vi "CRYStimulus Editor Sub.vi"(8 "List Index":i32, 9 "Stimulus In":T2={"StimulusType"="", "UseMLValArray"=[], "ML_axisArray"=[], "MLValLevelNameArray"=[], "Level(U)Array"=[1.0, 0.0, 0.0, 0.0, 0.0, 0.0, 0.26], "Start(Stop)FreqArray"=[20000.0, 20.0], "Start(Stop)AmpArray"=[0.5, 1.0], "StepResolutionArray"=[], "Unit_Array"=[], "DegValArray"=[], "DegUnitArray"=[], "Steps1"=19, "Cycle/step1(#)"=20, "Time/step1(s)"=0.01, "Transition1"=0.0, "SweepRate2"=1.0, "Freq3(Hz)"=0.0, "Steps3(#)"=19.0, "Cycles3(#)"=12, "StepSize3"=0.0, "wave time"="", "RMS_Value4"=0.0, "Peak_Value4"=0.0, "WavePath4"="", "RMS_unit4"="", "Peak_unit4"="", "wave Info"="", "dc_ctrl5_1"=0, "dc_ctrl5_2"=0, "dc_polar5"=0, "Max.Current"=0, "Steps5(#)"=19, "Time/Step5"=0.05, "Level5"=0.0, "StepsSize5Val"=0.0, "StepSize5Unit"="", "SweepType"=0, "Fixed/Ratio6"=0, "Transition6"=0.0, "Steps6(#)"=19.0, "Cycle/Steps6(#)"=12, "Time/Steps6(s)"=0.0, "Freq6(Hz)"=0.0, "Difference6(Hz)"=0.0, "Ratio6"="", "NoiseType7"=0, "Duration7(s)"=1.0, "MinFreq7(Hz)"=20000.0, "MaxFreq7(Hz)"=20.0, "MinFreq8(Hz)"=20000.0, "MaxFreq8(Hz)"=20.0, "FreqRounding8"=FALSE, "Duration8(s)"=1.0, "Tones8"=0.0, "RoundingVal8"=0.0, "ApplyEQ"=FALSE, "Duration(s)"=0.0, "CustomStimulusName "="", "Flatten Element Array"=[], "sine waves"=[], "Channel Out"=0, "RatioVal6"=0.0, "TabCtrl6"=enum."Master Tone", "Signal Type Name"="", "Help"="", "Channel Sel"=19, "V on DUT"=FALSE, "Output Imp"=6300.0, "Nominal Imp"=100.0} {"Nominal Imp" format="%.2p"; "Output Imp" format="%.2p"; "sine waves"."cycles" format="%.2f"; "sine waves"."ampl" format="%.2f"; "sine waves"."freq" format="%.2f"}) -> (1 "Ok Boolean":bool, 2 "Flatten Element Out":string, 3 "Stimulus Out":T2={"StimulusType"="", "UseMLValArray"=[], "ML_axisArray"=[], "MLValLevelNameArray"=[], "Level(U)Array"=[1.0, 0.0, 0.0, 0.0, 0.0, 0.0, 0.26], "Start(Stop)FreqArray"=[20000.0, 20.0], "Start(Stop)AmpArray"=[0.5, 1.0], "StepResolutionArray"=[], "Unit_Array"=[], "DegValArray"=[], "DegUnitArray"=[], "Steps1"=19, "Cycle/step1(#)"=20, "Time/step1(s)"=0.01, "Transition1"=0.0, "SweepRate2"=1.0, "Freq3(Hz)"=0.0, "Steps3(#)"=19.0, "Cycles3(#)"=12, "StepSize3"=0.0, "wave time"="", "RMS_Value4"=0.0, "Peak_Value4"=0.0, "WavePath4"="", "RMS_unit4"="", "Peak_unit4"="", "wave Info"="", "dc_ctrl5_1"=0, "dc_ctrl5_2"=0, "dc_polar5"=0, "Max.Current"=0, "Steps5(#)"=19, "Time/Step5"=0.05, "Level5"=0.0, "StepsSize5Val"=0.0, "StepSize5Unit"="", "SweepType"=0, "Fixed/Ratio6"=0, "Transition6"=0.0, "Steps6(#)"=19.0, "Cycle/Steps6(#)"=12, "Time/Steps6(s)"=0.0, "Freq6(Hz)"=0.0, "Difference6(Hz)"=0.0, "Ratio6"="", "NoiseType7"=0, "Duration7(s)"=1.0, "MinFreq7(Hz)"=20000.0, "MaxFreq7(Hz)"=20.0, "MinFreq8(Hz)"=20000.0, "MaxFreq8(Hz)"=20.0, "FreqRounding8"=FALSE, "Duration8(s)"=1.0, "Tones8"=0.0, "RoundingVal8"=0.0, "ApplyEQ"=FALSE, "Duration(s)"=0.0, "CustomStimulusName "="", "Flatten Element Array"=[], "sine waves"=[], "Channel Out"=0, "RatioVal6"=0.0, "TabCtrl6"=enum."Master Tone", "Signal Type Name"="", "Help"="", "Channel Sel"=19, "V on DUT"=FALSE, "Output Imp"=6300.0, "Nominal Imp"=100.0} {"Nominal Imp" format="%.2p"; "Output Imp" format="%.2p"; "sine waves"."cycles" format="%.2f"; "sine waves"."ampl" format="%.2f"; "sine waves"."freq" format="%.2f"})   [LabVIEW 2013]
uses:
  Typedef Control/CRYStimulus Cluster.ctl
  Control/CRYfstepsw.ctl
  Control/CRYflogsw.ctl
  Control/CRYampsw.ctl
  Control/CRYwavefile.ctl
  Control/CRYdcconn.ctl
  Control/CRYtwotone.ctl
  Control/CRYnoise.ctl
  Control/CRYmltitone.ctl
  SubVI/CRYStimulus Global.vi
  CRYProject/CRYProject Editor Global.vi
  CRYMainGlobal.vi
panel:
  in  "CurLibChange":bool caption="Add Lib"
  in  "StartFreq8_Flag":string
  in  "StopFreq8_Flag":string
  in  "StartFreq7_Flag":string
  in  "StopFreq7_Flag":string
  in  "StartFreq6_Flag":string
  in  "StopFreq6_Flag":string
  in  "StartFreq2_Flag":string
  in  "StopFreq2_Flag":string
  in  "StopFreq1_Flag":string
  in  "StartFreq1_Flag":string
  in  "StartStopFreqValue":string
  in  "StartStopAxis":string
  in  "Cancel":bool caption="Apply"
  in  "OK":bool caption="Apply"
  in  "stop":bool
  in  "Board1 Tab":enum32{"Setting", "Help"}(tab)
  in  "Stimulus Type":u16(ring) caption="激励类型" items=["频率步进扫频"=0, "频率对数扫频"=1, "幅度对数扫频"=2, "WAV文件"=3, "双音信号"=5, "噪声信号"=6, "多音信号"=7]
  in  "Control Tab":T1(tab)
  in  "StopFreq1_CurLib":u16(ring) caption="unity" items=["采集延迟", "Max FSD Out 12th&3rd Oct Sweep", "Max FSD In", "unity cal-in sens-in", "CRY33x Mic 1 sens-in", "CRY33x Mic 2 sens-in", "CRY33x Mic 3 sens-in", "CRY33x Mic 4 sens-in", "USB In L sens-in", "USB In R sens-in", "unity cal-out sens-out", "CRY602 Mouth 1 sens-out", "CRY602 Mouth 2 sens-out", "USB Out R sens-out"]
  in  "StopFreq1_axis":u16(slide) scale=0.0..2.0
  out "StopFreq1_Value":dbl caption="Hz" format="%#_6p"
  in  "StartFreq1_CurLib":u16(ring) caption="unity" items=["采集延迟", "Max FSD Out 12th&3rd Oct Sweep", "Max FSD In", "unity cal-in sens-in", "CRY33x Mic 1 sens-in", "CRY33x Mic 2 sens-in", "CRY33x Mic 3 sens-in", "CRY33x Mic 4 sens-in", "USB In L sens-in", "USB In R sens-in", "unity cal-out sens-out", "CRY602 Mouth 1 sens-out", "CRY602 Mouth 2 sens-out", "USB Out R sens-out"]
  in  "StartFreq1_axis":u16(slide) scale=0.0..2.0
  out "StartFreq1_Value":dbl caption="Hz" format="%#_6p"
  in  "StartFreq1_Caption":string caption="Message"
  in  "ML axis1":u16(slide) scale=0.0..2.0
  in  "UseMLVal_Level_1":u16(slide)
  in  "Time/steps1(s)":dbl=0.01 caption="最短持续时间(s)" format="%#_3p"
  out "Transition1":dbl caption="转换频率" format="%#_3p"
  in  "Cycle/step1":u32=20 caption="最小周期数" min=1 max=1000 format="%.0p"
  in  "Steps1":i32=19 caption="步骤数" format="%.0p"
  in  "StopFreq1(Hz)":dbl=20.0 caption="停止(Hz)" step=1000.0002384185791 format="%#.3p"
  in  "StartFreq1(Hz)":dbl=20000.0 caption="开始(Hz)" step=1200.0012397766113 format="%#.3p"
  in  "Step Resolution1":u16(ring) caption="分辨率" items=["R10(1/3 Oct.)", "R20(1/6 Oct.)", "R40(1/12 Oct.)", "R80(1/24 Oct.)", "User Defined, Log", "User Defined,Linear"]
  in  "unit1":u16(ring) items=["V  RMS", "dB re 1V"]
  in  "Level(U)1":dbl=1.0 format="%-#1.3p"
  out "deg1":dbl caption="Hz" format="%#_6p"
  in  "ML val level name":u16(ring) caption="unity" items=["unity cal-in sens-in", "CRY33x Mic 1 sens-in", "CRY33x Mic 2 sens-in", "CRY33x Mic 3 sens-in", "CRY33x Mic 4 sens-in", "USB In L sens-in", "USB In R sens-in", "unity cal-out sens-out", "CRY602 Mouth 1 sens-out", "CRY602 Mouth 2 sens-out", "USB Out R sens-out"]
  out "Level1":bool caption="幅度"
  out "Step Progression1":bool caption="步进设置"
  out "Frequency Range1":bool caption="频率范围"
  out "Step Size1":bool caption="步长"
  in  "StopFreq1_Caption":string caption="Message"
  in  "Nominal Imp1":dbl=1.0 caption="额定阻抗" min=1.0 max=2000.0 format="%-#1.3f"
  in  "Output Imp1":u16(ring) caption="输出阻抗" items=["1", "33", "150", "600", "750"]
  in  "V on DUT1":bool caption="Boolean"
  in  "V on DUT2":bool caption="Boolean"
  in  "Output Imp2":u16(ring) caption="输出阻抗" items=["1", "33", "150", "600", "750"]
  in  "Nominal Imp2":dbl=1.0 caption="额定阻抗" min=1.0 max=2000.0 format="%-#1.3f"
  in  "StopFreq2_CurLib":u16(ring) caption="unity" items=["采集延迟", "Max FSD Out 12th&3rd Oct Sweep", "Max FSD In", "unity cal-in sens-in", "CRY33x Mic 1 sens-in", "CRY33x Mic 2 sens-in", "CRY33x Mic 3 sens-in", "CRY33x Mic 4 sens-in", "USB In L sens-in", "USB In R sens-in", "unity cal-out sens-out", "CRY602 Mouth 1 sens-out", "CRY602 Mouth 2 sens-out", "USB Out R sens-out"]
  in  "StopFreq2_axis":u16(slide) scale=0.0..2.0
  out "StopFreq2_Value":dbl caption="Hz" format="%#_6p"
  in  "StartFreq2_CurLib":u16(ring) caption="unity" items=["采集延迟", "Max FSD Out 12th&3rd Oct Sweep", "Max FSD In", "unity cal-in sens-in", "CRY33x Mic 1 sens-in", "CRY33x Mic 2 sens-in", "CRY33x Mic 3 sens-in", "CRY33x Mic 4 sens-in", "USB In L sens-in", "USB In R sens-in", "unity cal-out sens-out", "CRY602 Mouth 1 sens-out", "CRY602 Mouth 2 sens-out", "USB Out R sens-out"]
  in  "StartFreq2_axis":u16(slide) scale=0.0..2.0
  out "StartFreq2_Value":dbl caption="Hz" format="%#_6p"
  out "Frequency Range2":bool caption="频率范围"
  out "Step Progression2":bool caption="步进设置"
  out "Level2":bool caption="幅度"
  in  "Sweept Rate2(s/dec)":dbl=1.0 caption="扫频速率(s/dec)" format="%#.3p"
  in  "StopFreq2(Hz)":dbl=100.0 caption="停止(Hz)" format="%#.3p"
  in  "StartFreq2(Hz)":dbl=10.0 caption="开始(Hz)" max=20000.0 format="%#.3p"
  in  "unit2":u16(ring) items=["V  RMS", "dB re 1V"]
  in  "Level(U)2":dbl=1.0 min=3.355e-21 max=1.84838 format="%-#1.3p"
  in  "ML val level name2":u16(ring) caption="unity" items=["unity cal-in sens-in", "CRY33x Mic 1 sens-in", "CRY33x Mic 2 sens-in", "CRY33x Mic 3 sens-in", "CRY33x Mic 4 sens-in", "USB In L sens-in", "USB In R sens-in", "unity cal-out sens-out", "CRY602 Mouth 1 sens-out", "CRY602 Mouth 2 sens-out", "USB Out R sens-out"]
  out "deg2":dbl caption="Hz" format="%#_6p"
  in  "UseMLVal_Level_2":u16(slide)
  in  "ML axis2":u16(slide) scale=0.0..2.0
  in  "StopFreq2_Caption":string caption="Message"
  in  "StartFreq2_Caption":string caption="Message"
  in  "Steps3":i32=19 caption="步骤数" format="%.0p"
  out "Step Size3":dbl caption="步长" format="%#.3p"
  in  "unit3":u16(ring) items=["V  RMS", "dB re 1V"]
  in  "Cycles3":u32=12 caption="周期" min=1 step=1 format="%.0p"
  in  "Stop Amp3":dbl=1.0 caption="停止" min=0.0 format="%#.3p"
  in  "Start Amp3":dbl=0.5 caption="开始" min=0.0 format="%#.3p"
  in  "Freq3(Hz)":dbl=1000.0 format="%#.3p"
  in  "ML val level name3":u16(ring) caption="unity" items=["unity cal-in sens-in", "CRY33x Mic 1 sens-in", "CRY33x Mic 2 sens-in", "CRY33x Mic 3 sens-in", "CRY33x Mic 4 sens-in", "USB In L sens-in", "USB In R sens-in", "unity cal-out sens-out", "CRY602 Mouth 1 sens-out", "CRY602 Mouth 2 sens-out", "USB Out R sens-out"]
  out "deg3":dbl caption="Hz" format="%#_6p"
  in  "UseMLVal_Level_3":u16(slide)
  in  "ML axis3":u16(slide) scale=0.0..2.0
  out "Frequency(Hz)3":bool caption="频率(Hz)"
  out "Step Progression3":bool caption="步进设置"
  out "Level Range3":bool caption="幅度范围"
  in  "Wave Channel":u16(ring) caption="通道" items=["Left", "Right"]
  in  "Wave Path4":path caption="波形文件路径"
  out "wave time":string caption="RMS"
  out "wave info":string caption="Peak"
  in  "RMS unit4":u16(ring) items=["dB FSD", "% FSD"]
  out "RMS value4":dbl caption="RMS"
  in  "Peak unit4":u16(ring) items=["dB FSD", "% FSD"]
  out "Peak value4":dbl caption="峰值"
  in  "unit4":u16(ring) items=["V  RMS", "dB RMS", "Vp"]
  in  "Level4(U)":dbl=1.0 min=0.0 max=1.84838 format="%#.3p"
  in  "ML val level name4":u16(ring) caption="unity" items=["unity cal-in sens-in", "CRY33x Mic 1 sens-in", "CRY33x Mic 2 sens-in", "CRY33x Mic 3 sens-in", "CRY33x Mic 4 sens-in", "USB In L sens-in", "USB In R sens-in", "unity cal-out sens-out", "CRY602 Mouth 1 sens-out", "CRY602 Mouth 2 sens-out", "USB Out R sens-out"]
  out "deg4":dbl caption="Hz" format="%#_6p"
  in  "UseMLVal_Level_4":u16(slide)
  in  "ML axis4":u16(slide) scale=0.0..2.0
  out "Level4":bool caption="幅度"
  out "WAV Info4":bool caption="WAV信息"
  in  "V on DUT4":bool caption="Boolean"
  in  "Output Imp4":u16(ring) caption="输出阻抗" items=["1", "33", "150", "600", "750"]
  in  "Nominal Imp4":dbl=1.0 caption="额定阻抗" min=1.0 max=2000.0 format="%-#1.3f"
  in  "dcpolar5":u16(slide) caption="极性"
  in  "dc_ctrl5_2":u16(slide) caption="源类型"
  out "Boolean3":bool
  in  "StopAmp5":dbl=1.0 caption="停止" format="%#.3p"
  in  "Time/Step5":dbl=0.05 caption="时间/步(s)" format="%.0p"
  out "Steps Size5":dbl caption="步长" format="%#_3g"
  in  "Steps5":i32=19 caption="步骤数" format="%.0p"
  in  "Level5":dbl caption="幅度"
  in  "dc_ctrl5_1":u16(slide) caption="控制方法"
  in  "Max.Current":u16(slide) caption="最大电流"
  in  "StartAmp5":dbl=1.0 caption="开始" format="%#.3p"
  out "Instrument Settings5":bool caption="仪器设置"
  out "Sweep Settings5":bool caption="扫描设置"
  out "Level Range5":bool caption="幅度范围"
  out "unit5_1":string
  out "unit5_2":string
  in  "Control6 Tab":enum32{"Master Tone", "Slave Tone"}(tab)
  out "Step Size6":bool caption="步长"
  out "Frequency Range6":bool caption="频率范围"
  out "Transition6":dbl caption="转换频率" format="%#_3p"
  in  "Time/step6(s)":dbl caption="最短持续时间(s)" min=0.0 format="%#.2p"
  in  "Cycle/steps6":u32=12 caption="最小周期数" min=1 step=1 format="%.0p"
  in  "StopFreq6(Hz)":dbl=100.0 caption="停止(Hz)" min=1.0 step=3.999999761581421 format="%#.3p"
  in  "StartFreq6(Hz)":dbl=6300.0 caption="开始(Hz)" min=1.0 step=3999.999761581421 format="%#.3p"
  in  "Steps6":i32=19 caption="步骤数" format="%.0p"
  in  "unit6":u16(ring) items=["V  RMS", "dB re 1V"]
  in  "Level6_1(U)":dbl=1.0 format="%#.3p"
  in  "StepResolution6":u16(ring) caption="分辨率" items=["R10(1/3 Oct.)", "R20(1/6 Oct.)", "R40(1/12 Oct.)", "R80(1/24 Oct.)", "User Defined, Log", "User Defined,Linear"]
  in  "deg6":dbl caption="Hz" format="%#_6p"
  in  "ML val level name6_1":u16(ring) caption="unity" items=["unity cal-in sens-in", "CRY33x Mic 1 sens-in", "CRY33x Mic 2 sens-in", "CRY33x Mic 3 sens-in", "CRY33x Mic 4 sens-in", "USB In L sens-in", "USB In R sens-in", "unity cal-out sens-out", "CRY602 Mouth 1 sens-out", "CRY602 Mouth 2 sens-out", "USB Out R sens-out"]
  in  "ML axis6_1":u16(slide) scale=0.0..2.0
  in  "UseMLVal_Level6_1":u16(slide)
  out "Level6":bool caption="幅度"
  in  "StartFreq6_Caption":string caption="Message"
  in  "StopFreq6_Caption":string caption="Message"
  in  "StartFreq6_CurLib":u16(ring) caption="unity" items=["采集延迟", "Max FSD Out 12th&3rd Oct Sweep", "Max FSD In", "unity cal-in sens-in", "CRY33x Mic 1 sens-in", "CRY33x Mic 2 sens-in", "CRY33x Mic 3 sens-in", "CRY33x Mic 4 sens-in", "USB In L sens-in", "USB In R sens-in", "unity cal-out sens-out", "CRY602 Mouth 1 sens-out", "CRY602 Mouth 2 sens-out", "USB Out R sens-out"]
  in  "StartFreq6_axis":u16(slide) scale=0.0..2.0
  out "StartFreq6_Value":dbl caption="Hz" format="%#_6p"
  in  "StopFreq6_CurLib":u16(ring) caption="unity" items=["采集延迟", "Max FSD Out 12th&3rd Oct Sweep", "Max FSD In", "unity cal-in sens-in", "CRY33x Mic 1 sens-in", "CRY33x Mic 2 sens-in", "CRY33x Mic 3 sens-in", "CRY33x Mic 4 sens-in", "USB In L sens-in", "USB In R sens-in", "unity cal-out sens-out", "CRY602 Mouth 1 sens-out", "CRY602 Mouth 2 sens-out", "USB Out R sens-out"]
  in  "StopFreq6_axis":u16(slide) scale=0.0..2.0
  out "StopFreq6_Value":dbl caption="Hz" format="%#_6p"
  in  "Fixed/Ratio6":u16(slide)
  in  "Ratio Freq6(Hz)":dbl=1000.0 caption="Fixed Tone(Hz)" format="%#_1p"
  in  "Difference6(Hz)":dbl=100.0 caption="差异(Hz)" format="%#_3p"
  in  "Freq6(Hz)":dbl=1000.0 caption="Fixed Tone(Hz)" format="%#.3p"
  in  "deg6_1":dbl caption="Hz" format="%#_6p"
  in  "ML val level name6_2":u16(ring) caption="unity" items=["unity cal-in sens-in", "CRY33x Mic 1 sens-in", "CRY33x Mic 2 sens-in", "CRY33x Mic 3 sens-in", "CRY33x Mic 4 sens-in", "USB In L sens-in", "USB In R sens-in", "unity cal-out sens-out", "CRY602 Mouth 1 sens-out", "CRY602 Mouth 2 sens-out", "USB Out R sens-out"]
  in  "unit6_1":u16(ring) items=["V  RMS", "dB re 1V"]
  in  "Level6_2(U)":dbl format="%#.3p"
  in  "Ratio6":u16(ring) caption="比率" items=["1/1 Oct.", "1/3 Oct.", "1/6 Oct.", "1/12 Oct.", "1/24 Oct.", "User Defined"]
  out "Boolean6":bool
  in  "UseMLVal_Level6_2":u16(slide)
  in  "ML axis6_2":u16(slide) scale=0.0..2.0
  out "Level6_1":bool caption="幅度"
  out "Fixed Ton (Hz)6":bool caption="固定音调(Hz)"
  in  "Sweep Type":u16(slide)
  out "Sweep Type6":bool caption="扫频类型"
  in  "Noise Type7":u16(slide)
  in  "Duration7(s)":dbl=1.0 caption="时间(s)" min=0.0 format="%#.3p"
  in  "StopFreq7(Hz)":dbl=20.0 caption="Stop(Hz)" min=0.001 format="%#.3p"
  in  "StartFreq7(Hz)":dbl=20000.0 caption="Start(Hz)" min=0.001 format="%#.3p"
  in  "unit7":u16(ring) items=["V  RMS", "dB RMS", "Vp"]
  in  "Level7(U)":dbl=0.26 format="%#_3p"
  in  "ML val level name7":u16(ring) caption="unity" items=["unity cal-in sens-in", "CRY33x Mic 1 sens-in", "CRY33x Mic 2 sens-in", "CRY33x Mic 3 sens-in", "CRY33x Mic 4 sens-in", "USB In L sens-in", "USB In R sens-in", "unity cal-out sens-out", "CRY602 Mouth 1 sens-out", "CRY602 Mouth 2 sens-out", "USB Out R sens-out"]
  out "deg7":dbl caption="Hz" format="%#_6p"
  in  "UseMLVal_Level_7":u16(slide)
  in  "ML axis7":u16(slide) scale=0.0..2.0
  out "Level7":bool caption="幅度"
  out "Noise7":bool caption="噪音"
  out "Frequency Range7":bool caption="频率范围"
  in  "StopFreq7_Caption":string caption="Message"
  in  "StartFreq7_Caption":string caption="Message"
  in  "StartFreq7_CurLib":u16(ring) caption="unity" items=["采集延迟", "Max FSD Out 12th&3rd Oct Sweep", "Max FSD In", "unity cal-in sens-in", "CRY33x Mic 1 sens-in", "CRY33x Mic 2 sens-in", "CRY33x Mic 3 sens-in", "CRY33x Mic 4 sens-in", "USB In L sens-in", "USB In R sens-in", "unity cal-out sens-out", "CRY602 Mouth 1 sens-out", "CRY602 Mouth 2 sens-out", "USB Out R sens-out"]
  in  "StartFreq7_axis":u16(slide) scale=0.0..2.0
  out "StartFreq7_Value":dbl caption="Hz" format="%#_6p"
  in  "StopFreq7_CurLib":u16(ring) caption="unity" items=["采集延迟", "Max FSD Out 12th&3rd Oct Sweep", "Max FSD In", "unity cal-in sens-in", "CRY33x Mic 1 sens-in", "CRY33x Mic 2 sens-in", "CRY33x Mic 3 sens-in", "CRY33x Mic 4 sens-in", "USB In L sens-in", "USB In R sens-in", "unity cal-out sens-out", "CRY602 Mouth 1 sens-out", "CRY602 Mouth 2 sens-out", "USB Out R sens-out"]
  in  "StopFreq7_axis":u16(slide) scale=0.0..2.0
  out "StopFreq7_Value":dbl caption="Hz" format="%#_6p"
  in  "V on DUT7":bool caption="Boolean"
  in  "Output Imp7":u16(ring) caption="输出阻抗" items=["1", "33", "150", "600", "750"]
  in  "Nominal Imp7":dbl=1.0 caption="额定阻抗" min=1.0 max=2000.0 format="%-#1.3f"
  in  "Rounding Val8":dbl=5.0 caption="舍入值(Hz)" format="%#.3f"
  in  "Freq Rounding8":bool caption="频率四舍五入"
  in  "Duration8(s)":dbl=1.0 caption="持续时间(s)" min=0.0 format="%#.3p"
  in  "Tones8":i32 caption="多音数量" format="%.0p"
  in  "StopFreq8(Hz)":dbl=20.0 caption="Stop(Hz)" min=1.0 step=3.999999761581421 format="%#.3p"
  in  "StartFreq8(Hz)":dbl=20000.0 caption="Start(Hz)" min=1.0 step=3999.999761581421 format="%#.3p"
  out "deg8":dbl caption="Hz" format="%#_6p"
  in  "ML val level name8":u16(ring) caption="unity" items=["unity cal-in sens-in", "CRY33x Mic 1 sens-in", "CRY33x Mic 2 sens-in", "CRY33x Mic 3 sens-in", "CRY33x Mic 4 sens-in", "USB In L sens-in", "USB In R sens-in", "unity cal-out sens-out", "CRY602 Mouth 1 sens-out", "CRY602 Mouth 2 sens-out", "USB Out R sens-out"]
  in  "Level8(U)":dbl=0.26 format="%#.3p"
  in  "unit8":u16(ring) items=["V  RMS", "dB RMS", "Vp"]
  in  "Step Resolution8":u16(ring) caption="分辨率" items=["R10(1/3 Oct.)", "R20(1/6 Oct.)", "R40(1/12 Oct.)", "R80(1/24 Oct.)", "User Defined, Log", "User Defined,Linear"]
  in  "UseMLVal_Level_8":u16(slide)
  in  "ML axis8":u16(slide) scale=0.0..2.0
  out "Level8":bool caption="幅度"
  out "Multitone8":bool caption="多频音"
  out "Frequency Range8":bool caption="频率范围"
  in  "StopFreq8_Caption":string caption="Message"
  in  "StartFreq8_Caption":string caption="Message"
  in  "StartFreq8_CurLib":u16(ring) caption="unity" items=["采集延迟", "Max FSD Out 12th&3rd Oct Sweep", "Max FSD In", "unity cal-in sens-in", "CRY33x Mic 1 sens-in", "CRY33x Mic 2 sens-in", "CRY33x Mic 3 sens-in", "CRY33x Mic 4 sens-in", "USB In L sens-in", "USB In R sens-in", "unity cal-out sens-out", "CRY602 Mouth 1 sens-out", "CRY602 Mouth 2 sens-out", "USB Out R sens-out"]
  in  "StartFreq8_axis":u16(slide) scale=0.0..2.0
  out "StartFreq8_Value":dbl caption="Hz" format="%#_6p"
  in  "StopFreq8_CurLib":u16(ring) caption="unity" items=["采集延迟", "Max FSD Out 12th&3rd Oct Sweep", "Max FSD In", "unity cal-in sens-in", "CRY33x Mic 1 sens-in", "CRY33x Mic 2 sens-in", "CRY33x Mic 3 sens-in", "CRY33x Mic 4 sens-in", "USB In L sens-in", "USB In R sens-in", "unity cal-out sens-out", "CRY602 Mouth 1 sens-out", "CRY602 Mouth 2 sens-out", "USB Out R sens-out"]
  in  "StopFreq8_axis":u16(slide) scale=0.0..2.0
  out "StopFreq8_Value":dbl caption="Hz" format="%#_6p"
  in  "V on DUT8":bool caption="Boolean"
  in  "Output Imp8":u16(ring) caption="输出阻抗" items=["1", "33", "150", "600", "750"]
  in  "Nominal Imp8":dbl=1.0 caption="额定阻抗" min=1.0 max=2000.0 format="%-#1.3f"
  out "Proper VI No":i32
  in  "Help":string
  out "Vmax (V)":dbl
  out "Sampling Rate (Hz)":u32
  out "Sens y":dbl
  out "Max Freq":dbl=20000.0
  in  "RealFreq3(Hz)":dbl=1000.0 format="%#.3p"
  out "LinLevel2":dbl=1.0 format="%-#1_3p"
  out "LinLevel1":dbl=1.0 format="%-#1_3p"
  out "Channel Change":string
  out "MaxLevel_2":dbl=1.0 format="%-#1_3p"
  out "MaxLevel_1":dbl=1.0 format="%-#1_3p"
  out "dB ref.":dbl=1.0 format="%.2f"
  out "prefix Out":string
  in  "Res Max Freq":dbl=20000.0
  out "Stimulus Change":string
  in  "Load_Test":bool
  in  "Update":bool
  out "TSR params":T3 {"Amplit" format="%.2f"; "FStop" format="%.2f"; "FStart" format="%.2f"; "FSamp" format="%.2f"; "Tsamp" format="%.2f"; "NHarm" format="%.2f"; "MStart" format="%.2f"; "MStop" format="%.2f"; "NOffset" format="%.2f"}
  out "step size Hz":dbl caption="Hz" format="%.1f"
  # "(1,2,3,4,6_1,6_2,7,8)"
  # "(1,2,3,4,6_1,6_2,7,8)"
  # "(1,2,3,4,6_1,6_2,7,8)"
  # "(1,2,4,6_1,6_2,7,8)"
  # "(1,2,6)"
  # "(3,5)"
  # "(1,6,8)"
  # "(1,2,4,6_1,6_2,7,8)"
  # "(1,2,3,4,6_1,6_2,7,8)"
  # "(1,2,3,4,6_1,6_2,7,8)"
  # "(1,2,3,4,6_1,6_2,7,8)"
  # "(1,2,3,4,6_1,6_2,7,8)"
  # "(1,2,3,4,6_1,6_2,7,8)"
  # "(1,2,4,6_1,6_2,7,8)"
  # "(1,2,6)"
  # "(3,5)"
  # "(1,6,8)"
  # "(1,2,4,6_1,6_2,7,8)"
  # "(1,2,3,4,6_1,6_2,7,8)"
  # "(1,2,3,4,6_1,6_2,7,8)"
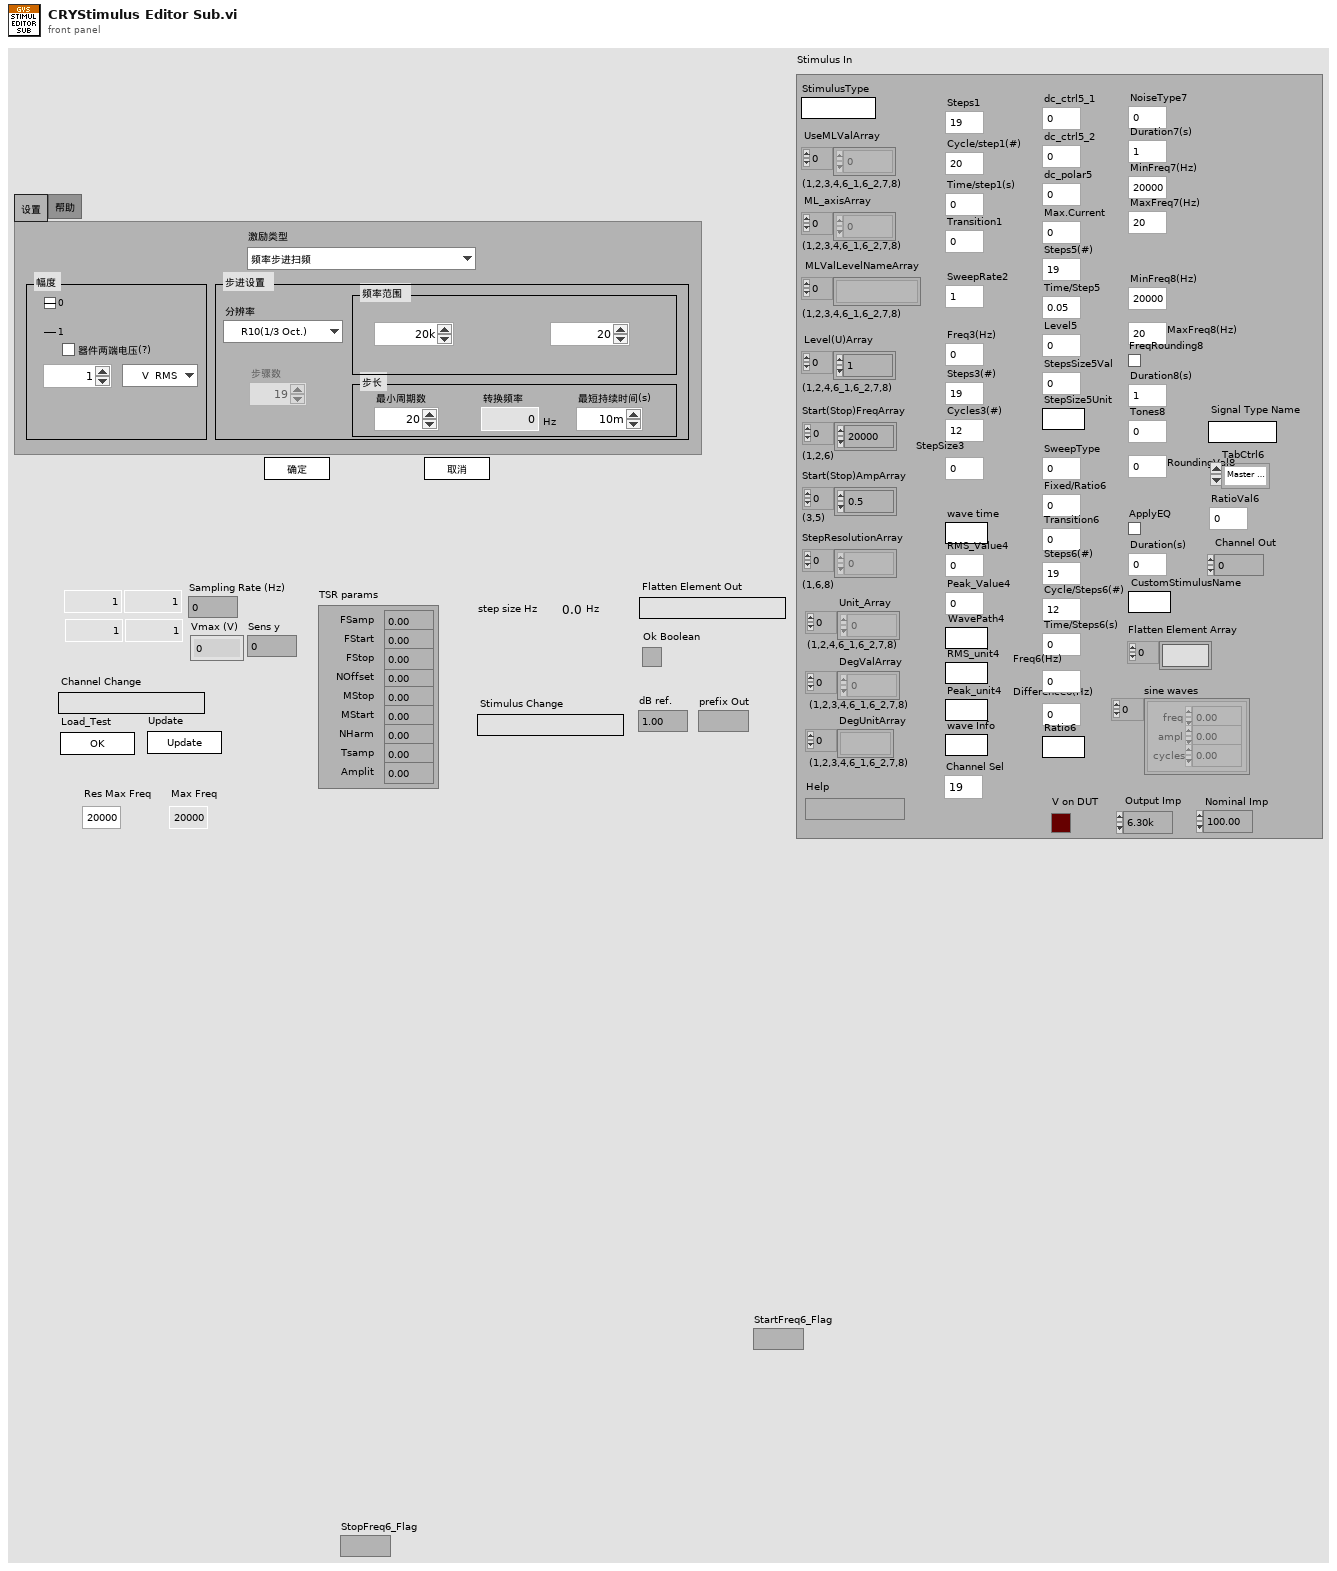
[diagram p1: front panel]
types:
  T1 = enum32{"Page1", "Page2", "Page3", "Page4", "Page5", "Page6", "Page7", "Page8"}
  T2 = typedef "CRYStimulus Cluster.ctl" = cluster{"StimulusType":string, "UseMLValArray":u16[], "ML_axisArray":u16[], "MLValLevelNameArray":string[], "Level(U)Array":dbl[], "Start(Stop)FreqArray":dbl[], "Start(Stop)AmpArray":dbl[], "StepResolutionArray":u16[], "Unit_Array":u16[], "DegValArray":dbl[], "DegUnitArray":string[], "Steps1":i32, "Cycle/step1(#)":u32, "Time/step1(s)":dbl, "Transition1":dbl, "SweepRate2":dbl, "Freq3(Hz)":dbl, "Steps3(#)":dbl, "Cycles3(#)":u32, "StepSize3":dbl, "wave time":string, "RMS_Value4":dbl, "Peak_Value4":dbl, "WavePath4":string, "RMS_unit4":string, "Peak_unit4":string, "wave Info":string, "dc_ctrl5_1":u16, "dc_ctrl5_2":u16, "dc_polar5":u16, "Max.Current":u16, "Steps5(#)":u32, "Time/Step5":dbl, "Level5":dbl, "StepsSize5Val":dbl, "StepSize5Unit":string, "SweepType":u16, "Fixed/Ratio6":u16, "Transition6":dbl, "Steps6(#)":dbl, "Cycle/Steps6(#)":u32, "Time/Steps6(s)":dbl, "Freq6(Hz)":dbl, "Difference6(Hz)":dbl, "Ratio6":string, "NoiseType7":u16, "Duration7(s)":dbl, "MinFreq7(Hz)":dbl, "MaxFreq7(Hz)":dbl, "MinFreq8(Hz)":dbl, "MaxFreq8(Hz)":dbl, "FreqRounding8":bool, "Duration8(s)":dbl, "Tones8":dbl, "RoundingVal8":dbl, "ApplyEQ":bool, "Duration(s)":dbl, "CustomStimulusName ":string, "Flatten Element Array":string[], "sine waves":cluster{"freq":dbl, "ampl":dbl, "cycles":dbl}[], "Channel Out":i32, "RatioVal6":dbl, "TabCtrl6":enum32{"Master Tone", "Slave Tone"}, "Signal Type Name":string, "Help":string, "Channel Sel":u16, "V on DUT":bool, "Output Imp":dbl, "Nominal Imp":dbl}
  T3 = cluster{"FSamp":dbl, "FStart":dbl, "FStop":dbl, "NOffset":dbl, "MStop":dbl, "MStart":dbl, "NHarm":dbl, "Tsamp":dbl, "Amplit":dbl}
  T4 = typedef "CRYStep.ctl" = cluster{"No.VI":i32, "Category":string, "StepName":string, "Seq setup flattened":string, "Comment":string, "Steps config.":bool[], "Jump config":i32[], "Start":dbl, "Increment":dbl, "Name":string, "Unit":string, "Y data":u16, "Y prefix":string, "Y dB ref":dbl, "Y unit":string, "Repeat State Array":cluster{"Start":dbl, "Increment":dbl, "Count":i32, "Num":i32}[]}
  T5 = typedef "CRYData Cluster Array.ctl" = T6[]
  T6 = typedef "CRYData Cluster.ctl" = cluster{"Name":string, "Curve":cluster{"x":dbl, "y":dbl, "z":dbl}[], "X data":u16, "Y data":u16, "Z data":u16, "X axis":u16, "Y axis":u16, "Z axis":u16, "X unit":string, "Y unit":string, "Z unit":string, "X dB ref":dbl, "Y dB ref":dbl, "Z dB ref":dbl, "single val":bool, "protected":bool, "display X":bool, "display Y":bool, "display Z":bool, "Test Info":string, "Step No.":i32, "Plot Settings":cluster{"Color":u32, "Interpolation":u8, "Point Style":u8, "Line Style":u8, "Point Color":u32, "Line Width":u8, "Bar Plot Style":u8, "Fill To":i16}, "AutoProtect":bool}
  T7 = typedef "CRYHardware.ctl" = cluster{"Name":string, "Analog I/O":u16, "Digital I/O":u16, "Channels":u8, "Dig Dev ID":u8, "N ports":u8, "Interface":u32, "Dig I/O Ports":cluster{"port #":i16, "width":i16, "direction":i32}[], "Interf settings":cluster{"Type":u16, "COM Port":u8, "Baud rate":u32, "Data bits":u32, "Parity":u16, "Stop bits":u16, "Flow control":u16, "Dev ID IEEE":u8}[], "N interfs":i32, "udev SNs":i16[], "udev enable":bool, "Channel Array":T8[], "Cal sequence":string, "SelectedIn":u16, "SelectedOut":u16, "SelectedTab":u16, "State":bool, "Help":string, "Advanced":bool, "In Audio Driver":u16, "Out Audio Driver":u16}
  T8 = typedef "CRYHardware Channel Info.ctl" = cluster{"ID":i32, "Name":string, "Digital":bool, "Input":bool, "Device Name":string, "Hardware Ch ID":u8, "Vmax (V)":dbl, "Latency (samples)":dbl, "Sampling Rate (Hz)":u32, "Bit Depth":u32, "Anti-aliasing Factor (%fs)":sgl, "DAQmx Channel":tag, "term config":i32, "Coupling":i32, "IEPE en":bool, "ASIOChannel Name":string, "Audio Driver":u16, "ASIOChannel Index":u8}
  T9 = enum8{"Enabled", "Disabled", "Disabled and Grayed Out"}
  T10 = typedef "CRYfstepsw.ctl" = cluster{"Level(U)":dbl, "Start Freq(Hz)":dbl, "Stop Freq(Hz)":dbl, "ML val level name":string, "Use ML Val level?":bool, "ML axis":u8, "Steps (#)":i32, "Cycles/step(#)":u32, "Time/step (s)":dbl, "Step Resolution":u16, "unit":u16, "Start Freq Name":string, "Stop Freq Name":string, "Start Freq Axis":u8, "Stop Freq Axis":u8, "Start Freq Flag":string, "Stop Freq Flag":string, "Output Imp":dbl, "Nominal Imp":dbl, "V on DUT":bool}
  T11 = typedef "CRYflogsw.ctl" = cluster{"Level(U)":dbl, "Start Freq(Hz)":dbl, "Stop Freq(Hz)":dbl, "Sweep Rate(s/dec)":dbl, "Use ML Val level?":bool, "ML val level name":string, "ML axis":u8, "TSR params":cluster{"FSamp":dbl, "FStart":dbl, "FStop":dbl, "NOffset":dbl, "MStop":dbl, "MStart":dbl, "NHarm":dbl, "Tsamp":dbl, "Amplit":dbl}, "unit":u16, "Start Freq Name":string, "Stop Freq Name":string, "Start Freq Axis":u8, "Stop Freq Axis":u8, "Start Freq Flag":string, "Stop Freq Flag":string, "Output Imp":dbl, "Nominal Imp":dbl, "V on DUT":bool}
  T12 = typedef "CRYampsw.ctl" = cluster{"Freq(Hz)":dbl, "Steps (#)":i32, "Cycles(#)":u32, "Use ML Val freq?":bool, "ML val freq name":string, "ML axis":u8, "Start Ampl(U)":dbl, "Stop Ampl(U)":dbl, "unit":u16}
  T13 = typedef "CRYwavefile.ctl" = cluster{"Level(U)":dbl, "Wave Path":string, "ML axis":u8, "ML val level name":string, "Use ML Val level?":bool, "wave info":string, "wave time":string, "Peak value4":dbl, "RMS value4":dbl, "wave channel":u16, "unit":u16, "Output Imp":dbl, "Nominal Imp":dbl, "V on DUT":bool}
  T14 = typedef "CRYdcconn.ctl" = cluster{"dc ctrl":u16, "dcmax I":u16, "dc polar":u16, "dc ctrl":u16, "Steps (#)":i32, "Time/step (s)":dbl, "Start Ampl(U)":dbl, "Stop Ampl(U)":dbl, "Level(U)":dbl, "Step Size":dbl}
  T15 = typedef "CRYtwotone.ctl" = cluster{"Steps (#)":i32, "Tone Type":u8, "Freq2(Hz)":dbl, "Time/step (s)":dbl, "Cycles/step (#)":u32, "ML val level name":string, "Use ML Val level?":bool, "Level(U) 2":dbl, "Diff Freq(Hz)":dbl, "ML axis 2":u8, "Diff/Ratio":u8, "Level(U)":dbl, "Stop Freq(Hz)":dbl, "Ratio Val":dbl, "ML val level name 2":string, "Use ML Val level? 2":bool, "ML axis":u8, "Start Freq(Hz)":dbl, "Step Resolution":u16, "Ratio":u16, "TabCtrl6":enum32{"Master Tone", "Slave Tone"}, "unit 1":u16, "unit 2":u16, "Start Freq Name":string, "Stop Freq Name":string, "Start Freq Axis":u8, "Stop Freq Axis":u8, "Start Freq Flag":string, "Stop Freq Flag":string}
  T16 = typedef "CRYnoise.ctl" = cluster{"Noise Type":u8, "Min Freq(Hz)":dbl, "Max Freq(Hz)":dbl, "Level(U)":dbl, "Duration(s)":dbl, "ML val level name":string, "Use ML Val level?":bool, "ML axis":u8, "unit":u16, "Start Freq Name":string, "Stop Freq Name":string, "Start Freq Axis":u8, "Stop Freq Axis":u8, "Start Freq Flag":string, "Stop Freq Flag":string, "Output Imp":dbl, "Nominal Imp":dbl, "V on DUT":bool}
  T17 = typedef "CRYmltitone.ctl" = cluster{"Level(U)":dbl, "Min Freq(Hz)":dbl, "Max Freq(Hz)":dbl, "Duration(s)":dbl, "Freq Rounding":bool, "Rounding Val":dbl, "Profile":i32, "ML axis 2":u8, "ML val level name":string, "Use ML Val level?":bool, "ML axis":u8, "Step Resolution":u16, "unit":u16, "Start Freq Name":string, "Stop Freq Name":string, "Start Freq Axis":u8, "Stop Freq Axis":u8, "Start Freq Flag":string, "Stop Freq Flag":string, "Output Imp":dbl, "Nominal Imp":dbl, "V on DUT":bool}
  T18 = typedef "CRYWaveFile Information Typedef.ctl" = cluster{"total number of samples/ch":u32, "total byte number":u32, "Time DBL":dbl, "format str":string, "Time Str":string, "peak FSD":dbl, "rms FSD":dbl, "peak %FSD":dbl, "rms %FSD":dbl, "rms":dbl, "Channel Number":u16, "rms L":dbl, "rms R":dbl}
  T19 = typedef "Sound Data Format.ctl" = cluster{"sample rate (S/s)":dbl, "number of channels":i32, "bits per sample":i32}
  T20 = typedef "CRYCalibration 2DCluster.ctl" = cluster{"Calibration":T21, "Corr Curve":T6, "EQ Curve":T6, "Sens Curve":T6}
  T21 = typedef "CRYCalibration Cluster.ctl" = cluster{"Calibration Step Name":string, "Device":string, "Correction Curve Name":string, "Equalization Curve Name":string, "Sensitivity Curve Name":string, "Corr Folder and File":string, "EQ Folder and File":string, "Sens Folder and File":string, "Corr Step size":u16, "EQ Step size":u16, "Input":bool, "Last Cal Date (sec)":timestamp, "Cha Name":string, "Corr Curve Found":bool, "EQ Curve Found":bool, "Sens Curve Found":bool, "Signal Type":string, "Calibrated Device":string, "Hz":u32}
  T22 = cluster{"Load_Test":bool, "OK":bool, "Cancel":bool}
  T23 = typedef "CRYCalibration All Cluster.ctl" = cluster{"Calibration 2D":T20[], "Help":string, "Tab Value":i32, "Input Signal Type":string, "Output Signal Type":string}
  T24 = typedef "CRYStimulus Parameter.ctl" = cluster{"Name":string, "Level Out":dbl, "Start Freq":dbl, "Stop Freq":dbl, "Steps":u32, "Cycles":u32, "Sweep type":i32, "Freq":dbl, "Start ampl":dbl, "Stop ampl":dbl, "sine waves":cluster{"freq":dbl, "ampl":dbl, "cycles":dbl}[], "wav path":string, "Sweep time":dbl, "Resolution":u16, "Tone type6":u16, "fix/ratio6":u16, "Ratio6":u16, "Difference6":u32, "RatioFreq6":u32}
  T25 = cluster{"fstepsw":T10, "flogsw":T11, "ampsw":T12, "wavefile":T13, "dcconn":T14, "twotone":T15, "mltitone":T17, "noise":T16, "sqwvsw":cluster{"Level(U)":dbl, "Duty Cycle":dbl, "ML val level name":string, "ML axis":u8, "Start Freq(Hz)":u32, "Stop Freq(Hz)":u32, "Use ML Val level?":bool, "Steps (#)":u32, "Cycles/step (#)":u32, "Time/step (s)":dbl, "Step Resolution":u16}, "tnbrst":cluster{"Level(U)":dbl, "ML val level name":string, "ML axis":u8, "Start Freq(Hz)":u32, "Use ML Val level?":bool, "Cycles/step (#)":u32, "Duration(s)":dbl}}
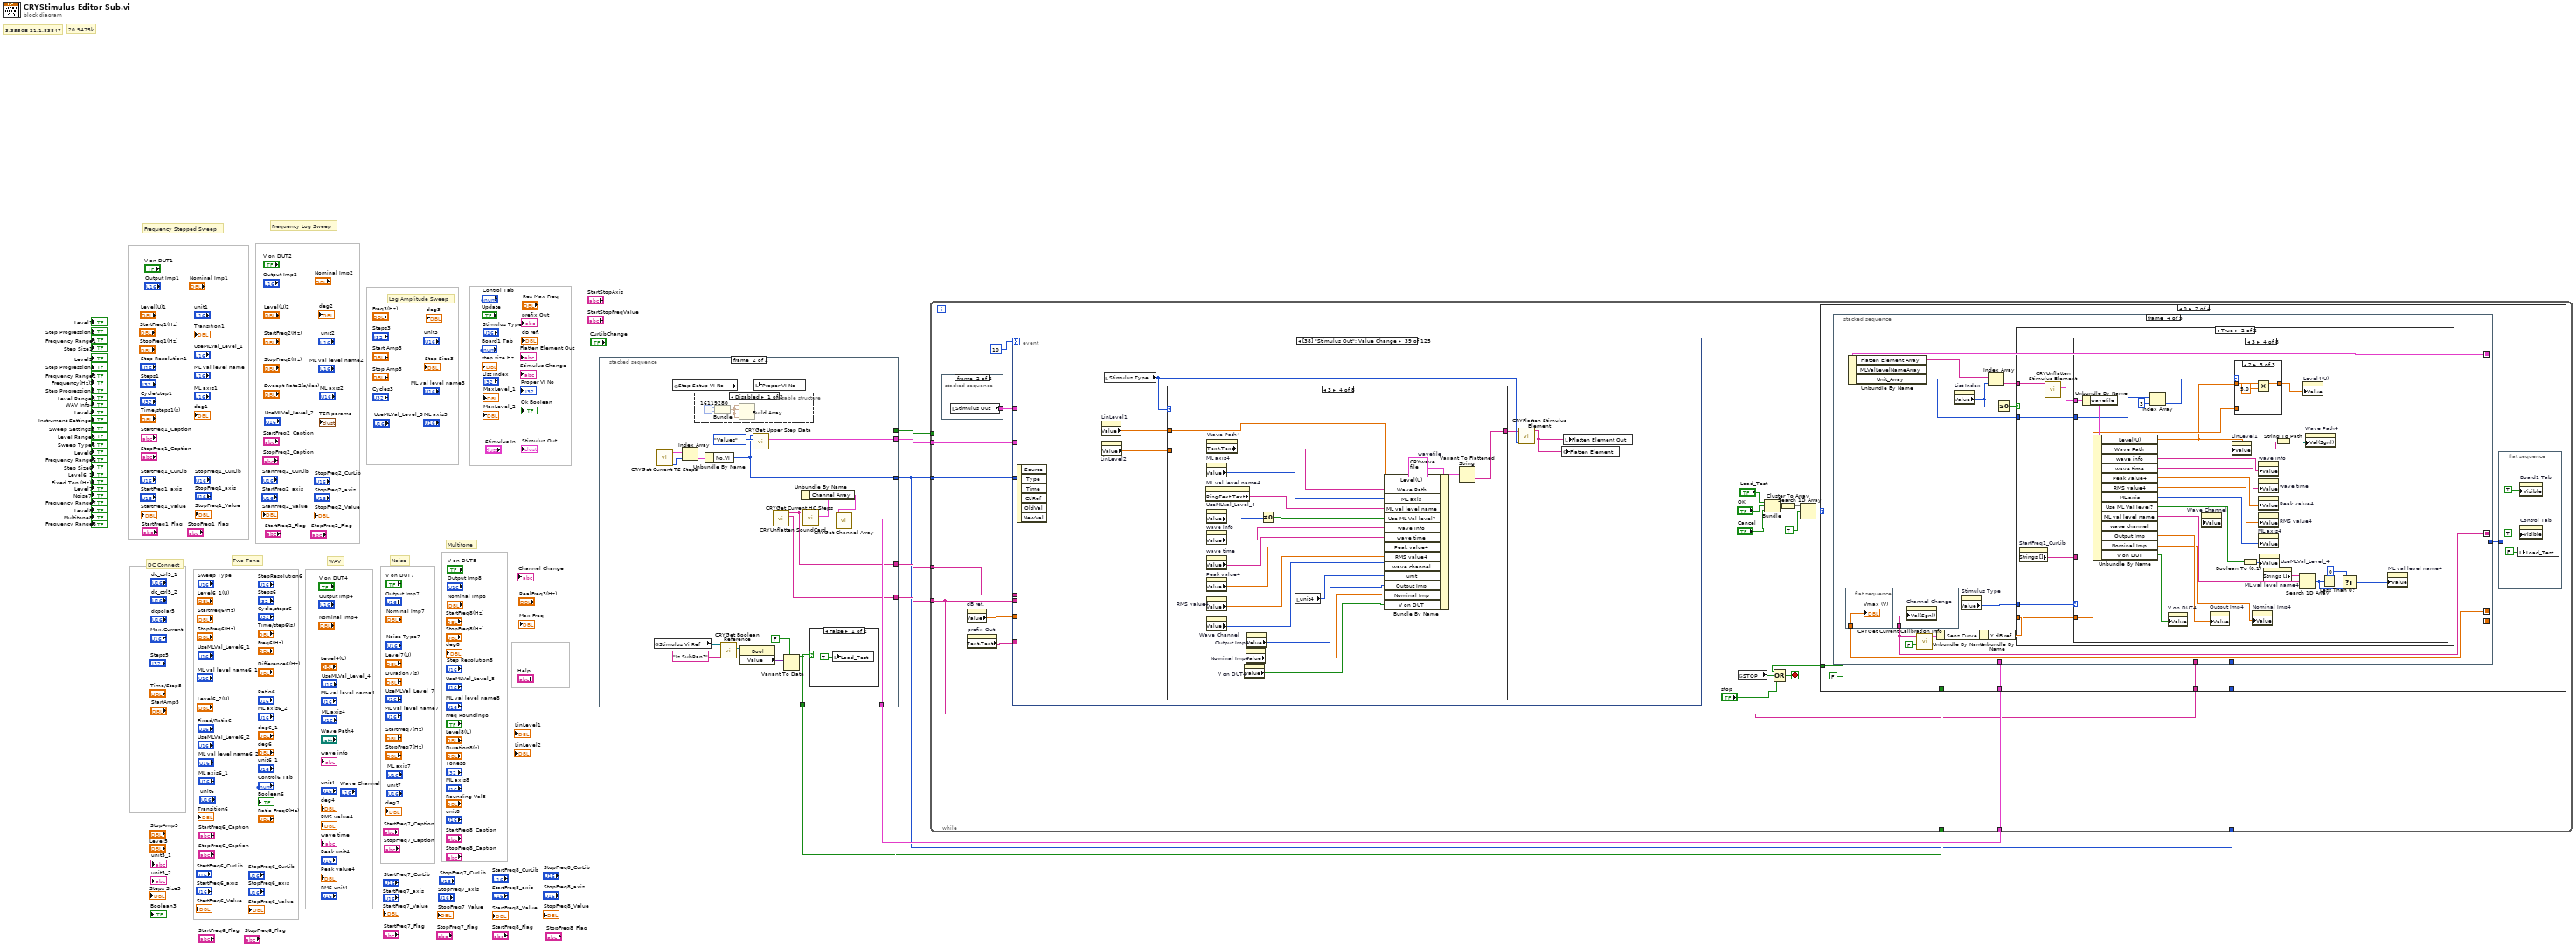
[diagram p0: block diagram]
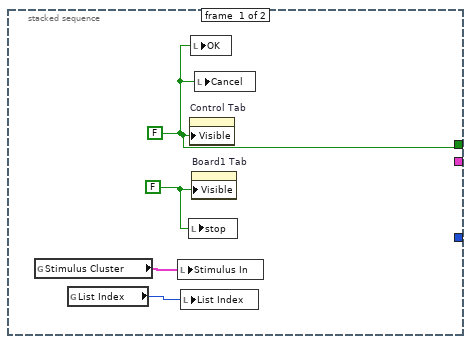
[diagram p2: hidden frame]
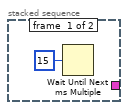
[diagram p5: hidden frame]
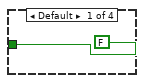
[diagram p6: hidden frame]
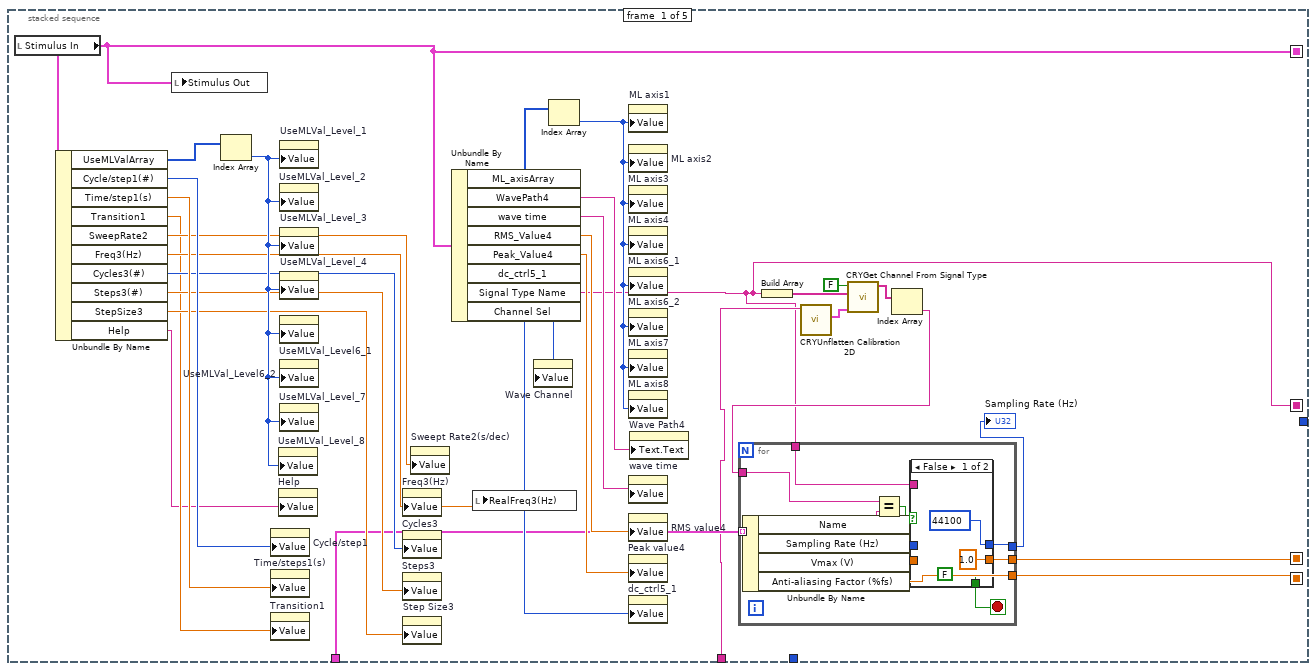
[diagram p7: hidden frame]
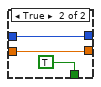
[diagram p8: hidden frame]
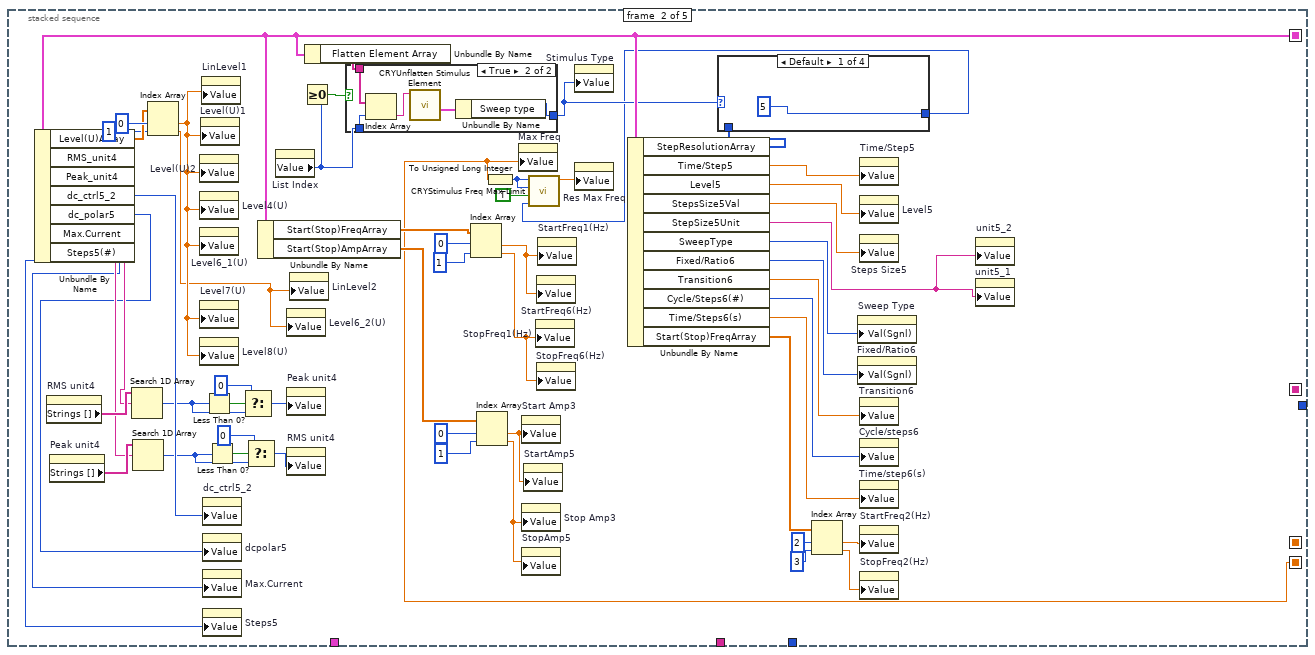
[diagram p9: hidden frame]
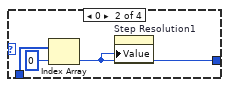
[diagram p10: hidden frame]
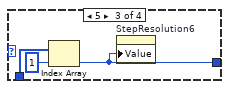
[diagram p11: hidden frame]
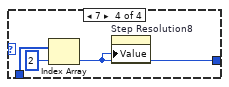
[diagram p12: hidden frame]
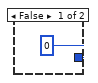
[diagram p13: hidden frame]
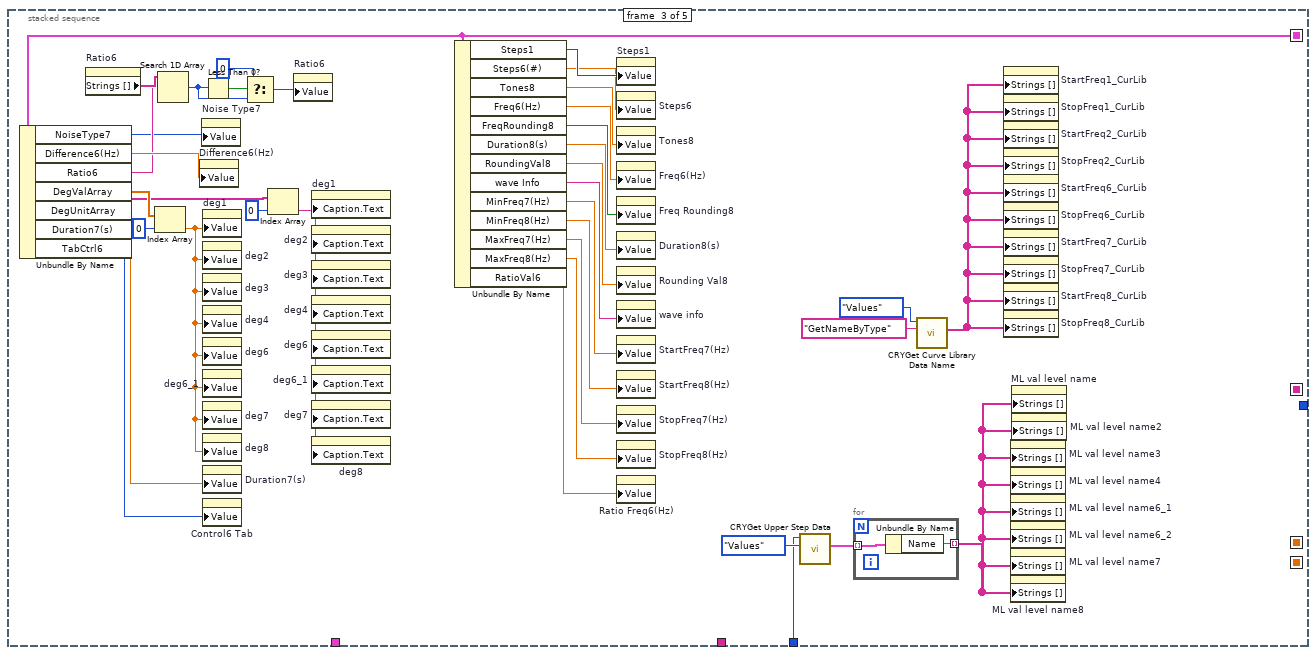
[diagram p14: hidden frame]
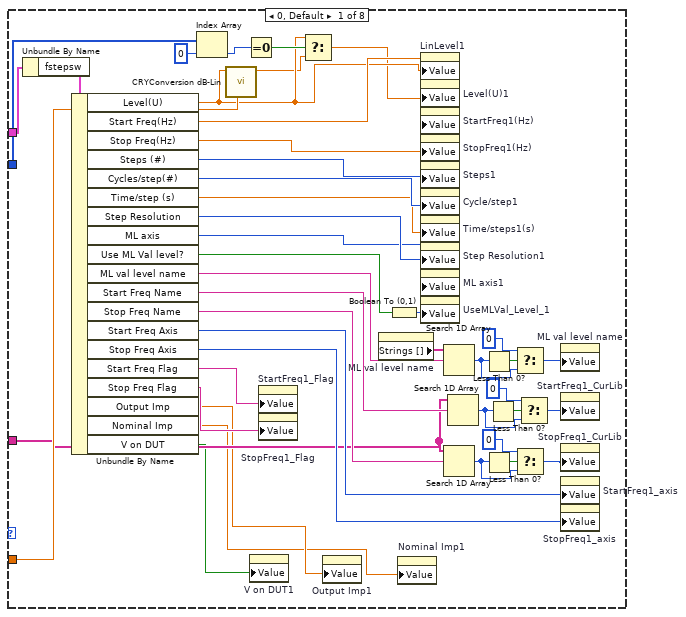
[diagram p16: hidden frame]
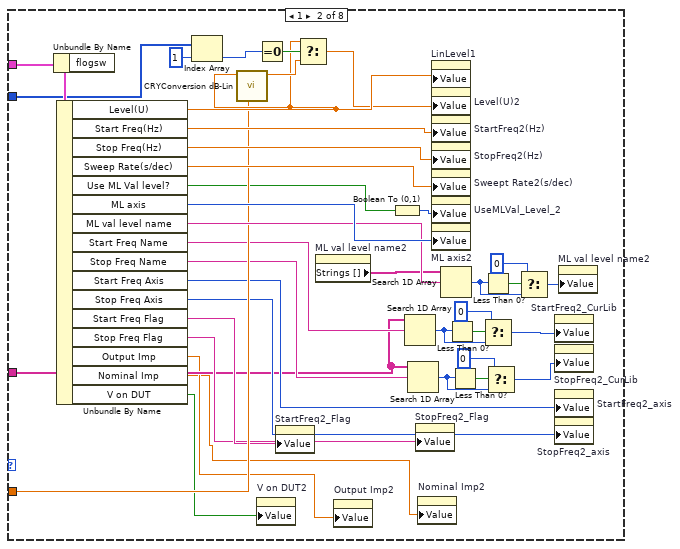
[diagram p17: hidden frame]
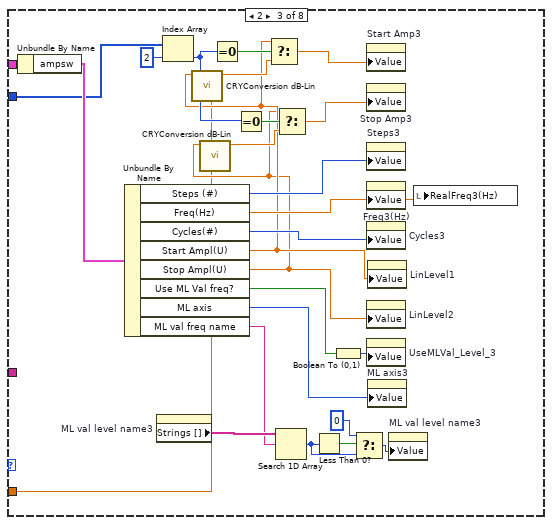
[diagram p18: hidden frame]
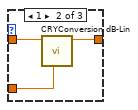
[diagram p20: hidden frame]
diagram:
  # "20.9475k"
  # "3.3550E-21,1.83847"
  # "Multitone"
  # "Noise"
  # "Two Tone"
  # "DC Connect"
  # "WAV"
  # "Log Amplitude Sweep"
  # "Frequency Log Sweep"
  # "Frequency Stepped Sweep"
  n1 = stacked-sequence {
    tunnel: [w8 _] -> w7
    tunnel: [_ w27] -> w6
    tunnel: [_ w26] -> w5
    tunnel: [_ w25] -> w4
    tunnel: [_ w22] -> w3
    tunnel: [_ w21] -> w2
    tunnel: [_ w12] -> w1
    frame #0 {
      w11 = FALSE ("Visible")
      w8 = FALSE ("Visible")
      n2 = global read "CRYStimulus Global.vi" "Stimulus Cluster"() -> (w10:T2)
      n3 = global read "CRYStimulus Global.vi" "List Index"() -> (w9:i32)
      n4 = local write "Stimulus In"(w10) -> ()
      n5 = local write "List Index"(w9) -> ()
      n6 = local write "stop"(w11) -> ()
      n7 = property on="Control Tab" class="TabCtl (strict)"("Visible"=w8) -> ()  [unwired: 2 in, 2 out]
      n8 = local write "OK"(w8) -> ()
      n9 = property on="Board1 Tab" class="TabCtl (strict)"("Visible"=w11) -> ()  [unwired: 2 in, 2 out]
      n10 = local write "Cancel"(w8) -> ()
    }
    frame #1 {
      n11 = global read "CRYStimulus Global.vi" "Stimulus Vi Ref"() -> (w19:refnum<vi>)
      n12 = call "CRYGet Current TS Steps.vi"() -> ("SelectStepNumber in Tree"=w13:i32, "Steps"=w14:T4[])  [unwired: 1 in, 9 out]
      n13 = global read "CRYProject Editor Global.vi" "Step Setup VI No"() -> (w29:i32)
      n14 = Index Array(array=w14, index=w13) -> (element=w15:T4)
      n15 = disable-structure shown="Disabled" {
        frame Disabled {
          w30 = u32 16119280
          n16 = Bundle(w30, w30) -> (w31:cluster{u32, u32})  [unwired: 1 in]
          n17 = Build Array(w31, w31, w31, w31) -> ()  [unwired: 1 out]
        }
        frame Enabled {
        }
      }
      n18 = Unbundle By Name(w15) -> ("No.VI"=w12:i32)
      n19 = call "CRYGet Boolean Reference.vi"("Label Name"="Is SubPan?", "VI Refnum"=w19) -> ("Boolean Ref"=w18:refnum<vi>)  [unwired: 9 out]
      n20 = property class="Bool"(reference=w18) -> ("Value"=w17:variant)  [unwired: 1 in, 2 out]
      n21 = call "CRYGet Upper Step Data.vi"("Type In"=enum16{"Curves", "Values", "Results", "WFM"}."Values", "No.VI"=w12) -> ("Value array"=w27:T5)  [unwired: 9 out]
      n22 = local write "Proper VI No"(w29) -> ()
      n23 = call "CRYGet Current HC Steps.vi"() -> ("Calibration setup flattened Out"=w21:string, "Hardware setup flattened Out"=w22:string)  [unwired: 10 in]
      n24 = Variant To Data(type=FALSE ("Visible"), Variant=w17) -> (data=w25:bool)  [unwired: 1 in, 1 out]
      n25 = call "CRYUnflatten SoundCard.vi"("Flatten SoundCard"=w22) -> ("SoundCard"=w24:T7)  [unwired: 10 out]
      n26 = Unbundle By Name(w24) -> ("Channel Array"=w23:T8[])
      n27 = case shown="False" w25 {
        frame False {
          n28 = local write "Load_Test"(TRUE ("Load_Test")) -> ()
        }
        frame True {
        }
      }
      n29 = call "CRYGet Channel Array.vi"("Channel Array"=w23) -> ("O Channel Info Out"=w26:T8[])  [unwired: 10 out]
    }
  }
  n30 = while {
    tunnel: w7 -> [_]
    tunnel: w6 -> [w45]
    tunnel: w5 -> [w41]
    tunnel: w4 -> [w40]
    tunnel: w3 -> [w39]
    tunnel: w2 -> [w35]
    tunnel: w1 -> [w34]
    tunnel: w1 -> [w33]
    stop <- w46 stop-if-true
    n31 = stacked-sequence {
      tunnel: [_ w56] -> w42
      frame #0 {
        n32 = Wait Until Next ms Multiple(millisecond multiple=u32 15) -> ()  [unwired: 1 out]
      }
      frame #1 {
        n33 = local read "Stimulus Out"() -> (w56:T2)
      }
    }
    n34 = property on="dB ref." class="DigNum (strict)"() -> ("Value"=w44:dbl)  [unwired: 2 in, 2 out]
    n35 = property on="prefix Out" class="Str"() -> ("Text.Text"=w43:string)  [unwired: 2 in, 2 out]
    n36 = event shown="[38] \"Stimulus Out\": Value Change" {
      selector: _ -> [_ _ _ _ _ _ _ _ _ _ _ _ _ _ _ _ _ _ _ _ _ _ _ _ _ _ _ _ _ _ _ _ _ _ _ _ _ _ _ _ _ _ _ _ _ _ _ _ _ _ _ _ _ _ _ _ _ _ _ _ _ _ _ _ _ _ _ _ _ _ _ _ _ _ _ _ _ _ _ _ _ _ _ _ _ _ _ _ _ _ _ _ _ _ _ _ _ _ _ _ _ _ _ _ _ _ _ _ _ _ _ _ _ _ _ _ _ _ _ _ _ _ _ _ _]
      dyn-events: _ -> [_ _ _ _ _ _ _ _ _ _ _ _ _ _ _ _ _ _ _ _ _ _ _ _ _ _ _ _ _ _ _ _ _ _ _ _ _ _ _ _ _ _ _ _ _ _ _ _ _ _ _ _ _ _ _ _ _ _ _ _ _ _ _ _ _ _ _ _ _ _ _ _ _ _ _ _ _ _ _ _ _ _ _ _ _ _ _ _ _ _ _ _ _ _ _ _ _ _ _ _ _ _ _ _ _ _ _ _ _ _ _ _ _ _ _ _ _ _ _ _ _ _ _ _ _]
      timeout: 10 -> [_ _ _ _ _ _ _ _ _ _ _ _ _ _ _ _ _ _ _ _ _ _ _ _ _ _ _ _ _ _ _ _ _ _ _ _ _ _ _ _ _ _ _ _ _ _ _ _ _ _ _ _ _ _ _ _ _ _ _ _ _ _ _ _ _ _ _ _ _ _ _ _ _ _ _ _ _ _ _ _ _ _ _ _ _ _ _ _ _ _ _ _ _ _ _ _ _ _ _ _ _ _ _ _ _ _ _ _ _ _ _ _ _ _ _ _ _ _ _ _ _ _ _ _ _]
      tunnel: w45 -> [_ _ _ _ _ _ _ _ w678 _ _ _ _ w728 _ w766 _ _ _ _ w814 _ _ _ w868 _ w904 _ _ _ _ _ w965 _ _ _ _ w1014 _ _ _ _ _ _ _ _ _ _ _ _ _ _ _ _ _ _ _ _ _ _ _ _ _ _ _ _ _ _ _ _ _ _ _ _ _ _ _ _ _ _ _ _ _ _ _ _ _ _ _ _ _ _ _ _ _ _ _ _ _ _ _ _ _ _ _ _ _ _ _ _ _ _ _ _ _ _ _ _ _ _ _ _ _ _ _]
      tunnel: w44 -> [_ w563 _ _ _ _ _ _ _ _ _ _ _ _ _ _ _ _ _ _ _ _ _ _ _ _ _ _ _ _ _ _ _ _ _ _ _ _ _ _ _ _ _ _ _ _ _ _ _ _ _ _ _ _ _ _ _ _ _ w1576 _ _ _ _ _ _ w1813 w1832 w1851 w1881 w1899 w1918 w1932 w1957 w1969 w2001 _ _ _ _ _ _ _ _ _ _ _ _ _ _ _ _ _ _ _ _ _ _ _ _ _ _ _ _ _ _ _ _ _ _ _ _ _ _ _ _ _ _ _ _ _ _ _ _ _]
      tunnel: w43 -> [_ w562 _ _ _ _ _ _ _ _ _ _ _ _ _ _ _ _ _ _ _ _ _ _ _ _ _ _ _ _ _ _ _ _ _ _ _ _ _ _ _ _ _ _ _ _ _ _ _ _ _ _ _ _ _ _ _ _ _ w1575 _ _ _ _ _ _ w1812 w1831 w1850 w1880 w1898 w1917 w1938 w1956 _ _ _ _ _ _ _ _ _ _ _ _ _ _ _ _ _ _ _ _ _ _ _ _ _ _ _ _ _ _ _ _ _ _ _ _ _ _ _ _ _ _ _ _ _ _ _ _ _ _ w2565]
      tunnel: w42 -> [_ w561 _ w603 w655 w668 w671 w674 w677 w702 w716 w719 w722 w724 w749 w761 w787 w801 w804 w807 w810 w834 w841 w851 w864 w888 w901 w925 w939 w953 w956 w959 w962 w987 w1001 w1004 w1007 w1010 _ _ _ _ _ _ _ w1373 w1379 w1385 w1391 w1397 w1403 w1409 w1415 w1426 w1453 w1477 w1499 w1527 w1551 w1569 w1599 w1625 w1665 w1691 w1723 w1768 w1811 w1828 w1847 w1877 w1895 w1914 w1935 w1952 w1970 w2002 w2033 w2069 w2094 w2118 w2143 w2155 w2163 w2171 w2173 w2188 w2190 w2193 w2203 w2220 w2239 w2275 w2278 w2281 w2284 w2288 _ w2294 w2305 w2318 w2322 w2325 w2361 w2373 w2392 w2395 w2403 w2415 w2419 w2425 w2431 w2443 w2467 w2489 w2497 w2504 w2510 w2516 w2519 w2522 w2528 w2531 w2537 w2544 w2562]
      tunnel: w39 -> [_ _ _ _ _ _ _ _ _ _ _ _ _ _ _ _ _ _ _ _ _ _ _ _ _ _ _ _ _ _ _ _ _ _ _ _ _ _ _ _ _ _ _ _ _ _ _ _ _ _ _ _ _ _ _ _ _ _ _ _ _ _ _ _ _ _ _ _ _ _ _ _ _ _ _ _ _ _ _ _ _ _ _ _ _ _ _ _ _ _ _ _ _ _ _ _ _ _ _ _ _ _ _ _ _ _ _ _ _ _ _ _ _ _ _ _ _ _ _ _ _ _ _ _ w2548]
      tunnel: w35 -> [_ _ _ _ _ _ _ _ _ _ _ _ _ _ _ _ _ _ _ _ _ _ _ _ _ _ _ _ _ _ _ _ _ _ _ _ _ _ _ _ _ _ _ _ _ _ _ _ _ _ _ _ _ _ _ _ _ _ _ _ _ _ _ _ _ _ _ _ _ _ _ _ _ _ _ _ _ _ _ _ _ _ _ _ _ _ _ _ _ _ _ _ _ _ _ _ _ _ _ _ _ _ _ _ _ _ _ _ _ _ _ _ _ _ _ _ _ _ _ _ _ _ _ _ w2546]
      tunnel: w34 -> [_ _ w592 _ _ _ _ _ _ _ _ _ _ _ _ _ _ _ _ _ _ _ _ _ _ _ _ _ _ _ _ _ _ _ _ _ _ _ _ _ _ _ _ _ _ _ _ _ _ _ _ _ _ _ _ _ _ _ _ _ _ _ _ _ _ _ _ _ _ _ _ _ _ _ _ _ _ _ _ _ _ _ _ _ _ _ _ _ _ _ _ _ _ _ _ _ _ _ _ _ _ _ _ _ _ _ _ _ _ _ _ _ _ _ _ _ _ _ _ _ _ _ _ _ _]
      event Timeout {
        n37 = event-data() -> ()  [unwired: 3 out]
      }
      event "Update": Value Change {
        n38 = event-data() -> ("CtlRef"=w567:refnum<vi>)  [unwired: 6 out]
        n39 = property class="Bool (strict)"(reference=w567, "Value"=FALSE) -> ()  [unwired: 1 in, 2 out]
        n40 = property on="Stop Amp3" class="DigNum (strict)"() -> ("Value"=w576:dbl)  [unwired: 2 in, 2 out]
        n41 = property on="Start Amp3" class="DigNum (strict)"() -> ("Value"=w577:dbl)  [unwired: 2 in, 2 out]
        n42 = property on="unit3" class="Ring (strict)"() -> ("Value"=w575:u16)  [unwired: 2 in, 2 out]
        n43 = case shown="0, Default" w575 {
          tunnel: w563 -> [w584 _]
          tunnel: w562 -> [w585 _]
          tunnel: [w582 w586] -> w572
          tunnel: w576 -> [w583 w586]
          frame 0, Default {
            n44 = call "CRYConversion dB-Lin.vi"("unit prefix"=w585, "dB ref."=w584, "Lin In"=w583) -> ("Log Out"=w582:dbl)  [unwired: 3 in, 3 out]
          }
          frame 1 {
          }
        }
        n45 = case shown="0, Default" w575 {
          tunnel: w563 -> [w589 _]
          tunnel: w562 -> [w590 _]
          tunnel: [w587 w591] -> w571
          tunnel: w577 -> [w588 w591]
          frame 0, Default {
            n46 = call "CRYConversion dB-Lin.vi"("unit prefix"=w590, "dB ref."=w589, "Lin In"=w588) -> ("Log Out"=w587:dbl)  [unwired: 3 in, 3 out]
          }
          frame 1 {
          }
        }
        n47 = property on="Steps3" class="DigNum (strict)"() -> ("Value"=w574:i32)  [unwired: 2 in, 2 out]
        n48 = Subtract(x=w572, y=w571) -> (x-y=w569:dbl)
        n49 = Decrement(x=w574) -> (x-1=w570:i32)
        n50 = Absolute Value(x=w569) -> (abs(x)=w568:dbl)
        n51 = Less Or Equal To 0?(x=w570) -> (x <= 0?=w573:bool)
        n52 = case shown="False" w573 {
          tunnel: w568 -> [w580 _]
          tunnel: w570 -> [w579 _]
          tunnel: [w578 0.0] -> w564
          frame False {
            n53 = Divide(x=w580, y=w579) -> (x/y=w578:dbl)
          }
          frame True {
          }
        }
        n54 = property on="Step Size3" class="DigNum (strict)"("Value"=w564) -> ()  [unwired: 2 in, 2 out]
        n55 = Bundle By Name(cluster=w561, "StepSize3"=w564) -> (w565:T2)
        n56 = property on="Stimulus Out" class="Clust (strict)"("Val(Sgnl)"=w565) -> ()  [unwired: 2 in, 2 out]
      }
      event "CurLibChange": Value Change {
        n57 = event-data() -> ()  [unwired: 7 out]
        n58 = call "CRYGet Upper Step Data.vi"("Type In"=enum16{"Curves", "Values", "Results", "WFM"}."Values", "No.VI"=w592) -> ("Value array"=w594:T5)  [unwired: 9 out]
        n59 = for {
          tunnel: w594 -> [w600] mode=indexing
          tunnel: [w599] -> w593 mode=indexing
          n60 = Unbundle By Name(w600) -> ("Name"=w599:string)
        }
        n61 = call "CRYGet Curve Library Data Name.vi"("sAction"="GetNameByType", "Type"=enum16{"Curves", "Values", "Results", "WFM"}."Values") -> ("sNames"=w596:string[])  [unwired: 6 in, 3 out]
        n62 = property on="StartFreq1_CurLib" class="Ring (strict)"("Strings []"=w596) -> ()  [unwired: 2 in, 2 out]
        n63 = property on="StopFreq1_CurLib" class="Ring (strict)"("Strings []"=w596) -> ()  [unwired: 2 in, 2 out]
        n64 = property on="StartFreq2_CurLib" class="Ring (strict)"("Strings []"=w596) -> ()  [unwired: 2 in, 2 out]
        n65 = property on="StopFreq2_CurLib" class="Ring (strict)"("Strings []"=w596) -> ()  [unwired: 2 in, 2 out]
        n66 = property on="StartFreq6_CurLib" class="Ring (strict)"("Strings []"=w596) -> ()  [unwired: 2 in, 2 out]
        n67 = property on="StopFreq6_CurLib" class="Ring (strict)"("Strings []"=w596) -> ()  [unwired: 2 in, 2 out]
        n68 = property on="StartFreq7_CurLib" class="Ring (strict)"("Strings []"=w596) -> ()  [unwired: 2 in, 2 out]
        n69 = property on="StopFreq7_CurLib" class="Ring (strict)"("Strings []"=w596) -> ()  [unwired: 2 in, 2 out]
        n70 = property on="StartFreq8_CurLib" class="Ring (strict)"("Strings []"=w596) -> ()  [unwired: 2 in, 2 out]
        n71 = property on="StopFreq8_CurLib" class="Ring (strict)"("Strings []"=w596) -> ()  [unwired: 2 in, 2 out]
        n72 = property on="ML val level name3" class="Ring (strict)"("Strings []"=w593) -> ()  [unwired: 2 in, 2 out]
        n73 = property on="ML val level name4" class="Ring (strict)"("Strings []"=w593) -> ()  [unwired: 2 in, 2 out]
        n74 = property on="ML val level name6_1" class="Ring (strict)"("Strings []"=w593) -> ()  [unwired: 2 in, 2 out]
        n75 = property on="ML val level name6_2" class="Ring (strict)"("Strings []"=w593) -> ()  [unwired: 2 in, 2 out]
        n76 = property on="ML val level name7" class="Ring (strict)"("Strings []"=w593) -> ()  [unwired: 2 in, 2 out]
        n77 = property on="ML val level name8" class="Ring (strict)"("Strings []"=w593) -> ()  [unwired: 2 in, 2 out]
        n78 = property on="ML val level name" class="Ring (strict)"("Strings []"=w593) -> ()  [unwired: 2 in, 2 out]
        n79 = property on="ML val level name2" class="Ring (strict)"("Strings []"=w593) -> ()  [unwired: 2 in, 2 out]
      }
      event "Stimulus Type": Value Change {
        n80 = event-data() -> ("NewVal"=w602:u16)  [unwired: 6 out]
        n81 = property on="Stimulus Type" class="Ring (strict)"() -> ("RingText.Text"=w604:string)  [unwired: 2 in, 2 out]
        n82 = case shown="3" w602 {
          tunnel: [T1."Page1" ("Tab Control") T1."Page2" ("Tab Control") T1."Page3" ("Tab Control") T1."Page4" ("Tab Control") T1."Page5" ("Tab Control") T1."Page6" ("Tab Control") T1."Page7" ("Tab Control") T1."Page8" ("Tab Control")] -> w606
          frame 0, Default {
            n83 = property on="UseMLVal_Level_1" class="Slide (strict)"() -> ("Value"=w628:u16)  [unwired: 2 in, 2 out]
            n84 = property on="Step Resolution1" class="Ring (strict)"() -> ("Value"=w627:u16)  [unwired: 2 in, 2 out]
            n85 = property on="UseMLVal_Level_1" class="Slide (strict)"("Val(Sgnl)"=w628) -> ()  [unwired: 2 in, 2 out]
            n86 = property on="Step Resolution1" class="Ring (strict)"("Val(Sgnl)"=w627) -> ()  [unwired: 2 in, 2 out]
          }
          frame 1 {
            n87 = property on="UseMLVal_Level_2" class="Slide (strict)"() -> ("Value"=w630:u16)  [unwired: 2 in, 2 out]
            n88 = property on="UseMLVal_Level_2" class="Slide (strict)"("Val(Sgnl)"=w630) -> ()  [unwired: 2 in, 2 out]
          }
          frame 2 {
            n89 = property on="UseMLVal_Level_3" class="Slide (strict)"() -> ("Value"=w632:u16)  [unwired: 2 in, 2 out]
            n90 = property on="UseMLVal_Level_3" class="Slide (strict)"("Val(Sgnl)"=w632) -> ()  [unwired: 2 in, 2 out]
          }
          frame 3 {
            n91 = property on="Wave Path4" class="Path"() -> ("Value"=w634:path)  [unwired: 2 in, 2 out]
            n92 = property on="UseMLVal_Level_4" class="Slide (strict)"() -> ("Value"=w635:u16)  [unwired: 2 in, 2 out]
            n93 = property on="Wave Path4" class="Path"("Val(Sgnl)"=w634) -> ()  [unwired: 2 in, 2 out]
            n94 = property on="UseMLVal_Level_4" class="Slide (strict)"("Val(Sgnl)"=w635) -> ()  [unwired: 2 in, 2 out]
          }
          frame 4 {
            n95 = property on="dc_ctrl5_2" class="Slide (strict)"() -> ("Value"=w637:u16)  [unwired: 2 in, 2 out]
            n96 = property on="dc_ctrl5_1" class="Slide (strict)"() -> ("Value"=w638:u16)  [unwired: 2 in, 2 out]
            n97 = property on="dc_ctrl5_1" class="Slide (strict)"("Val(Sgnl)"=w638) -> ()  [unwired: 2 in, 2 out]
            n98 = property on="dc_ctrl5_2" class="Slide (strict)"("Val(Sgnl)"=w637) -> ()  [unwired: 2 in, 2 out]
          }
          frame 5 {
            n99 = property on="Sweep Type" class="Slide (strict)"() -> ("Value"=w644:u16)  [unwired: 2 in, 2 out]
            n100 = property on="Control6 Tab" class="TabCtl (strict)"() -> ("Value"=w643:enum32{"Master Tone", "Slave Tone"})  [unwired: 2 in, 2 out]
            n101 = property on="UseMLVal_Level6_2" class="Slide (strict)"() -> ("Value"=w642:u16)  [unwired: 2 in, 2 out]
            n102 = property on="UseMLVal_Level6_1" class="Slide (strict)"() -> ("Value"=w641:u16)  [unwired: 2 in, 2 out]
            n103 = property on="StepResolution6" class="Ring (strict)"() -> ("Value"=w640:u16)  [unwired: 2 in, 2 out]
            n104 = property on="Sweep Type" class="Slide (strict)"("Val(Sgnl)"=w644) -> ()  [unwired: 2 in, 2 out]
            n105 = property on="Control6 Tab" class="TabCtl (strict)"("Val(Sgnl)"=w643) -> ()  [unwired: 2 in, 2 out]
            n106 = property on="UseMLVal_Level6_2" class="Slide (strict)"("Val(Sgnl)"=w642) -> ()  [unwired: 2 in, 2 out]
            n107 = property on="UseMLVal_Level6_1" class="Slide (strict)"("Val(Sgnl)"=w641) -> ()  [unwired: 2 in, 2 out]
            n108 = property on="StepResolution6" class="Ring (strict)"("Val(Sgnl)"=w640) -> ()  [unwired: 2 in, 2 out]
          }
          frame 6 {
            n109 = property on="Noise Type7" class="Slide (strict)"() -> ("Value"=w647:u16)  [unwired: 2 in, 2 out]
            n110 = property on="UseMLVal_Level_7" class="Slide (strict)"() -> ("Value"=w646:u16)  [unwired: 2 in, 2 out]
            n111 = property on="Noise Type7" class="Slide (strict)"("Val(Sgnl)"=w647) -> ()  [unwired: 2 in, 2 out]
            n112 = property on="UseMLVal_Level_7" class="Slide (strict)"("Val(Sgnl)"=w646) -> ()  [unwired: 2 in, 2 out]
          }
          frame 7 {
            n113 = property on="Freq Rounding8" class="Bool (strict)"() -> ("Value"=w650:bool)  [unwired: 2 in, 2 out]
            n114 = property on="UseMLVal_Level_8" class="Slide (strict)"() -> ("Value"=w651:u16)  [unwired: 2 in, 2 out]
            n115 = property on="Step Resolution8" class="Ring (strict)"() -> ("Value"=w649:u16)  [unwired: 2 in, 2 out]
            n116 = property on="Freq Rounding8" class="Bool (strict)"("Val(Sgnl)"=w650) -> ()  [unwired: 2 in, 2 out]
            n117 = property on="UseMLVal_Level_8" class="Slide (strict)"("Val(Sgnl)"=w651) -> ()  [unwired: 2 in, 2 out]
            n118 = property on="Step Resolution8" class="Ring (strict)"("Val(Sgnl)"=w649) -> ()  [unwired: 2 in, 2 out]
          }
        }
        n119 = Increment(x=w602) -> (x+1=w601:u16)
        n120 = Bundle By Name(cluster=w603, "StimulusType"=w604) -> (w605:T2)
        n121 = property on="Stimulus Out" class="Clust (strict)"("Val(Sgnl)"=w605) -> ()  [unwired: 2 in, 2 out]
        n122 = property on="Control Tab" class="TabCtl (strict)"("Value"=w606) -> ()  [unwired: 2 in, 2 out]
        n123 = case shown="1, 2, 6..8" w601 {
          selector: w601 -> [_ w607]
          frame Default {
          }
          frame 1, 2, 6..8 {
            n124 = Number To Decimal String(number=w607) -> (decimal integer string=w622:string)  [unwired: 1 in]
            n125 = Concatenate Strings("StopFreq" ("string"), w622) -> (w609:string)
            n126 = Concatenate Strings("StartFreq" ("string"), w622) -> (w621:string)
            n127 = Concatenate Strings(w609, "_Flag" ("string")) -> (w608:string)
            n128 = Concatenate Strings(w621, "_Flag" ("string")) -> (w618:string)
            n129 = invoke class="VI" method="Ctrl Val.Get"("Control Name"=w608) -> ("Get Control Value Variant"=w612:variant)  [unwired: 3 in, 3 out]
            n130 = invoke class="VI" method="Ctrl Val.Get"("Control Name"=w618) -> ("Get Control Value Variant"=w617:variant)  [unwired: 3 in, 3 out]
            n131 = Variant To Data(type="" ("string"), Variant=w612) -> (data=w614:string)  [unwired: 1 in, 1 out]
            n132 = Variant To Data(type="" ("string"), Variant=w617) -> (data=w615:string)  [unwired: 1 in, 1 out]
            n133 = Concatenate Strings(w609, "###" ("string"), w614) -> (w611:string)
            n134 = Concatenate Strings(w621, "###" ("string"), w615) -> (w625:string)
            n135 = property on="StartStopFreqValue" class="Str"("Val(Sgnl)"=w611) -> ()  [unwired: 2 in, 2 out]
            n136 = property on="StartStopFreqValue" class="Str"("Val(Sgnl)"=w625) -> ()  [unwired: 2 in, 2 out]
          }
        }
      }
      event "UseMLVal_Level_1": Value Change {
        n137 = event-data() -> ("NewVal"=w658:u16)  [unwired: 6 out]
        n138 = case shown="0, Default" w658 {
          tunnel: [TRUE ("Visible") FALSE ("Visible")] -> w653
          tunnel: [FALSE ("Visible") TRUE ("Visible")] -> w654
          frame 0, Default {
            n139 = property on="Level(U)1" class="DigNum (strict)"() -> ("Value"=w661:dbl)  [unwired: 2 in, 2 out]
            n140 = property on="Level(U)1" class="DigNum (strict)"("Val(Sgnl)"=w661) -> ()  [unwired: 2 in, 2 out]
          }
          frame 1 {
            n141 = property on="ML axis1" class="Slide (strict)"() -> ("Value"=w664:u16)  [unwired: 2 in, 2 out]
            n142 = property on="ML axis1" class="Slide (strict)"("Val(Sgnl)"=w664) -> ()  [unwired: 2 in, 2 out]
          }
        }
        n143 = Build Array(w658) -> (w657:u16[])
        n144 = Bundle By Name(cluster=w655, "UseMLValArray"=w657) -> (w656:T2)
        n145 = property on="Level(U)1" class="DigNum (strict)"("Visible"=w653) -> ()  [unwired: 2 in, 2 out]
        n146 = property on="unit1" class="Ring (strict)"("Visible"=w653) -> ()  [unwired: 2 in, 2 out]
        n147 = property on="ML val level name" class="Ring (strict)"("Visible"=w654) -> ()  [unwired: 2 in, 2 out]
        n148 = property on="deg1" class="DigNum (strict)"("Visible"=w654) -> ()  [unwired: 2 in, 2 out]
        n149 = property on="ML axis1" class="Slide (strict)"("Visible"=w654) -> ()  [unwired: 2 in, 2 out]
        n150 = property on="Stimulus Out" class="Clust (strict)"("Val(Sgnl)"=w656) -> ()  [unwired: 2 in, 2 out]
        n151 = property on="V on DUT1" class="Bool (strict)"("Visible"=w653) -> ()  [unwired: 2 in, 2 out]
        n152 = case shown="False" w653 {
          selector: w653 -> [w659 _]
          frame False {
            n153 = property on="Output Imp1" class="Ring (strict)"("Visible"=w659) -> ()  [unwired: 2 in, 2 out]
            n154 = property on="Nominal Imp1" class="DigNum (strict)"("Visible"=w659) -> ()  [unwired: 2 in, 2 out]
          }
          frame True {
            n155 = property on="V on DUT1" class="Bool (strict)"() -> ("Value"=w660:bool)  [unwired: 2 in, 2 out]
            n156 = property on="V on DUT1" class="Bool (strict)"("Val(Sgnl)"=w660) -> ()  [unwired: 2 in, 2 out]
          }
        }
      }
      event "V on DUT1": Value Change {
        n157 = event-data() -> ("NewVal"=w667:bool)  [unwired: 6 out]
        n158 = Bundle By Name(cluster=w668, "V on DUT"=w667) -> (w669:T2)
        n159 = property on="Output Imp1" class="Ring (strict)"("Visible"=w667) -> ()  [unwired: 2 in, 2 out]
        n160 = property on="Nominal Imp1" class="DigNum (strict)"("Visible"=w667) -> ()  [unwired: 2 in, 2 out]
        n161 = property on="Stimulus Out" class="Clust (strict)"("Val(Sgnl)"=w669) -> ()  [unwired: 2 in, 2 out]
      }
      event "Output Imp1": Value Change {
        n162 = event-data() -> ("NewVal"=w670:u16)  [unwired: 6 out]
        n163 = Bundle By Name(cluster=w671, "Output Imp"=w670) -> (w672:T2)
        n164 = property on="Stimulus Out" class="Clust (strict)"("Val(Sgnl)"=w672) -> ()  [unwired: 2 in, 2 out]
      }
      event "Nominal Imp1": Value Change {
        n165 = event-data() -> ("NewVal"=w673:dbl)  [unwired: 6 out]
        n166 = Bundle By Name(cluster=w674, "Nominal Imp"=w673) -> (w675:T2)
        n167 = property on="Stimulus Out" class="Clust (strict)"("Val(Sgnl)"=w675) -> ()  [unwired: 2 in, 2 out]
      }
      event "ML axis1": Value Change {
        n168 = event-data() -> ("NewVal"=w689:u16)  [unwired: 6 out]
        n169 = property on="ML val level name" class="Ring (strict)"() -> ("Value"=w685:u16)  [unwired: 2 in, 2 out]
        n170 = Index Array(array=w678, index=w685) -> (element=w676:T6)
        n171 = Unbundle By Name(w676) -> ("Curve"=w686:cluster{"x":dbl, "y":dbl, "z":dbl}[], "X unit"=w683:string, "Y unit"=w682:string, "Z unit"=w681:string)
        n172 = Index Array(array=w686) -> (element=w684:cluster{"x":dbl, "y":dbl, "z":dbl})  [unwired: 1 in]
        n173 = case shown="0, Default" w689 {
          tunnel: w684 -> [w694 w697 w700]
          tunnel: w683 -> [w692 _ _]
          tunnel: w682 -> [_ w696 _]
          tunnel: w681 -> [_ _ w699]
          tunnel: [w692 w696 w699] -> w679
          tunnel: [w693 w695 w698] -> w680
          frame 0, Default {
            n174 = Unbundle By Name(w694) -> ("x"=w693:dbl)
          }
          frame 1 {
            n175 = Unbundle By Name(w697) -> ("y"=w695:dbl)
            n176 = property on="LinLevel1" class="DigNum (strict)"("Value"=w695) -> ()  [unwired: 2 in, 2 out]
          }
          frame 2 {
            n177 = Unbundle By Name(w700) -> ("z"=w698:dbl)
          }
        }
        n178 = property on="deg1" class="DigNum (strict)"("Caption.Text"=w679) -> ()  [unwired: 2 in, 2 out]
        n179 = property on="deg1" class="DigNum (strict)"("Value"=w680) -> ()  [unwired: 2 in, 2 out]
        n180 = Build Array(w689) -> (w691:u16[])
        n181 = Build Array(w680) -> (w688:dbl[])
        n182 = Build Array(w679) -> (w687:string[])
        n183 = Bundle By Name(cluster=w677, "ML_axisArray"=w691, "DegValArray"=w688, "DegUnitArray"=w687) -> (w690:T2)
        n184 = property on="Stimulus Out" class="Clust (strict)"("Val(Sgnl)"=w690) -> ()  [unwired: 2 in, 2 out]
      }
      event "UseMLVal_Level_2": Value Change {
        n185 = event-data() -> ("NewVal"=w703:u16)  [unwired: 6 out]
        n186 = Build Array(w703) -> (w705:u16[])
        n187 = case shown="0, Default" w703 {
          tunnel: [TRUE ("Visible") FALSE ("Visible")] -> w701
          tunnel: [FALSE ("Visible") TRUE ("Visible")] -> w706
          frame 0, Default {
            n188 = property on="Level(U)2" class="DigNum (strict)"() -> ("Value"=w709:dbl)  [unwired: 2 in, 2 out]
            n189 = property on="Level(U)2" class="DigNum (strict)"("Val(Sgnl)"=w709) -> ()  [unwired: 2 in, 2 out]
          }
          frame 1 {
            n190 = property on="ML axis2" class="Slide (strict)"() -> ("Value"=w712:u16)  [unwired: 2 in, 2 out]
            n191 = property on="ML axis2" class="Slide (strict)"("Val(Sgnl)"=w712) -> ()  [unwired: 2 in, 2 out]
          }
        }
        n192 = Bundle By Name(cluster=w702, "UseMLValArray"=w705) -> (w704:T2)
        n193 = property on="Stimulus Out" class="Clust (strict)"("Val(Sgnl)"=w704) -> ()  [unwired: 2 in, 2 out]
        n194 = property on="Level(U)2" class="DigNum (strict)"("Visible"=w701) -> ()  [unwired: 2 in, 2 out]
        n195 = property on="unit2" class="Ring (strict)"("Visible"=w701) -> ()  [unwired: 2 in, 2 out]
        n196 = property on="ML val level name2" class="Ring (strict)"("Visible"=w706) -> ()  [unwired: 2 in, 2 out]
        n197 = property on="deg2" class="DigNum (strict)"("Visible"=w706) -> ()  [unwired: 2 in, 2 out]
        n198 = property on="ML axis2" class="Slide (strict)"("Visible"=w706) -> ()  [unwired: 2 in, 2 out]
        n199 = property on="V on DUT2" class="Bool (strict)"("Visible"=w701) -> ()  [unwired: 2 in, 2 out]
        n200 = case shown="False" w701 {
          selector: w701 -> [w707 _]
          frame False {
            n201 = property on="Output Imp2" class="Ring (strict)"("Visible"=w707) -> ()  [unwired: 2 in, 2 out]
            n202 = property on="Nominal Imp2" class="DigNum (strict)"("Visible"=w707) -> ()  [unwired: 2 in, 2 out]
          }
          frame True {
            n203 = property on="V on DUT2" class="Bool (strict)"() -> ("Value"=w708:bool)  [unwired: 2 in, 2 out]
            n204 = property on="V on DUT2" class="Bool (strict)"("Val(Sgnl)"=w708) -> ()  [unwired: 2 in, 2 out]
          }
        }
      }
      event "V on DUT2": Value Change {
        n205 = event-data() -> ("NewVal"=w715:bool)  [unwired: 6 out]
        n206 = Bundle By Name(cluster=w716, "V on DUT"=w715) -> (w717:T2)
        n207 = property on="Output Imp2" class="Ring (strict)"("Visible"=w715) -> ()  [unwired: 2 in, 2 out]
        n208 = property on="Stimulus Out" class="Clust (strict)"("Val(Sgnl)"=w717) -> ()  [unwired: 2 in, 2 out]
        n209 = property on="Nominal Imp2" class="DigNum (strict)"("Visible"=w715) -> ()  [unwired: 2 in, 2 out]
      }
      event "Output Imp2": Value Change {
        n210 = event-data() -> ("NewVal"=w718:u16)  [unwired: 6 out]
        n211 = Bundle By Name(cluster=w719, "Output Imp"=w718) -> (w720:T2)
        n212 = property on="Stimulus Out" class="Clust (strict)"("Val(Sgnl)"=w720) -> ()  [unwired: 2 in, 2 out]
      }
      event "Nominal Imp2": Value Change {
        n213 = event-data() -> ("NewVal"=w721:dbl)  [unwired: 6 out]
        n214 = Bundle By Name(cluster=w722, "Nominal Imp"=w721) -> (w723:T2)
        n215 = property on="Stimulus Out" class="Clust (strict)"("Val(Sgnl)"=w723) -> ()  [unwired: 2 in, 2 out]
      }
      event "ML axis2": Value Change {
        n216 = event-data() -> ("NewVal"=w729:u16)  [unwired: 6 out]
        n217 = property on="ML val level name2" class="Ring (strict)"() -> ("Value"=w725:u16)  [unwired: 2 in, 2 out]
        n218 = Index Array(array=w728, index=w725) -> (element=w734:T6)
        n219 = Unbundle By Name(w734) -> ("Curve"=w735:cluster{"x":dbl, "y":dbl, "z":dbl}[], "X unit"=w732:string, "Y unit"=w731:string, "Z unit"=w730:string)
        n220 = Index Array(array=w735) -> (element=w733:cluster{"x":dbl, "y":dbl, "z":dbl})  [unwired: 1 in]
        n221 = case shown="1" w729 {
          tunnel: w733 -> [w742 w745 w748]
          tunnel: w732 -> [w741 _ _]
          tunnel: w731 -> [_ w744 _]
          tunnel: w730 -> [_ _ w747]
          tunnel: [w741 w744 w747] -> w726
          tunnel: [w740 w743 w746] -> w727
          frame 0, Default {
            n222 = Unbundle By Name(w742) -> ("x"=w740:dbl)
          }
          frame 1 {
            n223 = Unbundle By Name(w745) -> ("y"=w743:dbl)
            n224 = property on="LinLevel1" class="DigNum (strict)"("Value"=w743) -> ()  [unwired: 2 in, 2 out]
          }
          frame 2 {
            n225 = Unbundle By Name(w748) -> ("z"=w746:dbl)
          }
        }
        n226 = property on="deg2" class="DigNum (strict)"("Caption.Text"=w726) -> ()  [unwired: 2 in, 2 out]
        n227 = property on="deg2" class="DigNum (strict)"("Value"=w727) -> ()  [unwired: 2 in, 2 out]
        n228 = Build Array(w729) -> (w739:u16[])
        n229 = Build Array(w727) -> (w737:dbl[])
        n230 = Build Array(w726) -> (w736:string[])
        n231 = Bundle By Name(cluster=w724, "ML_axisArray"=w739, "DegValArray"=w737, "DegUnitArray"=w736) -> (w738:T2)
        n232 = property on="Stimulus Out" class="Clust (strict)"("Val(Sgnl)"=w738) -> ()  [unwired: 2 in, 2 out]
      }
      event "UseMLVal_Level_3": Value Change {
        n233 = event-data() -> ("NewVal"=w750:u16)  [unwired: 6 out]
        n234 = case shown="0, Default" w750 {
          tunnel: [TRUE ("Visible") FALSE ("Visible")] -> w754
          tunnel: [FALSE ("Visible") TRUE ("Visible")] -> w753
          frame 0, Default {
            n235 = property on="Freq3(Hz)" class="DigNum (strict)"() -> ("Value"=w755:dbl)  [unwired: 2 in, 2 out]
            n236 = property on="Freq3(Hz)" class="DigNum (strict)"("Val(Sgnl)"=w755) -> ()  [unwired: 2 in, 2 out]
          }
          frame 1 {
            n237 = property on="ML axis3" class="Slide (strict)"() -> ("Value"=w758:u16)  [unwired: 2 in, 2 out]
            n238 = property on="ML axis3" class="Slide (strict)"("Val(Sgnl)"=w758) -> ()  [unwired: 2 in, 2 out]
          }
        }
        n239 = Build Array(w750) -> (w752:u16[])
        n240 = Bundle By Name(cluster=w749, "UseMLValArray"=w752) -> (w751:T2)
        n241 = property on="Freq3(Hz)" class="DigNum (strict)"("Visible"=w754) -> ()  [unwired: 2 in, 2 out]
        n242 = property on="ML val level name3" class="Ring (strict)"("Visible"=w753) -> ()  [unwired: 2 in, 2 out]
        n243 = property on="deg3" class="DigNum (strict)"("Visible"=w753) -> ()  [unwired: 2 in, 2 out]
        n244 = property on="ML axis3" class="Slide (strict)"("Visible"=w753) -> ()  [unwired: 2 in, 2 out]
        n245 = property on="Stimulus Out" class="Clust (strict)"("Val(Sgnl)"=w751) -> ()  [unwired: 2 in, 2 out]
      }
      event "ML axis3": Value Change {
        n246 = event-data() -> ("NewVal"=w765:u16)  [unwired: 6 out]
        n247 = property on="ML val level name3" class="Ring (strict)"() -> ("Value"=w762:u16)  [unwired: 2 in, 2 out]
        n248 = Index Array(array=w766, index=w762) -> (element=w771:T6)
        n249 = Unbundle By Name(w771) -> ("Curve"=w772:cluster{"x":dbl, "y":dbl, "z":dbl}[], "X unit"=w769:string, "Y unit"=w768:string, "Z unit"=w767:string)
        n250 = Index Array(array=w772) -> (element=w770:cluster{"x":dbl, "y":dbl, "z":dbl})  [unwired: 1 in]
        n251 = case shown="1" w765 {
          tunnel: w770 -> [w779 w782 w785]
          tunnel: w769 -> [w778 _ _]
          tunnel: w768 -> [_ w781 _]
          tunnel: w767 -> [_ _ w784]
          tunnel: [w778 w781 w784] -> w763
          tunnel: [w777 w780 w783] -> w764
          frame 0, Default {
            n252 = Unbundle By Name(w779) -> ("x"=w777:dbl)
          }
          frame 1 {
            n253 = Unbundle By Name(w782) -> ("y"=w780:dbl)
            n254 = local write "RealFreq3(Hz)"(w780) -> ()
          }
          frame 2 {
            n255 = Unbundle By Name(w785) -> ("z"=w783:dbl)
          }
        }
        n256 = property on="deg3" class="DigNum (strict)"("Value"=w764) -> ()  [unwired: 2 in, 2 out]
        n257 = property on="deg3" class="DigNum (strict)"("Caption.Text"=w763) -> ()  [unwired: 2 in, 2 out]
        n258 = Build Array(w765) -> (w776:u16[])
        n259 = Build Array(w764) -> (w774:dbl[])
        n260 = Build Array(w763) -> (w773:string[])
        n261 = Bundle By Name(cluster=w761, "ML_axisArray"=w776, "DegValArray"=w774, "DegUnitArray"=w773) -> (w775:T2)
        n262 = property on="Stimulus Out" class="Clust (strict)"("Val(Sgnl)"=w775) -> ()  [unwired: 2 in, 2 out]
      }
      event "UseMLVal_Level_4": Value Change {
        n263 = event-data() -> ("NewVal"=w788:u16)  [unwired: 6 out]
        n264 = case shown="0, Default" w788 {
          tunnel: [TRUE ("Visible") FALSE ("Visible")] -> w786
          tunnel: [FALSE ("Visible") TRUE ("Visible")] -> w791
          frame 0, Default {
            n265 = property on="Level4(U)" class="DigNum (strict)"() -> ("Value"=w794:dbl)  [unwired: 2 in, 2 out]
            n266 = property on="Level4(U)" class="DigNum (strict)"("Val(Sgnl)"=w794) -> ()  [unwired: 2 in, 2 out]
          }
          frame 1 {
            n267 = property on="ML axis4" class="Slide (strict)"() -> ("Value"=w797:u16)  [unwired: 2 in, 2 out]
            n268 = property on="ML axis4" class="Slide (strict)"("Val(Sgnl)"=w797) -> ()  [unwired: 2 in, 2 out]
          }
        }
        n269 = Build Array(w788) -> (w790:u16[])
        n270 = Bundle By Name(cluster=w787, "UseMLValArray"=w790) -> (w789:T2)
        n271 = property on="Level4(U)" class="DigNum (strict)"("Visible"=w786) -> ()  [unwired: 2 in, 2 out]
        n272 = property on="unit4" class="Ring (strict)"("Visible"=w786) -> ()  [unwired: 2 in, 2 out]
        n273 = property on="ML val level name4" class="Ring (strict)"("Visible"=w791) -> ()  [unwired: 2 in, 2 out]
        n274 = property on="deg4" class="DigNum (strict)"("Visible"=w791) -> ()  [unwired: 2 in, 2 out]
        n275 = property on="ML axis4" class="Slide (strict)"("Visible"=w791) -> ()  [unwired: 2 in, 2 out]
        n276 = property on="Stimulus Out" class="Clust (strict)"("Val(Sgnl)"=w789) -> ()  [unwired: 2 in, 2 out]
        n277 = property on="V on DUT4" class="Bool (strict)"("Visible"=w786) -> ()  [unwired: 2 in, 2 out]
        n278 = case shown="False" w786 {
          selector: w786 -> [w792 _]
          frame False {
            n279 = property on="Output Imp4" class="Ring (strict)"("Visible"=w792) -> ()  [unwired: 2 in, 2 out]
            n280 = property on="Nominal Imp4" class="DigNum (strict)"("Visible"=w792) -> ()  [unwired: 2 in, 2 out]
          }
          frame True {
            n281 = property on="V on DUT4" class="Bool (strict)"() -> ("Value"=w793:bool)  [unwired: 2 in, 2 out]
            n282 = property on="V on DUT4" class="Bool (strict)"("Val(Sgnl)"=w793) -> ()  [unwired: 2 in, 2 out]
          }
        }
      }
      event "V on DUT4": Value Change {
        n283 = event-data() -> ("NewVal"=w800:bool)  [unwired: 6 out]
        n284 = Bundle By Name(cluster=w801, "V on DUT"=w800) -> (w802:T2)
        n285 = property on="Output Imp4" class="Ring (strict)"("Visible"=w800) -> ()  [unwired: 2 in, 2 out]
        n286 = property on="Stimulus Out" class="Clust (strict)"("Val(Sgnl)"=w802) -> ()  [unwired: 2 in, 2 out]
        n287 = property on="Nominal Imp4" class="DigNum (strict)"("Visible"=w800) -> ()  [unwired: 2 in, 2 out]
      }
      event "Output Imp4": Value Change {
        n288 = event-data() -> ("NewVal"=w803:u16)  [unwired: 6 out]
        n289 = Bundle By Name(cluster=w804, "Output Imp"=w803) -> (w805:T2)
        n290 = property on="Stimulus Out" class="Clust (strict)"("Val(Sgnl)"=w805) -> ()  [unwired: 2 in, 2 out]
      }
      event "Nominal Imp4": Value Change {
        n291 = event-data() -> ("NewVal"=w806:dbl)  [unwired: 6 out]
        n292 = Bundle By Name(cluster=w807, "Nominal Imp"=w806) -> (w808:T2)
        n293 = property on="Stimulus Out" class="Clust (strict)"("Val(Sgnl)"=w808) -> ()  [unwired: 2 in, 2 out]
      }
      event "ML axis4": Value Change {
        n294 = event-data() -> ("NewVal"=w813:u16)  [unwired: 6 out]
        n295 = property on="ML val level name4" class="Ring (strict)"() -> ("Value"=w809:u16)  [unwired: 2 in, 2 out]
        n296 = Index Array(array=w814, index=w809) -> (element=w819:T6)
        n297 = Unbundle By Name(w819) -> ("Curve"=w820:cluster{"x":dbl, "y":dbl, "z":dbl}[], "X unit"=w817:string, "Y unit"=w816:string, "Z unit"=w815:string)
        n298 = Index Array(array=w820) -> (element=w818:cluster{"x":dbl, "y":dbl, "z":dbl})  [unwired: 1 in]
        n299 = case shown="1" w813 {
          tunnel: w818 -> [w827 w830 w833]
          tunnel: w817 -> [w826 _ _]
          tunnel: w816 -> [_ w829 _]
          tunnel: w815 -> [_ _ w832]
          tunnel: [w826 w829 w832] -> w811
          tunnel: [w825 w828 w831] -> w812
          frame 0, Default {
            n300 = Unbundle By Name(w827) -> ("x"=w825:dbl)
          }
          frame 1 {
            n301 = Unbundle By Name(w830) -> ("y"=w828:dbl)
            n302 = property on="LinLevel1" class="DigNum (strict)"("Value"=w828) -> ()  [unwired: 2 in, 2 out]
          }
          frame 2 {
            n303 = Unbundle By Name(w833) -> ("z"=w831:dbl)
          }
        }
        n304 = Build Array(w813) -> (w824:u16[])
        n305 = Build Array(w812) -> (w822:dbl[])
        n306 = property on="deg4" class="DigNum (strict)"("Caption.Text"=w811) -> ()  [unwired: 2 in, 2 out]
        n307 = property on="deg4" class="DigNum (strict)"("Value"=w812) -> ()  [unwired: 2 in, 2 out]
        n308 = Build Array(w811) -> (w821:string[])
        n309 = Bundle By Name(cluster=w810, "ML_axisArray"=w824, "DegValArray"=w822, "DegUnitArray"=w821) -> (w823:T2)
        n310 = property on="Stimulus Out" class="Clust (strict)"("Val(Sgnl)"=w823) -> ()  [unwired: 2 in, 2 out]
      }
      event "dc_ctrl5_1": Value Change {
        n311 = event-data() -> ("NewVal"=w835:u16)  [unwired: 6 out]
        n312 = case shown="0, Default" w835 {
          tunnel: [TRUE ("Visible") FALSE ("Visible")] -> w837
          frame 0, Default {
          }
          frame 1 {
          }
        }
        n313 = Bundle By Name(cluster=w834, "dc_ctrl5_1"=w835) -> (w836:T2)
        n314 = property on="Stimulus Out" class="Clust (strict)"("Val(Sgnl)"=w836) -> ()  [unwired: 2 in, 2 out]
        n315 = property on="Level5" class="DigNum (strict)"("Visible"=w837) -> ()  [unwired: 2 in, 2 out]
        n316 = property on="Boolean3" class="Bool (strict)"("Visible"=w837) -> ()  [unwired: 2 in, 2 out]
      }
      event "Sweep Type": Value Change {
        n317 = event-data() -> ("NewVal"=w843:u16)  [unwired: 6 out]
        n318 = Bundle By Name(cluster=w841, "SweepType"=w843) -> (w842:T2)
        n319 = Unbundle By Name(w842) -> ("Fixed/Ratio6"=w840:u16)
        n320 = case shown="1" w843 {
          tunnel: [w846 TRUE ("Visible")] -> w844
          tunnel: [TRUE ("Visible") FALSE ("Visible")] -> w845
          tunnel: w840 -> [_ w848]
          frame 0, Default {
            w846 = FALSE ("Visible")
            n321 = property on="Difference6(Hz)" class="DigNum (strict)"("Visible"=w846) -> ()  [unwired: 2 in, 2 out]
            n322 = property on="Ratio6" class="Ring (strict)"("Visible"=w846) -> ()  [unwired: 2 in, 2 out]
            n323 = property on="Ratio Freq6(Hz)" class="DigNum (strict)"("Visible"=w846) -> ()  [unwired: 2 in, 2 out]
          }
          frame 1 {
            n324 = property on="Fixed/Ratio6" class="Slide (strict)"("Val(Sgnl)"=w848) -> ()  [unwired: 2 in, 2 out]
          }
        }
        n325 = property on="Stimulus Out" class="Clust (strict)"("Val(Sgnl)"=w842) -> ()  [unwired: 2 in, 2 out]
        n326 = property on="Boolean6" class="Bool (strict)"("Visible"=w844) -> ()  [unwired: 2 in, 2 out]
        n327 = property on="Fixed/Ratio6" class="Slide (strict)"("Visible"=w844) -> ()  [unwired: 2 in, 2 out]
        n328 = property on="Freq6(Hz)" class="DigNum (strict)"("Visible"=w845) -> ()  [unwired: 2 in, 2 out]
      }
      event "UseMLVal_Level6_1": Value Change {
        n329 = event-data() -> ("NewVal"=w852:u16)  [unwired: 6 out]
        n330 = case shown="1" w852 {
          tunnel: [TRUE ("Visible") FALSE ("Visible")] -> w856
          tunnel: [FALSE ("Visible") TRUE ("Visible")] -> w855
          frame 0, Default {
            n331 = property on="Level6_1(U)" class="DigNum (strict)"() -> ("Value"=w857:dbl)  [unwired: 2 in, 2 out]
            n332 = property on="Level6_1(U)" class="DigNum (strict)"("Val(Sgnl)"=w857) -> ()  [unwired: 2 in, 2 out]
          }
          frame 1 {
            n333 = property on="ML axis6_1" class="Slide (strict)"() -> ("Value"=w860:u16)  [unwired: 2 in, 2 out]
            n334 = property on="ML axis6_1" class="Slide (strict)"("Val(Sgnl)"=w860) -> ()  [unwired: 2 in, 2 out]
          }
        }
        n335 = Build Array(w852) -> (w854:u16[])
        n336 = Bundle By Name(cluster=w851, "UseMLValArray"=w854) -> (w853:T2)
        n337 = property on="Level6_1(U)" class="DigNum (strict)"("Visible"=w856) -> ()  [unwired: 2 in, 2 out]
        n338 = property on="unit6" class="Ring (strict)"("Visible"=w856) -> ()  [unwired: 2 in, 2 out]
        n339 = property on="ML val level name6_1" class="Ring (strict)"("Visible"=w855) -> ()  [unwired: 2 in, 2 out]
        n340 = property on="deg6" class="DigNum (strict)"("Visible"=w855) -> ()  [unwired: 2 in, 2 out]
        n341 = property on="ML axis6_1" class="Slide (strict)"("Visible"=w855) -> ()  [unwired: 2 in, 2 out]
        n342 = property on="Stimulus Out" class="Clust (strict)"("Val(Sgnl)"=w853) -> ()  [unwired: 2 in, 2 out]
      }
      event "ML axis6_1": Value Change {
        n343 = event-data() -> ("NewVal"=w867:u16)  [unwired: 6 out]
        n344 = property on="ML val level name6_1" class="Ring (strict)"() -> ("Value"=w863:u16)  [unwired: 2 in, 2 out]
        n345 = Index Array(array=w868, index=w863) -> (element=w873:T6)
        n346 = Unbundle By Name(w873) -> ("Curve"=w874:cluster{"x":dbl, "y":dbl, "z":dbl}[], "X unit"=w871:string, "Y unit"=w870:string, "Z unit"=w869:string)
        n347 = Index Array(array=w874) -> (element=w872:cluster{"x":dbl, "y":dbl, "z":dbl})  [unwired: 1 in]
        n348 = case shown="1" w867 {
          tunnel: w872 -> [w881 w884 w887]
          tunnel: w871 -> [w880 _ _]
          tunnel: w870 -> [_ w883 _]
          tunnel: w869 -> [_ _ w886]
          tunnel: [w880 w883 w886] -> w865
          tunnel: [w879 w882 w885] -> w866
          frame 0, Default {
            n349 = Unbundle By Name(w881) -> ("x"=w879:dbl)
          }
          frame 1 {
            n350 = Unbundle By Name(w884) -> ("y"=w882:dbl)
            n351 = property on="LinLevel1" class="DigNum (strict)"("Value"=w882) -> ()  [unwired: 2 in, 2 out]
          }
          frame 2 {
            n352 = Unbundle By Name(w887) -> ("z"=w885:dbl)
          }
        }
        n353 = property on="deg6" class="DigNum (strict)"("Value"=w866) -> ()  [unwired: 2 in, 2 out]
        n354 = property on="deg6" class="DigNum (strict)"("Caption.Text"=w865) -> ()  [unwired: 2 in, 2 out]
        n355 = Build Array(w867) -> (w878:u16[])
        n356 = Build Array(w866) -> (w876:dbl[])
        n357 = Build Array(w865) -> (w875:string[])
        n358 = Bundle By Name(cluster=w864, "ML_axisArray"=w878, "DegValArray"=w876, "DegUnitArray"=w875) -> (w877:T2)
        n359 = property on="Stimulus Out" class="Clust (strict)"("Val(Sgnl)"=w877) -> ()  [unwired: 2 in, 2 out]
      }
      event "UseMLVal_Level6_2": Value Change {
        n360 = event-data() -> ("NewVal"=w889:u16)  [unwired: 6 out]
        n361 = Build Array(w889) -> (w891:u16[])
        n362 = case shown="0, Default" w889 {
          tunnel: [TRUE ("Visible") FALSE ("Visible")] -> w893
          tunnel: [FALSE ("Visible") TRUE ("Visible")] -> w892
          frame 0, Default {
            n363 = property on="Level6_2(U)" class="DigNum (strict)"() -> ("Value"=w894:dbl)  [unwired: 2 in, 2 out]
            n364 = property on="Level6_2(U)" class="DigNum (strict)"("Val(Sgnl)"=w894) -> ()  [unwired: 2 in, 2 out]
          }
          frame 1 {
            n365 = property on="ML axis6_2" class="Slide (strict)"() -> ("Value"=w897:u16)  [unwired: 2 in, 2 out]
            n366 = property on="ML axis6_2" class="Slide (strict)"("Val(Sgnl)"=w897) -> ()  [unwired: 2 in, 2 out]
          }
        }
        n367 = Bundle By Name(cluster=w888, "UseMLValArray"=w891) -> (w890:T2)
        n368 = property on="Stimulus Out" class="Clust (strict)"("Val(Sgnl)"=w890) -> ()  [unwired: 2 in, 2 out]
        n369 = property on="Level6_2(U)" class="DigNum (strict)"("Visible"=w893) -> ()  [unwired: 2 in, 2 out]
        n370 = property on="unit6_1" class="Ring (strict)"("Visible"=w893) -> ()  [unwired: 2 in, 2 out]
        n371 = property on="ML val level name6_2" class="Ring (strict)"("Visible"=w892) -> ()  [unwired: 2 in, 2 out]
        n372 = property on="deg6_1" class="DigNum (strict)"("Visible"=w892) -> ()  [unwired: 2 in, 2 out]
        n373 = property on="ML axis6_2" class="Slide (strict)"("Visible"=w892) -> ()  [unwired: 2 in, 2 out]
      }
      event "ML axis6_2": Value Change {
        n374 = event-data() -> ("NewVal"=w905:u16)  [unwired: 6 out]
        n375 = property on="ML val level name6_2" class="Ring (strict)"() -> ("Value"=w900:u16)  [unwired: 2 in, 2 out]
        n376 = Index Array(array=w904, index=w900) -> (element=w910:T6)
        n377 = Unbundle By Name(w910) -> ("Curve"=w911:cluster{"x":dbl, "y":dbl, "z":dbl}[], "X unit"=w908:string, "Y unit"=w907:string, "Z unit"=w906:string)
        n378 = Index Array(array=w911) -> (element=w909:cluster{"x":dbl, "y":dbl, "z":dbl})  [unwired: 1 in]
        n379 = case shown="1" w905 {
          tunnel: w909 -> [w918 w921 w924]
          tunnel: w908 -> [w917 _ _]
          tunnel: w907 -> [_ w920 _]
          tunnel: w906 -> [_ _ w923]
          tunnel: [w917 w920 w923] -> w902
          tunnel: [w916 w919 w922] -> w903
          frame 0, Default {
            n380 = Unbundle By Name(w918) -> ("x"=w916:dbl)
          }
          frame 1 {
            n381 = Unbundle By Name(w921) -> ("y"=w919:dbl)
            n382 = property on="LinLevel2" class="DigNum (strict)"("Value"=w919) -> ()  [unwired: 2 in, 2 out]
          }
          frame 2 {
            n383 = Unbundle By Name(w924) -> ("z"=w922:dbl)
          }
        }
        n384 = property on="deg6_1" class="DigNum (strict)"("Value"=w903) -> ()  [unwired: 2 in, 2 out]
        n385 = property on="deg6_1" class="DigNum (strict)"("Caption.Text"=w902) -> ()  [unwired: 2 in, 2 out]
        n386 = Build Array(w905) -> (w915:u16[])
        n387 = Build Array(w903) -> (w913:dbl[])
        n388 = Build Array(w902) -> (w912:string[])
        n389 = Bundle By Name(cluster=w901, "ML_axisArray"=w915, "DegValArray"=w913, "DegUnitArray"=w912) -> (w914:T2)
        n390 = property on="Stimulus Out" class="Clust (strict)"("Val(Sgnl)"=w914) -> ()  [unwired: 2 in, 2 out]
      }
      event "Fixed/Ratio6": Value Change {
        n391 = event-data() -> ("NewVal"=w926:u16)  [unwired: 6 out]
        n392 = case shown="0, Default" w926 {
          frame 0, Default {
            w928 = FALSE ("Visible")
            n393 = property on="Difference6(Hz)" class="DigNum (strict)"("Visible"=TRUE) -> ()  [unwired: 2 in, 2 out]
            n394 = property on="Ratio6" class="Ring (strict)"("Visible"=w928) -> ()  [unwired: 2 in, 2 out]
            n395 = property on="Ratio Freq6(Hz)" class="DigNum (strict)"("Visible"=w928) -> ()  [unwired: 2 in, 2 out]
          }
          frame 1 {
            n396 = property on="Ratio6" class="Ring (strict)"() -> ("Value"=w931:u16)  [unwired: 2 in, 2 out]
            n397 = Equal?(x=w931, y=u32 5) -> (x = y?=w932:bool)
            n398 = case shown="False" w932 {
              tunnel: [FALSE ("Visible") TRUE ("Visible")] -> w930
              frame False {
              }
              frame True {
              }
            }
            n399 = property on="Difference6(Hz)" class="DigNum (strict)"("Visible"=FALSE) -> ()  [unwired: 2 in, 2 out]
            n400 = property on="Ratio6" class="Ring (strict)"("Visible"=TRUE) -> ()  [unwired: 2 in, 2 out]
            n401 = property on="Ratio Freq6(Hz)" class="DigNum (strict)"("Visible"=w930) -> ()  [unwired: 2 in, 2 out]
          }
        }
        n402 = Bundle By Name(cluster=w925, "Fixed/Ratio6"=w926) -> (w927:T2)
        n403 = property on="Stimulus Out" class="Clust (strict)"("Val(Sgnl)"=w927) -> ()  [unwired: 2 in, 2 out]
      }
      event "UseMLVal_Level_7": Value Change {
        n404 = event-data() -> ("NewVal"=w940:u16)  [unwired: 6 out]
        n405 = case shown="0, Default" w940 {
          tunnel: [TRUE ("Visible") FALSE ("Visible")] -> w938
          tunnel: [FALSE ("Visible") TRUE ("Visible")] -> w943
          frame 0, Default {
            n406 = property on="Level7(U)" class="DigNum (strict)"() -> ("Value"=w946:dbl)  [unwired: 2 in, 2 out]
            n407 = property on="Level7(U)" class="DigNum (strict)"("Val(Sgnl)"=w946) -> ()  [unwired: 2 in, 2 out]
          }
          frame 1 {
            n408 = property on="ML axis7" class="Slide (strict)"() -> ("Value"=w949:u16)  [unwired: 2 in, 2 out]
            n409 = property on="ML axis7" class="Slide (strict)"("Val(Sgnl)"=w949) -> ()  [unwired: 2 in, 2 out]
          }
        }
        n410 = Build Array(w940) -> (w942:u16[])
        n411 = Bundle By Name(cluster=w939, "UseMLValArray"=w942) -> (w941:T2)
        n412 = property on="Level7(U)" class="DigNum (strict)"("Visible"=w938) -> ()  [unwired: 2 in, 2 out]
        n413 = property on="unit7" class="Ring (strict)"("Visible"=w938) -> ()  [unwired: 2 in, 2 out]
        n414 = property on="ML val level name7" class="Ring (strict)"("Visible"=w943) -> ()  [unwired: 2 in, 2 out]
        n415 = property on="deg7" class="DigNum (strict)"("Visible"=w943) -> ()  [unwired: 2 in, 2 out]
        n416 = property on="ML axis7" class="Slide (strict)"("Visible"=w943) -> ()  [unwired: 2 in, 2 out]
        n417 = property on="Stimulus Out" class="Clust (strict)"("Val(Sgnl)"=w941) -> ()  [unwired: 2 in, 2 out]
        n418 = property on="V on DUT7" class="Bool (strict)"("Visible"=w938) -> ()  [unwired: 2 in, 2 out]
        n419 = case shown="False" w938 {
          selector: w938 -> [w944 _]
          frame False {
            n420 = property on="Output Imp7" class="Ring (strict)"("Visible"=w944) -> ()  [unwired: 2 in, 2 out]
            n421 = property on="Nominal Imp7" class="DigNum (strict)"("Visible"=w944) -> ()  [unwired: 2 in, 2 out]
          }
          frame True {
            n422 = property on="V on DUT7" class="Bool (strict)"() -> ("Value"=w945:bool)  [unwired: 2 in, 2 out]
            n423 = property on="V on DUT7" class="Bool (strict)"("Val(Sgnl)"=w945) -> ()  [unwired: 2 in, 2 out]
          }
        }
      }
      event "V on DUT7": Value Change {
        n424 = event-data() -> ("NewVal"=w952:bool)  [unwired: 6 out]
        n425 = Bundle By Name(cluster=w953, "V on DUT"=w952) -> (w954:T2)
        n426 = property on="Output Imp7" class="Ring (strict)"("Visible"=w952) -> ()  [unwired: 2 in, 2 out]
        n427 = property on="Nominal Imp7" class="DigNum (strict)"("Visible"=w952) -> ()  [unwired: 2 in, 2 out]
        n428 = property on="Stimulus Out" class="Clust (strict)"("Val(Sgnl)"=w954) -> ()  [unwired: 2 in, 2 out]
      }
      event "Output Imp7": Value Change {
        n429 = event-data() -> ("NewVal"=w955:u16)  [unwired: 6 out]
        n430 = Bundle By Name(cluster=w956, "Output Imp"=w955) -> (w957:T2)
        n431 = property on="Stimulus Out" class="Clust (strict)"("Val(Sgnl)"=w957) -> ()  [unwired: 2 in, 2 out]
      }
      event "Nominal Imp7": Value Change {
        n432 = event-data() -> ("NewVal"=w958:dbl)  [unwired: 6 out]
        n433 = Bundle By Name(cluster=w959, "Nominal Imp"=w958) -> (w960:T2)
        n434 = property on="Stimulus Out" class="Clust (strict)"("Val(Sgnl)"=w960) -> ()  [unwired: 2 in, 2 out]
      }
      event "ML axis7": Value Change {
        n435 = event-data() -> ("NewVal"=w966:u16)  [unwired: 6 out]
        n436 = property on="ML val level name7" class="Ring (strict)"() -> ("Value"=w961:u16)  [unwired: 2 in, 2 out]
        n437 = Index Array(array=w965, index=w961) -> (element=w971:T6)
        n438 = Unbundle By Name(w971) -> ("Curve"=w972:cluster{"x":dbl, "y":dbl, "z":dbl}[], "X unit"=w969:string, "Y unit"=w968:string, "Z unit"=w967:string)
        n439 = Index Array(array=w972) -> (element=w970:cluster{"x":dbl, "y":dbl, "z":dbl})  [unwired: 1 in]
        n440 = case shown="1" w966 {
          tunnel: w970 -> [w979 w982 w985]
          tunnel: w969 -> [w978 _ _]
          tunnel: w968 -> [_ w981 _]
          tunnel: w967 -> [_ _ w984]
          tunnel: [w978 w981 w984] -> w963
          tunnel: [w977 w980 w983] -> w964
          frame 0, Default {
            n441 = Unbundle By Name(w979) -> ("x"=w977:dbl)
          }
          frame 1 {
            n442 = Unbundle By Name(w982) -> ("y"=w980:dbl)
            n443 = property on="LinLevel1" class="DigNum (strict)"("Value"=w980) -> ()  [unwired: 2 in, 2 out]
          }
          frame 2 {
            n444 = Unbundle By Name(w985) -> ("z"=w983:dbl)
          }
        }
        n445 = property on="deg7" class="DigNum (strict)"("Caption.Text"=w963) -> ()  [unwired: 2 in, 2 out]
        n446 = property on="deg7" class="DigNum (strict)"("Value"=w964) -> ()  [unwired: 2 in, 2 out]
        n447 = Build Array(w966) -> (w976:u16[])
        n448 = Build Array(w964) -> (w974:dbl[])
        n449 = Build Array(w963) -> (w973:string[])
        n450 = Bundle By Name(cluster=w962, "ML_axisArray"=w976, "DegValArray"=w974, "DegUnitArray"=w973) -> (w975:T2)
        n451 = property on="Stimulus Out" class="Clust (strict)"("Val(Sgnl)"=w975) -> ()  [unwired: 2 in, 2 out]
      }
      event "UseMLVal_Level_8": Value Change {
        n452 = event-data() -> ("NewVal"=w988:u16)  [unwired: 6 out]
        n453 = case shown="0, Default" w988 {
          tunnel: [TRUE ("Visible") FALSE ("Visible")] -> w986
          tunnel: [FALSE ("Visible") TRUE ("Visible")] -> w991
          frame 0, Default {
            n454 = property on="Level8(U)" class="DigNum (strict)"() -> ("Value"=w994:dbl)  [unwired: 2 in, 2 out]
            n455 = property on="Level8(U)" class="DigNum (strict)"("Val(Sgnl)"=w994) -> ()  [unwired: 2 in, 2 out]
          }
          frame 1 {
            n456 = property on="ML axis8" class="Slide (strict)"() -> ("Value"=w997:u16)  [unwired: 2 in, 2 out]
            n457 = property on="ML axis8" class="Slide (strict)"("Val(Sgnl)"=w997) -> ()  [unwired: 2 in, 2 out]
          }
        }
        n458 = Build Array(w988) -> (w990:u16[])
        n459 = Bundle By Name(cluster=w987, "UseMLValArray"=w990) -> (w989:T2)
        n460 = property on="Level8(U)" class="DigNum (strict)"("Visible"=w986) -> ()  [unwired: 2 in, 2 out]
        n461 = property on="unit8" class="Ring (strict)"("Visible"=w986) -> ()  [unwired: 2 in, 2 out]
        n462 = property on="ML val level name8" class="Ring (strict)"("Visible"=w991) -> ()  [unwired: 2 in, 2 out]
        n463 = property on="deg8" class="DigNum (strict)"("Visible"=w991) -> ()  [unwired: 2 in, 2 out]
        n464 = property on="ML axis8" class="Slide (strict)"("Visible"=w991) -> ()  [unwired: 2 in, 2 out]
        n465 = property on="Stimulus Out" class="Clust (strict)"("Val(Sgnl)"=w989) -> ()  [unwired: 2 in, 2 out]
        n466 = property on="V on DUT8" class="Bool (strict)"("Visible"=w986) -> ()  [unwired: 2 in, 2 out]
        n467 = case shown="False" w986 {
          selector: w986 -> [w992 _]
          frame False {
            n468 = property on="Output Imp8" class="Ring (strict)"("Visible"=w992) -> ()  [unwired: 2 in, 2 out]
            n469 = property on="Nominal Imp8" class="DigNum (strict)"("Visible"=w992) -> ()  [unwired: 2 in, 2 out]
          }
          frame True {
            n470 = property on="V on DUT8" class="Bool (strict)"() -> ("Value"=w993:bool)  [unwired: 2 in, 2 out]
            n471 = property on="V on DUT8" class="Bool (strict)"("Val(Sgnl)"=w993) -> ()  [unwired: 2 in, 2 out]
          }
        }
      }
      event "V on DUT8": Value Change {
        n472 = event-data() -> ("NewVal"=w1000:bool)  [unwired: 6 out]
        n473 = Bundle By Name(cluster=w1001, "V on DUT"=w1000) -> (w1002:T2)
        n474 = property on="Output Imp8" class="Ring (strict)"("Visible"=w1000) -> ()  [unwired: 2 in, 2 out]
        n475 = property on="Stimulus Out" class="Clust (strict)"("Val(Sgnl)"=w1002) -> ()  [unwired: 2 in, 2 out]
        n476 = property on="Nominal Imp8" class="DigNum (strict)"("Visible"=w1000) -> ()  [unwired: 2 in, 2 out]
      }
      event "Output Imp8": Value Change {
        n477 = event-data() -> ("NewVal"=w1003:u16)  [unwired: 6 out]
        n478 = Bundle By Name(cluster=w1004, "Output Imp"=w1003) -> (w1005:T2)
        n479 = property on="Stimulus Out" class="Clust (strict)"("Val(Sgnl)"=w1005) -> ()  [unwired: 2 in, 2 out]
      }
      event "Nominal Imp8": Value Change {
        n480 = event-data() -> ("NewVal"=w1006:dbl)  [unwired: 6 out]
        n481 = Bundle By Name(cluster=w1007, "Nominal Imp"=w1006) -> (w1008:T2)
        n482 = property on="Stimulus Out" class="Clust (strict)"("Val(Sgnl)"=w1008) -> ()  [unwired: 2 in, 2 out]
      }
      event "ML axis8": Value Change {
        n483 = event-data() -> ("NewVal"=w1013:u16)  [unwired: 6 out]
        n484 = property on="ML val level name8" class="Ring (strict)"() -> ("Value"=w1009:u16)  [unwired: 2 in, 2 out]
        n485 = Index Array(array=w1014, index=w1009) -> (element=w1019:T6)
        n486 = Unbundle By Name(w1019) -> ("Curve"=w1020:cluster{"x":dbl, "y":dbl, "z":dbl}[], "X unit"=w1017:string, "Y unit"=w1016:string, "Z unit"=w1015:string)
        n487 = Index Array(array=w1020) -> (element=w1018:cluster{"x":dbl, "y":dbl, "z":dbl})  [unwired: 1 in]
        n488 = case shown="1" w1013 {
          tunnel: w1018 -> [w1027 w1030 w1033]
          tunnel: w1017 -> [w1026 _ _]
          tunnel: w1016 -> [_ w1029 _]
          tunnel: w1015 -> [_ _ w1032]
          tunnel: [w1026 w1029 w1032] -> w1011
          tunnel: [w1025 w1028 w1031] -> w1012
          frame 0, Default {
            n489 = Unbundle By Name(w1027) -> ("x"=w1025:dbl)
          }
          frame 1 {
            n490 = Unbundle By Name(w1030) -> ("y"=w1028:dbl)
            n491 = property on="LinLevel1" class="DigNum (strict)"("Value"=w1028) -> ()  [unwired: 2 in, 2 out]
          }
          frame 2 {
            n492 = Unbundle By Name(w1033) -> ("z"=w1031:dbl)
          }
        }
        n493 = property on="deg8" class="DigNum (strict)"("Caption.Text"=w1011) -> ()  [unwired: 2 in, 2 out]
        n494 = property on="deg8" class="DigNum (strict)"("Value"=w1012) -> ()  [unwired: 2 in, 2 out]
        n495 = Build Array(w1011) -> (w1021:string[])
        n496 = Build Array(w1012) -> (w1022:dbl[])
        n497 = Build Array(w1013) -> (w1024:u16[])
        n498 = Bundle By Name(cluster=w1010, "ML_axisArray"=w1024, "DegValArray"=w1022, "DegUnitArray"=w1021) -> (w1023:T2)
        n499 = property on="Stimulus Out" class="Clust (strict)"("Val(Sgnl)"=w1023) -> ()  [unwired: 2 in, 2 out]
      }
      event Value Change {
        n500 = event-data() -> ()  [unwired: 7 out]
        n501 = property on="LinLevel1" class="DigNum (strict)"() -> ("Value"=w1035:dbl)  [unwired: 2 in, 2 out]
        n502 = property on="LinLevel2" class="DigNum (strict)"() -> ("Value"=w1034:dbl)  [unwired: 2 in, 2 out]
        n503 = local read "Stimulus Type"() -> (w1038:u16)
        n504 = case shown="3" w1038 {
          tunnel: [w1052 w1076 w1095 w1113 w1126 w1160 w1182 w1208] -> w1037
          tunnel: w1035 -> [w1051 w1074 _ w1103 _ w1138 _ _]
          tunnel: w1034 -> [_ _ _ _ _ w1137 _ _]
          frame 0, Default {
            w1048 = T10 {"Level(U)"=0.7071067811865476, "Start Freq(Hz)"=20000.0, "Stop Freq(Hz)"=20.0, "ML val level name"="Calibration sens-out Left", "Use ML Val level?"=FALSE, "ML axis"=0, "Steps (#)"=31, "Cycles/step(#)"=20, "Time/step (s)"=0.01, "Step Resolution"=0, "unit"=0, "Start Freq Name"="Calibration sens-out Left", "Stop Freq Name"="Calibration sens-out Left", "Start Freq Axis"=0, "Stop Freq Axis"=0, "Start Freq Flag"="", "Stop Freq Flag"="", "Output Imp"=0.0, "Nominal Imp"=0.0, "V on DUT"=FALSE}  # fstepsw
            n505 = property on="StartFreq1_CurLib" class="Ring (strict)"() -> ("RingText.Text"=w1047:string)  [unwired: 2 in, 2 out]
            n506 = property on="StopFreq1_CurLib" class="Ring (strict)"() -> ("RingText.Text"=w1046:string)  [unwired: 2 in, 2 out]
            n507 = property on="ML val level name" class="Ring (strict)"() -> ("RingText.Text"=w1050:string)  [unwired: 2 in, 2 out]
            n508 = local read "unit1"() -> (w1049:u16)
            n509 = property on="V on DUT1" class="Bool (strict)"() -> ("Value"=w1039:bool)  [unwired: 2 in, 2 out]
            n510 = property on="Nominal Imp1" class="DigNum (strict)"() -> ("Value"=w1040:dbl)  [unwired: 2 in, 2 out]
            n511 = property on="StartFreq1_Flag" class="Str"() -> ("Value"=w1043:string)  [unwired: 2 in, 2 out]
            n512 = property on="StopFreq1_Flag" class="Str"() -> ("Value"=w1042:string)  [unwired: 2 in, 2 out]
            n513 = property on="Output Imp1" class="Ring (strict)"() -> ("Value"=w1041:u16)  [unwired: 2 in, 2 out]
            n514 = property on="StartFreq1_axis" class="Slide (strict)"() -> ("Value"=w1045:u16)  [unwired: 2 in, 2 out]
            n515 = property on="StopFreq1_axis" class="Slide (strict)"() -> ("Value"=w1044:u16)  [unwired: 2 in, 2 out]
            n516 = property on="StartFreq1(Hz)" class="DigNum (strict)"() -> ("Value"=w1062:dbl)  [unwired: 2 in, 2 out]
            n517 = property on="StopFreq1(Hz)" class="DigNum (strict)"() -> ("Value"=w1061:dbl)  [unwired: 2 in, 2 out]
            n518 = property on="UseMLVal_Level_1" class="Slide (strict)"() -> ("Value"=w1060:u16)  [unwired: 2 in, 2 out]
            n519 = property on="ML axis1" class="Slide (strict)"() -> ("Value"=w1058:u16)  [unwired: 2 in, 2 out]
            n520 = property on="Steps1" class="DigNum (strict)"() -> ("Value"=w1057:i32)  [unwired: 2 in, 2 out]
            n521 = property on="Cycle/step1" class="DigNum (strict)"() -> ("Value"=w1056:u32)  [unwired: 2 in, 2 out]
            n522 = property on="Time/steps1(s)" class="DigNum (strict)"() -> ("Value"=w1055:dbl)  [unwired: 2 in, 2 out]
            n523 = property on="Step Resolution1" class="Ring (strict)"() -> ("Value"=w1054:u16)  [unwired: 2 in, 2 out]
            n524 = Not Equal To 0?(x=w1060) -> (x != 0?=w1059:bool)
            n525 = Bundle By Name(cluster=w1048, "Level(U)"=w1051, "Start Freq(Hz)"=w1062, "Stop Freq(Hz)"=w1061, "ML val level name"=w1050, "Use ML Val level?"=w1059, "ML axis"=w1058, "Steps (#)"=w1057, "Cycles/step(#)"=w1056, "Time/step (s)"=w1055, "Step Resolution"=w1054, "unit"=w1049, "Start Freq Name"=w1047, "Stop Freq Name"=w1046, "Start Freq Axis"=w1045, "Stop Freq Axis"=w1044, "Start Freq Flag"=w1043, "Stop Freq Flag"=w1042, "Output Imp"=w1041, "Nominal Imp"=w1040, "V on DUT"=w1039) -> (w1053:T10)
            n526 = Variant To Flattened String(Variant=w1053) -> (data string=w1052:string)  [unwired: 1 out]
          }
          frame 1 {
            w1072 = T11 {"Level(U)"=1.0, "Start Freq(Hz)"=100.0, "Stop Freq(Hz)"=6300.0, "Sweep Rate(s/dec)"=1.0, "Use ML Val level?"=FALSE, "ML val level name"="", "ML axis"=1, "TSR params"={"FSamp"=0.0, "FStart"=0.0, "FStop"=0.0, "NOffset"=0.0, "MStop"=0.0, "MStart"=0.0, "NHarm"=0.0, "Tsamp"=0.0, "Amplit"=0.0}, "unit"=0, "Start Freq Name"="Calibration sens-out Left", "Stop Freq Name"="Calibration sens-out Left", "Start Freq Axis"=0, "Stop Freq Axis"=0, "Start Freq Flag"="", "Stop Freq Flag"="", "Output Imp"=0.0, "Nominal Imp"=0.0, "V on DUT"=FALSE}  # flogsw
            n527 = property on="ML val level name2" class="Ring (strict)"() -> ("RingText.Text"=w1078:string)  [unwired: 2 in, 2 out]
            n528 = property on="StartFreq2_CurLib" class="Ring (strict)"() -> ("RingText.Text"=w1071:string)  [unwired: 2 in, 2 out]
            n529 = property on="StopFreq2_CurLib" class="Ring (strict)"() -> ("RingText.Text"=w1070:string)  [unwired: 2 in, 2 out]
            n530 = local read "unit2"() -> (w1073:u16)
            n531 = property on="V on DUT2" class="Bool (strict)"() -> ("Value"=w1063:bool)  [unwired: 2 in, 2 out]
            n532 = property on="Output Imp2" class="Ring (strict)"() -> ("Value"=w1065:u16)  [unwired: 2 in, 2 out]
            n533 = property on="Nominal Imp2" class="DigNum (strict)"() -> ("Value"=w1064:dbl)  [unwired: 2 in, 2 out]
            n534 = property on="StartFreq2(Hz)" class="DigNum (strict)"() -> ("Value"=w1083:dbl)  [unwired: 2 in, 2 out]
            n535 = property on="StopFreq2(Hz)" class="DigNum (strict)"() -> ("Value"=w1082:dbl)  [unwired: 2 in, 2 out]
            n536 = property on="Sweept Rate2(s/dec)" class="DigNum (strict)"() -> ("Value"=w1081:dbl)  [unwired: 2 in, 2 out]
            n537 = property on="UseMLVal_Level_2" class="Slide (strict)"() -> ("Value"=w1080:u16)  [unwired: 2 in, 2 out]
            n538 = property on="ML axis2" class="Slide (strict)"() -> ("Value"=w1077:u16)  [unwired: 2 in, 2 out]
            n539 = property on="StartFreq2_axis" class="Slide (strict)"() -> ("Value"=w1069:u16)  [unwired: 2 in, 2 out]
            n540 = property on="StopFreq2_axis" class="Slide (strict)"() -> ("Value"=w1068:u16)  [unwired: 2 in, 2 out]
            n541 = property on="StartFreq2_Flag" class="Str"() -> ("Value"=w1067:string)  [unwired: 2 in, 2 out]
            n542 = property on="StopFreq2_Flag" class="Str"() -> ("Value"=w1066:string)  [unwired: 2 in, 2 out]
            n543 = Not Equal To 0?(x=w1080) -> (x != 0?=w1079:bool)
            n544 = Bundle By Name(cluster=w1072, "Level(U)"=w1074, "Start Freq(Hz)"=w1083, "Stop Freq(Hz)"=w1082, "Sweep Rate(s/dec)"=w1081, "Use ML Val level?"=w1079, "ML val level name"=w1078, "ML axis"=w1077, "unit"=w1073, "Start Freq Name"=w1071, "Stop Freq Name"=w1070, "Start Freq Axis"=w1069, "Stop Freq Axis"=w1068, "Start Freq Flag"=w1067, "Stop Freq Flag"=w1066, "Output Imp"=w1065, "Nominal Imp"=w1064, "V on DUT"=w1063) -> (w1075:T11)
            n545 = Variant To Flattened String(Variant=w1075) -> (data string=w1076:string)  [unwired: 1 out]
          }
          frame 2 {
            w1084 = T12 {"Freq(Hz)"=1000.0, "Steps (#)"=19, "Cycles(#)"=12, "Use ML Val freq?"=FALSE, "ML val freq name"="", "ML axis"=1, "Start Ampl(U)"=0.5, "Stop Ampl(U)"=1.0, "unit"=0}  # ampsw
            n546 = local read "RealFreq3(Hz)"() -> (w1088:dbl)
            n547 = property on="ML val level name3" class="Ring (strict)"() -> ("RingText.Text"=w1090:string)  [unwired: 2 in, 2 out]
            n548 = local read "unit3"() -> (w1085:u16)
            n549 = property on="Steps3" class="DigNum (strict)"() -> ("Value"=w1094:i32)  [unwired: 2 in, 2 out]
            n550 = property on="Cycles3" class="DigNum (strict)"() -> ("Value"=w1093:u32)  [unwired: 2 in, 2 out]
            n551 = property on="UseMLVal_Level_3" class="Slide (strict)"() -> ("Value"=w1092:u16)  [unwired: 2 in, 2 out]
            n552 = property on="ML axis3" class="Slide (strict)"() -> ("Value"=w1089:u16)  [unwired: 2 in, 2 out]
            n553 = property on="LinLevel1" class="DigNum (strict)"() -> ("Value"=w1087:dbl)  [unwired: 2 in, 2 out]
            n554 = property on="LinLevel2" class="DigNum (strict)"() -> ("Value"=w1086:dbl)  [unwired: 2 in, 2 out]
            n555 = Not Equal To 0?(x=w1092) -> (x != 0?=w1091:bool)
            n556 = Bundle By Name(cluster=w1084, "Freq(Hz)"=w1088, "Steps (#)"=w1094, "Cycles(#)"=w1093, "Use ML Val freq?"=w1091, "ML val freq name"=w1090, "ML axis"=w1089, "Start Ampl(U)"=w1087, "Stop Ampl(U)"=w1086, "unit"=w1085) -> (w1096:T12)
            n557 = Variant To Flattened String(Variant=w1096) -> (data string=w1095:string)  [unwired: 1 out]
          }
          frame 3 {
            w1100 = T13 {"Level(U)"=0.0, "Wave Path"="", "ML axis"=1, "ML val level name"="", "Use ML Val level?"=FALSE, "wave info"="", "wave time"="", "Peak value4"=0.0, "RMS value4"=0.0, "wave channel"=0, "unit"=0, "Output Imp"=0.0, "Nominal Imp"=0.0, "V on DUT"=FALSE}  # wavefile
            n558 = property on="ML val level name4" class="Ring (strict)"() -> ("RingText.Text"=w1110:string)  [unwired: 2 in, 2 out]
            n559 = property on="ML axis4" class="Slide (strict)"() -> ("Value"=w1111:u16)  [unwired: 2 in, 2 out]
            n560 = property on="UseMLVal_Level_4" class="Slide (strict)"() -> ("Value"=w1109:u16)  [unwired: 2 in, 2 out]
            n561 = property on="wave info" class="Str"() -> ("Value"=w1107:string)  [unwired: 2 in, 2 out]
            n562 = property on="wave time" class="Str"() -> ("Value"=w1106:string)  [unwired: 2 in, 2 out]
            n563 = property on="Peak value4" class="DigNum (strict)"() -> ("Value"=w1105:dbl)  [unwired: 2 in, 2 out]
            n564 = property on="RMS value4" class="DigNum (strict)"() -> ("Value"=w1104:dbl)  [unwired: 2 in, 2 out]
            n565 = property on="Wave Channel" class="Ring (strict)"() -> ("Value"=w1102:u16)  [unwired: 2 in, 2 out]
            n566 = property on="Wave Path4" class="Path"() -> ("Text.Text"=w1112:string)  [unwired: 2 in, 2 out]
            n567 = property on="V on DUT4" class="Bool (strict)"() -> ("Value"=w1097:bool)  [unwired: 2 in, 2 out]
            n568 = property on="Nominal Imp4" class="DigNum (strict)"() -> ("Value"=w1098:dbl)  [unwired: 2 in, 2 out]
            n569 = property on="Output Imp4" class="Ring (strict)"() -> ("Value"=w1099:u16)  [unwired: 2 in, 2 out]
            n570 = Not Equal To 0?(x=w1109) -> (x != 0?=w1108:bool)
            n571 = local read "unit4"() -> (w1101:u16)
            n572 = Bundle By Name(cluster=w1100, "Level(U)"=w1103, "Wave Path"=w1112, "ML axis"=w1111, "ML val level name"=w1110, "Use ML Val level?"=w1108, "wave info"=w1107, "wave time"=w1106, "Peak value4"=w1105, "RMS value4"=w1104, "wave channel"=w1102, "unit"=w1101, "Output Imp"=w1099, "Nominal Imp"=w1098, "V on DUT"=w1097) -> (w1114:T13)
            n573 = Variant To Flattened String(Variant=w1114) -> (data string=w1113:string)  [unwired: 1 out]
          }
          frame 4 {
            w1115 = T14 {"dc ctrl"=0, "dcmax I"=0, "dc polar"=0, "dc ctrl"=0, "Steps (#)"=19, "Time/step (s)"=0.05, "Start Ampl(U)"=1.0, "Stop Ampl(U)"=1.0, "Level(U)"=1.0, "Step Size"=1.0}  # dcconn
            n574 = property on="dc_ctrl5_1" class="Slide (strict)"() -> ("Value"=w1125:u16)  [unwired: 2 in, 2 out]
            n575 = property on="Max.Current" class="Slide (strict)"() -> ("Value"=w1124:u16)  [unwired: 2 in, 2 out]
            n576 = property on="dcpolar5" class="Slide (strict)"() -> ("Value"=w1123:u16)  [unwired: 2 in, 2 out]
            n577 = property on="dc_ctrl5_2" class="Slide (strict)"() -> ("Value"=w1122:u16)  [unwired: 2 in, 2 out]
            n578 = property on="Steps5" class="DigNum (strict)"() -> ("Value"=w1121:i32)  [unwired: 2 in, 2 out]
            n579 = property on="Time/Step5" class="DigNum (strict)"() -> ("Value"=w1120:dbl)  [unwired: 2 in, 2 out]
            n580 = property on="StartAmp5" class="DigNum (strict)"() -> ("Value"=w1118:dbl)  [unwired: 2 in, 2 out]
            n581 = property on="StopAmp5" class="DigNum (strict)"() -> ("Value"=w1119:dbl)  [unwired: 2 in, 2 out]
            n582 = property on="Level5" class="DigNum (strict)"() -> ("Value"=w1117:dbl)  [unwired: 2 in, 2 out]
            n583 = property on="Steps Size5" class="DigNum (strict)"() -> ("Value"=w1116:dbl)  [unwired: 2 in, 2 out]
            n584 = Bundle By Name(cluster=w1115, "dc ctrl"=w1125, "dcmax I"=w1124, "dc polar"=w1123, "dc ctrl"=w1122, "Steps (#)"=w1121, "Time/step (s)"=w1120, "Start Ampl(U)"=w1118, "Stop Ampl(U)"=w1119, "Level(U)"=w1117, "Step Size"=w1116) -> (w1127:T14)
            n585 = Variant To Flattened String(Variant=w1127) -> (data string=w1126:string)  [unwired: 1 out]
          }
          frame 5 {
            w1134 = T15 {"Steps (#)"=19, "Tone Type"=0, "Freq2(Hz)"=1000.0, "Time/step (s)"=0.0, "Cycles/step (#)"=12, "ML val level name"="", "Use ML Val level?"=FALSE, "Level(U) 2"=1.0, "Diff Freq(Hz)"=100.0, "ML axis 2"=1, "Diff/Ratio"=0, "Level(U)"=1.0, "Stop Freq(Hz)"=100.0, "Ratio Val"=0.8, "ML val level name 2"="", "Use ML Val level? 2"=FALSE, "ML axis"=1, "Start Freq(Hz)"=6300.0, "Step Resolution"=0, "Ratio"=0, "TabCtrl6"=enum."Master Tone", "unit 1"=0, "unit 2"=0, "Start Freq Name"="", "Stop Freq Name"="", "Start Freq Axis"=0, "Stop Freq Axis"=0, "Start Freq Flag"="", "Stop Freq Flag"=""}  # twotone
            n586 = property on="ML val level name6_2" class="Ring (strict)"() -> ("RingText.Text"=w1147:string)  [unwired: 2 in, 2 out]
            n587 = property on="Sweep Type" class="Slide (strict)"() -> ("Value"=w1158:u16)  [unwired: 2 in, 2 out]
            n588 = property on="Time/step6(s)" class="DigNum (strict)"() -> ("Value"=w1156:dbl)  [unwired: 2 in, 2 out]
            n589 = property on="Cycle/steps6" class="DigNum (strict)"() -> ("Value"=w1155:u32)  [unwired: 2 in, 2 out]
            n590 = property on="UseMLVal_Level6_1" class="Slide (strict)"() -> ("Value"=w1153:u16)  [unwired: 2 in, 2 out]
            n591 = property on="Difference6(Hz)" class="DigNum (strict)"() -> ("Value"=w1151:dbl)  [unwired: 2 in, 2 out]
            n592 = property on="Fixed/Ratio6" class="Slide (strict)"() -> ("Value"=w1149:u16)  [unwired: 2 in, 2 out]
            n593 = property on="StopFreq6(Hz)" class="DigNum (strict)"() -> ("Value"=w1148:dbl)  [unwired: 2 in, 2 out]
            n594 = property on="ML axis6_1" class="Slide (strict)"() -> ("Value"=w1144:u16)  [unwired: 2 in, 2 out]
            n595 = property on="StepResolution6" class="Ring (strict)"() -> ("Value"=w1142:u16)  [unwired: 2 in, 2 out]
            n596 = Not Equal To 0?(x=w1153) -> (x != 0?=w1152:bool)
            n597 = property on="ML val level name6_1" class="Ring (strict)"() -> ("RingText.Text"=w1154:string)  [unwired: 2 in, 2 out]
            n598 = property on="Steps6" class="DigNum (strict)"() -> ("Value"=w1159:i32)  [unwired: 2 in, 2 out]
            n599 = property on="Freq6(Hz)" class="DigNum (strict)"() -> ("Value"=w1157:dbl)  [unwired: 2 in, 2 out]
            n600 = property on="ML axis6_2" class="Slide (strict)"() -> ("Value"=w1150:u16)  [unwired: 2 in, 2 out]
            n601 = property on="UseMLVal_Level6_2" class="Slide (strict)"() -> ("Value"=w1146:u16)  [unwired: 2 in, 2 out]
            n602 = property on="StartFreq6_CurLib" class="Ring (strict)"() -> ("RingText.Text"=w1133:string)  [unwired: 2 in, 2 out]
            n603 = property on="StopFreq6_CurLib" class="Ring (strict)"() -> ("RingText.Text"=w1132:string)  [unwired: 2 in, 2 out]
            n604 = property on="StartFreq6(Hz)" class="DigNum (strict)"() -> ("Value"=w1143:dbl)  [unwired: 2 in, 2 out]
            n605 = property on="Ratio6" class="Ring (strict)"() -> ("Value"=w1141:u16)  [unwired: 2 in, 2 out]
            n606 = property on="Ratio Freq6(Hz)" class="DigNum (strict)"() -> ("Value"=w1140:dbl)  [unwired: 2 in, 2 out]
            n607 = property on="Control6 Tab" class="TabCtl (strict)"() -> ("Value"=w1139:enum32{"Master Tone", "Slave Tone"})  [unwired: 2 in, 2 out]
            n608 = property on="StartFreq6_axis" class="Slide (strict)"() -> ("Value"=w1131:u16)  [unwired: 2 in, 2 out]
            n609 = property on="StopFreq6_axis" class="Slide (strict)"() -> ("Value"=w1130:u16)  [unwired: 2 in, 2 out]
            n610 = Not Equal To 0?(x=w1146) -> (x != 0?=w1145:bool)
            n611 = local read "unit6_1"() -> (w1135:u16)
            n612 = local read "unit6"() -> (w1136:u16)
            n613 = property on="StartFreq6_Flag" class="Str"() -> ("Value"=w1129:string)  [unwired: 2 in, 2 out]
            n614 = property on="StopFreq6_Flag" class="Str"() -> ("Value"=w1128:string)  [unwired: 2 in, 2 out]
            n615 = Bundle By Name(cluster=w1134, "Steps (#)"=w1159, "Tone Type"=w1158, "Freq2(Hz)"=w1157, "Time/step (s)"=w1156, "Cycles/step (#)"=w1155, "ML val level name"=w1154, "Use ML Val level?"=w1152, "Level(U) 2"=w1137, "Diff Freq(Hz)"=w1151, "ML axis 2"=w1150, "Diff/Ratio"=w1149, "Level(U)"=w1138, "Stop Freq(Hz)"=w1148, "ML val level name 2"=w1147, "Use ML Val level? 2"=w1145, "ML axis"=w1144, "Start Freq(Hz)"=w1143, "Step Resolution"=w1142, "Ratio"=w1141, "Ratio Val"=w1140, "TabCtrl6"=w1139, "unit 1"=w1136, "unit 2"=w1135, "Start Freq Name"=w1133, "Stop Freq Name"=w1132, "Start Freq Axis"=w1131, "Stop Freq Axis"=w1130, "Start Freq Flag"=w1129, "Stop Freq Flag"=w1128) -> (w1161:T15)
            n616 = Variant To Flattened String(Variant=w1161) -> (data string=w1160:string)  [unwired: 1 out]
          }
          frame 6 {
            w1171 = T16 {"Noise Type"=0, "Min Freq(Hz)"=20.0, "Max Freq(Hz)"=20000.0, "Level(U)"=1.0, "Duration(s)"=1.0, "ML val level name"="", "Use ML Val level?"=FALSE, "ML axis"=1, "unit"=0, "Start Freq Name"="", "Stop Freq Name"="", "Start Freq Axis"=0, "Stop Freq Axis"=0, "Start Freq Flag"="", "Stop Freq Flag"="", "Output Imp"=0.0, "Nominal Imp"=0.0, "V on DUT"=FALSE}  # noise
            n617 = property on="StartFreq7_CurLib" class="Ring (strict)"() -> ("RingText.Text"=w1170:string)  [unwired: 2 in, 2 out]
            n618 = property on="StopFreq7_CurLib" class="Ring (strict)"() -> ("RingText.Text"=w1169:string)  [unwired: 2 in, 2 out]
            n619 = property on="ML val level name7" class="Ring (strict)"() -> ("RingText.Text"=w1174:string)  [unwired: 2 in, 2 out]
            n620 = local read "unit7"() -> (w1173:u16)
            n621 = property on="Nominal Imp7" class="DigNum (strict)"() -> ("Value"=w1163:dbl)  [unwired: 2 in, 2 out]
            n622 = property on="V on DUT7" class="Bool (strict)"() -> ("Value"=w1162:bool)  [unwired: 2 in, 2 out]
            n623 = property on="Output Imp7" class="Ring (strict)"() -> ("Value"=w1164:u16)  [unwired: 2 in, 2 out]
            n624 = property on="StartFreq7_axis" class="Slide (strict)"() -> ("Value"=w1168:u16)  [unwired: 2 in, 2 out]
            n625 = property on="StopFreq7_axis" class="Slide (strict)"() -> ("Value"=w1167:u16)  [unwired: 2 in, 2 out]
            n626 = property on="StartFreq7_Flag" class="Str"() -> ("Value"=w1166:string)  [unwired: 2 in, 2 out]
            n627 = property on="StopFreq7_Flag" class="Str"() -> ("Value"=w1165:string)  [unwired: 2 in, 2 out]
            n628 = property on="Noise Type7" class="Slide (strict)"() -> ("Value"=w1181:u16)  [unwired: 2 in, 2 out]
            n629 = property on="StartFreq7(Hz)" class="DigNum (strict)"() -> ("Value"=w1180:dbl)  [unwired: 2 in, 2 out]
            n630 = property on="StopFreq7(Hz)" class="DigNum (strict)"() -> ("Value"=w1179:dbl)  [unwired: 2 in, 2 out]
            n631 = property on="Level7(U)" class="DigNum (strict)"() -> ("Value"=w1172:dbl)  [unwired: 2 in, 2 out]
            n632 = property on="Duration7(s)" class="DigNum (strict)"() -> ("Value"=w1178:dbl)  [unwired: 2 in, 2 out]
            n633 = property on="UseMLVal_Level_7" class="Slide (strict)"() -> ("Value"=w1177:u16)  [unwired: 2 in, 2 out]
            n634 = property on="ML axis7" class="Slide (strict)"() -> ("Value"=w1175:u16)  [unwired: 2 in, 2 out]
            n635 = Not Equal To 0?(x=w1177) -> (x != 0?=w1176:bool)
            n636 = Bundle By Name(cluster=w1171, "Noise Type"=w1181, "Min Freq(Hz)"=w1180, "Max Freq(Hz)"=w1179, "Level(U)"=w1172, "Duration(s)"=w1178, "ML val level name"=w1174, "Use ML Val level?"=w1176, "ML axis"=w1175, "unit"=w1173, "Start Freq Name"=w1170, "Stop Freq Name"=w1169, "Start Freq Axis"=w1168, "Stop Freq Axis"=w1167, "Start Freq Flag"=w1166, "Stop Freq Flag"=w1165, "Output Imp"=w1164, "Nominal Imp"=w1163, "V on DUT"=w1162) -> (w1183:T16)
            n637 = Variant To Flattened String(Variant=w1183) -> (data string=w1182:string)  [unwired: 1 out]
          }
          frame 7 {
            w1193 = T17 {"Level(U)"=0.0, "Min Freq(Hz)"=0.0, "Max Freq(Hz)"=0.0, "Duration(s)"=0.0, "Freq Rounding"=FALSE, "Rounding Val"=5.0, "Profile"=0, "ML axis 2"=0, "ML val level name"="", "Use ML Val level?"=FALSE, "ML axis"=0, "Step Resolution"=0, "unit"=0, "Start Freq Name"="Calibration sens-out Left", "Stop Freq Name"="Calibration sens-out Left", "Start Freq Axis"=0, "Stop Freq Axis"=0, "Start Freq Flag"="", "Stop Freq Flag"="", "Output Imp"=0.0, "Nominal Imp"=0.0, "V on DUT"=FALSE}  # mltitone
            n638 = property on="StartFreq8_CurLib" class="Ring (strict)"() -> ("RingText.Text"=w1192:string)  [unwired: 2 in, 2 out]
            n639 = property on="StopFreq8_CurLib" class="Ring (strict)"() -> ("RingText.Text"=w1191:string)  [unwired: 2 in, 2 out]
            n640 = property on="ML val level name8" class="Ring (strict)"() -> ("RingText.Text"=w1199:string)  [unwired: 2 in, 2 out]
            n641 = local read "unit8"() -> (w1195:u16)
            n642 = property on="StartFreq8_axis" class="Slide (strict)"() -> ("Value"=w1190:u16)  [unwired: 2 in, 2 out]
            n643 = property on="StopFreq8_axis" class="Slide (strict)"() -> ("Value"=w1189:u16)  [unwired: 2 in, 2 out]
            n644 = property on="StartFreq8_Flag" class="Str"() -> ("Value"=w1188:string)  [unwired: 2 in, 2 out]
            n645 = property on="StopFreq8_Flag" class="Str"() -> ("Value"=w1187:string)  [unwired: 2 in, 2 out]
            n646 = property on="Level8(U)" class="DigNum (strict)"() -> ("Value"=w1194:dbl)  [unwired: 2 in, 2 out]
            n647 = property on="StartFreq8(Hz)" class="DigNum (strict)"() -> ("Value"=w1206:dbl)  [unwired: 2 in, 2 out]
            n648 = property on="StopFreq8(Hz)" class="DigNum (strict)"() -> ("Value"=w1205:dbl)  [unwired: 2 in, 2 out]
            n649 = property on="Duration8(s)" class="DigNum (strict)"() -> ("Value"=w1204:dbl)  [unwired: 2 in, 2 out]
            n650 = property on="Tones8" class="DigNum (strict)"() -> ("Value"=w1203:i32)  [unwired: 2 in, 2 out]
            n651 = property on="Step Resolution8" class="Ring (strict)"() -> ("Value"=w1202:u16)  [unwired: 2 in, 2 out]
            n652 = property on="Freq Rounding8" class="Bool (strict)"() -> ("Value"=w1201:bool)  [unwired: 2 in, 2 out]
            n653 = property on="Rounding Val8" class="DigNum (strict)"() -> ("Value"=w1200:dbl)  [unwired: 2 in, 2 out]
            n654 = property on="UseMLVal_Level_8" class="Slide (strict)"() -> ("Value"=w1198:u16)  [unwired: 2 in, 2 out]
            n655 = property on="ML axis8" class="Slide (strict)"() -> ("Value"=w1196:u16)  [unwired: 2 in, 2 out]
            n656 = property on="Nominal Imp8" class="DigNum (strict)"() -> ("Value"=w1185:dbl)  [unwired: 2 in, 2 out]
            n657 = property on="V on DUT8" class="Bool (strict)"() -> ("Value"=w1184:bool)  [unwired: 2 in, 2 out]
            n658 = property on="Output Imp8" class="Ring (strict)"() -> ("Value"=w1186:u16)  [unwired: 2 in, 2 out]
            n659 = Not Equal To 0?(x=w1198) -> (x != 0?=w1197:bool)
            n660 = Bundle By Name(cluster=w1193, "Level(U)"=w1194, "Min Freq(Hz)"=w1206, "Max Freq(Hz)"=w1205, "Duration(s)"=w1204, "Profile"=w1203, "Step Resolution"=w1202, "Freq Rounding"=w1201, "Rounding Val"=w1200, "ML val level name"=w1199, "Use ML Val level?"=w1197, "ML axis"=w1196, "unit"=w1195, "Start Freq Name"=w1192, "Stop Freq Name"=w1191, "Start Freq Axis"=w1190, "Stop Freq Axis"=w1189, "Start Freq Flag"=w1188, "Stop Freq Flag"=w1187, "Output Imp"=w1186, "Nominal Imp"=w1185, "V on DUT"=w1184) -> (w1207:T17)
            n661 = Variant To Flattened String(Variant=w1207) -> (data string=w1208:string)  [unwired: 1 out]
          }
        }
        n662 = call "CRYFlatten Stimulus Element.vi"("Stimulus Type"=w1038, "Flattened Stimulus Element"=w1037) -> ("Flatten Stimulus Setup String"=w1036:string)  [unwired: 9 out]
        n663 = global write "CRYStimulus Global.vi" "Flatten Element"(w1036) -> ()
        n664 = local write "Flatten Element Out"(w1036) -> ()
      }
      event "StartFreq1(Hz)", "StopFreq1(Hz)", "StopFreq1_CurLib", "StartFreq1_CurLib", "StartFreq2(Hz)", "StopFreq2(Hz)", "StartFreq6(Hz)", "StopFreq6(Hz)", "StartFreq7(Hz)", "StopFreq7(Hz)", "StartFreq8(Hz)", "StopFreq8(Hz)", "StopFreq6_CurLib", "StartFreq6_CurLib", "StopFreq7_CurLib", "StartFreq7_CurLib", "StopFreq8_CurLib", "StartFreq8_CurLib", "StartFreq2_CurLib", "StopFreq2_CurLib": Shortcut Menu Activation? {
        n665 = event-data() -> ("MenuRef"=w1209:refnum<k9>)  [unwired: 7 out]
        n666 = call "CRYGet HZ Input Shortcut Menu.vi"("Runtime Menu Ref In"=w1209) -> ()  [unwired: 9 in, 2 out]
        n667 = event-data() -> ()  [unwired: 2 in, 1 out]
      }
      event "StartFreq1(Hz)", "StartFreq1_CurLib", "StopFreq1_CurLib", "StopFreq1(Hz)", "StartFreq2(Hz)", "StopFreq2(Hz)", "StartFreq6(Hz)", "StopFreq6(Hz)", "StartFreq7(Hz)", "StopFreq7(Hz)", "StartFreq8(Hz)", "StopFreq8(Hz)", "StopFreq6_CurLib", "StartFreq6_CurLib", "StopFreq7_CurLib", "StartFreq7_CurLib", "StopFreq8_CurLib", "StartFreq8_CurLib", "StartFreq2_CurLib", "StopFreq2_CurLib": Shortcut Menu Selection (User) {
        n668 = event-data() -> ("CtlRef"=w1226:refnum<vi>, "ItemTag"=w1217:string)  [unwired: 7 out]
        n669 = property class="Num"(reference=w1226) -> ("Label.Text"=w1213:string)  [unwired: 1 in, 2 out]
        n670 = Match Pattern(string=w1213, regular expression="Freq" ("y")) -> (after substring=w1215:string)  [unwired: 1 in, 3 out]
        n671 = Concatenate Strings(w1213, "###" ("string"), w1217) -> (w1210:string)
        n672 = String Subset(string=w1215, length (rest)=1 ("length (rest)")) -> (substring=w1212:string)  [unwired: 1 in]
        n673 = Match Pattern(string=w1213, regular expression="_") -> (before substring=w1219:string)  [unwired: 1 in, 3 out]
        n674 = Match Pattern(string=w1213, regular expression="(") -> (before substring=w1220:string, offset past match=w1222:i32)  [unwired: 1 in, 2 out]
        n675 = Decimal String To Number(string=w1212) -> (offset past number=w1211:i32)  [unwired: 2 in, 1 out]
        n676 = Greater Or Equal To 0?(x=w1222) -> (x >= 0?=w1221:bool)
        n677 = Select(t=w1220, s=w1221, f=w1219) -> (s? t:f=w1218:string)
        n678 = case shown="\"CURVE_VALUE\"" w1217 {
          tunnel: w1211 -> [_ w1235]
          frame "USER_INPUT", Default {
          }
          frame "CURVE_VALUE" {
            n679 = call "CRYGet Curve Library Data Name.vi"("sAction"="GetNameByType", "Type"=enum16{"Curves", "Values", "Results", "WFM"}."Values") -> ("sNames"=w1234:string[])  [unwired: 6 in, 3 out]
            n680 = case shown="1, Default" w1235 {
              tunnel: w1234 -> [w1238 w1239 w1240 w1241 w1242]
              frame 1, Default {
                n681 = property on="StartFreq1_CurLib" class="Ring (strict)"("Strings []"=w1238) -> ()  [unwired: 2 in, 2 out]
                n682 = property on="StopFreq1_CurLib" class="Ring (strict)"("Strings []"=w1238) -> ()  [unwired: 2 in, 2 out]
              }
              frame 2 {
                n683 = property on="StartFreq2_CurLib" class="Ring (strict)"("Strings []"=w1239) -> ()  [unwired: 2 in, 2 out]
                n684 = property on="StopFreq2_CurLib" class="Ring (strict)"("Strings []"=w1239) -> ()  [unwired: 2 in, 2 out]
              }
              frame 6 {
                n685 = property on="StartFreq6_CurLib" class="Ring (strict)"("Strings []"=w1240) -> ()  [unwired: 2 in, 2 out]
                n686 = property on="StopFreq6_CurLib" class="Ring (strict)"("Strings []"=w1240) -> ()  [unwired: 2 in, 2 out]
              }
              frame 7 {
                n687 = property on="StartFreq7_CurLib" class="Ring (strict)"("Strings []"=w1241) -> ()  [unwired: 2 in, 2 out]
                n688 = property on="StopFreq7_CurLib" class="Ring (strict)"("Strings []"=w1241) -> ()  [unwired: 2 in, 2 out]
              }
              frame 8 {
                n689 = property on="StartFreq8_CurLib" class="Ring (strict)"("Strings []"=w1242) -> ()  [unwired: 2 in, 2 out]
                n690 = property on="StopFreq8_CurLib" class="Ring (strict)"("Strings []"=w1242) -> ()  [unwired: 2 in, 2 out]
              }
            }
          }
        }
        n691 = case shown="1, 2, 6..8" w1211 {
          tunnel: w1218 -> [_ w1229]
          tunnel: w1217 -> [_ w1228]
          tunnel: w1210 -> [_ w1227]
          frame Default {
          }
          frame 1, 2, 6..8 {
            n692 = property on="StartStopFreqValue" class="Str"("Val(Sgnl)"=w1227) -> ()  [unwired: 2 in, 2 out]
            n693 = Concatenate Strings(w1229, "_Flag" ("string")) -> (w1232:string)
            n694 = invoke class="VI" method="Ctrl Val.Set"("Control Name"=w1232, "Value"=w1228) -> (reference out=w1231:refnum<vi>)  [unwired: 3 in, 4 out]
            n695 = flat-sequence {
              tunnel: w1231 -> [_]
              frame #0 {
                n696 = property on="Stimulus Out" class="Clust (strict)"() -> ("Value"=w1233:T2)  [unwired: 2 in, 2 out]
                n697 = property on="Stimulus Out" class="Clust (strict)"("Val(Sgnl)"=w1233) -> ()  [unwired: 2 in, 2 out]
              }
            }
          }
        }
      }
      event "StartFreq1_axis", "StopFreq1_axis", "StartFreq2_axis", "StopFreq2_axis", "StopFreq6_axis", "StartFreq6_axis", "StopFreq7_axis", "StartFreq7_axis", "StopFreq8_axis", "StartFreq8_axis": Value Change {
        n698 = event-data() -> ("CtlRef"=w1246:refnum<vi>)  [unwired: 6 out]
        n699 = property class="Slide (strict)"(reference=w1246) -> ("Label.Text"=w1245:string)  [unwired: 1 in, 2 out]
        n700 = property on="Stimulus Out" class="Clust (strict)"() -> ("Value"=w1243:T2)  [unwired: 2 in, 2 out]
        n701 = property on="Stimulus Out" class="Clust (strict)"("Val(Sgnl)"=w1243) -> ()  [unwired: 2 in, 2 out]
        n702 = Match Pattern(string=w1245, regular expression="_axis" ("y")) -> (before substring=w1244:string)  [unwired: 1 in, 3 out]
        n703 = property on="StartStopAxis" class="Str"("Val(Sgnl)"=w1244) -> ()  [unwired: 2 in, 2 out]
      }
      event "StartFreq1_CurLib", "StopFreq1_CurLib", "StartFreq2_CurLib", "StopFreq2_CurLib", "StopFreq6_CurLib", "StartFreq6_CurLib", "StopFreq7_CurLib", "StartFreq7_CurLib", "StopFreq8_CurLib", "StartFreq8_CurLib": Value Change {
        n704 = event-data() -> ("CtlRef"=w1249:refnum<vi>)  [unwired: 6 out]
        n705 = property class="Ring (strict)"(reference=w1249) -> ("Label.Text"=w1251:string)  [unwired: 1 in, 2 out]
        n706 = property on="Stimulus Out" class="Clust (strict)"() -> ("Value"=w1248:T2)  [unwired: 2 in, 2 out]
        n707 = property on="Stimulus Out" class="Clust (strict)"("Val(Sgnl)"=w1248) -> ()  [unwired: 2 in, 2 out]
        n708 = Match Pattern(string=w1251, regular expression="_CurLib" ("y")) -> (before substring=w1250:string)  [unwired: 1 in, 3 out]
        n709 = property on="StartStopAxis" class="Str"("Val(Sgnl)"=w1250) -> ()  [unwired: 2 in, 2 out]
      }
      event "StartStopAxis": Value Change {
        n710 = event-data() -> ("NewVal"=w1258:string)  [unwired: 6 out]
        n711 = control-ref of="This VI"() -> (w1281:refnum<vi>)
        n712 = Concatenate Strings(w1258, "_CurLib" ("string")) -> (w1280:string)
        n713 = Concatenate Strings(w1258, "_Value" ("string")) -> (w1278:string)
        n714 = Concatenate Strings(w1258, "_axis" ("string")) -> (w1257:string)
        n715 = Match Pattern(string=w1258, regular expression="Freq") -> (before substring=w1266:string, after substring=w1267:string)  [unwired: 1 in, 2 out]
        n716 = invoke class="VI" method="Ctrl Val.Get"(reference=w1281, "Control Name"=w1280) -> (reference out=w1260:refnum<vi>, "Get Control Value Variant"=w1277:variant)  [unwired: 2 in, 2 out]
        n717 = Decimal String To Number(string=w1267) -> (offset past number=w1269:i32)  [unwired: 2 in, 1 out]
        n718 = Variant To Data(type=u16 0 ("StartFreq1_CurLib"), Variant=w1277) -> (data=w1264:u16)  [unwired: 1 in, 1 out]
        n719 = case shown="1, Default" w1269 {
          tunnel: w1266 -> [w1284 w1288 w1292 w1296 w1300]
          tunnel: [w1283 w1287 w1291 w1295 w1299] -> w1265
          frame 1, Default {
            n720 = case shown="\"Start\"" w1284 {
              tunnel: [w1285 w1286] -> w1283
              frame "Stop", Default {
                n721 = property on="StopFreq1_CurLib" class="Ring (strict)"() -> ("Strings []"=w1285:string[])  [unwired: 2 in, 2 out]
              }
              frame "Start" {
                n722 = property on="StartFreq1_CurLib" class="Ring (strict)"() -> ("Strings []"=w1286:string[])  [unwired: 2 in, 2 out]
              }
            }
          }
          frame 2 {
            n723 = case shown="\"Start\"" w1288 {
              tunnel: [w1289 w1290] -> w1287
              frame "Stop", Default {
                n724 = property on="StopFreq2_CurLib" class="Ring (strict)"() -> ("Strings []"=w1289:string[])  [unwired: 2 in, 2 out]
              }
              frame "Start" {
                n725 = property on="StartFreq2_CurLib" class="Ring (strict)"() -> ("Strings []"=w1290:string[])  [unwired: 2 in, 2 out]
              }
            }
          }
          frame 6 {
            n726 = case shown="\"Stop\", Default" w1292 {
              tunnel: [w1293 w1294] -> w1291
              frame "Stop", Default {
                n727 = property on="StopFreq6_CurLib" class="Ring (strict)"() -> ("Strings []"=w1293:string[])  [unwired: 2 in, 2 out]
              }
              frame "Start" {
                n728 = property on="StartFreq6_CurLib" class="Ring (strict)"() -> ("Strings []"=w1294:string[])  [unwired: 2 in, 2 out]
              }
            }
          }
          frame 7 {
            n729 = case shown="\"Start\"" w1296 {
              tunnel: [w1297 w1298] -> w1295
              frame "Stop", Default {
                n730 = property on="StopFreq7_CurLib" class="Ring (strict)"() -> ("Strings []"=w1297:string[])  [unwired: 2 in, 2 out]
              }
              frame "Start" {
                n731 = property on="StartFreq7_CurLib" class="Ring (strict)"() -> ("Strings []"=w1298:string[])  [unwired: 2 in, 2 out]
              }
            }
          }
          frame 8 {
            n732 = case shown="\"Stop\", Default" w1300 {
              tunnel: [w1301 w1302] -> w1299
              frame "Stop", Default {
                n733 = property on="StopFreq8_CurLib" class="Ring (strict)"() -> ("Strings []"=w1301:string[])  [unwired: 2 in, 2 out]
              }
              frame "Start" {
                n734 = property on="StartFreq8_CurLib" class="Ring (strict)"() -> ("Strings []"=w1302:string[])  [unwired: 2 in, 2 out]
              }
            }
          }
        }
        n735 = invoke class="VI" method="Ctrl Val.Get"(reference=w1260, "Control Name"=w1257) -> (reference out=w1253:refnum<vi>, "Get Control Value Variant"=w1256:variant)  [unwired: 2 in, 2 out]
        n736 = Index Array(array=w1265, index=w1264) -> (element=w1263:string)
        n737 = Variant To Data(type=u16 0 ("StartFreq1_axis"), Variant=w1256) -> (data=w1254:u16)  [unwired: 1 in, 1 out]
        n738 = call "CRYGet Curve Library One Data .vi"("Data Name"=w1263, "Type"=enum16{"Curves", "Values", "Results", "WFM"}."Values") -> ("Value"=w1261:T6)  [unwired: 3 in, 6 out]
        n739 = Unbundle By Name(w1261) -> ("Curve"=w1276:cluster{"x":dbl, "y":dbl, "z":dbl}[])
        n740 = Index Array(array=w1276) -> (element=w1275:cluster{"x":dbl, "y":dbl, "z":dbl})  [unwired: 1 in]
        n741 = Unbundle By Name(w1275) -> ("x"=w1274:dbl, "y"=w1273:dbl, "z"=w1272:dbl)
        n742 = case shown="2" w1254 {
          tunnel: w1274 -> [w1303 _ _]
          tunnel: w1273 -> [_ w1304 _]
          tunnel: w1272 -> [_ _ w1305]
          tunnel: [w1303 w1304 w1305] -> w1271
          frame 0, Default {
          }
          frame 1 {
          }
          frame 2 {
          }
        }
        n743 = invoke class="VI" method="Ctrl Val.Set"(reference=w1253, "Control Name"=w1278, "Value"=w1271) -> ()  [unwired: 2 in, 5 out]
      }
      event "StartStopFreqValue": Value Change {
        n744 = event-data() -> ("NewVal"=w1309:string)  [unwired: 6 out]
        n745 = Match Pattern(string=w1309, regular expression="###" ("string")) -> (before substring=w1307:string, after substring=w1306:string)  [unwired: 1 in, 2 out]
        n746 = Match Pattern(string=w1307, regular expression="Freq" ("y")) -> (before substring=w1313:string, after substring=w1316:string)  [unwired: 1 in, 2 out]
        n747 = String Subset(string=w1316, length (rest)=1 ("length (rest)")) -> (substring=w1311:string)  [unwired: 1 in]
        n748 = Concatenate Strings(w1313, "Freq" ("y"), w1311) -> (w1310:string)
        n749 = Decimal String To Number(string=w1311) -> (number=w1314:i32)  [unwired: 2 in, 1 out]
        n750 = case shown="\"USER_INPUT\", Default" w1306 {
          tunnel: w1314 -> [w1320 w1347]
          tunnel: w1313 -> [w1319 w1346]
          tunnel: w1310 -> [w1318 _]
          frame "CURVE_VALUE" {
            n751 = case shown="1" w1320 {
              tunnel: w1319 -> [_ w1321 w1326 w1331 w1336 w1341]
              frame 0, Default {
              }
              frame 1 {
                n752 = case shown="\"Stop\"" w1321 {
                  frame "Start", Default {
                    w1323 = TRUE ("Visible")
                    n753 = property on="StartFreq1_CurLib" class="Ring (strict)"("Visible"=w1323) -> ()  [unwired: 2 in, 2 out]
                    n754 = property on="StartFreq1_axis" class="Slide (strict)"("Visible"=w1323) -> ()  [unwired: 2 in, 2 out]
                    n755 = property on="StartFreq1_Value" class="DigNum (strict)"("Visible"=w1323) -> ()  [unwired: 2 in, 2 out]
                    n756 = property on="StartFreq1(Hz)" class="DigNum (strict)"("Visible"=FALSE) -> ()  [unwired: 2 in, 2 out]
                  }
                  frame "Stop" {
                    w1324 = TRUE ("Visible")
                    n757 = property on="StopFreq1_CurLib" class="Ring (strict)"("Visible"=w1324) -> ()  [unwired: 2 in, 2 out]
                    n758 = property on="StopFreq1_axis" class="Slide (strict)"("Visible"=w1324) -> ()  [unwired: 2 in, 2 out]
                    n759 = property on="StopFreq1_Value" class="DigNum (strict)"("Visible"=w1324) -> ()  [unwired: 2 in, 2 out]
                    n760 = property on="StopFreq1(Hz)" class="DigNum (strict)"("Visible"=FALSE) -> ()  [unwired: 2 in, 2 out]
                  }
                }
              }
              frame 2 {
                n761 = case shown="\"Start\", Default" w1326 {
                  frame "Start", Default {
                    w1327 = TRUE ("Visible")
                    n762 = property on="StartFreq2_CurLib" class="Ring (strict)"("Visible"=w1327) -> ()  [unwired: 2 in, 2 out]
                    n763 = property on="StartFreq2_axis" class="Slide (strict)"("Visible"=w1327) -> ()  [unwired: 2 in, 2 out]
                    n764 = property on="StartFreq2_Value" class="DigNum (strict)"("Visible"=w1327) -> ()  [unwired: 2 in, 2 out]
                    n765 = property on="StartFreq2(Hz)" class="DigNum (strict)"("Visible"=FALSE) -> ()  [unwired: 2 in, 2 out]
                  }
                  frame "Stop" {
                    w1329 = TRUE ("Visible")
                    n766 = property on="StopFreq2_CurLib" class="Ring (strict)"("Visible"=w1329) -> ()  [unwired: 2 in, 2 out]
                    n767 = property on="StopFreq2_axis" class="Slide (strict)"("Visible"=w1329) -> ()  [unwired: 2 in, 2 out]
                    n768 = property on="StopFreq2_Value" class="DigNum (strict)"("Visible"=w1329) -> ()  [unwired: 2 in, 2 out]
                    n769 = property on="StopFreq2(Hz)" class="DigNum (strict)"("Visible"=FALSE) -> ()  [unwired: 2 in, 2 out]
                  }
                }
              }
              frame 6 {
                n770 = case shown="\"Stop\"" w1331 {
                  frame "Start", Default {
                    w1332 = TRUE ("Visible")
                    n771 = property on="StartFreq6_CurLib" class="Ring (strict)"("Visible"=w1332) -> ()  [unwired: 2 in, 2 out]
                    n772 = property on="StartFreq6_axis" class="Slide (strict)"("Visible"=w1332) -> ()  [unwired: 2 in, 2 out]
                    n773 = property on="StartFreq6_Value" class="DigNum (strict)"("Visible"=w1332) -> ()  [unwired: 2 in, 2 out]
                    n774 = property on="StartFreq6(Hz)" class="DigNum (strict)"("Visible"=FALSE) -> ()  [unwired: 2 in, 2 out]
                  }
                  frame "Stop" {
                    w1334 = TRUE ("Visible")
                    n775 = property on="StopFreq6(Hz)" class="DigNum (strict)"("Visible"=FALSE) -> ()  [unwired: 2 in, 2 out]
                    n776 = property on="StopFreq6_CurLib" class="Ring (strict)"("Visible"=w1334) -> ()  [unwired: 2 in, 2 out]
                    n777 = property on="StopFreq6_axis" class="Slide (strict)"("Visible"=w1334) -> ()  [unwired: 2 in, 2 out]
                    n778 = property on="StopFreq6_Value" class="DigNum (strict)"("Visible"=w1334) -> ()  [unwired: 2 in, 2 out]
                  }
                }
              }
              frame 7 {
                n779 = case shown="\"Stop\"" w1336 {
                  frame "Start", Default {
                    w1337 = TRUE ("Visible")
                    n780 = property on="StartFreq7(Hz)" class="DigNum (strict)"("Visible"=FALSE) -> ()  [unwired: 2 in, 2 out]
                    n781 = property on="StartFreq7_CurLib" class="Ring (strict)"("Visible"=w1337) -> ()  [unwired: 2 in, 2 out]
                    n782 = property on="StartFreq7_axis" class="Slide (strict)"("Visible"=w1337) -> ()  [unwired: 2 in, 2 out]
                    n783 = property on="StartFreq7_Value" class="DigNum (strict)"("Visible"=w1337) -> ()  [unwired: 2 in, 2 out]
                  }
                  frame "Stop" {
                    w1339 = TRUE ("Visible")
                    n784 = property on="StopFreq7_CurLib" class="Ring (strict)"("Visible"=w1339) -> ()  [unwired: 2 in, 2 out]
                    n785 = property on="StopFreq7_axis" class="Slide (strict)"("Visible"=w1339) -> ()  [unwired: 2 in, 2 out]
                    n786 = property on="StopFreq7_Value" class="DigNum (strict)"("Visible"=w1339) -> ()  [unwired: 2 in, 2 out]
                    n787 = property on="StopFreq7(Hz)" class="DigNum (strict)"("Visible"=FALSE) -> ()  [unwired: 2 in, 2 out]
                  }
                }
              }
              frame 8 {
                n788 = case shown="\"Start\", Default" w1341 {
                  frame "Start", Default {
                    w1342 = TRUE ("Visible")
                    n789 = property on="StartFreq8(Hz)" class="DigNum (strict)"("Visible"=FALSE) -> ()  [unwired: 2 in, 2 out]
                    n790 = property on="StartFreq8_CurLib" class="Ring (strict)"("Visible"=w1342) -> ()  [unwired: 2 in, 2 out]
                    n791 = property on="StartFreq8_axis" class="Slide (strict)"("Visible"=w1342) -> ()  [unwired: 2 in, 2 out]
                    n792 = property on="StartFreq8_Value" class="DigNum (strict)"("Visible"=w1342) -> ()  [unwired: 2 in, 2 out]
                  }
                  frame "Stop" {
                    w1344 = TRUE ("Visible")
                    n793 = property on="StopFreq8_CurLib" class="Ring (strict)"("Visible"=w1344) -> ()  [unwired: 2 in, 2 out]
                    n794 = property on="StopFreq8_axis" class="Slide (strict)"("Visible"=w1344) -> ()  [unwired: 2 in, 2 out]
                    n795 = property on="StopFreq8_Value" class="DigNum (strict)"("Visible"=w1344) -> ()  [unwired: 2 in, 2 out]
                    n796 = property on="StopFreq8(Hz)" class="DigNum (strict)"("Visible"=FALSE) -> ()  [unwired: 2 in, 2 out]
                  }
                }
              }
            }
            n797 = property on="StartStopAxis" class="Str"("Val(Sgnl)"=w1318) -> ()  [unwired: 2 in, 2 out]
          }
          frame "USER_INPUT", Default {
            n798 = case shown="1" w1347 {
              tunnel: w1346 -> [_ w1348 w1353 w1358 w1363 w1368]
              frame 0, Default {
              }
              frame 1 {
                n799 = case shown="\"Stop\"" w1348 {
                  frame "Start", Default {
                    w1350 = FALSE ("Visible")
                    n800 = property on="StartFreq1_CurLib" class="Ring (strict)"("Visible"=w1350) -> ()  [unwired: 2 in, 2 out]
                    n801 = property on="StartFreq1_axis" class="Slide (strict)"("Visible"=w1350) -> ()  [unwired: 2 in, 2 out]
                    n802 = property on="StartFreq1_Value" class="DigNum (strict)"("Visible"=w1350) -> ()  [unwired: 2 in, 2 out]
                    n803 = property on="StartFreq1(Hz)" class="DigNum (strict)"("Visible"=TRUE) -> ()  [unwired: 2 in, 2 out]
                  }
                  frame "Stop" {
                    w1351 = FALSE ("Visible")
                    n804 = property on="StopFreq1_CurLib" class="Ring (strict)"("Visible"=w1351) -> ()  [unwired: 2 in, 2 out]
                    n805 = property on="StopFreq1_axis" class="Slide (strict)"("Visible"=w1351) -> ()  [unwired: 2 in, 2 out]
                    n806 = property on="StopFreq1_Value" class="DigNum (strict)"("Visible"=w1351) -> ()  [unwired: 2 in, 2 out]
                    n807 = property on="StopFreq1(Hz)" class="DigNum (strict)"("Visible"=TRUE) -> ()  [unwired: 2 in, 2 out]
                  }
                }
              }
              frame 2 {
                n808 = case shown="\"Start\", Default" w1353 {
                  frame "Start", Default {
                    w1354 = FALSE ("Visible")
                    n809 = property on="StartFreq2_CurLib" class="Ring (strict)"("Visible"=w1354) -> ()  [unwired: 2 in, 2 out]
                    n810 = property on="StartFreq2_axis" class="Slide (strict)"("Visible"=w1354) -> ()  [unwired: 2 in, 2 out]
                    n811 = property on="StartFreq2_Value" class="DigNum (strict)"("Visible"=w1354) -> ()  [unwired: 2 in, 2 out]
                    n812 = property on="StartFreq2(Hz)" class="DigNum (strict)"("Visible"=TRUE) -> ()  [unwired: 2 in, 2 out]
                  }
                  frame "Stop" {
                    w1356 = FALSE ("Visible")
                    n813 = property on="StopFreq2_CurLib" class="Ring (strict)"("Visible"=w1356) -> ()  [unwired: 2 in, 2 out]
                    n814 = property on="StopFreq2_axis" class="Slide (strict)"("Visible"=w1356) -> ()  [unwired: 2 in, 2 out]
                    n815 = property on="StopFreq2_Value" class="DigNum (strict)"("Visible"=w1356) -> ()  [unwired: 2 in, 2 out]
                    n816 = property on="StopFreq2(Hz)" class="DigNum (strict)"("Visible"=TRUE) -> ()  [unwired: 2 in, 2 out]
                  }
                }
              }
              frame 6 {
                n817 = case shown="\"Stop\"" w1358 {
                  frame "Start", Default {
                    w1359 = FALSE ("Visible")
                    n818 = property on="StartFreq6_CurLib" class="Ring (strict)"("Visible"=w1359) -> ()  [unwired: 2 in, 2 out]
                    n819 = property on="StartFreq6_axis" class="Slide (strict)"("Visible"=w1359) -> ()  [unwired: 2 in, 2 out]
                    n820 = property on="StartFreq6_Value" class="DigNum (strict)"("Visible"=w1359) -> ()  [unwired: 2 in, 2 out]
                    n821 = property on="StartFreq6(Hz)" class="DigNum (strict)"("Visible"=TRUE) -> ()  [unwired: 2 in, 2 out]
                  }
                  frame "Stop" {
                    w1361 = FALSE ("Visible")
                    n822 = property on="StopFreq6(Hz)" class="DigNum (strict)"("Visible"=TRUE) -> ()  [unwired: 2 in, 2 out]
                    n823 = property on="StopFreq6_CurLib" class="Ring (strict)"("Visible"=w1361) -> ()  [unwired: 2 in, 2 out]
                    n824 = property on="StopFreq6_axis" class="Slide (strict)"("Visible"=w1361) -> ()  [unwired: 2 in, 2 out]
                    n825 = property on="StopFreq6_Value" class="DigNum (strict)"("Visible"=w1361) -> ()  [unwired: 2 in, 2 out]
                  }
                }
              }
              frame 7 {
                n826 = case shown="\"Start\", Default" w1363 {
                  frame "Start", Default {
                    w1364 = FALSE ("Visible")
                    n827 = property on="StartFreq7(Hz)" class="DigNum (strict)"("Visible"=TRUE) -> ()  [unwired: 2 in, 2 out]
                    n828 = property on="StartFreq7_CurLib" class="Ring (strict)"("Visible"=w1364) -> ()  [unwired: 2 in, 2 out]
                    n829 = property on="StartFreq7_axis" class="Slide (strict)"("Visible"=w1364) -> ()  [unwired: 2 in, 2 out]
                    n830 = property on="StartFreq7_Value" class="DigNum (strict)"("Visible"=w1364) -> ()  [unwired: 2 in, 2 out]
                  }
                  frame "Stop" {
                    w1366 = FALSE ("Visible")
                    n831 = property on="StopFreq7_CurLib" class="Ring (strict)"("Visible"=w1366) -> ()  [unwired: 2 in, 2 out]
                    n832 = property on="StopFreq7_axis" class="Slide (strict)"("Visible"=w1366) -> ()  [unwired: 2 in, 2 out]
                    n833 = property on="StopFreq7_Value" class="DigNum (strict)"("Visible"=w1366) -> ()  [unwired: 2 in, 2 out]
                    n834 = property on="StopFreq7(Hz)" class="DigNum (strict)"("Visible"=TRUE) -> ()  [unwired: 2 in, 2 out]
                  }
                }
              }
              frame 8 {
                n835 = case shown="\"Stop\"" w1368 {
                  frame "Start", Default {
                    w1369 = FALSE ("Visible")
                    n836 = property on="StartFreq8(Hz)" class="DigNum (strict)"("Visible"=TRUE) -> ()  [unwired: 2 in, 2 out]
                    n837 = property on="StartFreq8_CurLib" class="Ring (strict)"("Visible"=w1369) -> ()  [unwired: 2 in, 2 out]
                    n838 = property on="StartFreq8_axis" class="Slide (strict)"("Visible"=w1369) -> ()  [unwired: 2 in, 2 out]
                    n839 = property on="StartFreq8_Value" class="DigNum (strict)"("Visible"=w1369) -> ()  [unwired: 2 in, 2 out]
                  }
                  frame "Stop" {
                    w1371 = FALSE ("Visible")
                    n840 = property on="StopFreq8_CurLib" class="Ring (strict)"("Visible"=w1371) -> ()  [unwired: 2 in, 2 out]
                    n841 = property on="StopFreq8_axis" class="Slide (strict)"("Visible"=w1371) -> ()  [unwired: 2 in, 2 out]
                    n842 = property on="StopFreq8_Value" class="DigNum (strict)"("Visible"=w1371) -> ()  [unwired: 2 in, 2 out]
                    n843 = property on="StopFreq8(Hz)" class="DigNum (strict)"("Visible"=TRUE) -> ()  [unwired: 2 in, 2 out]
                  }
                }
              }
            }
          }
        }
      }
      event "ML val level name": Value Change {
        n844 = event-data() -> ()  [unwired: 7 out]
        n845 = property on="ML val level name" class="Ring (strict)"() -> ("RingText.Text"=w1378:string)  [unwired: 2 in, 2 out]
        n846 = Build Array(w1378) -> (w1377:string[])
        n847 = Bundle By Name(cluster=w1373, "MLValLevelNameArray"=w1377) -> (w1376:T2)
        n848 = Unbundle By Name(w1376) -> ("ML_axisArray"=w1375:u16[])
        n849 = property on="Stimulus Out" class="Clust (strict)"("Val(Sgnl)"=w1376) -> ()  [unwired: 2 in, 2 out]
        n850 = Index Array(array=w1375) -> (element=w1374:u16)  [unwired: 1 in]
        n851 = property on="ML axis1" class="Slide (strict)"("Val(Sgnl)"=w1374) -> ()  [unwired: 2 in, 2 out]
      }
      event "ML val level name2": Value Change {
        n852 = event-data() -> ()  [unwired: 7 out]
        n853 = property on="ML val level name2" class="Ring (strict)"() -> ("RingText.Text"=w1383:string)  [unwired: 2 in, 2 out]
        n854 = Build Array(w1383) -> (w1384:string[])
        n855 = Bundle By Name(cluster=w1379, "MLValLevelNameArray"=w1384) -> (w1381:T2)
        n856 = Unbundle By Name(w1381) -> ("ML_axisArray"=w1382:u16[])
        n857 = property on="Stimulus Out" class="Clust (strict)"("Val(Sgnl)"=w1381) -> ()  [unwired: 2 in, 2 out]
        n858 = Index Array(array=w1382) -> (element=w1380:u16)  [unwired: 1 in]
        n859 = property on="ML axis2" class="Slide (strict)"("Val(Sgnl)"=w1380) -> ()  [unwired: 2 in, 2 out]
      }
      event "ML val level name3": Value Change {
        n860 = event-data() -> ()  [unwired: 7 out]
        n861 = property on="ML val level name3" class="Ring (strict)"() -> ("RingText.Text"=w1389:string)  [unwired: 2 in, 2 out]
        n862 = Build Array(w1389) -> (w1390:string[])
        n863 = Bundle By Name(cluster=w1385, "MLValLevelNameArray"=w1390) -> (w1387:T2)
        n864 = Unbundle By Name(w1387) -> ("ML_axisArray"=w1388:u16[])
        n865 = property on="Stimulus Out" class="Clust (strict)"("Val(Sgnl)"=w1387) -> ()  [unwired: 2 in, 2 out]
        n866 = Index Array(array=w1388) -> (element=w1386:u16)  [unwired: 1 in]
        n867 = property on="ML axis3" class="Slide (strict)"("Val(Sgnl)"=w1386) -> ()  [unwired: 2 in, 2 out]
      }
      event "ML val level name4": Value Change {
        n868 = event-data() -> ()  [unwired: 7 out]
        n869 = property on="ML val level name4" class="Ring (strict)"() -> ("RingText.Text"=w1395:string)  [unwired: 2 in, 2 out]
        n870 = Build Array(w1395) -> (w1396:string[])
        n871 = Bundle By Name(cluster=w1391, "MLValLevelNameArray"=w1396) -> (w1393:T2)
        n872 = Unbundle By Name(w1393) -> ("ML_axisArray"=w1394:u16[])
        n873 = property on="Stimulus Out" class="Clust (strict)"("Val(Sgnl)"=w1393) -> ()  [unwired: 2 in, 2 out]
        n874 = Index Array(array=w1394) -> (element=w1392:u16)  [unwired: 1 in]
        n875 = property on="ML axis4" class="Slide (strict)"("Val(Sgnl)"=w1392) -> ()  [unwired: 2 in, 2 out]
      }
      event "ML val level name6_1": Value Change {
        n876 = event-data() -> ()  [unwired: 7 out]
        n877 = property on="ML val level name6_1" class="Ring (strict)"() -> ("RingText.Text"=w1401:string)  [unwired: 2 in, 2 out]
        n878 = Build Array(w1401) -> (w1402:string[])
        n879 = Bundle By Name(cluster=w1397, "MLValLevelNameArray"=w1402) -> (w1399:T2)
        n880 = Unbundle By Name(w1399) -> ("ML_axisArray"=w1400:u16[])
        n881 = property on="Stimulus Out" class="Clust (strict)"("Val(Sgnl)"=w1399) -> ()  [unwired: 2 in, 2 out]
        n882 = Index Array(array=w1400) -> (element=w1398:u16)  [unwired: 1 in]
        n883 = property on="ML axis6_1" class="Slide (strict)"("Val(Sgnl)"=w1398) -> ()  [unwired: 2 in, 2 out]
      }
      event "ML val level name6_2": Value Change {
        n884 = event-data() -> ()  [unwired: 7 out]
        n885 = property on="ML val level name6_2" class="Ring (strict)"() -> ("RingText.Text"=w1407:string)  [unwired: 2 in, 2 out]
        n886 = Build Array(w1407) -> (w1408:string[])
        n887 = Bundle By Name(cluster=w1403, "MLValLevelNameArray"=w1408) -> (w1405:T2)
        n888 = Unbundle By Name(w1405) -> ("ML_axisArray"=w1406:u16[])
        n889 = property on="Stimulus Out" class="Clust (strict)"("Val(Sgnl)"=w1405) -> ()  [unwired: 2 in, 2 out]
        n890 = Index Array(array=w1406) -> (element=w1404:u16)  [unwired: 1 in]
        n891 = property on="ML axis6_2" class="Slide (strict)"("Val(Sgnl)"=w1404) -> ()  [unwired: 2 in, 2 out]
      }
      event "ML val level name7": Value Change {
        n892 = event-data() -> ()  [unwired: 7 out]
        n893 = property on="ML val level name7" class="Ring (strict)"() -> ("RingText.Text"=w1413:string)  [unwired: 2 in, 2 out]
        n894 = Build Array(w1413) -> (w1414:string[])
        n895 = Bundle By Name(cluster=w1409, "MLValLevelNameArray"=w1414) -> (w1411:T2)
        n896 = Unbundle By Name(w1411) -> ("ML_axisArray"=w1412:u16[])
        n897 = property on="Stimulus Out" class="Clust (strict)"("Val(Sgnl)"=w1411) -> ()  [unwired: 2 in, 2 out]
        n898 = Index Array(array=w1412) -> (element=w1410:u16)  [unwired: 1 in]
        n899 = property on="ML axis7" class="Slide (strict)"("Val(Sgnl)"=w1410) -> ()  [unwired: 2 in, 2 out]
      }
      event "ML val level name8": Value Change {
        n900 = event-data() -> ()  [unwired: 7 out]
        n901 = property on="ML val level name8" class="Ring (strict)"() -> ("RingText.Text"=w1419:string)  [unwired: 2 in, 2 out]
        n902 = Build Array(w1419) -> (w1420:string[])
        n903 = Bundle By Name(cluster=w1415, "MLValLevelNameArray"=w1420) -> (w1417:T2)
        n904 = Unbundle By Name(w1417) -> ("ML_axisArray"=w1418:u16[])
        n905 = property on="Stimulus Out" class="Clust (strict)"("Val(Sgnl)"=w1417) -> ()  [unwired: 2 in, 2 out]
        n906 = Index Array(array=w1418) -> (element=w1416:u16)  [unwired: 1 in]
        n907 = property on="ML axis8" class="Slide (strict)"("Val(Sgnl)"=w1416) -> ()  [unwired: 2 in, 2 out]
      }
      event "StartFreq1(Hz)": Value Change {
        n908 = event-data() -> ("NewVal"=w1429:dbl)  [unwired: 6 out]
        n909 = property on="Step Resolution1" class="Ring (strict)"() -> ("Value"=w1422:u16)  [unwired: 2 in, 2 out]
        n910 = property on="Res Max Freq" class="DigNum (strict)"() -> ("Value"=w1421:dbl)  [unwired: 2 in, 2 out]
        n911 = call "CRYStimulus Freq Max Limit.vi"("Resolution"=w1422, "Max Freq"=w1421, "Input Val"=w1429) -> ("Decrement Val"=w1427:dbl, "Output Val"=w1428:dbl)  [unwired: 1 in, 6 out]
        n912 = property on="StartFreq1(Hz)" class="DigNum (strict)"("Increment"=w1427) -> ()  [unwired: 2 in, 2 out]
        n913 = property on="StopFreq1(Hz)" class="DigNum (strict)"() -> ("Value"=w1439:dbl)  [unwired: 2 in, 2 out]
        n914 = property on="Steps1" class="DigNum (strict)"() -> ("Value"=w1424:i32)  [unwired: 2 in, 2 out]
        n915 = call "CRYGet Steps From F1 F2 Resolution.vi"("Steps/Tone"=w1424, "Stop Freq"=w1439, "Start Freq"=w1428, "Resolution"=w1422) -> ("Start Freq Out"=w1431:dbl, "Steps"=w1423:i32)  [unwired: 6 out]
        n916 = property on="StartFreq1(Hz)" class="DigNum (strict)"("Value"=w1431) -> ()  [unwired: 2 in, 2 out]
        n917 = property on="Steps1" class="DigNum (strict)"("Value"=w1423) -> ()  [unwired: 2 in, 2 out]
        n918 = Unbundle By Name(w1426) -> ("Start(Stop)FreqArray"=w1435:dbl[])
        n919 = case shown="Default" w1422 {
          tunnel: w1439 -> [_ w1452]
          tunnel: w1431 -> [_ w1451]
          tunnel: [w1443 w1447] -> w1425
          tunnel: w1423 -> [w1442 _]
          frame Default {
            n920 = Less Or Equal?(x=w1442, y=1) -> (x <= y?=w1446:bool)
            n921 = Select(t=u8 2 ("Disabled"), s=w1446, f=u8 0 ("Disabled")) -> (s? t:f=w1443:u8)
          }
          frame 0..3 {
            n922 = Equal?(x=w1451, y=w1452) -> (x = y?=w1450:bool)
            n923 = Select(t=u8 2 ("Disabled"), s=w1450, f=u8 0 ("Disabled")) -> (s? t:f=w1447:u8)
          }
        }
        n924 = Index Array(array=w1435, index=1) -> (element=w1432:dbl)
        n925 = Index Array(array=w1435, index=2) -> (element=w1433:dbl)
        n926 = Index Array(array=w1435, index=3) -> (element=w1434:dbl)
        n927 = Build Array(w1431, w1432, w1433, w1434) -> (w1430:dbl[])
        n928 = Bundle By Name(cluster=w1426, "Start(Stop)FreqArray"=w1430, "Steps1"=w1423) -> (w1440:T2)
        n929 = property on="StartFreq1(Hz)" class="DigNum (strict)"("Disabled"=w1425) -> ()  [unwired: 2 in, 2 out]
        n930 = property on="Stimulus Out" class="Clust (strict)"("Val(Sgnl)"=w1440) -> ()  [unwired: 2 in, 2 out]
      }
      event "StartFreq2(Hz)": Value Change {
        w1456 = 0.001 ("y")
        n931 = event-data() -> ("NewVal"=w1455:dbl)  [unwired: 6 out]
        n932 = Less?(x=w1455, y=w1456) -> (x < y?=w1457:bool)
        n933 = case shown="False" w1457 {
          tunnel: [w1470 w1471] -> w1454
          tunnel: w1456 -> [_ w1471]
          tunnel: w1455 -> [w1468 _]
          frame False {
            n934 = property on="Res Max Freq" class="DigNum (strict)"() -> ("Value"=w1467:dbl)  [unwired: 2 in, 2 out]
            n935 = Less?(x=w1468, y=w1467) -> (x < y?=w1469:bool)
            n936 = Select(t=w1468, s=w1469, f=w1467) -> (s? t:f=w1470:dbl)
          }
          frame True {
          }
        }
        n937 = Unbundle By Name(w1453) -> ("Start(Stop)FreqArray"=w1462:dbl[])
        n938 = property on="StartFreq2(Hz)" class="DigNum (strict)"("Value"=w1454) -> ()  [unwired: 2 in, 2 out]
        n939 = Index Array(array=w1462, index=0) -> (element=w1461:dbl)
        n940 = Index Array(array=w1462, index=1) -> (element=w1460:dbl)
        n941 = Index Array(array=w1462, index=3) -> (element=w1459:dbl)
        n942 = Build Array(w1461, w1460, w1454, w1459) -> (w1458:dbl[])
        n943 = Bundle By Name(cluster=w1453, "Start(Stop)FreqArray"=w1458) -> (w1466:T2)
        n944 = property on="Stimulus Out" class="Clust (strict)"("Val(Sgnl)"=w1466) -> ()  [unwired: 2 in, 2 out]
      }
      event "StartFreq6(Hz)": Value Change {
        n945 = event-data() -> ("NewVal"=w1492:dbl)  [unwired: 6 out]
        n946 = property on="StepResolution6" class="Ring (strict)"() -> ("Value"=w1479:u16)  [unwired: 2 in, 2 out]
        n947 = property on="Res Max Freq" class="DigNum (strict)"() -> ("Value"=w1493:dbl)  [unwired: 2 in, 2 out]
        n948 = call "CRYStimulus Freq Max Limit.vi"("Resolution"=w1479, "Max Freq"=w1493, "Input Val"=w1492) -> ("Decrement Val"=w1478:dbl, "Output Val"=w1484:dbl)  [unwired: 1 in, 6 out]
        n949 = Unbundle By Name(w1477) -> ("Start(Stop)FreqArray"=w1486:dbl[])
        n950 = property on="StartFreq6(Hz)" class="DigNum (strict)"("Increment"=w1478) -> ()  [unwired: 2 in, 2 out]
        n951 = property on="StopFreq6(Hz)" class="DigNum (strict)"() -> ("Value"=w1490:dbl)  [unwired: 2 in, 2 out]
        n952 = Index Array(array=w1486, index=1) -> (element=w1483:dbl)
        n953 = Index Array(array=w1486, index=2) -> (element=w1482:dbl)
        n954 = Index Array(array=w1486, index=3) -> (element=w1481:dbl)
        n955 = property on="Steps6" class="DigNum (strict)"() -> ("Value"=w1472:i32)  [unwired: 2 in, 2 out]
        n956 = Build Array(w1484, w1483, w1482, w1481) -> (w1485:dbl[])
        n957 = call "CRYGet Steps From F1 F2 Resolution.vi"("Steps/Tone"=w1472, "Stop Freq"=w1490, "Start Freq"=w1484, "Resolution"=w1479) -> ("Start Freq Out"=w1491:dbl, "Steps"=w1480:i32)  [unwired: 6 out]
        n958 = Bundle By Name(cluster=w1477, "Start(Stop)FreqArray"=w1485, "Steps6(#)"=w1480) -> (w1494:T2)
        n959 = Equal?(x=w1491, y=w1490) -> (x = y?=w1476:bool)
        n960 = property on="StartFreq6(Hz)" class="DigNum (strict)"("Value"=w1491) -> ()  [unwired: 2 in, 2 out]
        n961 = property on="Steps6" class="DigNum (strict)"("Value"=w1480) -> ()  [unwired: 2 in, 2 out]
        n962 = Select(t=u8 2 ("Disabled"), s=w1476, f=u8 0 ("Disabled")) -> (s? t:f=w1473:u8)
        n963 = property on="Stimulus Out" class="Clust (strict)"("Val(Sgnl)"=w1494) -> ()  [unwired: 2 in, 2 out]
        n964 = property on="StartFreq6(Hz)" class="DigNum (strict)"("Disabled"=w1473) -> ()  [unwired: 2 in, 2 out]
      }
      event "StopFreq1(Hz)": Value Change {
        n965 = event-data() -> ("NewVal"=w1502:dbl)  [unwired: 6 out]
        n966 = property on="Res Max Freq" class="DigNum (strict)"() -> ("Value"=w1503:dbl)  [unwired: 2 in, 2 out]
        n967 = property on="Step Resolution1" class="Ring (strict)"() -> ("Value"=w1496:u16)  [unwired: 2 in, 2 out]
        n968 = call "CRYStimulus Freq Max Limit.vi"("Resolution"=w1496, "Max Freq"=w1503, "Input Val"=w1502) -> ("Decrement Val"=w1500:dbl, "Output Val"=w1501:dbl)  [unwired: 1 in, 6 out]
        n969 = Unbundle By Name(w1499) -> ("Start(Stop)FreqArray"=w1509:dbl[])
        n970 = property on="StopFreq1(Hz)" class="DigNum (strict)"("Increment"=w1500) -> ()  [unwired: 2 in, 2 out]
        n971 = property on="StartFreq1(Hz)" class="DigNum (strict)"() -> ("Value"=w1513:dbl)  [unwired: 2 in, 2 out]
        n972 = property on="Steps1" class="DigNum (strict)"() -> ("Value"=w1497:i32)  [unwired: 2 in, 2 out]
        n973 = Index Array(array=w1509, index=0) -> (element=w1507:dbl)
        n974 = Index Array(array=w1509, index=2) -> (element=w1506:dbl)
        n975 = Index Array(array=w1509, index=3) -> (element=w1505:dbl)
        n976 = call "CRYGet Steps From F1 F2 Resolution.vi"("Steps/Tone"=w1497, "Stop Freq"=w1501, "Start Freq"=w1513, "Resolution"=w1496) -> ("Stop Freq Out"=w1508:dbl, "Steps"=w1495:i32)  [unwired: 6 out]
        n977 = Build Array(w1507, w1508, w1506, w1505) -> (w1504:dbl[])
        n978 = property on="StopFreq1(Hz)" class="DigNum (strict)"("Value"=w1508) -> ()  [unwired: 2 in, 2 out]
        n979 = property on="Steps1" class="DigNum (strict)"("Value"=w1495) -> ()  [unwired: 2 in, 2 out]
        n980 = case shown="Default" w1496 {
          tunnel: w1513 -> [_ w1526]
          tunnel: w1508 -> [_ w1525]
          tunnel: [w1517 w1521] -> w1498
          tunnel: w1495 -> [w1516 _]
          frame Default {
            n981 = Less Or Equal?(x=w1516, y=1) -> (x <= y?=w1519:bool)
            n982 = Select(t=u8 2 ("Disabled"), s=w1519, f=u8 0 ("Disabled")) -> (s? t:f=w1517:u8)
          }
          frame 0..3 {
            n983 = Equal?(x=w1525, y=w1526) -> (x = y?=w1523:bool)
            n984 = Select(t=u8 2 ("Disabled"), s=w1523, f=u8 0 ("Disabled")) -> (s? t:f=w1521:u8)
          }
        }
        n985 = Bundle By Name(cluster=w1499, "Start(Stop)FreqArray"=w1504, "Steps1"=w1495) -> (w1514:T2)
        n986 = property on="StartFreq1(Hz)" class="DigNum (strict)"("Disabled"=w1498) -> ()  [unwired: 2 in, 2 out]
        n987 = property on="Stimulus Out" class="Clust (strict)"("Val(Sgnl)"=w1514) -> ()  [unwired: 2 in, 2 out]
      }
      event "StopFreq2(Hz)": Value Change {
        w1530 = 0.001 ("y")
        n988 = event-data() -> ("NewVal"=w1529:dbl)  [unwired: 6 out]
        n989 = Less?(x=w1529, y=w1530) -> (x < y?=w1531:bool)
        n990 = case shown="False" w1531 {
          tunnel: [w1544 w1545] -> w1528
          tunnel: w1530 -> [_ w1545]
          tunnel: w1529 -> [w1542 _]
          frame False {
            n991 = property on="Res Max Freq" class="DigNum (strict)"() -> ("Value"=w1541:dbl)  [unwired: 2 in, 2 out]
            n992 = Less?(x=w1542, y=w1541) -> (x < y?=w1543:bool)
            n993 = Select(t=w1542, s=w1543, f=w1541) -> (s? t:f=w1544:dbl)
          }
          frame True {
          }
        }
        n994 = property on="StopFreq2(Hz)" class="DigNum (strict)"("Value"=w1528) -> ()  [unwired: 2 in, 2 out]
        n995 = Unbundle By Name(w1527) -> ("Start(Stop)FreqArray"=w1536:dbl[])
        n996 = Index Array(array=w1536, index=0) -> (element=w1535:dbl)
        n997 = Index Array(array=w1536, index=1) -> (element=w1534:dbl)
        n998 = Index Array(array=w1536, index=2) -> (element=w1533:dbl)
        n999 = Build Array(w1535, w1534, w1533, w1528) -> (w1532:dbl[])
        n1000 = Bundle By Name(cluster=w1527, "Start(Stop)FreqArray"=w1532) -> (w1540:T2)
        n1001 = property on="Stimulus Out" class="Clust (strict)"("Val(Sgnl)"=w1540) -> ()  [unwired: 2 in, 2 out]
      }
      event "StopFreq6(Hz)": Value Change {
        n1002 = event-data() -> ("NewVal"=w1566:dbl)  [unwired: 6 out]
        n1003 = property on="StepResolution6" class="Ring (strict)"() -> ("Value"=w1553:u16)  [unwired: 2 in, 2 out]
        n1004 = property on="Res Max Freq" class="DigNum (strict)"() -> ("Value"=w1567:dbl)  [unwired: 2 in, 2 out]
        n1005 = Unbundle By Name(w1551) -> ("Start(Stop)FreqArray"=w1560:dbl[])
        n1006 = call "CRYStimulus Freq Max Limit.vi"("Resolution"=w1553, "Max Freq"=w1567, "Input Val"=w1566) -> ("Decrement Val"=w1552:dbl, "Output Val"=w1559:dbl)  [unwired: 1 in, 6 out]
        n1007 = property on="StopFreq6(Hz)" class="DigNum (strict)"("Increment"=w1552) -> ()  [unwired: 2 in, 2 out]
        n1008 = property on="StartFreq6(Hz)" class="DigNum (strict)"() -> ("Value"=w1564:dbl)  [unwired: 2 in, 2 out]
        n1009 = property on="Steps6" class="DigNum (strict)"() -> ("Value"=w1546:i32)  [unwired: 2 in, 2 out]
        n1010 = Index Array(array=w1560, index=0) -> (element=w1558:dbl)
        n1011 = Index Array(array=w1560, index=2) -> (element=w1557:dbl)
        n1012 = Index Array(array=w1560, index=3) -> (element=w1556:dbl)
        n1013 = Build Array(w1558, w1559, w1557, w1556) -> (w1555:dbl[])
        n1014 = call "CRYGet Steps From F1 F2 Resolution.vi"("Steps/Tone"=w1546, "Stop Freq"=w1559, "Start Freq"=w1564, "Resolution"=w1553) -> ("Stop Freq Out"=w1565:dbl, "Steps"=w1554:i32)  [unwired: 6 out]
        n1015 = Bundle By Name(cluster=w1551, "Start(Stop)FreqArray"=w1555, "Steps6(#)"=w1554) -> (w1568:T2)
        n1016 = Equal?(x=w1565, y=w1564) -> (x = y?=w1550:bool)
        n1017 = property on="StopFreq6(Hz)" class="DigNum (strict)"("Value"=w1565) -> ()  [unwired: 2 in, 2 out]
        n1018 = property on="Steps6" class="DigNum (strict)"("Value"=w1554) -> ()  [unwired: 2 in, 2 out]
        n1019 = Select(t=u8 2 ("Disabled"), s=w1550, f=u8 0 ("Disabled")) -> (s? t:f=w1547:u8)
        n1020 = property on="StartFreq6(Hz)" class="DigNum (strict)"("Disabled"=w1547) -> ()  [unwired: 2 in, 2 out]
        n1021 = property on="Stimulus Out" class="Clust (strict)"("Val(Sgnl)"=w1568) -> ()  [unwired: 2 in, 2 out]
      }
      event "Level(U)1": Value Change {
        n1022 = event-data() -> ("NewVal"=w1579:dbl)  [unwired: 6 out]
        n1023 = local read "MaxLevel_1"() -> (w1578:dbl)
        n1024 = local read "MaxLevel_2"() -> (w1577:dbl)
        n1025 = property on="unit1" class="Ring (strict)"() -> ("Value"=w1580:u16)  [unwired: 2 in, 2 out]
        n1026 = case shown="0, Default" w1580 {
          tunnel: w1579 -> [w1585 w1594]
          tunnel: [w1583 w1592] -> w1571
          tunnel: w1578 -> [w1584 _]
          tunnel: w1577 -> [_ w1593]
          tunnel: w1576 -> [_ w1598]
          tunnel: w1575 -> [_ w1597]
          tunnel: [w1583 w1596] -> w1574
          frame 0, Default {
            n1027 = Less Than 0?(x=w1585) -> (x < 0?=w1586:bool)
            n1028 = case shown="False" w1586 {
              tunnel: [w1587 0.0 ("y")] -> w1583
              tunnel: w1585 -> [w1589 _]
              tunnel: w1584 -> [w1588 _]
              frame False {
                n1029 = Less?(x=w1589, y=w1588) -> (x < y?=w1590:bool)
                n1030 = Select(t=w1589, s=w1590, f=w1588) -> (s? t:f=w1587:dbl)
              }
              frame True {
              }
            }
          }
          frame 1 {
            n1031 = Less?(x=w1594, y=w1593) -> (x < y?=w1595:bool)
            n1032 = Select(t=w1594, s=w1595, f=w1593) -> (s? t:f=w1592:dbl)
            n1033 = call "CRYConversion dB-Lin.vi"("unit prefix"=w1597, "dB ref."=w1598, "Log In"=w1592) -> ("Lin Out"=w1596:dbl)  [unwired: 3 in, 3 out]
          }
        }
        n1034 = Unbundle By Name(w1569) -> ("Level(U)Array"=w1573:dbl[])
        n1035 = Index Array(array=w1573, index=1) -> (element=w1570:dbl)
        n1036 = property on="Level(U)1" class="DigNum (strict)"("Value"=w1571) -> ()  [unwired: 2 in, 2 out]
        n1037 = property on="LinLevel1" class="DigNum (strict)"("Value"=w1574) -> ()  [unwired: 2 in, 2 out]
        n1038 = Build Array(w1571, w1570) -> (w1581:dbl[])
        n1039 = Bundle By Name(cluster=w1569, "Level(U)Array"=w1581) -> (w1582:T2)
        n1040 = property on="Stimulus Out" class="Clust (strict)"("Val(Sgnl)"=w1582) -> ()  [unwired: 2 in, 2 out]
      }
      event "Level(U)2": Value Change {
        n1041 = event-data() -> ("NewVal"=w1607:dbl)  [unwired: 6 out]
        n1042 = local read "MaxLevel_1"() -> (w1605:dbl)
        n1043 = local read "MaxLevel_2"() -> (w1604:dbl)
        n1044 = property on="unit2" class="Ring (strict)"() -> ("Value"=w1608:u16)  [unwired: 2 in, 2 out]
        n1045 = case shown="1" w1608 {
          tunnel: w1607 -> [w1613 w1622]
          tunnel: [w1611 w1620] -> w1606
          tunnel: w1605 -> [w1612 _]
          tunnel: w1604 -> [_ w1621]
          tunnel: [w1611 w1624] -> w1603
          frame 0, Default {
            n1046 = Less Than 0?(x=w1613) -> (x < 0?=w1614:bool)
            n1047 = case shown="False" w1614 {
              tunnel: [w1615 0.0 ("y")] -> w1611
              tunnel: w1613 -> [w1617 _]
              tunnel: w1612 -> [w1616 _]
              frame False {
                n1048 = Less?(x=w1617, y=w1616) -> (x < y?=w1618:bool)
                n1049 = Select(t=w1617, s=w1618, f=w1616) -> (s? t:f=w1615:dbl)
              }
              frame True {
              }
            }
          }
          frame 1 {
            n1050 = Less?(x=w1622, y=w1621) -> (x < y?=w1623:bool)
            n1051 = Select(t=w1622, s=w1623, f=w1621) -> (s? t:f=w1620:dbl)
            n1052 = call "CRYConversion dB-Lin.vi"("Log In"=w1620) -> ("Lin Out"=w1624:dbl)  [unwired: 5 in, 3 out]
          }
        }
        n1053 = Unbundle By Name(w1599) -> ("Level(U)Array"=w1602:dbl[])
        n1054 = Index Array(array=w1602, index=1) -> (element=w1600:dbl)
        n1055 = property on="LinLevel1" class="DigNum (strict)"("Value"=w1603) -> ()  [unwired: 2 in, 2 out]
        n1056 = property on="Level(U)2" class="DigNum (strict)"("Value"=w1606) -> ()  [unwired: 2 in, 2 out]
        n1057 = Build Array(w1606, w1600) -> (w1609:dbl[])
        n1058 = Bundle By Name(cluster=w1599, "Level(U)Array"=w1609) -> (w1610:T2)
        n1059 = property on="Stimulus Out" class="Clust (strict)"("Val(Sgnl)"=w1610) -> ()  [unwired: 2 in, 2 out]
      }
      event "Level4(U)": Value Change {
        n1060 = event-data() -> ("NewVal"=w1634:dbl)  [unwired: 6 out]
        n1061 = local read "MaxLevel_1"() -> (w1632:dbl)
        n1062 = local read "MaxLevel_2"() -> (w1631:dbl)
        n1063 = local read "Vmax (V)"() -> (w1629:dbl)
        n1064 = property on="unit4" class="Ring (strict)"() -> ("Value"=w1635:u16)  [unwired: 2 in, 2 out]
        n1065 = case shown="2" w1635 {
          tunnel: w1634 -> [w1640 w1649 w1656]
          tunnel: [w1638 w1647 w1653] -> w1633
          tunnel: w1632 -> [w1639 _ w1655]
          tunnel: w1631 -> [_ w1648 _]
          tunnel: [w1638 w1651 w1654] -> w1630
          tunnel: w1629 -> [_ _ _]
          frame 0, Default {
            n1066 = Less Than 0?(x=w1640) -> (x < 0?=w1641:bool)
            n1067 = case shown="False" w1641 {
              tunnel: [w1642 0.0 ("y")] -> w1638
              tunnel: w1640 -> [w1644 _]
              tunnel: w1639 -> [w1643 _]
              frame False {
                n1068 = Less?(x=w1644, y=w1643) -> (x < y?=w1645:bool)
                n1069 = Select(t=w1644, s=w1645, f=w1643) -> (s? t:f=w1642:dbl)
              }
              frame True {
              }
            }
          }
          frame 1 {
            n1070 = Less?(x=w1649, y=w1648) -> (x < y?=w1650:bool)
            n1071 = Select(t=w1649, s=w1650, f=w1648) -> (s? t:f=w1647:dbl)
            n1072 = call "CRYConversion dB-Lin.vi"("Log In"=w1647) -> ("Lin Out"=w1651:dbl)  [unwired: 5 in, 3 out]
          }
          frame 2 {
            n1073 = Less Than 0?(x=w1656) -> (x < 0?=w1657:bool)
            n1074 = case shown="False" w1657 {
              tunnel: [w1660 0.0 ("y")] -> w1653
              tunnel: w1656 -> [w1662 _]
              tunnel: w1655 -> [w1661 _]
              frame False {
                n1075 = Multiply(x=5.0, y=w1661) -> (x*y=w1659:dbl)
                n1076 = Less?(x=w1662, y=w1659) -> (x < y?=w1663:bool)
                n1077 = Select(t=w1662, s=w1663, f=w1659) -> (s? t:f=w1660:dbl)
              }
              frame True {
              }
            }
            n1078 = Divide(x=w1653, y=5.0) -> (x/y=w1654:dbl)
          }
        }
        n1079 = Unbundle By Name(w1625) -> ("Level(U)Array"=w1628:dbl[])
        n1080 = Index Array(array=w1628, index=1) -> (element=w1626:dbl)
        n1081 = Build Array(w1633, w1626) -> (w1636:dbl[])
        n1082 = property on="Level4(U)" class="DigNum (strict)"("Value"=w1633) -> ()  [unwired: 2 in, 2 out]
        n1083 = property on="LinLevel1" class="DigNum (strict)"("Value"=w1630) -> ()  [unwired: 2 in, 2 out]
        n1084 = Bundle By Name(cluster=w1625, "Level(U)Array"=w1636) -> (w1637:T2)
        n1085 = property on="Stimulus Out" class="Clust (strict)"("Val(Sgnl)"=w1637) -> ()  [unwired: 2 in, 2 out]
      }
      event "Level6_1(U)": Value Change {
        n1086 = event-data() -> ("NewVal"=w1673:dbl)  [unwired: 6 out]
        n1087 = local read "MaxLevel_1"() -> (w1671:dbl)
        n1088 = local read "MaxLevel_2"() -> (w1670:dbl)
        n1089 = property on="unit6" class="Ring (strict)"() -> ("Value"=w1674:u16)  [unwired: 2 in, 2 out]
        n1090 = case shown="1" w1674 {
          tunnel: w1673 -> [w1679 w1688]
          tunnel: [w1677 w1686] -> w1672
          tunnel: w1671 -> [w1678 _]
          tunnel: w1670 -> [_ w1687]
          tunnel: [w1677 w1690] -> w1669
          frame 0, Default {
            n1091 = Less Than 0?(x=w1679) -> (x < 0?=w1680:bool)
            n1092 = case shown="True" w1680 {
              tunnel: [w1681 0.0 ("y")] -> w1677
              tunnel: w1679 -> [w1683 _]
              tunnel: w1678 -> [w1682 _]
              frame False {
                n1093 = Less?(x=w1683, y=w1682) -> (x < y?=w1684:bool)
                n1094 = Select(t=w1683, s=w1684, f=w1682) -> (s? t:f=w1681:dbl)
              }
              frame True {
              }
            }
          }
          frame 1 {
            n1095 = Less?(x=w1688, y=w1687) -> (x < y?=w1689:bool)
            n1096 = Select(t=w1688, s=w1689, f=w1687) -> (s? t:f=w1686:dbl)
            n1097 = call "CRYConversion dB-Lin.vi"("Log In"=w1686) -> ("Lin Out"=w1690:dbl)  [unwired: 5 in, 3 out]
          }
        }
        n1098 = Unbundle By Name(w1665) -> ("Level(U)Array"=w1668:dbl[])
        n1099 = Index Array(array=w1668, index=1) -> (element=w1666:dbl)
        n1100 = property on="LinLevel1" class="DigNum (strict)"("Value"=w1669) -> ()  [unwired: 2 in, 2 out]
        n1101 = Build Array(w1672, w1666) -> (w1675:dbl[])
        n1102 = property on="Level6_1(U)" class="DigNum (strict)"("Value"=w1672) -> ()  [unwired: 2 in, 2 out]
        n1103 = Bundle By Name(cluster=w1665, "Level(U)Array"=w1675) -> (w1676:T2)
        n1104 = property on="Stimulus Out" class="Clust (strict)"("Val(Sgnl)"=w1676) -> ()  [unwired: 2 in, 2 out]
      }
      event "Level6_2(U)": Value Change {
        n1105 = event-data() -> ("NewVal"=w1699:dbl)  [unwired: 6 out]
        n1106 = local read "MaxLevel_1"() -> (w1697:dbl)
        n1107 = local read "MaxLevel_2"() -> (w1696:dbl)
        n1108 = property on="unit6_1" class="Ring (strict)"() -> ("Value"=w1700:u16)  [unwired: 2 in, 2 out]
        n1109 = case shown="1" w1700 {
          tunnel: w1699 -> [w1705 w1714]
          tunnel: [w1703 w1712] -> w1698
          tunnel: w1697 -> [w1704 _]
          tunnel: w1696 -> [_ w1713]
          tunnel: [w1703 w1716] -> w1695
          frame 0, Default {
            n1110 = Less Than 0?(x=w1705) -> (x < 0?=w1706:bool)
            n1111 = case shown="False" w1706 {
              tunnel: [w1707 0.0 ("y")] -> w1703
              tunnel: w1705 -> [w1709 _]
              tunnel: w1704 -> [w1708 _]
              frame False {
                n1112 = Less?(x=w1709, y=w1708) -> (x < y?=w1710:bool)
                n1113 = Select(t=w1709, s=w1710, f=w1708) -> (s? t:f=w1707:dbl)
              }
              frame True {
              }
            }
          }
          frame 1 {
            n1114 = Less?(x=w1714, y=w1713) -> (x < y?=w1715:bool)
            n1115 = Select(t=w1714, s=w1715, f=w1713) -> (s? t:f=w1712:dbl)
            n1116 = call "CRYConversion dB-Lin.vi"("Log In"=w1712) -> ("Lin Out"=w1716:dbl)  [unwired: 5 in, 3 out]
          }
        }
        n1117 = Unbundle By Name(w1691) -> ("Level(U)Array"=w1694:dbl[])
        n1118 = Index Array(array=w1694, index=0) -> (element=w1692:dbl)
        n1119 = property on="LinLevel2" class="DigNum (strict)"("Value"=w1695) -> ()  [unwired: 2 in, 2 out]
        n1120 = Build Array(w1692, w1698) -> (w1701:dbl[])
        n1121 = property on="Level6_2(U)" class="DigNum (strict)"("Value"=w1698) -> ()  [unwired: 2 in, 2 out]
        n1122 = Bundle By Name(cluster=w1691, "Level(U)Array"=w1701) -> (w1702:T2)
        n1123 = property on="Stimulus Out" class="Clust (strict)"("Val(Sgnl)"=w1702) -> ()  [unwired: 2 in, 2 out]
      }
      event "Level7(U)": Value Change {
        n1124 = event-data() -> ("NewVal"=w1731:dbl)  [unwired: 6 out]
        n1125 = local read "MaxLevel_1"() -> (w1719:dbl)
        n1126 = local read "MaxLevel_2"() -> (w1729:dbl)
        n1127 = local read "Vmax (V)"() -> (w1727:dbl)
        n1128 = Square Root(x=2.0 ("y")) -> (sqrt(x)=w1720:dbl)
        n1129 = Divide(x=w1719, y=w1720) -> (x/y=w1718:dbl)
        n1130 = property on="unit7" class="Ring (strict)"() -> ("Value"=w1732:u16)  [unwired: 2 in, 2 out]
        n1131 = Multiply(x=w1718, y=2.0) -> (x*y=w1717:dbl)
        n1132 = case shown="1" w1732 {
          tunnel: w1731 -> [w1737 w1748 w1755]
          tunnel: [w1735 w1746 w1753] -> w1730
          tunnel: w1717 -> [w1736 _ w1754]
          tunnel: w1729 -> [_ w1747 _]
          tunnel: [w1735 w1750 w1752] -> w1728
          tunnel: w1727 -> [_ _ _]
          frame 0, Default {
            n1133 = Less Than 0?(x=w1737) -> (x < 0?=w1738:bool)
            n1134 = case shown="False" w1738 {
              tunnel: [w1742 0.0 ("y")] -> w1735
              tunnel: w1737 -> [w1743 _]
              tunnel: w1736 -> [w1740 _]
              frame False {
                n1135 = Divide(x=w1740, y=5.0) -> (x/y=w1739:dbl)
                n1136 = Less?(x=w1743, y=w1739) -> (x < y?=w1744:bool)
                n1137 = Select(t=w1743, s=w1744, f=w1739) -> (s? t:f=w1742:dbl)
              }
              frame True {
              }
            }
          }
          frame 1 {
            n1138 = Less?(x=w1748, y=w1747) -> (x < y?=w1749:bool)
            n1139 = Select(t=w1748, s=w1749, f=w1747) -> (s? t:f=w1746:dbl)
            n1140 = call "CRYConversion dB-Lin.vi"("Log In"=w1746) -> ("Lin Out"=w1750:dbl)  [unwired: 5 in, 3 out]
          }
          frame 2 {
            n1141 = Less Than 0?(x=w1755) -> (x < 0?=w1756:bool)
            n1142 = case shown="False" w1756 {
              tunnel: [w1758 0.0 ("y")] -> w1753
              tunnel: w1755 -> [w1759 _]
              tunnel: w1754 -> [w1757 _]
              frame False {
                n1143 = Less?(x=w1759, y=w1757) -> (x < y?=w1760:bool)
                n1144 = Select(t=w1759, s=w1760, f=w1757) -> (s? t:f=w1758:dbl)
              }
              frame True {
              }
            }
            n1145 = Divide(x=w1753, y=5.0) -> (x/y=w1752:dbl)
          }
        }
        n1146 = Unbundle By Name(w1723) -> ("Level(U)Array"=w1726:dbl[])
        n1147 = Index Array(array=w1726, index=1) -> (element=w1724:dbl)
        n1148 = property on="LinLevel1" class="DigNum (strict)"("Value"=w1728) -> ()  [unwired: 2 in, 2 out]
        n1149 = property on="Level7(U)" class="DigNum (strict)"("Value"=w1730) -> ()  [unwired: 2 in, 2 out]
        n1150 = Build Array(w1730, w1724) -> (w1733:dbl[])
        n1151 = Bundle By Name(cluster=w1723, "Level(U)Array"=w1733) -> (w1734:T2)
        n1152 = property on="Stimulus Out" class="Clust (strict)"("Val(Sgnl)"=w1734) -> ()  [unwired: 2 in, 2 out]
      }
      event "Level8(U)": Value Change {
        n1153 = event-data() -> ("NewVal"=w1776:dbl)  [unwired: 6 out]
        n1154 = Square Root(x=2.0 ("y")) -> (sqrt(x)=w1765:dbl)
        n1155 = local read "MaxLevel_1"() -> (w1763:dbl)
        n1156 = local read "MaxLevel_2"() -> (w1774:dbl)
        n1157 = local read "Vmax (V)"() -> (w1772:dbl)
        n1158 = Divide(x=w1763, y=w1765) -> (x/y=w1764:dbl)
        n1159 = Multiply(x=w1764, y=2.0) -> (x*y=w1762:dbl)
        n1160 = property on="unit8" class="Ring (strict)"() -> ("Value"=w1777:u16)  [unwired: 2 in, 2 out]
        n1161 = case shown="0, Default" w1777 {
          tunnel: w1776 -> [w1782 w1794 w1800]
          tunnel: [w1780 w1791 w1798] -> w1775
          tunnel: w1762 -> [w1781 _ w1799]
          tunnel: w1774 -> [_ w1792 _]
          tunnel: [w1780 w1795 w1797] -> w1773
          tunnel: w1772 -> [_ _ _]
          frame 0, Default {
            n1162 = Less Than 0?(x=w1782) -> (x < 0?=w1783:bool)
            n1163 = case shown="False" w1783 {
              tunnel: [w1787 0.0 ("y")] -> w1780
              tunnel: w1782 -> [w1788 _]
              tunnel: w1781 -> [w1785 _]
              frame False {
                n1164 = Divide(x=w1785, y=5.0) -> (x/y=w1784:dbl)
                n1165 = Less?(x=w1788, y=w1784) -> (x < y?=w1789:bool)
                n1166 = Select(t=w1788, s=w1789, f=w1784) -> (s? t:f=w1787:dbl)
              }
              frame True {
              }
            }
          }
          frame 1 {
            n1167 = Less?(x=w1794, y=w1792) -> (x < y?=w1793:bool)
            n1168 = Select(t=w1794, s=w1793, f=w1792) -> (s? t:f=w1791:dbl)
            n1169 = call "CRYConversion dB-Lin.vi"("Log In"=w1791) -> ("Lin Out"=w1795:dbl)  [unwired: 5 in, 3 out]
          }
          frame 2 {
            n1170 = Less Than 0?(x=w1800) -> (x < 0?=w1801:bool)
            n1171 = case shown="False" w1801 {
              tunnel: [w1803 0.0 ("y")] -> w1798
              tunnel: w1800 -> [w1804 _]
              tunnel: w1799 -> [w1802 _]
              frame False {
                n1172 = Less?(x=w1804, y=w1802) -> (x < y?=w1805:bool)
                n1173 = Select(t=w1804, s=w1805, f=w1802) -> (s? t:f=w1803:dbl)
              }
              frame True {
              }
            }
            n1174 = Divide(x=w1798, y=5.0) -> (x/y=w1797:dbl)
          }
        }
        n1175 = Unbundle By Name(w1768) -> ("Level(U)Array"=w1771:dbl[])
        n1176 = Index Array(array=w1771, index=1) -> (element=w1769:dbl)
        n1177 = property on="Level8(U)" class="DigNum (strict)"("Value"=w1775) -> ()  [unwired: 2 in, 2 out]
        n1178 = property on="LinLevel1" class="DigNum (strict)"("Value"=w1773) -> ()  [unwired: 2 in, 2 out]
        n1179 = Build Array(w1775, w1769) -> (w1778:dbl[])
        n1180 = Bundle By Name(cluster=w1768, "Level(U)Array"=w1778) -> (w1779:T2)
        n1181 = property on="Stimulus Out" class="Clust (strict)"("Val(Sgnl)"=w1779) -> ()  [unwired: 2 in, 2 out]
      }
      event "unit1": Value Change {
        n1182 = event-data() -> ("NewVal"=w1809:u16)  [unwired: 6 out]
        n1183 = property on="Level(U)1" class="DigNum (strict)"() -> ("Value"=w1816:dbl)  [unwired: 2 in, 2 out]
        n1184 = case shown="0, Default" w1809 {
          tunnel: w1813 -> [w1820 w1825]
          tunnel: w1812 -> [w1821 w1824]
          tunnel: w1816 -> [w1819 w1822]
          tunnel: [w1818 w1823] -> w1815
          frame 0, Default {
            n1185 = call "CRYConversion dB-Lin.vi"("unit prefix"=w1821, "dB ref."=w1820, "Log In"=w1819) -> ("Lin Out"=w1818:dbl)  [unwired: 3 in, 3 out]
            n1186 = property on="LinLevel1" class="DigNum (strict)"("Value"=w1818) -> ()  [unwired: 2 in, 2 out]
          }
          frame 1 {
            n1187 = property on="LinLevel1" class="DigNum (strict)"("Value"=w1822) -> ()  [unwired: 2 in, 2 out]
            n1188 = call "CRYConversion dB-Lin.vi"("unit prefix"=w1824, "dB ref."=w1825, "Lin In"=w1822) -> ("Log Out"=w1823:dbl)  [unwired: 3 in, 3 out]
          }
        }
        n1189 = Unbundle By Name(w1811) -> ("Unit_Array"=w1810:u16[])
        n1190 = property on="Level(U)1" class="DigNum (strict)"("Value"=w1815) -> ()  [unwired: 2 in, 2 out]
        n1191 = Build Array(w1815) -> (w1814:dbl[])
        n1192 = Replace Array Subset(array=w1810, new element=w1809, index=0) -> (w1808:u16[])
        n1193 = Bundle By Name(cluster=w1811, "Unit_Array"=w1808, "DegValArray"=w1814) -> (w1817:T2)
        n1194 = property on="Stimulus Out" class="Clust (strict)"("Val(Sgnl)"=w1817) -> ()  [unwired: 2 in, 2 out]
      }
      event "unit2": Value Change {
        n1195 = event-data() -> ("NewVal"=w1826:u16)  [unwired: 6 out]
        n1196 = property on="Level(U)2" class="DigNum (strict)"() -> ("Value"=w1835:dbl)  [unwired: 2 in, 2 out]
        n1197 = case shown="1" w1826 {
          tunnel: w1832 -> [w1839 w1844]
          tunnel: w1831 -> [w1840 w1843]
          tunnel: w1835 -> [w1838 w1841]
          tunnel: [w1837 w1842] -> w1834
          frame 0, Default {
            n1198 = call "CRYConversion dB-Lin.vi"("unit prefix"=w1840, "dB ref."=w1839, "Log In"=w1838) -> ("Lin Out"=w1837:dbl)  [unwired: 3 in, 3 out]
            n1199 = property on="LinLevel1" class="DigNum (strict)"("Value"=w1837) -> ()  [unwired: 2 in, 2 out]
          }
          frame 1 {
            n1200 = property on="LinLevel1" class="DigNum (strict)"("Value"=w1841) -> ()  [unwired: 2 in, 2 out]
            n1201 = call "CRYConversion dB-Lin.vi"("unit prefix"=w1843, "dB ref."=w1844, "Lin In"=w1841) -> ("Log Out"=w1842:dbl)  [unwired: 3 in, 3 out]
          }
        }
        n1202 = Unbundle By Name(w1828) -> ("Unit_Array"=w1830:u16[])
        n1203 = Replace Array Subset(array=w1830, new element=w1826, index=1) -> (w1827:u16[])
        n1204 = Build Array(w1834) -> (w1833:dbl[])
        n1205 = property on="Level(U)2" class="DigNum (strict)"("Value"=w1834) -> ()  [unwired: 2 in, 2 out]
        n1206 = Bundle By Name(cluster=w1828, "Unit_Array"=w1827, "Level(U)Array"=w1833) -> (w1836:T2)
        n1207 = property on="Stimulus Out" class="Clust (strict)"("Val(Sgnl)"=w1836) -> ()  [unwired: 2 in, 2 out]
      }
      event "unit3": Value Change {
        n1208 = event-data() -> ("NewVal"=w1846:u16)  [unwired: 6 out]
        n1209 = property on="Stop Amp3" class="DigNum (strict)"() -> ("Value"=w1855:dbl)  [unwired: 2 in, 2 out]
        n1210 = property on="Start Amp3" class="DigNum (strict)"() -> ("Value"=w1856:dbl)  [unwired: 2 in, 2 out]
        n1211 = case shown="0, Default" w1846 {
          tunnel: w1851 -> [w1860 w1865]
          tunnel: w1850 -> [w1861 w1864]
          tunnel: [w1859 w1862] -> w1853
          tunnel: w1855 -> [w1858 w1863]
          frame 0, Default {
            n1212 = call "CRYConversion dB-Lin.vi"("unit prefix"=w1861, "dB ref."=w1860, "Log In"=w1858) -> ("Lin Out"=w1859:dbl)  [unwired: 3 in, 3 out]
          }
          frame 1 {
            n1213 = call "CRYConversion dB-Lin.vi"("unit prefix"=w1864, "dB ref."=w1865, "Lin In"=w1863) -> ("Log Out"=w1862:dbl)  [unwired: 3 in, 3 out]
          }
        }
        n1214 = case shown="0, Default" w1846 {
          tunnel: w1851 -> [w1868 w1873]
          tunnel: w1850 -> [w1869 w1872]
          tunnel: [w1867 w1870] -> w1854
          tunnel: w1856 -> [w1866 w1871]
          frame 0, Default {
            n1215 = call "CRYConversion dB-Lin.vi"("unit prefix"=w1869, "dB ref."=w1868, "Log In"=w1866) -> ("Lin Out"=w1867:dbl)  [unwired: 3 in, 3 out]
          }
          frame 1 {
            n1216 = call "CRYConversion dB-Lin.vi"("unit prefix"=w1872, "dB ref."=w1873, "Lin In"=w1871) -> ("Log Out"=w1870:dbl)  [unwired: 3 in, 3 out]
          }
        }
        n1217 = Unbundle By Name(w1847) -> ("Unit_Array"=w1849:u16[])
        n1218 = property on="Stop Amp3" class="DigNum (strict)"("Value"=w1853) -> ()  [unwired: 2 in, 2 out]
        n1219 = property on="Start Amp3" class="DigNum (strict)"("Value"=w1854) -> ()  [unwired: 2 in, 2 out]
        n1220 = Replace Array Subset(array=w1849, new element=w1846, index=2) -> (w1845:u16[])
        n1221 = Build Array(w1854, w1853) -> (w1852:dbl[])
        n1222 = Bundle By Name(cluster=w1847, "Unit_Array"=w1845, "Start(Stop)AmpArray"=w1852) -> (w1857:T2)
        n1223 = property on="Stimulus Out" class="Clust (strict)"("Val(Sgnl)"=w1857) -> ()  [unwired: 2 in, 2 out]
      }
      event "unit4": Value Change {
        n1224 = event-data() -> ("NewVal"=w1876:u16)  [unwired: 6 out]
        n1225 = property on="LinLevel1" class="DigNum (strict)"() -> ("Value"=w1874:dbl)  [unwired: 2 in, 2 out]
        n1226 = case shown="2" w1876 {
          tunnel: w1881 -> [_ w1889 _]
          tunnel: w1880 -> [_ w1888 _]
          tunnel: w1874 -> [w1885 w1886 w1891]
          tunnel: [w1885 w1887 w1892] -> w1883
          frame 0, Default {
          }
          frame 1 {
            n1227 = call "CRYConversion dB-Lin.vi"("unit prefix"=w1888, "dB ref."=w1889, "Lin In"=w1886) -> ("Log Out"=w1887:dbl)  [unwired: 3 in, 3 out]
          }
          frame 2 {
            n1228 = Multiply(x=w1891, y=5.0) -> (x*y=w1892:dbl)
          }
        }
        n1229 = Unbundle By Name(w1877) -> ("Unit_Array"=w1879:u16[])
        n1230 = property on="Level4(U)" class="DigNum (strict)"("Value"=w1883) -> ()  [unwired: 2 in, 2 out]
        n1231 = Build Array(w1883) -> (w1882:dbl[])
        n1232 = Replace Array Subset(array=w1879, new element=w1876, index=3) -> (w1875:u16[])
        n1233 = Bundle By Name(cluster=w1877, "Unit_Array"=w1875, "Level(U)Array"=w1882) -> (w1884:T2)
        n1234 = property on="Stimulus Out" class="Clust (strict)"("Val(Sgnl)"=w1884) -> ()  [unwired: 2 in, 2 out]
      }
      event "unit6": Value Change {
        n1235 = event-data() -> ("NewVal"=w1894:u16)  [unwired: 6 out]
        n1236 = property on="Level6_1(U)" class="DigNum (strict)"() -> ("Value"=w1902:dbl)  [unwired: 2 in, 2 out]
        n1237 = case shown="1" w1894 {
          tunnel: w1899 -> [w1906 w1911]
          tunnel: w1898 -> [w1907 w1910]
          tunnel: w1902 -> [w1905 w1908]
          tunnel: [w1904 w1909] -> w1901
          frame 0, Default {
            n1238 = call "CRYConversion dB-Lin.vi"("unit prefix"=w1907, "dB ref."=w1906, "Log In"=w1905) -> ("Lin Out"=w1904:dbl)  [unwired: 3 in, 3 out]
            n1239 = property on="LinLevel1" class="DigNum (strict)"("Value"=w1904) -> ()  [unwired: 2 in, 2 out]
          }
          frame 1 {
            n1240 = property on="LinLevel1" class="DigNum (strict)"("Value"=w1908) -> ()  [unwired: 2 in, 2 out]
            n1241 = call "CRYConversion dB-Lin.vi"("unit prefix"=w1910, "dB ref."=w1911, "Lin In"=w1908) -> ("Log Out"=w1909:dbl)  [unwired: 3 in, 3 out]
          }
        }
        n1242 = Unbundle By Name(w1895) -> ("Unit_Array"=w1897:u16[])
        n1243 = property on="Level6_1(U)" class="DigNum (strict)"("Value"=w1901) -> ()  [unwired: 2 in, 2 out]
        n1244 = Build Array(w1901) -> (w1900:dbl[])
        n1245 = Replace Array Subset(array=w1897, new element=w1894, index=4) -> (w1893:u16[])
        n1246 = Bundle By Name(cluster=w1895, "Unit_Array"=w1893, "Level(U)Array"=w1900) -> (w1903:T2)
        n1247 = property on="Stimulus Out" class="Clust (strict)"("Val(Sgnl)"=w1903) -> ()  [unwired: 2 in, 2 out]
      }
      event "unit6_1": Value Change {
        n1248 = event-data() -> ("NewVal"=w1912:u16)  [unwired: 6 out]
        n1249 = property on="Level6_2(U)" class="DigNum (strict)"() -> ("Value"=w1921:dbl)  [unwired: 2 in, 2 out]
        n1250 = case shown="1" w1912 {
          tunnel: w1918 -> [w1925 w1930]
          tunnel: w1917 -> [w1926 w1929]
          tunnel: w1921 -> [w1924 w1927]
          tunnel: [w1923 w1928] -> w1920
          frame 0, Default {
            n1251 = call "CRYConversion dB-Lin.vi"("unit prefix"=w1926, "dB ref."=w1925, "Log In"=w1924) -> ("Lin Out"=w1923:dbl)  [unwired: 3 in, 3 out]
            n1252 = property on="LinLevel2" class="DigNum (strict)"("Value"=w1923) -> ()  [unwired: 2 in, 2 out]
          }
          frame 1 {
            n1253 = property on="LinLevel2" class="DigNum (strict)"("Value"=w1927) -> ()  [unwired: 2 in, 2 out]
            n1254 = call "CRYConversion dB-Lin.vi"("unit prefix"=w1929, "dB ref."=w1930, "Lin In"=w1927) -> ("Log Out"=w1928:dbl)  [unwired: 3 in, 3 out]
          }
        }
        n1255 = Unbundle By Name(w1914) -> ("Unit_Array"=w1916:u16[])
        n1256 = Replace Array Subset(array=w1916, new element=w1912, index=5) -> (w1913:u16[])
        n1257 = Build Array(w1920) -> (w1919:dbl[])
        n1258 = property on="Level6_2(U)" class="DigNum (strict)"("Value"=w1920) -> ()  [unwired: 2 in, 2 out]
        n1259 = Bundle By Name(cluster=w1914, "Unit_Array"=w1913, "Level(U)Array"=w1919) -> (w1922:T2)
        n1260 = property on="Stimulus Out" class="Clust (strict)"("Val(Sgnl)"=w1922) -> ()  [unwired: 2 in, 2 out]
      }
      event "unit7": Value Change {
        n1261 = event-data() -> ("NewVal"=w1933:u16)  [unwired: 6 out]
        n1262 = property on="LinLevel1" class="DigNum (strict)"() -> ("Value"=w1931:dbl)  [unwired: 2 in, 2 out]
        n1263 = case shown="2" w1933 {
          tunnel: w1932 -> [_ w1946 _]
          tunnel: w1938 -> [_ w1945 _]
          tunnel: w1931 -> [w1942 w1943 w1949]
          tunnel: [w1942 w1944 w1948] -> w1940
          frame 0, Default {
          }
          frame 1 {
            n1264 = call "CRYConversion dB-Lin.vi"("unit prefix"=w1945, "dB ref."=w1946, "Lin In"=w1943) -> ("Log Out"=w1944:dbl)  [unwired: 3 in, 3 out]
          }
          frame 2 {
            n1265 = Multiply(x=w1949, y=5.0) -> (x*y=w1948:dbl)
          }
        }
        n1266 = Unbundle By Name(w1935) -> ("Unit_Array"=w1937:u16[])
        n1267 = Replace Array Subset(array=w1937, new element=w1933, index=6) -> (w1934:u16[])
        n1268 = property on="Level7(U)" class="DigNum (strict)"("Value"=w1940) -> ()  [unwired: 2 in, 2 out]
        n1269 = Build Array(w1940) -> (w1939:dbl[])
        n1270 = Bundle By Name(cluster=w1935, "Unit_Array"=w1934, "Level(U)Array"=w1939) -> (w1941:T2)
        n1271 = property on="Stimulus Out" class="Clust (strict)"("Val(Sgnl)"=w1941) -> ()  [unwired: 2 in, 2 out]
      }
      event "unit8": Value Change {
        n1272 = event-data() -> ("NewVal"=w1951:u16)  [unwired: 6 out]
        n1273 = property on="LinLevel1" class="DigNum (strict)"() -> ("Value"=w1950:dbl)  [unwired: 2 in, 2 out]
        n1274 = case shown="2" w1951 {
          tunnel: w1957 -> [_ w1965 _]
          tunnel: w1956 -> [_ w1964 _]
          tunnel: w1950 -> [w1961 w1962 w1968]
          tunnel: [w1961 w1963 w1967] -> w1958
          frame 0, Default {
          }
          frame 1 {
            n1275 = call "CRYConversion dB-Lin.vi"("unit prefix"=w1964, "dB ref."=w1965, "Lin In"=w1962) -> ("Log Out"=w1963:dbl)  [unwired: 3 in, 3 out]
          }
          frame 2 {
            n1276 = Multiply(x=w1968, y=5.0) -> (x*y=w1967:dbl)
          }
        }
        n1277 = Unbundle By Name(w1952) -> ("Unit_Array"=w1955:u16[])
        n1278 = property on="Level8(U)" class="DigNum (strict)"("Value"=w1958) -> ()  [unwired: 2 in, 2 out]
        n1279 = Replace Array Subset(array=w1955, new element=w1951, index=7) -> (w1953:u16[])
        n1280 = Build Array(w1958) -> (w1959:dbl[])
        n1281 = Bundle By Name(cluster=w1952, "Unit_Array"=w1953, "Level(U)Array"=w1959) -> (w1960:T2)
        n1282 = property on="Stimulus Out" class="Clust (strict)"("Val(Sgnl)"=w1960) -> ()  [unwired: 2 in, 2 out]
      }
      event "Start Amp3": Value Change {
        n1283 = event-data() -> ("NewVal"=w1971:dbl)  [unwired: 6 out]
        n1284 = flat-sequence {
          tunnel: w1971 -> [w1979]
          tunnel: w1970 -> [w1974]
          tunnel: w1969 -> [w1972]
          frame #0 {
            n1285 = local read "MaxLevel_1"() -> (w1975:dbl)
            n1286 = local read "MaxLevel_2"() -> (w1976:dbl)
            n1287 = Unbundle By Name(w1974) -> ("Start(Stop)AmpArray"=w1982:dbl[])
            n1288 = property on="unit3" class="Ring (strict)"() -> ("Value"=w1978:u16)  [unwired: 2 in, 2 out]
            n1289 = Index Array(array=w1982, index=1) -> (element=w1980:dbl)
            n1290 = case shown="1" w1978 {
              tunnel: w1979 -> [w1987 w1997]
              tunnel: [w1985 w1996] -> w1977
              tunnel: w1976 -> [_ w1998]
              tunnel: w1975 -> [w1986 _]
              tunnel: [w1985 w1995] -> w1973
              tunnel: w1972 -> [_ w1994]
              frame 0, Default {
                n1291 = Less Than 0?(x=w1987) -> (x < 0?=w1988:bool)
                n1292 = case shown="True" w1988 {
                  tunnel: [w1989 0.0 ("y")] -> w1985
                  tunnel: w1987 -> [w1991 _]
                  tunnel: w1986 -> [w1990 _]
                  frame False {
                    n1293 = Greater?(x=w1991, y=w1990) -> (0:w1992:bool)
                    n1294 = Select(t=w1990, s=w1992, f=w1991) -> (s? t:f=w1989:dbl)
                  }
                  frame True {
                  }
                }
              }
              frame 1 {
                n1295 = Greater?(x=w1997, y=w1998) -> (0:w1999:bool)
                n1296 = Select(t=w1998, s=w1999, f=w1997) -> (s? t:f=w1996:dbl)
                n1297 = call "CRYConversion dB-Lin.vi"("dB ref."=w1994, "Log In"=w1996) -> ("Lin Out"=w1995:dbl)  [unwired: 4 in, 3 out]
              }
            }
            n1298 = Build Array(w1977, w1980) -> (w1983:dbl[])
            n1299 = Bundle By Name(cluster=w1974, "Start(Stop)AmpArray"=w1983) -> (w1984:T2)
            n1300 = property on="Stimulus Out" class="Clust (strict)"("Val(Sgnl)"=w1984) -> ()  [unwired: 2 in, 2 out]
            n1301 = property on="Start Amp3" class="DigNum (strict)"("Value"=w1977) -> ()  [unwired: 2 in, 2 out]
            n1302 = property on="LinLevel1" class="DigNum (strict)"("Value"=w1973) -> ()  [unwired: 2 in, 2 out]
          }
          frame #1 {
            n1303 = property on="Update" class="Bool (strict)"("Val(Sgnl)"=TRUE ("Value (Signaling)")) -> ()  [unwired: 2 in, 2 out]
          }
        }
      }
      event "Stop Amp3": Value Change {
        n1304 = event-data() -> ("NewVal"=w2003:dbl)  [unwired: 6 out]
        n1305 = flat-sequence {
          tunnel: w2003 -> [w2010]
          tunnel: w2002 -> [w2006]
          tunnel: w2001 -> [w2004]
          frame #0 {
            n1306 = local read "MaxLevel_1"() -> (w2008:dbl)
            n1307 = local read "MaxLevel_2"() -> (w2007:dbl)
            n1308 = Unbundle By Name(w2006) -> ("Start(Stop)AmpArray"=w2014:dbl[])
            n1309 = property on="unit3" class="Ring (strict)"() -> ("Value"=w2011:u16)  [unwired: 2 in, 2 out]
            n1310 = Index Array(array=w2014, index=0) -> (element=w2012:dbl)
            n1311 = case shown="0, Default" w2011 {
              tunnel: w2010 -> [w2019 w2029]
              tunnel: [w2017 w2028] -> w2009
              tunnel: w2008 -> [w2018 _]
              tunnel: w2007 -> [_ w2030]
              tunnel: [w2017 w2027] -> w2005
              tunnel: w2004 -> [_ w2026]
              frame 0, Default {
                n1312 = Less Than 0?(x=w2019) -> (x < 0?=w2020:bool)
                n1313 = case shown="False" w2020 {
                  tunnel: [w2022 0.0 ("y")] -> w2017
                  tunnel: w2019 -> [w2024 _]
                  tunnel: w2018 -> [w2023 _]
                  frame False {
                    n1314 = Less?(x=w2024, y=w2023) -> (x < y?=w2021:bool)
                    n1315 = Select(t=w2024, s=w2021, f=w2023) -> (s? t:f=w2022:dbl)
                  }
                  frame True {
                  }
                }
              }
              frame 1 {
                n1316 = Less?(x=w2029, y=w2030) -> (x < y?=w2031:bool)
                n1317 = Select(t=w2029, s=w2031, f=w2030) -> (s? t:f=w2028:dbl)
                n1318 = call "CRYConversion dB-Lin.vi"("dB ref."=w2026, "Log In"=w2028) -> ("Lin Out"=w2027:dbl)  [unwired: 4 in, 3 out]
              }
            }
            n1319 = Build Array(w2012, w2009) -> (w2015:dbl[])
            n1320 = Bundle By Name(cluster=w2006, "Start(Stop)AmpArray"=w2015) -> (w2016:T2)
            n1321 = property on="Stimulus Out" class="Clust (strict)"("Val(Sgnl)"=w2016) -> ()  [unwired: 2 in, 2 out]
            n1322 = property on="LinLevel2" class="DigNum (strict)"("Value"=w2005) -> ()  [unwired: 2 in, 2 out]
            n1323 = property on="Stop Amp3" class="DigNum (strict)"("Value"=w2009) -> ()  [unwired: 2 in, 2 out]
          }
          frame #1 {
            n1324 = property on="Update" class="Bool (strict)"("Val(Sgnl)"=TRUE ("Value (Signaling)")) -> ()  [unwired: 2 in, 2 out]
          }
        }
      }
      event "StopAmp5": Value Change {
        n1325 = event-data() -> ("NewVal"=w2036:dbl)  [unwired: 6 out]
        n1326 = property on="dc_ctrl5_2" class="Slide (strict)"() -> ("Value"=w2037:u16)  [unwired: 2 in, 2 out]
        n1327 = case shown="1" w2037 {
          tunnel: w2036 -> [w2050 w2058]
          tunnel: [w2049 w2057] -> w2035
          frame 0, Default {
            n1328 = Less Than 0?(x=w2050) -> (x < 0?=w2051:bool)
            n1329 = case shown="False" w2051 {
              tunnel: [w2052 0.0 ("x")] -> w2049
              tunnel: w2050 -> [w2054 _]
              frame False {
                w2053 = 10.0 ("y")
                n1330 = Less?(x=w2054, y=w2053) -> (x < y?=w2055:bool)
                n1331 = Select(t=w2054, s=w2055, f=w2053) -> (s? t:f=w2052:dbl)
              }
              frame True {
              }
            }
          }
          frame 1 {
            n1332 = Less Than 0?(x=w2058) -> (x < 0?=w2059:bool)
            n1333 = case shown="False" w2059 {
              tunnel: [w2060 0.0 ("x")] -> w2057
              tunnel: w2058 -> [w2061 _]
              frame False {
                w2062 = 0.003 ("y")
                n1334 = Less?(x=w2061, y=w2062) -> (x < y?=w2063:bool)
                n1335 = Select(t=w2061, s=w2063, f=w2062) -> (s? t:f=w2060:dbl)
              }
              frame True {
              }
            }
          }
        }
        n1336 = property on="Steps5" class="DigNum (strict)"() -> ("Value"=w2039:i32)  [unwired: 2 in, 2 out]
        n1337 = property on="StartAmp5" class="DigNum (strict)"() -> ("Value"=w2038:dbl)  [unwired: 2 in, 2 out]
        n1338 = property on="StopAmp5" class="DigNum (strict)"("Value"=w2035) -> ()  [unwired: 2 in, 2 out]
        n1339 = Unbundle By Name(w2033) -> ("Start(Stop)AmpArray"=w2046:dbl[])
        n1340 = Subtract(x=w2038, y=w2035) -> (x-y=w2043:dbl)
        n1341 = Decrement(x=w2039) -> (x-1=w2042:i32)
        n1342 = Absolute Value(x=w2043) -> (abs(x)=w2040:dbl)
        n1343 = Less Or Equal To 0?(x=w2042) -> (x <= 0?=w2041:bool)
        n1344 = Index Array(array=w2046, index=0) -> (element=w2044:dbl)
        n1345 = case shown="False" w2041 {
          tunnel: w2042 -> [w2066 _]
          tunnel: w2040 -> [w2067 _]
          tunnel: [w2065 0.0] -> w2034
          frame False {
            n1346 = Divide(x=w2067, y=w2066) -> (x/y=w2065:dbl)
          }
          frame True {
          }
        }
        n1347 = Build Array(w2044, w2035) -> (w2047:dbl[])
        n1348 = Bundle By Name(cluster=w2033, "Start(Stop)AmpArray"=w2047, "StepsSize5Val"=w2034) -> (w2048:T2)
        n1349 = property on="Steps Size5" class="DigNum (strict)"("Value"=w2034) -> ()  [unwired: 2 in, 2 out]
        n1350 = property on="Stimulus Out" class="Clust (strict)"("Val(Sgnl)"=w2048) -> ()  [unwired: 2 in, 2 out]
      }
      event "Step Resolution1": Value Change {
        n1351 = event-data() -> ("NewVal"=w2071:u16)  [unwired: 6 out]
        n1352 = Less?(x=w2071, y=u16 4) -> (x < y?=w2080:bool)
        n1353 = Unbundle By Name(w2069) -> ("StepResolutionArray"=w2073:u16[])
        n1354 = property on="StartFreq1(Hz)" class="DigNum (strict)"() -> ("Value"=w2084:dbl)  [unwired: 2 in, 2 out]
        n1355 = property on="StopFreq1(Hz)" class="DigNum (strict)"() -> ("Value"=w2083:dbl)  [unwired: 2 in, 2 out]
        n1356 = Select(t=u8 2 ("Disabled"), s=w2080, f=u8 0 ("Disabled")) -> (s? t:f=w2077:u8)
        n1357 = property on="Steps1" class="DigNum (strict)"() -> ("Value"=w2076:i32)  [unwired: 2 in, 2 out]
        n1358 = property on="Steps1" class="DigNum (strict)"("Disabled"=w2077) -> ()  [unwired: 2 in, 2 out]
        n1359 = Replace Array Subset(array=w2073, new element=w2071, index=0) -> (w2070:u16[])
        n1360 = property on="Max Freq" class="DigNum (strict)"() -> ("Value"=w2074:dbl)  [unwired: 2 in, 2 out]
        n1361 = call "CRYGet Steps From F1 F2 Resolution.vi"("Steps/Tone"=w2076, "Stop Freq"=w2083, "Start Freq"=w2084, "Resolution"=w2071) -> ("Steps"=w2081:i32)  [unwired: 7 out]
        n1362 = Bundle By Name(cluster=w2069, "StepResolutionArray"=w2070, "Steps1"=w2081) -> (w2085:T2)
        n1363 = case shown="0..3" w2071 {
          selector: w2071 -> [_ w2090]
          tunnel: [w2089 w2092] -> w2075
          tunnel: w2074 -> [w2089 w2091]
          frame Default {
          }
          frame 0..3 {
            n1364 = call "CRYStimulus Freq Max Limit.vi"("Resolution"=w2090, "Max Freq"=w2091, "Input Val"=w2091) -> ("Output Val"=w2092:dbl)  [unwired: 1 in, 7 out]
          }
        }
        n1365 = property on="Steps1" class="DigNum (strict)"("Value"=w2081) -> ()  [unwired: 2 in, 2 out]
        n1366 = property on="Stimulus Out" class="Clust (strict)"("Val(Sgnl)"=w2085) -> ()  [unwired: 2 in, 2 out]
        n1367 = flat-sequence {
          tunnel: w2075 -> [w2086]
          frame #0 {
            n1368 = property on="Res Max Freq" class="DigNum (strict)"("Value"=w2086) -> ()  [unwired: 2 in, 2 out]
          }
          frame #1 {
            n1369 = property on="StopFreq1(Hz)" class="DigNum (strict)"() -> ("Value"=w2087:dbl)  [unwired: 2 in, 2 out]
            n1370 = property on="StartFreq1(Hz)" class="DigNum (strict)"() -> ("Value"=w2088:dbl)  [unwired: 2 in, 2 out]
            n1371 = property on="StartFreq1(Hz)" class="DigNum (strict)"("Val(Sgnl)"=w2088) -> ()  [unwired: 2 in, 2 out]
            n1372 = property on="StopFreq1(Hz)" class="DigNum (strict)"("Val(Sgnl)"=w2087) -> ()  [unwired: 2 in, 2 out]
          }
        }
      }
      event "StepResolution6": Value Change {
        n1373 = event-data() -> ("NewVal"=w2093:u16)  [unwired: 6 out]
        n1374 = Unbundle By Name(w2094) -> ("StepResolutionArray"=w2097:u16[])
        n1375 = Less?(x=w2093, y=u16 4) -> (x < y?=w2104:bool)
        n1376 = property on="StartFreq6(Hz)" class="DigNum (strict)"() -> ("Value"=w2108:dbl)  [unwired: 2 in, 2 out]
        n1377 = property on="StopFreq6(Hz)" class="DigNum (strict)"() -> ("Value"=w2107:dbl)  [unwired: 2 in, 2 out]
        n1378 = Select(t=u8 2 ("Disabled"), s=w2104, f=u8 0 ("Disabled")) -> (s? t:f=w2101:u8)
        n1379 = property on="Steps6" class="DigNum (strict)"() -> ("Value"=w2100:i32)  [unwired: 2 in, 2 out]
        n1380 = Replace Array Subset(array=w2097, new element=w2093, index=1) -> (w2095:u16[])
        n1381 = property on="Steps6" class="DigNum (strict)"("Disabled"=w2101) -> ()  [unwired: 2 in, 2 out]
        n1382 = call "CRYGet Steps From F1 F2 Resolution.vi"("Steps/Tone"=w2100, "Stop Freq"=w2107, "Start Freq"=w2108, "Resolution"=w2093) -> ("Steps"=w2105:i32)  [unwired: 7 out]
        n1383 = Bundle By Name(cluster=w2094, "StepResolutionArray"=w2095, "Steps6(#)"=w2105) -> (w2109:T2)
        n1384 = property on="Steps6" class="DigNum (strict)"("Value"=w2105) -> ()  [unwired: 2 in, 2 out]
        n1385 = property on="Stimulus Out" class="Clust (strict)"("Val(Sgnl)"=w2109) -> ()  [unwired: 2 in, 2 out]
        n1386 = property on="Max Freq" class="DigNum (strict)"() -> ("Value"=w2098:dbl)  [unwired: 2 in, 2 out]
        n1387 = case shown="0..3" w2093 {
          selector: w2093 -> [_ w2114]
          tunnel: [w2113 w2116] -> w2099
          tunnel: w2098 -> [w2113 w2115]
          frame Default {
          }
          frame 0..3 {
            n1388 = call "CRYStimulus Freq Max Limit.vi"("Resolution"=w2114, "Max Freq"=w2115, "Input Val"=w2115) -> ("Output Val"=w2116:dbl)  [unwired: 1 in, 7 out]
          }
        }
        n1389 = flat-sequence {
          tunnel: w2099 -> [w2110]
          frame #0 {
            n1390 = property on="Res Max Freq" class="DigNum (strict)"("Value"=w2110) -> ()  [unwired: 2 in, 2 out]
          }
          frame #1 {
            n1391 = property on="StartFreq6(Hz)" class="DigNum (strict)"() -> ("Value"=w2112:dbl)  [unwired: 2 in, 2 out]
            n1392 = property on="StopFreq6(Hz)" class="DigNum (strict)"() -> ("Value"=w2111:dbl)  [unwired: 2 in, 2 out]
            n1393 = property on="StopFreq6(Hz)" class="DigNum (strict)"("Val(Sgnl)"=w2111) -> ()  [unwired: 2 in, 2 out]
            n1394 = property on="StartFreq6(Hz)" class="DigNum (strict)"("Val(Sgnl)"=w2112) -> ()  [unwired: 2 in, 2 out]
          }
        }
      }
      event "Step Resolution8": Value Change {
        n1395 = event-data() -> ("NewVal"=w2117:u16)  [unwired: 6 out]
        n1396 = Unbundle By Name(w2118) -> ("StepResolutionArray"=w2121:u16[])
        n1397 = Less?(x=w2117, y=u16 4) -> (x < y?=w2128:bool)
        n1398 = property on="StartFreq8(Hz)" class="DigNum (strict)"() -> ("Value"=w2132:dbl)  [unwired: 2 in, 2 out]
        n1399 = property on="StopFreq8(Hz)" class="DigNum (strict)"() -> ("Value"=w2131:dbl)  [unwired: 2 in, 2 out]
        n1400 = Select(t=u8 2 ("Disabled"), s=w2128, f=u8 0 ("Disabled")) -> (s? t:f=w2125:u8)
        n1401 = Replace Array Subset(array=w2121, new element=w2117, index=2) -> (w2119:u16[])
        n1402 = property on="Tones8" class="DigNum (strict)"("Disabled"=w2125) -> ()  [unwired: 2 in, 2 out]
        n1403 = property on="Tones8" class="DigNum (strict)"() -> ("Value"=w2124:i32)  [unwired: 2 in, 2 out]
        n1404 = call "CRYGet Steps From F1 F2 Resolution.vi"("Steps/Tone"=w2124, "Stop Freq"=w2131, "Start Freq"=w2132, "Resolution"=w2117) -> ("Steps"=w2129:i32)  [unwired: 7 out]
        n1405 = Bundle By Name(cluster=w2118, "StepResolutionArray"=w2119, "Tones8"=w2129) -> (w2133:T2)
        n1406 = property on="Max Freq" class="DigNum (strict)"() -> ("Value"=w2122:dbl)  [unwired: 2 in, 2 out]
        n1407 = property on="Tones8" class="DigNum (strict)"("Value"=w2129) -> ()  [unwired: 2 in, 2 out]
        n1408 = case shown="0..3" w2117 {
          selector: w2117 -> [_ w2138]
          tunnel: [w2137 w2140] -> w2123
          tunnel: w2122 -> [w2137 w2139]
          frame Default {
          }
          frame 0..3 {
            n1409 = call "CRYStimulus Freq Max Limit.vi"("Resolution"=w2138, "Max Freq"=w2139, "Input Val"=w2139) -> ("Output Val"=w2140:dbl)  [unwired: 1 in, 7 out]
          }
        }
        n1410 = property on="Stimulus Out" class="Clust (strict)"("Val(Sgnl)"=w2133) -> ()  [unwired: 2 in, 2 out]
        n1411 = flat-sequence {
          tunnel: w2123 -> [w2134]
          frame #0 {
            n1412 = property on="Res Max Freq" class="DigNum (strict)"("Value"=w2134) -> ()  [unwired: 2 in, 2 out]
          }
          frame #1 {
            n1413 = property on="StartFreq8(Hz)" class="DigNum (strict)"() -> ("Value"=w2135:dbl)  [unwired: 2 in, 2 out]
            n1414 = property on="StopFreq8(Hz)" class="DigNum (strict)"() -> ("Value"=w2136:dbl)  [unwired: 2 in, 2 out]
            n1415 = property on="StartFreq8(Hz)" class="DigNum (strict)"("Val(Sgnl)"=w2135) -> ()  [unwired: 2 in, 2 out]
            n1416 = property on="StopFreq8(Hz)" class="DigNum (strict)"("Val(Sgnl)"=w2136) -> ()  [unwired: 2 in, 2 out]
          }
        }
      }
      event "Steps1": Value Change {
        n1417 = event-data() -> ("NewVal"=w2142:i32)  [unwired: 6 out]
        n1418 = property on="Step Resolution1" class="Ring (strict)"() -> ("Value"=w2141:u16)  [unwired: 2 in, 2 out]
        n1419 = Bundle By Name(cluster=w2143, "Steps1"=w2142) -> (w2144:T2)
        n1420 = case shown="Default" w2141 {
          tunnel: w2142 -> [w2147 _]
          frame Default {
            n1421 = Less Or Equal?(x=w2147, y=1) -> (x <= y?=w2150:bool)
            n1422 = Select(t=u8 2 ("Disabled"), s=w2150, f=u8 0 ("Disabled")) -> (s? t:f=w2145:u8)
            n1423 = property on="StartFreq1(Hz)" class="DigNum (strict)"("Disabled"=w2145) -> ()  [unwired: 2 in, 2 out]
          }
          frame 0..3 {
          }
        }
        n1424 = property on="Stimulus Out" class="Clust (strict)"("Val(Sgnl)"=w2144) -> ()  [unwired: 2 in, 2 out]
      }
      event "Cycle/step1": Value Change {
        w2152 = u32 1 ("y")
        n1425 = event-data() -> ("NewVal"=w2153:u32)  [unwired: 6 out]
        n1426 = Greater?(x=w2153, y=w2152) -> (0:w2154:bool)
        n1427 = Select(t=w2153, s=w2154, f=w2152) -> (s? t:f=w2151:u32)
        n1428 = property on="Cycle/step1" class="DigNum (strict)"("Value"=w2151) -> ()  [unwired: 2 in, 2 out]
        n1429 = property on="Time/steps1(s)" class="DigNum (strict)"() -> ("Value"=w2158:dbl)  [unwired: 2 in, 2 out]
        n1430 = Divide(x=w2151, y=w2158) -> (x/y=w2156:dbl)
        n1431 = property on="Transition1" class="DigNum (strict)"("Value"=w2156) -> ()  [unwired: 2 in, 2 out]
        n1432 = Bundle By Name(cluster=w2155, "Cycle/step1(#)"=w2151, "Transition1"=w2156) -> (w2157:T2)
        n1433 = property on="Stimulus Out" class="Clust (strict)"("Val(Sgnl)"=w2157) -> ()  [unwired: 2 in, 2 out]
      }
      event "Time/steps1(s)": Value Change {
        w2160 = 0.0 ("y")
        n1434 = event-data() -> ("NewVal"=w2161:dbl)  [unwired: 6 out]
        n1435 = Greater?(x=w2161, y=w2160) -> (0:w2162:bool)
        n1436 = Select(t=w2161, s=w2162, f=w2160) -> (s? t:f=w2159:dbl)
        n1437 = property on="Time/steps1(s)" class="DigNum (strict)"("Value"=w2159) -> ()  [unwired: 2 in, 2 out]
        n1438 = property on="Cycle/step1" class="DigNum (strict)"() -> ("Value"=w2165:u32)  [unwired: 2 in, 2 out]
        n1439 = Divide(x=w2165, y=w2159) -> (x/y=w2164:dbl)
        n1440 = Bundle By Name(cluster=w2163, "Time/step1(s)"=w2159, "Transition1"=w2164) -> (w2166:T2)
        n1441 = property on="Transition1" class="DigNum (strict)"("Value"=w2164) -> ()  [unwired: 2 in, 2 out]
        n1442 = property on="Stimulus Out" class="Clust (strict)"("Val(Sgnl)"=w2166) -> ()  [unwired: 2 in, 2 out]
      }
      event "Sweept Rate2(s/dec)": Value Change {
        n1443 = event-data() -> ("NewVal"=w2169:dbl)  [unwired: 6 out]
        n1444 = Greater Than 0?(x=w2169) -> (x > 0?=w2170:bool)
        n1445 = Select(t=w2169, s=w2170, f=0.0) -> (s? t:f=w2167:dbl)
        n1446 = property on="Sweept Rate2(s/dec)" class="DigNum (strict)"("Value"=w2167) -> ()  [unwired: 2 in, 2 out]
        n1447 = Bundle By Name(cluster=w2171, "SweepRate2"=w2167) -> (w2172:T2)
        n1448 = property on="Stimulus Out" class="Clust (strict)"("Val(Sgnl)"=w2172) -> ()  [unwired: 2 in, 2 out]
      }
      event "Freq3(Hz)": Value Change {
        w2176 = 0.001 ("y")
        n1449 = event-data() -> ("NewVal"=w2175:dbl)  [unwired: 6 out]
        n1450 = Less?(x=w2175, y=w2176) -> (x < y?=w2177:bool)
        n1451 = case shown="False" w2177 {
          tunnel: [w2179 w2183] -> w2174
          tunnel: w2176 -> [_ w2183]
          tunnel: w2175 -> [w2181 _]
          frame False {
            n1452 = property on="Res Max Freq" class="DigNum (strict)"() -> ("Value"=w2180:dbl)  [unwired: 2 in, 2 out]
            n1453 = Less?(x=w2181, y=w2180) -> (x < y?=w2182:bool)
            n1454 = Select(t=w2181, s=w2182, f=w2180) -> (s? t:f=w2179:dbl)
          }
          frame True {
          }
        }
        n1455 = local write "RealFreq3(Hz)"(w2174) -> ()
        n1456 = Bundle By Name(cluster=w2173, "Freq3(Hz)"=w2174) -> (w2178:T2)
        n1457 = property on="Freq3(Hz)" class="DigNum (strict)"("Value"=w2174) -> ()  [unwired: 2 in, 2 out]
        n1458 = property on="Stimulus Out" class="Clust (strict)"("Val(Sgnl)"=w2178) -> ()  [unwired: 2 in, 2 out]
      }
      event "Cycles3": Value Change {
        w2185 = u32 1 ("y")
        n1459 = event-data() -> ("NewVal"=w2186:u32)  [unwired: 6 out]
        n1460 = Greater?(x=w2186, y=w2185) -> (0:w2187:bool)
        n1461 = Select(t=w2186, s=w2187, f=w2185) -> (s? t:f=w2184:u32)
        n1462 = property on="Cycles3" class="DigNum (strict)"("Value"=w2184) -> ()  [unwired: 2 in, 2 out]
        n1463 = Bundle By Name(cluster=w2188, "Cycles3(#)"=w2184) -> (w2189:T2)
        n1464 = property on="Stimulus Out" class="Clust (strict)"("Val(Sgnl)"=w2189) -> ()  [unwired: 2 in, 2 out]
      }
      event "Step Size3": Value Change {
        n1465 = event-data() -> ("NewVal"=w2191:dbl)  [unwired: 6 out]
        n1466 = Bundle By Name(cluster=w2190, "StepSize3"=w2191) -> (w2192:T2)
        n1467 = property on="Stimulus Out" class="Clust (strict)"("Val(Sgnl)"=w2192) -> ()  [unwired: 2 in, 2 out]
      }
      event "Steps3": Value Change {
        n1468 = event-data() -> ("NewVal"=w2194:i32)  [unwired: 6 out]
        n1469 = flat-sequence {
          tunnel: [w2197] -> _
          tunnel: w2194 -> [w2197]
          tunnel: w2193 -> [w2199]
          frame #0 {
            w2196 = u32 1 ("y")
            n1470 = Greater?(x=w2197, y=w2196) -> (0:w2198:bool)
            n1471 = Select(t=w2197, s=w2198, f=w2196) -> (s? t:f=w2195:u32)
            n1472 = Bundle By Name(cluster=w2199, "Steps3(#)"=w2195) -> (w2200:T2)
            n1473 = property on="Stimulus Out" class="Clust (strict)"("Val(Sgnl)"=w2200) -> ()  [unwired: 2 in, 2 out]
            n1474 = property on="Steps3" class="DigNum (strict)"("Value"=w2195) -> ()  [unwired: 2 in, 2 out]
          }
          frame #1 {
            n1475 = property on="Update" class="Bool (strict)"("Val(Sgnl)"=TRUE ("Value (Signaling)")) -> ()  [unwired: 2 in, 2 out]
          }
        }
      }
      event "Peak unit4": Value Change {
        n1476 = event-data() -> ("NewVal"=w2207:u16)  [unwired: 6 out]
        n1477 = property on="Wave Path4" class="Path"() -> ("Value"=w2208:path)  [unwired: 2 in, 2 out]
        n1478 = Path To String(path=w2208) -> (string=w2205:string)
        n1479 = call "CRYGet Wave File Information.vi"("FileNameStr"=w2205) -> ("wave info"=w2204:T18, "Error Output"=w2202:errorcluster)  [unwired: 13 out]
        n1480 = case shown="No Error" w2202 {
          tunnel: w2207 -> [w2213 _]
          tunnel: [w2212 0.0 ("peak %FSD")] -> w2206
          tunnel: w2204 -> [w2211 _]
          frame No Error {
            n1481 = case shown="1" w2213 {
              tunnel: w2211 -> [w2215 w2217]
              tunnel: [w2214 w2216] -> w2212
              frame 0, Default {
                n1482 = Unbundle By Name(w2215) -> ("peak FSD"=w2214:dbl)
              }
              frame 1 {
                n1483 = Unbundle By Name(w2217) -> ("peak %FSD"=w2216:dbl)
              }
            }
          }
          frame Error {
          }
        }
        n1484 = property on="Peak unit4" class="Ring (strict)"() -> ("RingText.Text"=w2209:string)  [unwired: 2 in, 2 out]
        n1485 = property on="Peak value4" class="DigNum (strict)"("Value"=w2206) -> ()  [unwired: 2 in, 2 out]
        n1486 = Bundle By Name(cluster=w2203, "Peak_unit4"=w2209, "Peak_Value4"=w2206) -> (w2210:T2)
        n1487 = property on="Stimulus Out" class="Clust (strict)"("Val(Sgnl)"=w2210) -> ()  [unwired: 2 in, 2 out]
      }
      event "RMS unit4": Value Change {
        n1488 = event-data() -> ("NewVal"=w2225:u16)  [unwired: 6 out]
        n1489 = property on="Wave Path4" class="Path"() -> ("Value"=w2223:path)  [unwired: 2 in, 2 out]
        n1490 = Path To String(path=w2223) -> (string=w2222:string)
        n1491 = call "CRYGet Wave File Information.vi"("FileNameStr"=w2222) -> ("wave info"=w2221:T18, "Error Output"=w2219:errorcluster)  [unwired: 1 in, 12 out]
        n1492 = case shown="No Error" w2219 {
          tunnel: w2225 -> [w2230 _]
          tunnel: [w2229 0.0 ("rms %FSD")] -> w2224
          tunnel: w2221 -> [w2228 _]
          frame No Error {
            n1493 = case shown="0, Default" w2230 {
              tunnel: w2228 -> [w2232 w2234]
              tunnel: [w2231 w2233] -> w2229
              frame 0, Default {
                n1494 = Unbundle By Name(w2232) -> ("rms FSD"=w2231:dbl)
              }
              frame 1 {
                n1495 = Unbundle By Name(w2234) -> ("rms %FSD"=w2233:dbl)
              }
            }
          }
          frame Error {
          }
        }
        n1496 = property on="RMS unit4" class="Ring (strict)"() -> ("RingText.Text"=w2226:string)  [unwired: 2 in, 2 out]
        n1497 = property on="RMS value4" class="DigNum (strict)"("Value"=w2224) -> ()  [unwired: 2 in, 2 out]
        n1498 = Bundle By Name(cluster=w2220, "RMS_unit4"=w2226, "RMS_Value4"=w2224) -> (w2227:T2)
        n1499 = property on="Stimulus Out" class="Clust (strict)"("Val(Sgnl)"=w2227) -> ()  [unwired: 2 in, 2 out]
      }
      event "Wave Path4": Value Change {
        n1500 = event-data() -> ("NewVal"=w2247:path)  [unwired: 6 out]
        n1501 = Path To String(path=w2247) -> (string=w2241:string)
        n1502 = call "CRYGet Wave File Information.vi"("FileNameStr"=w2241) -> ("sound format"=w2238:T19, "wave info"=w2240:T18, "Error Output"=w2237:errorcluster)  [unwired: 12 out]
        n1503 = Unbundle By Name(w2237) -> ("status"=w2236:bool)
        n1504 = case shown="False" w2236 {
          tunnel: w2240 -> [w2257 _]
          tunnel: [w2255 w2273] -> w2246
          tunnel: [w2254 w2273] -> w2245
          tunnel: [w2253 w2272] -> w2244
          tunnel: [w2252 w2272] -> w2243
          tunnel: w2238 -> [w2251 _]
          frame False {
            n1505 = Unbundle By Name(w2257) -> ("format str"=w2253:string, "Time Str"=w2252:string)
            n1506 = Unbundle By Name(w2251) -> ("number of channels"=w2250:i32)
            n1507 = property on="wave info" class="Str"("Value"=w2253) -> ()  [unwired: 2 in, 2 out]
            n1508 = property on="wave time" class="Str"("Value"=w2252) -> ()  [unwired: 2 in, 2 out]
            n1509 = case shown="1" w2250 {
              tunnel: [T9."Enabled" ("Disabled") T9."Disabled and Grayed Out" ("Disabled")] -> w2249
              frame Default {
              }
              frame 1 {
                w2260 = u16 0 items=["Left", "Right"] ("Channel")
                n1510 = property on="Wave Channel" class="Ring (strict)"("Value"=w2260) -> ()  [unwired: 2 in, 2 out]
              }
            }
            n1511 = property on="Peak unit4" class="Ring (strict)"() -> ("Value"=w2258:u16)  [unwired: 2 in, 2 out]
            n1512 = property on="RMS unit4" class="Ring (strict)"() -> ("Value"=w2256:u16)  [unwired: 2 in, 2 out]
            n1513 = case shown="1" w2258 {
              tunnel: w2257 -> [w2267 w2269]
              tunnel: [w2266 w2268] -> w2255
              frame 0, Default {
                n1514 = Unbundle By Name(w2267) -> ("peak FSD"=w2266:dbl)
              }
              frame 1 {
                n1515 = Unbundle By Name(w2269) -> ("peak %FSD"=w2268:dbl)
              }
            }
            n1516 = case shown="1" w2256 {
              tunnel: w2257 -> [w2263 w2265]
              tunnel: [w2262 w2264] -> w2254
              frame 0, Default {
                n1517 = Unbundle By Name(w2263) -> ("rms FSD"=w2262:dbl)
              }
              frame 1 {
                n1518 = Unbundle By Name(w2265) -> ("rms %FSD"=w2264:dbl)
              }
            }
            n1519 = property on="Wave Channel" class="Ring (strict)"("DisabledEnum"=w2249) -> ()  [unwired: 2 in, 2 out]
            n1520 = property on="Peak value4" class="DigNum (strict)"("Value"=w2255) -> ()  [unwired: 2 in, 2 out]
            n1521 = property on="RMS value4" class="DigNum (strict)"("Value"=w2254) -> ()  [unwired: 2 in, 2 out]
          }
          frame True {
            w2270 = u16 0 items=["Left", "Right"] ("Channel")
            w2274 = u16 0 items=["dB FSD", "% FSD"] ("Peak unit4")
            w2273 = 0.0 ("Peak value4")
            w2272 = "" ("wave info")
            n1522 = property on="Wave Channel" class="Ring (strict)"("Value"=w2270) -> ()  [unwired: 2 in, 2 out]
            n1523 = property on="Wave Channel" class="Ring (strict)"("DisabledEnum"=T9."Disabled and Grayed Out" ("Disabled")) -> ()  [unwired: 2 in, 2 out]
            n1524 = local write "wave time"(w2272) -> ()
            n1525 = local write "wave info"(w2272) -> ()
            n1526 = local write "Peak value4"(w2273) -> ()
            n1527 = local write "RMS value4"(w2273) -> ()
            n1528 = local write "Peak unit4"(w2274) -> ()
            n1529 = local write "RMS unit4"(w2274) -> ()
          }
        }
        n1530 = property on="Wave Path4" class="Path"() -> ("Text.Text"=w2248:string)  [unwired: 2 in, 2 out]
        n1531 = Bundle By Name(cluster=w2239, "WavePath4"=w2248, "Peak_Value4"=w2246, "RMS_Value4"=w2245, "wave Info"=w2244, "wave time"=w2243) -> (w2242:T2)
        n1532 = property on="Stimulus Out" class="Clust (strict)"("Val(Sgnl)"=w2242) -> ()  [unwired: 2 in, 2 out]
      }
      event "Peak value4": Value Change {
        n1533 = event-data() -> ("NewVal"=w2276:dbl)  [unwired: 6 out]
        n1534 = Bundle By Name(cluster=w2275, "Peak_Value4"=w2276) -> (w2277:T2)
        n1535 = property on="Stimulus Out" class="Clust (strict)"("Val(Sgnl)"=w2277) -> ()  [unwired: 2 in, 2 out]
      }
      event "RMS value4": Value Change {
        n1536 = event-data() -> ("NewVal"=w2279:dbl)  [unwired: 6 out]
        n1537 = Bundle By Name(cluster=w2278, "RMS_Value4"=w2279) -> (w2280:T2)
        n1538 = property on="Stimulus Out" class="Clust (strict)"("Val(Sgnl)"=w2280) -> ()  [unwired: 2 in, 2 out]
      }
      event "wave info": Value Change {
        n1539 = event-data() -> ("NewVal"=w2282:string)  [unwired: 6 out]
        n1540 = Bundle By Name(cluster=w2281, "wave Info"=w2282) -> (w2283:T2)
        n1541 = property on="Stimulus Out" class="Clust (strict)"("Val(Sgnl)"=w2283) -> ()  [unwired: 2 in, 2 out]
      }
      event "wave time": Value Change {
        n1542 = event-data() -> ("NewVal"=w2285:string)  [unwired: 6 out]
        n1543 = Bundle By Name(cluster=w2284, "wave time"=w2285) -> (w2286:T2)
        n1544 = property on="Stimulus Out" class="Clust (strict)"("Val(Sgnl)"=w2286) -> ()  [unwired: 2 in, 2 out]
      }
      event "Wave Channel": Value Change {
        n1545 = event-data() -> ("NewVal"=w2287:u16)  [unwired: 6 out]
        n1546 = Bundle By Name(cluster=w2288, "Channel Sel"=w2287) -> (w2289:T2)
        n1547 = property on="Stimulus Out" class="Clust (strict)"("Val(Sgnl)"=w2289) -> ()  [unwired: 2 in, 2 out]
      }
      event "Stimulus Change": Value Change {
        n1548 = event-data() -> ("NewVal"=w2290:string)  [unwired: 6 out]
        n1549 = flat-sequence {
          tunnel: w2290 -> [w2292]
          frame #0 {
            n1550 = call "CRYUnflatten Stimulus.vi"("Flatten Stimulus"=w2292) -> ("Stimulus"=w2291:T2)  [unwired: 10 out]
            n1551 = local write "Stimulus In"(w2291) -> ()
          }
          frame #1 {
            n1552 = local write "Load_Test"(TRUE ("Load_Test")) -> ()
          }
        }
      }
      event "StopFreq7(Hz)": Value Change {
        w2297 = 0.001 ("y")
        n1553 = event-data() -> ("NewVal"=w2296:dbl)  [unwired: 6 out]
        n1554 = Less?(x=w2296, y=w2297) -> (x < y?=w2298:bool)
        n1555 = case shown="False" w2298 {
          tunnel: [w2303 w2304] -> w2295
          tunnel: w2297 -> [_ w2304]
          tunnel: w2296 -> [w2301 _]
          frame False {
            n1556 = property on="Res Max Freq" class="DigNum (strict)"() -> ("Value"=w2300:dbl)  [unwired: 2 in, 2 out]
            n1557 = Less?(x=w2301, y=w2300) -> (x < y?=w2302:bool)
            n1558 = Select(t=w2301, s=w2302, f=w2300) -> (s? t:f=w2303:dbl)
          }
          frame True {
          }
        }
        n1559 = property on="StopFreq7(Hz)" class="DigNum (strict)"("Value"=w2295) -> ()  [unwired: 2 in, 2 out]
        n1560 = Bundle By Name(cluster=w2294, "MaxFreq7(Hz)"=w2295) -> (w2299:T2)
        n1561 = property on="Stimulus Out" class="Clust (strict)"("Val(Sgnl)"=w2299) -> ()  [unwired: 2 in, 2 out]
      }
      event "StartFreq7(Hz)": Value Change {
        w2308 = 0.001 ("y")
        n1562 = event-data() -> ("NewVal"=w2307:dbl)  [unwired: 6 out]
        n1563 = Less?(x=w2307, y=w2308) -> (x < y?=w2309:bool)
        n1564 = case shown="False" w2309 {
          tunnel: [w2314 w2315] -> w2306
          tunnel: w2308 -> [_ w2315]
          tunnel: w2307 -> [w2312 _]
          frame False {
            n1565 = property on="Res Max Freq" class="DigNum (strict)"() -> ("Value"=w2311:dbl)  [unwired: 2 in, 2 out]
            n1566 = Less?(x=w2312, y=w2311) -> (x < y?=w2313:bool)
            n1567 = Select(t=w2312, s=w2313, f=w2311) -> (s? t:f=w2314:dbl)
          }
          frame True {
          }
        }
        n1568 = Bundle By Name(cluster=w2305, "MinFreq7(Hz)"=w2306) -> (w2310:T2)
        n1569 = property on="StartFreq7(Hz)" class="DigNum (strict)"("Value"=w2306) -> ()  [unwired: 2 in, 2 out]
        n1570 = property on="Stimulus Out" class="Clust (strict)"("Val(Sgnl)"=w2310) -> ()  [unwired: 2 in, 2 out]
      }
      event "Duration7(s)": Value Change {
        w2316 = 0.001 ("y")
        n1571 = event-data() -> ("NewVal"=w2317:dbl)  [unwired: 6 out]
        n1572 = Greater?(x=w2317, y=w2316) -> (0:w2320:bool)
        n1573 = Select(t=w2317, s=w2320, f=w2316) -> (s? t:f=w2319:dbl)
        n1574 = property on="Duration7(s)" class="DigNum (strict)"("Value"=w2319) -> ()  [unwired: 2 in, 2 out]
        n1575 = Bundle By Name(cluster=w2318, "Duration7(s)"=w2319) -> (w2321:T2)
        n1576 = property on="Stimulus Out" class="Clust (strict)"("Val(Sgnl)"=w2321) -> ()  [unwired: 2 in, 2 out]
      }
      event "Transition1": Value Change {
        n1577 = event-data() -> ("NewVal"=w2323:dbl)  [unwired: 6 out]
        n1578 = Bundle By Name(cluster=w2322, "Transition1"=w2323) -> (w2324:T2)
        n1579 = property on="Stimulus Out" class="Clust (strict)"("Val(Sgnl)"=w2324) -> ()  [unwired: 2 in, 2 out]
      }
      event "StartAmp5": Value Change {
        n1580 = event-data() -> ("NewVal"=w2328:dbl)  [unwired: 6 out]
        n1581 = property on="dc_ctrl5_2" class="Slide (strict)"() -> ("Value"=w2329:u16)  [unwired: 2 in, 2 out]
        n1582 = case shown="0, Default" w2329 {
          tunnel: w2328 -> [w2342 w2350]
          tunnel: [w2341 w2349] -> w2327
          frame 0, Default {
            n1583 = Less Than 0?(x=w2342) -> (x < 0?=w2343:bool)
            n1584 = case shown="False" w2343 {
              tunnel: [w2344 0.0 ("x")] -> w2341
              tunnel: w2342 -> [w2346 _]
              frame False {
                w2345 = 10.0 ("y")
                n1585 = Less?(x=w2346, y=w2345) -> (x < y?=w2347:bool)
                n1586 = Select(t=w2346, s=w2347, f=w2345) -> (s? t:f=w2344:dbl)
              }
              frame True {
              }
            }
          }
          frame 1 {
            n1587 = Less Than 0?(x=w2350) -> (x < 0?=w2351:bool)
            n1588 = case shown="False" w2351 {
              tunnel: [w2352 0.0 ("x")] -> w2349
              tunnel: w2350 -> [w2354 _]
              frame False {
                w2353 = 0.003 ("y")
                n1589 = Less?(x=w2354, y=w2353) -> (x < y?=w2355:bool)
                n1590 = Select(t=w2354, s=w2355, f=w2353) -> (s? t:f=w2352:dbl)
              }
              frame True {
              }
            }
          }
        }
        n1591 = Unbundle By Name(w2325) -> ("Start(Stop)AmpArray"=w2338:dbl[])
        n1592 = property on="StartAmp5" class="DigNum (strict)"("Value"=w2327) -> ()  [unwired: 2 in, 2 out]
        n1593 = Index Array(array=w2338, index=1) -> (element=w2336:dbl)
        n1594 = property on="StopAmp5" class="DigNum (strict)"() -> ("Value"=w2335:dbl)  [unwired: 2 in, 2 out]
        n1595 = property on="Steps5" class="DigNum (strict)"() -> ("Value"=w2330:i32)  [unwired: 2 in, 2 out]
        n1596 = Subtract(x=w2327, y=w2335) -> (x-y=w2334:dbl)
        n1597 = Build Array(w2327, w2336) -> (w2339:dbl[])
        n1598 = Decrement(x=w2330) -> (x-1=w2333:i32)
        n1599 = Absolute Value(x=w2334) -> (abs(x)=w2331:dbl)
        n1600 = Less Or Equal To 0?(x=w2333) -> (x <= 0?=w2332:bool)
        n1601 = case shown="False" w2332 {
          tunnel: w2333 -> [w2358 _]
          tunnel: w2331 -> [w2359 _]
          tunnel: [w2357 0.0] -> w2326
          frame False {
            n1602 = Divide(x=w2359, y=w2358) -> (x/y=w2357:dbl)
          }
          frame True {
          }
        }
        n1603 = Bundle By Name(cluster=w2325, "Start(Stop)AmpArray"=w2339, "StepsSize5Val"=w2326) -> (w2340:T2)
        n1604 = property on="Stimulus Out" class="Clust (strict)"("Val(Sgnl)"=w2340) -> ()  [unwired: 2 in, 2 out]
        n1605 = property on="Steps Size5" class="DigNum (strict)"("Value"=w2326) -> ()  [unwired: 2 in, 2 out]
      }
      event "Level5": Value Change {
        n1606 = event-data() -> ("NewVal"=w2363:dbl)  [unwired: 6 out]
        n1607 = Less Than 0?(x=w2363) -> (x < 0?=w2364:bool)
        n1608 = case shown="False" w2364 {
          tunnel: [w2368 0.0 ("NewVal")] -> w2362
          tunnel: w2363 -> [w2367 _]
          frame False {
            n1609 = Greater?(x=w2367, y=10.0) -> (0:w2369:bool)
            n1610 = case shown="True" w2369 {
              tunnel: [w2370 10.0 ("NewVal")] -> w2368
              tunnel: w2367 -> [w2370 _]
              frame False {
              }
              frame True {
              }
            }
          }
          frame True {
          }
        }
        n1611 = property on="Level5" class="DigNum (strict)"("Value"=w2362) -> ()  [unwired: 2 in, 2 out]
        n1612 = Bundle By Name(cluster=w2361, "Level5"=w2362) -> (w2365:T2)
        n1613 = property on="Stimulus Out" class="Clust (strict)"("Val(Sgnl)"=w2365) -> ()  [unwired: 2 in, 2 out]
      }
      event "Steps5": Value Change {
        n1614 = event-data() -> ("NewVal"=w2385:i32)  [unwired: 6 out]
        n1615 = Less?(x=w2385, y=u32 1) -> (x < y?=w2381:bool)
        n1616 = case shown="True" w2381 {
          tunnel: [w2390 w2391] -> w2384
          tunnel: w2385 -> [w2390 _]
          frame False {
          }
          frame True {
            w2391 = u32 1 ("y")
            n1617 = property on="Steps5" class="DigNum (strict)"("Value"=w2391) -> ()  [unwired: 2 in, 2 out]
          }
        }
        n1618 = property on="StartAmp5" class="DigNum (strict)"() -> ("Value"=w2375:dbl)  [unwired: 2 in, 2 out]
        n1619 = property on="StopAmp5" class="DigNum (strict)"() -> ("Value"=w2376:dbl)  [unwired: 2 in, 2 out]
        n1620 = Subtract(x=w2375, y=w2376) -> (x-y=w2377:dbl)
        n1621 = Decrement(x=w2384) -> (x-1=w2378:u32)
        n1622 = Absolute Value(x=w2377) -> (abs(x)=w2380:dbl)
        n1623 = Less Or Equal To 0?(x=w2378) -> (x <= 0?=w2379:bool)
        n1624 = case shown="False" w2379 {
          tunnel: w2378 -> [w2387 _]
          tunnel: w2380 -> [w2388 _]
          tunnel: [w2386 0.0] -> w2374
          frame False {
            n1625 = Divide(x=w2388, y=w2387) -> (x/y=w2386:dbl)
          }
          frame True {
          }
        }
        n1626 = Bundle By Name(cluster=w2373, "Steps5(#)"=w2384, "StepsSize5Val"=w2374) -> (w2383:T2)
        n1627 = property on="Steps Size5" class="DigNum (strict)"("Value"=w2374) -> ()  [unwired: 2 in, 2 out]
        n1628 = property on="Stimulus Out" class="Clust (strict)"("Val(Sgnl)"=w2383) -> ()  [unwired: 2 in, 2 out]
      }
      event "Steps Size5": Value Change {
        n1629 = event-data() -> ("NewVal"=w2393:dbl)  [unwired: 6 out]
        n1630 = Bundle By Name(cluster=w2392, "StepsSize5Val"=w2393) -> (w2394:T2)
        n1631 = property on="Stimulus Out" class="Clust (strict)"("Val(Sgnl)"=w2394) -> ()  [unwired: 2 in, 2 out]
      }
      event "Time/Step5": Value Change {
        n1632 = event-data() -> ("NewVal"=w2398:dbl)  [unwired: 6 out]
        n1633 = Greater Than 0?(x=w2398) -> (x > 0?=w2399:bool)
        n1634 = Select(t=w2398, s=w2399, f=0.0) -> (s? t:f=w2396:dbl)
        n1635 = Bundle By Name(cluster=w2395, "Time/Step5"=w2396) -> (w2400:T2)
        n1636 = property on="Time/Step5" class="DigNum (strict)"("Value"=w2396) -> ()  [unwired: 2 in, 2 out]
        n1637 = property on="Stimulus Out" class="Clust (strict)"("Val(Sgnl)"=w2400) -> ()  [unwired: 2 in, 2 out]
      }
      event "Steps6": Value Change {
        n1638 = event-data() -> ("NewVal"=w2401:i32)  [unwired: 6 out]
        n1639 = property on="StepResolution6" class="Ring (strict)"() -> ("Value"=w2402:u16)  [unwired: 2 in, 2 out]
        n1640 = Bundle By Name(cluster=w2403, "Steps6(#)"=w2401) -> (w2404:T2)
        n1641 = case shown="Default" w2402 {
          tunnel: w2401 -> [w2407 _]
          frame Default {
            n1642 = Less Or Equal?(x=w2407, y=1) -> (x <= y?=w2410:bool)
            n1643 = Select(t=u8 2 ("Disabled"), s=w2410, f=u8 0 ("Disabled")) -> (s? t:f=w2405:u8)
            n1644 = property on="StartFreq6(Hz)" class="DigNum (strict)"("DisabledEnum"=w2405) -> ()  [unwired: 2 in, 2 out]
          }
          frame 0..3 {
          }
        }
        n1645 = property on="Stimulus Out" class="Clust (strict)"("Val(Sgnl)"=w2404) -> ()  [unwired: 2 in, 2 out]
      }
      event "Cycle/steps6": Value Change {
        w2412 = u32 1 ("y")
        n1646 = event-data() -> ("NewVal"=w2413:u32)  [unwired: 6 out]
        n1647 = Greater?(x=w2413, y=w2412) -> (0:w2414:bool)
        n1648 = Select(t=w2413, s=w2414, f=w2412) -> (s? t:f=w2411:u32)
        n1649 = property on="Cycle/steps6" class="DigNum (strict)"("Value"=w2411) -> ()  [unwired: 2 in, 2 out]
        n1650 = property on="Time/step6(s)" class="DigNum (strict)"() -> ("Value"=w2417:dbl)  [unwired: 2 in, 2 out]
        n1651 = Divide(x=w2411, y=w2417) -> (x/y=w2416:dbl)
        n1652 = Bundle By Name(cluster=w2415, "Cycle/Steps6(#)"=w2411, "Transition6"=w2416) -> (w2418:T2)
        n1653 = property on="Transition6" class="DigNum (strict)"("Value"=w2416) -> ()  [unwired: 2 in, 2 out]
        n1654 = property on="Stimulus Out" class="Clust (strict)"("Val(Sgnl)"=w2418) -> ()  [unwired: 2 in, 2 out]
      }
      event "Freq6(Hz)": Value Change {
        w2423 = 0.001 ("y")
        n1655 = event-data() -> ("NewVal"=w2422:dbl)  [unwired: 6 out]
        n1656 = Greater?(x=w2422, y=w2423) -> (0:w2420:bool)
        n1657 = Select(t=w2422, s=w2420, f=w2423) -> (s? t:f=w2421:dbl)
        n1658 = Bundle By Name(cluster=w2419, "Freq6(Hz)"=w2421) -> (w2424:T2)
        n1659 = property on="Freq6(Hz)" class="DigNum (strict)"("Value"=w2421) -> ()  [unwired: 2 in, 2 out]
        n1660 = property on="Stimulus Out" class="Clust (strict)"("Val(Sgnl)"=w2424) -> ()  [unwired: 2 in, 2 out]
      }
      event "Difference6(Hz)": Value Change {
        w2429 = 0.001 ("y")
        n1661 = event-data() -> ("NewVal"=w2428:dbl)  [unwired: 6 out]
        n1662 = Greater?(x=w2428, y=w2429) -> (0:w2426:bool)
        n1663 = Select(t=w2428, s=w2426, f=w2429) -> (s? t:f=w2427:dbl)
        n1664 = property on="Difference6(Hz)" class="DigNum (strict)"("Value"=w2427) -> ()  [unwired: 2 in, 2 out]
        n1665 = Bundle By Name(cluster=w2425, "Difference6(Hz)"=w2427) -> (w2430:T2)
        n1666 = property on="Stimulus Out" class="Clust (strict)"("Val(Sgnl)"=w2430) -> ()  [unwired: 2 in, 2 out]
      }
      event "Time/step6(s)": Value Change {
        n1667 = event-data() -> ("NewVal"=w2434:dbl)  [unwired: 6 out]
        n1668 = Less Than 0?(x=w2434) -> (x < 0?=w2435:bool)
        n1669 = Select(t=0.0, s=w2435, f=w2434) -> (s? t:f=w2432:dbl)
        n1670 = property on="Time/step6(s)" class="DigNum (strict)"("Value"=w2432) -> ()  [unwired: 2 in, 2 out]
        n1671 = property on="Cycle/steps6" class="DigNum (strict)"() -> ("Value"=w2437:u32)  [unwired: 2 in, 2 out]
        n1672 = Divide(x=w2437, y=w2432) -> (x/y=w2436:dbl)
        n1673 = Bundle By Name(cluster=w2431, "Time/Steps6(s)"=w2432, "Transition6"=w2436) -> (w2438:T2)
        n1674 = property on="Transition6" class="DigNum (strict)"("Value"=w2436) -> ()  [unwired: 2 in, 2 out]
        n1675 = property on="Stimulus Out" class="Clust (strict)"("Val(Sgnl)"=w2438) -> ()  [unwired: 2 in, 2 out]
      }
      event "StartFreq8(Hz)": Value Change {
        n1676 = event-data() -> ("NewVal"=w2448:dbl)  [unwired: 6 out]
        n1677 = property on="Res Max Freq" class="DigNum (strict)"() -> ("Value"=w2449:dbl)  [unwired: 2 in, 2 out]
        n1678 = property on="Step Resolution8" class="Ring (strict)"() -> ("Value"=w2441:u16)  [unwired: 2 in, 2 out]
        n1679 = call "CRYStimulus Freq Max Limit.vi"("Resolution"=w2441, "Max Freq"=w2449, "Input Val"=w2448) -> ("Decrement Val"=w2444:dbl, "Output Val"=w2447:dbl)  [unwired: 1 in, 6 out]
        n1680 = property on="StartFreq8(Hz)" class="DigNum (strict)"("Increment"=w2444) -> ()  [unwired: 2 in, 2 out]
        n1681 = property on="StopFreq8(Hz)" class="DigNum (strict)"() -> ("Value"=w2445:dbl)  [unwired: 2 in, 2 out]
        n1682 = property on="Tones8" class="DigNum (strict)"() -> ("Value"=w2442:i32)  [unwired: 2 in, 2 out]
        n1683 = call "CRYGet Steps From F1 F2 Resolution.vi"("Steps/Tone"=w2442, "Stop Freq"=w2447, "Start Freq"=w2445, "Resolution"=w2441) -> ("Stop Freq Out"=w2446:dbl, "Steps"=w2439:i32)  [unwired: 6 out]
        n1684 = case shown="Default" w2441 {
          tunnel: w2446 -> [_ w2462]
          tunnel: w2445 -> [_ w2461]
          tunnel: [w2451 w2457] -> w2440
          tunnel: w2439 -> [w2453 _]
          frame Default {
            n1685 = Less Or Equal?(x=w2453, y=1) -> (x <= y?=w2456:bool)
            n1686 = Select(t=u8 2 ("Disabled"), s=w2456, f=u8 0 ("Disabled")) -> (s? t:f=w2451:u8)
          }
          frame 0..3 {
            n1687 = Equal?(x=w2462, y=w2461) -> (x = y?=w2460:bool)
            n1688 = Select(t=u8 2 ("Disabled"), s=w2460, f=u8 0 ("Disabled")) -> (s? t:f=w2457:u8)
          }
        }
        n1689 = property on="StartFreq8(Hz)" class="DigNum (strict)"("Value"=w2446) -> ()  [unwired: 2 in, 2 out]
        n1690 = property on="Tones8" class="DigNum (strict)"("Value"=w2439) -> ()  [unwired: 2 in, 2 out]
        n1691 = Bundle By Name(cluster=w2443, "Tones8"=w2439, "MinFreq8(Hz)"=w2446) -> (w2450:T2)
        n1692 = property on="Stimulus Out" class="Clust (strict)"("Val(Sgnl)"=w2450) -> ()  [unwired: 2 in, 2 out]
        n1693 = property on="StartFreq8(Hz)" class="DigNum (strict)"("Disabled"=w2440) -> ()  [unwired: 2 in, 2 out]
      }
      event "StopFreq8(Hz)": Value Change {
        n1694 = event-data() -> ("NewVal"=w2472:dbl)  [unwired: 6 out]
        n1695 = property on="StartFreq8(Hz)" class="DigNum (strict)" props=["Value"]() -> ()  [unwired: 2 in, 3 out]
        n1696 = property on="Res Max Freq" class="DigNum (strict)"() -> ("Value"=w2473:dbl)  [unwired: 2 in, 2 out]
        n1697 = property on="Step Resolution8" class="Ring (strict)"() -> ("Value"=w2465:u16)  [unwired: 2 in, 2 out]
        n1698 = call "CRYStimulus Freq Max Limit.vi"("Resolution"=w2465, "Max Freq"=w2473, "Input Val"=w2472) -> ("Decrement Val"=w2468:dbl, "Output Val"=w2471:dbl)  [unwired: 1 in, 6 out]
        n1699 = property on="StopFreq8(Hz)" class="DigNum (strict)"("Increment"=w2468) -> ()  [unwired: 2 in, 2 out]
        n1700 = property on="StartFreq8(Hz)" class="DigNum (strict)"() -> ("Value"=w2469:dbl)  [unwired: 2 in, 2 out]
        n1701 = property on="Tones8" class="DigNum (strict)"() -> ("Value"=w2466:i32)  [unwired: 2 in, 2 out]
        n1702 = call "CRYGet Steps From F1 F2 Resolution.vi"("Steps/Tone"=w2466, "Stop Freq"=w2469, "Start Freq"=w2471, "Resolution"=w2465) -> ("Start Freq Out"=w2470:dbl, "Steps"=w2463:i32)  [unwired: 6 out]
        n1703 = Bundle By Name(cluster=w2467, "Tones8"=w2463, "MaxFreq8(Hz)"=w2470) -> (w2474:T2)
        n1704 = property on="StopFreq8(Hz)" class="DigNum (strict)"("Value"=w2470) -> ()  [unwired: 2 in, 2 out]
        n1705 = property on="Tones8" class="DigNum (strict)"("Value"=w2463) -> ()  [unwired: 2 in, 2 out]
        n1706 = case shown="Default" w2465 {
          tunnel: w2470 -> [_ w2486]
          tunnel: w2469 -> [_ w2485]
          tunnel: [w2477 w2481] -> w2464
          tunnel: w2463 -> [w2476 _]
          frame Default {
            n1707 = Less Or Equal?(x=w2476, y=1) -> (x <= y?=w2480:bool)
            n1708 = Select(t=u8 2 ("Disabled"), s=w2480, f=u8 0 ("Disabled")) -> (s? t:f=w2477:u8)
          }
          frame 0..3 {
            n1709 = Equal?(x=w2486, y=w2485) -> (x = y?=w2484:bool)
            n1710 = Select(t=u8 2 ("Disabled"), s=w2484, f=u8 0 ("Disabled")) -> (s? t:f=w2481:u8)
          }
        }
        n1711 = property on="Stimulus Out" class="Clust (strict)"("Val(Sgnl)"=w2474) -> ()  [unwired: 2 in, 2 out]
        n1712 = property on="StartFreq8(Hz)" class="DigNum (strict)"("Disabled"=w2464) -> ()  [unwired: 2 in, 2 out]
      }
      event "Tones8": Value Change {
        n1713 = event-data() -> ("NewVal"=w2488:i32)  [unwired: 6 out]
        n1714 = Bundle By Name(cluster=w2489, "Tones8"=w2488) -> (w2490:T2)
        n1715 = property on="Step Resolution8" class="Ring (strict)"() -> ("Value"=w2487:u16)  [unwired: 2 in, 2 out]
        n1716 = property on="Stimulus Out" class="Clust (strict)"("Val(Sgnl)"=w2490) -> ()  [unwired: 2 in, 2 out]
        n1717 = case shown="Default" w2487 {
          tunnel: w2488 -> [_ w2492]
          frame 0..3 {
          }
          frame Default {
            n1718 = Less Or Equal?(x=w2492, y=1) -> (x <= y?=w2496:bool)
            n1719 = Select(t=u8 2 ("Disabled"), s=w2496, f=u8 0 ("Disabled")) -> (s? t:f=w2491:u8)
            n1720 = property on="StartFreq8(Hz)" class="DigNum (strict)"("Disabled"=w2491) -> ()  [unwired: 2 in, 2 out]
          }
        }
      }
      event "Duration8(s)": Value Change {
        n1721 = event-data() -> ("NewVal"=w2499:dbl)  [unwired: 6 out]
        n1722 = Less Than 0?(x=w2499) -> (x < 0?=w2501:bool)
        n1723 = Select(t=0.0 ("x"), s=w2501, f=w2499) -> (s? t:f=w2498:dbl)
        n1724 = Bundle By Name(cluster=w2497, "Duration8(s)"=w2498) -> (w2502:T2)
        n1725 = property on="Duration8(s)" class="DigNum (strict)"("Value"=w2498) -> ()  [unwired: 2 in, 2 out]
        n1726 = property on="Stimulus Out" class="Clust (strict)"("Val(Sgnl)"=w2502) -> ()  [unwired: 2 in, 2 out]
      }
      event "dc_ctrl5_2": Value Change {
        n1727 = event-data() -> ("NewVal"=w2508:u16)  [unwired: 6 out]
        n1728 = Equal To 0?(x=w2508) -> (x = 0?=w2507:bool)
        n1729 = Select(t="V" ("Caption.Text"), s=w2507, f="A" ("Caption.Text")) -> (s? t:f=w2503:string)
        n1730 = Bundle By Name(cluster=w2504, "dc_ctrl5_2"=w2508) -> (w2509:T2)
        n1731 = property on="unit5_2" class="Str"("Value"=w2503) -> ()  [unwired: 2 in, 2 out]
        n1732 = property on="unit5_1" class="Str"("Value"=w2503) -> ()  [unwired: 2 in, 2 out]
        n1733 = property on="Stimulus Out" class="Clust (strict)"("Val(Sgnl)"=w2509) -> ()  [unwired: 2 in, 2 out]
      }
      event "Ratio6": Value Change {
        n1734 = event-data() -> ("NewVal"=w2515:u16)  [unwired: 6 out]
        n1735 = Equal?(x=w2515, y=u16 5) -> (x = y?=w2511:bool)
        n1736 = property on="Ratio Freq6(Hz)" class="DigNum (strict)"("Visible"=w2511) -> ()  [unwired: 2 in, 2 out]
        n1737 = property on="Ratio6" class="Ring (strict)"() -> ("RingText.Text"=w2512:string)  [unwired: 2 in, 2 out]
        n1738 = Bundle By Name(cluster=w2510, "Ratio6"=w2512) -> (w2513:T2)
        n1739 = property on="Stimulus Out" class="Clust (strict)"("Val(Sgnl)"=w2513) -> ()  [unwired: 2 in, 2 out]
      }
      event "Transition6": Value Change {
        n1740 = event-data() -> ("NewVal"=w2517:dbl)  [unwired: 6 out]
        n1741 = Bundle By Name(cluster=w2516, "Transition6"=w2517) -> (w2518:T2)
        n1742 = property on="Stimulus Out" class="Clust (strict)"("Val(Sgnl)"=w2518) -> ()  [unwired: 2 in, 2 out]
      }
      event "Noise Type7": Value Change {
        n1743 = event-data() -> ("NewVal"=w2520:u16)  [unwired: 6 out]
        n1744 = Bundle By Name(cluster=w2519, "NoiseType7"=w2520) -> (w2521:T2)
        n1745 = property on="Stimulus Out" class="Clust (strict)"("Val(Sgnl)"=w2521) -> ()  [unwired: 2 in, 2 out]
      }
      event "Ratio Freq6(Hz)": Value Change {
        w2525 = 0.001 ("y")
        n1746 = event-data() -> ("NewVal"=w2526:dbl)  [unwired: 6 out]
        n1747 = Greater?(x=w2526, y=w2525) -> (0:w2523:bool)
        n1748 = Select(t=w2526, s=w2523, f=w2525) -> (s? t:f=w2524:dbl)
        n1749 = Bundle By Name(cluster=w2522, "RatioVal6"=w2524) -> (w2527:T2)
        n1750 = property on="Ratio Freq6(Hz)" class="DigNum (strict)"("Value"=w2524) -> ()  [unwired: 2 in, 2 out]
        n1751 = property on="Stimulus Out" class="Clust (strict)"("Val(Sgnl)"=w2527) -> ()  [unwired: 2 in, 2 out]
      }
      event "Control6 Tab": Value Change {
        n1752 = event-data() -> ("NewVal"=w2529:enum32{"Master Tone", "Slave Tone"})  [unwired: 6 out]
        n1753 = Bundle By Name(cluster=w2528, "TabCtrl6"=w2529) -> (w2530:T2)
        n1754 = property on="Stimulus Out" class="Clust (strict)"("Val(Sgnl)"=w2530) -> ()  [unwired: 2 in, 2 out]
      }
      event "Rounding Val8": Value Change {
        w2535 = 0.1 ("y")
        n1755 = event-data() -> ("NewVal"=w2534:dbl)  [unwired: 6 out]
        n1756 = Greater?(x=w2534, y=w2535) -> (0:w2532:bool)
        n1757 = Select(t=w2534, s=w2532, f=w2535) -> (s? t:f=w2533:dbl)
        n1758 = Bundle By Name(cluster=w2531, "RoundingVal8"=w2533) -> (w2536:T2)
        n1759 = property on="Rounding Val8" class="DigNum (strict)"("Value"=w2533) -> ()  [unwired: 2 in, 2 out]
        n1760 = property on="Stimulus Out" class="Clust (strict)"("Val(Sgnl)"=w2536) -> ()  [unwired: 2 in, 2 out]
      }
      event "Freq Rounding8": Value Change {
        n1761 = event-data() -> ("NewVal"=w2538:bool)  [unwired: 6 out]
        n1762 = property on="Rounding Val8" class="DigNum (strict)"("Visible"=w2538) -> ()  [unwired: 2 in, 2 out]
        n1763 = Bundle By Name(cluster=w2537, "FreqRounding8"=w2538) -> (w2539:T2)
        n1764 = property on="Stimulus Out" class="Clust (strict)"("Val(Sgnl)"=w2539) -> ()  [unwired: 2 in, 2 out]
      }
      event "Help": Value Change {
        n1765 = event-data() -> ("NewVal"=w2540:string)  [unwired: 6 out]
        n1766 = Bundle By Name(cluster=w2544, "Help"=w2540) -> (w2545:T2)
        n1767 = property on="Stimulus Out" class="Clust (strict)"("Val(Sgnl)"=w2545) -> ()  [unwired: 2 in, 2 out]
        n1768 = global read "CRYStimulus Global.vi" "Stimulus Vi Ref"() -> (w2543:refnum<vi>)
        n1769 = call "CRYGet String Reference.vi"("Label Name"="Help Change" ("Control Name"), "VI Refnum"=w2543) -> ("String Ref Out"=w2541:refnum<vi>)  [unwired: 7 in, 2 out]
        n1770 = property class="Str"(reference=w2541, "Val(Sgnl)"=w2540) -> ()  [unwired: 1 in, 2 out]
      }
      event "Channel Change": Value Change {
        # "set Vmax(V), Sampling Rate and so on According to Hardware."
        n1771 = event-data() -> ("NewVal"=w2549:string)  [unwired: 6 out]
        n1772 = call "CRYGet Current Calibration Info.vi"("Is Input?"=FALSE, "Signal Type Name"=w2549) -> ("Calibration All Cluster"=w2560:T20)  [unwired: 9 out]
        n1773 = call "CRYGet Hardware Info From Signal Type.vi"("Calibration In"=w2546, "Hardware In"=w2548, "Signal Type"=w2549, "In/Out?"=FALSE) -> ("Channel Info Out"=w2547:T8)  [unwired: 5 in, 2 out]
        n1774 = local read "Vmax (V)"() -> (w2554:dbl)
        n1775 = Unbundle By Name(w2547) -> ("Anti-aliasing Factor (%fs)"=w2559:sgl)  [unwired: 1 out]
        n1776 = Unbundle By Name(w2560) -> ("Sens Curve"=w2567:T6)
        n1777 = Square Root(x=2.0) -> (sqrt(x)=w2583:dbl)
        n1778 = Multiply(x=w2554, y=w2583) -> (x*y=w2582:dbl)
        n1779 = Unbundle By Name(w2567) -> ("Curve"=w2580:cluster{"x":dbl, "y":dbl, "z":dbl}[], "Y dB ref"=w2553:dbl, "Y unit"=w2552:string, "Y data"=w2558:u16)
        n1780 = Index Array(array=w2580) -> (element=w2581:cluster{"x":dbl, "y":dbl, "z":dbl})  [unwired: 1 in]
        n1781 = Unbundle By Name(w2581) -> ("y"=w2557:dbl)
        n1782 = Divide(x=w2582, y=2.0) -> (x/y=w2563:dbl)
        n1783 = case shown="0, Default" w2558 {
          tunnel: w2557 -> [w2589 w2590]
          tunnel: [w2588 w2590] -> w2556
          tunnel: w2553 -> [w2587 _]
          frame 0, Default {
            n1784 = call "CRYConversion dB-Lin.vi"("dB ref."=w2587, "Log In"=w2589) -> ("Lin Out"=w2588:dbl)  [unwired: 4 in, 3 out]
          }
          frame 1 {
          }
        }
        "Sens y" <- w2556
        n1785 = Multiply(x=w2556, y=w2563) -> (x*y=w2555:dbl)
        n1786 = call "CRYConversion dB-Lin.vi"("unit prefix"=w2565, "dB ref."=w2553, "Lin In"=w2555) -> ("Log Out"=w2586:dbl)  [unwired: 3 in, 3 out]
        n1787 = local write "MaxLevel_1"(w2555) -> ()
        n1788 = local write "MaxLevel_2"(w2586) -> ()
        n1789 = property on="dB ref." class="DigNum (strict)"("Value"=w2553) -> ()  [unwired: 2 in, 2 out]
        n1790 = Match Pattern(string=w2552, regular expression="/") -> (before substring=w2551:string)  [unwired: 4 out]
        n1791 = Format Value(string ("")="", format string="%#.1p", value (0)=w2553) -> (output string=w2570:string)
        n1792 = Concatenate Strings(w2551, "  RMS" ("string")) -> (w2575:string)
        n1793 = Concatenate Strings(w2551, "p" ("string")) -> (w2578:string)
        n1794 = Concatenate Strings("dB re " ("string"), w2570, w2551) -> (w2571:string)
        n1795 = Build Array(w2575, "dB RMS" ("element"), w2578) -> (w2579:string[])
        n1796 = Build Array(w2575, w2571) -> (w2572:string[])
        n1797 = flat-sequence {
          tunnel: w2579 -> [w2596]
          tunnel: w2572 -> [w2595]
          tunnel: w2559 -> [w2591]
          tunnel: w2561 -> [w2613]
          frame #0 {
            n1798 = property on="unit1" class="Ring (strict)"("Strings []"=w2595) -> ()  [unwired: 2 in, 2 out]
            n1799 = property on="unit2" class="Ring (strict)"("Strings []"=w2595) -> ()  [unwired: 2 in, 2 out]
            n1800 = property on="unit3" class="Ring (strict)"("Strings []"=w2595) -> ()  [unwired: 2 in, 2 out]
            n1801 = property on="unit6" class="Ring (strict)"("Strings []"=w2595) -> ()  [unwired: 2 in, 2 out]
            n1802 = property on="unit6_1" class="Ring (strict)"("Strings []"=w2595) -> ()  [unwired: 2 in, 2 out]
            n1803 = property on="unit4" class="Ring (strict)"("Strings []"=w2596) -> ()  [unwired: 2 in, 2 out]
            n1804 = property on="unit7" class="Ring (strict)"("Strings []"=w2596) -> ()  [unwired: 2 in, 2 out]
            n1805 = property on="unit8" class="Ring (strict)"("Strings []"=w2596) -> ()  [unwired: 2 in, 2 out]
            n1806 = To Unsigned Long Integer(number=w2591) -> (unsigned 32bit integer=w2592:u32)
            n1807 = property on="Max Freq" class="DigNum (strict)"("Value"=w2591) -> ()  [unwired: 2 in, 2 out]
            n1808 = call "CRYStimulus Freq Max Limit.vi"("Decrement Flag"=TRUE, "Max Freq"=w2592, "Input Val"=w2592) -> ("Output Val"=w2594:dbl)  [unwired: 1 in, 7 out]
            n1809 = property on="Res Max Freq" class="DigNum (strict)"("Value"=w2594) -> ()  [unwired: 2 in, 2 out]
          }
          frame #1 {
            n1810 = Index Array(array=w2613, index #1=0 ("index"), index #2=1 ("index"), index #3=2 ("index"), index #4=3 ("index"), index #5=4 ("index"), index #6=5 ("index"), index #7=6 ("index"), index #8=7 ("index")) -> (element #1=w2605:u16, element #2=w2604:u16, element #3=w2603:u16, element #4=w2602:u16, element #5=w2601:u16, element #6=w2600:u16, element #7=w2599:u16, element #8=w2598:u16)
            n1811 = property on="unit1" class="Ring (strict)"("Value"=w2605) -> ()  [unwired: 2 in, 2 out]
            n1812 = property on="unit2" class="Ring (strict)"("Value"=w2604) -> ()  [unwired: 2 in, 2 out]
            n1813 = property on="unit3" class="Ring (strict)"("Value"=w2603) -> ()  [unwired: 2 in, 2 out]
            n1814 = property on="unit4" class="Ring (strict)"("Value"=w2602) -> ()  [unwired: 2 in, 2 out]
            n1815 = property on="unit6" class="Ring (strict)"("Value"=w2601) -> ()  [unwired: 2 in, 2 out]
            n1816 = property on="unit6_1" class="Ring (strict)"("Value"=w2600) -> ()  [unwired: 2 in, 2 out]
            n1817 = property on="unit7" class="Ring (strict)"("Value"=w2599) -> ()  [unwired: 2 in, 2 out]
            n1818 = property on="unit8" class="Ring (strict)"("Value"=w2598) -> ()  [unwired: 2 in, 2 out]
            n1819 = property on="Stimulus Type" class="Ring (strict)"() -> ("Value"=w2597:u16)  [unwired: 2 in, 2 out]
            n1820 = property on="Stimulus Type" class="Ring (strict)"("Val(Sgnl)"=w2597) -> ()  [unwired: 2 in, 2 out]
          }
        }
        n1821 = Unbundle By Name(w2562) -> ("Unit_Array"=w2561:u16[])
      }
    }
    n1822 = global read "CRYMainGlobal.vi" "STOP"() -> (w48:bool)
    n1823 = Bundle("Load_Test"="Load_Test", "OK"="OK", "Cancel"="Cancel") -> (w51:T22)  [unwired: 1 out]
    n1824 = Cluster To Array(cluster=w51) -> (array=w52:bool[])
    n1825 = Search 1D Array(1D array=w52, element=TRUE) -> (index of element=w49:i32)  [unwired: 1 out]
    n1826 = case shown="0" w49 {
      tunnel: [FALSE ("element") FALSE ("element") w546 w555] -> w47
      tunnel: w41 -> [_ w61 _ _]
      tunnel: w40 -> [_ _ w545 w554]
      tunnel: w35 -> [_ w59 _ _]
      tunnel: w33 -> [_ w58 _ _]
      frame Default {
      }
      frame 0 {
        n1827 = stacked-sequence {
          seq-local: [w96 _ _ _ _] -> [_ w169 w193 w237 _]
          seq-local: [w77 _ _ _ _] -> [_ _ _ w233 _]
          seq-local: [w66 _ _ _ _] -> [_ _ _ w227 _]
          seq-local: [w74 _ _ _ _] -> [_ w115 _ _ _]
          tunnel: [_ _ _ _ w544] -> w62
          tunnel: w61 -> [w78 _ _ _ _]
          tunnel: w59 -> [w69 _ _ _ _]
          tunnel: w58 -> [_ _ w186 _ _]
          frame #0 {
            n1828 = local read "Stimulus In"() -> (w96:T2)
            n1829 = Unbundle By Name(w96) -> ("UseMLValArray"=w95:u16[], "Cycle/step1(#)"=w91:u32, "Time/step1(s)"=w90:dbl, "Transition1"=w79:dbl, "SweepRate2"=w89:dbl, "Freq3(Hz)"=w80:dbl, "Cycles3(#)"=w88:u32, "Steps3(#)"=w87:dbl, "StepSize3"=w86:dbl, "Help"=w75:string)
            n1830 = local write "Stimulus Out"(w96) -> ()
            n1831 = Index Array(array=w95) -> (element=w94:u16)  [unwired: 1 in]
            n1832 = property on="Cycle/step1" class="DigNum (strict)"("Value"=w91) -> ()  [unwired: 2 in, 2 out]
            n1833 = property on="Time/steps1(s)" class="DigNum (strict)"("Value"=w90) -> ()  [unwired: 2 in, 2 out]
            n1834 = property on="Transition1" class="DigNum (strict)"("Value"=w79) -> ()  [unwired: 2 in, 2 out]
            n1835 = property on="UseMLVal_Level_8" class="Slide (strict)"("Value"=w94) -> ()  [unwired: 2 in, 2 out]
            n1836 = property on="Help" class="Str"("Value"=w75) -> ()  [unwired: 2 in, 2 out]
            n1837 = property on="UseMLVal_Level_1" class="Slide (strict)"("Value"=w94) -> ()  [unwired: 2 in, 2 out]
            n1838 = property on="UseMLVal_Level_2" class="Slide (strict)"("Value"=w94) -> ()  [unwired: 2 in, 2 out]
            n1839 = property on="UseMLVal_Level_3" class="Slide (strict)"("Value"=w94) -> ()  [unwired: 2 in, 2 out]
            n1840 = property on="UseMLVal_Level_4" class="Slide (strict)"("Value"=w94) -> ()  [unwired: 2 in, 2 out]
            n1841 = property on="UseMLVal_Level6_1" class="Slide (strict)"("Value"=w94) -> ()  [unwired: 2 in, 2 out]
            n1842 = property on="UseMLVal_Level6_2" class="Slide (strict)"("Value"=w94) -> ()  [unwired: 2 in, 2 out]
            n1843 = property on="UseMLVal_Level_7" class="Slide (strict)"("Value"=w94) -> ()  [unwired: 2 in, 2 out]
            n1844 = property on="Freq3(Hz)" class="DigNum (strict)"("Value"=w80) -> ()  [unwired: 2 in, 2 out]
            n1845 = property on="Cycles3" class="DigNum (strict)"("Value"=w88) -> ()  [unwired: 2 in, 2 out]
            n1846 = property on="Steps3" class="DigNum (strict)"("Value"=w87) -> ()  [unwired: 2 in, 2 out]
            n1847 = property on="Step Size3" class="DigNum (strict)"("Value"=w86) -> ()  [unwired: 2 in, 2 out]
            n1848 = property on="Sweept Rate2(s/dec)" class="DigNum (strict)"("Value"=w89) -> ()  [unwired: 2 in, 2 out]
            n1849 = Unbundle By Name(w96) -> ("ML_axisArray"=w93:u16[], "WavePath4"=w85:string, "wave time"=w81:string, "RMS_Value4"=w84:dbl, "Peak_Value4"=w83:dbl, "dc_ctrl5_1"=w82:u16, "Signal Type Name"=w66:string, "Channel Sel"=w73:u16)
            n1850 = local write "RealFreq3(Hz)"(w80) -> ()
            n1851 = property on="Wave Channel" class="Ring (strict)"("Value"=w73) -> ()  [unwired: 2 in, 2 out]
            n1852 = Index Array(array=w93) -> (element=w92:u16)  [unwired: 1 in]
            n1853 = property on="ML axis1" class="Slide (strict)"("Value"=w92) -> ()  [unwired: 2 in, 2 out]
            n1854 = property on="ML axis2" class="Slide (strict)"("Value"=w92) -> ()  [unwired: 2 in, 2 out]
            n1855 = property on="ML axis3" class="Slide (strict)"("Value"=w92) -> ()  [unwired: 2 in, 2 out]
            n1856 = property on="ML axis4" class="Slide (strict)"("Value"=w92) -> ()  [unwired: 2 in, 2 out]
            n1857 = property on="ML axis6_1" class="Slide (strict)"("Value"=w92) -> ()  [unwired: 2 in, 2 out]
            n1858 = property on="ML axis6_2" class="Slide (strict)"("Value"=w92) -> ()  [unwired: 2 in, 2 out]
            n1859 = property on="ML axis7" class="Slide (strict)"("Value"=w92) -> ()  [unwired: 2 in, 2 out]
            n1860 = property on="ML axis8" class="Slide (strict)"("Value"=w92) -> ()  [unwired: 2 in, 2 out]
            n1861 = property on="wave time" class="Str"("Value"=w81) -> ()  [unwired: 2 in, 2 out]
            n1862 = property on="RMS value4" class="DigNum (strict)"("Value"=w84) -> ()  [unwired: 2 in, 2 out]
            n1863 = property on="Peak value4" class="DigNum (strict)"("Value"=w83) -> ()  [unwired: 2 in, 2 out]
            n1864 = property on="dc_ctrl5_1" class="Slide (strict)"("Value"=w82) -> ()  [unwired: 2 in, 2 out]
            n1865 = property on="Wave Path4" class="Path"("Text.Text"=w85) -> ()  [unwired: 2 in, 2 out]
            n1866 = Build Array(w66) -> (w71:string[])
            n1867 = call "CRYUnflatten Calibration 2D.vi"("Flattened Calibration"=w69) -> ("Calibration Step Out"=w70:T23)  [unwired: 8 in, 2 out]
            n1868 = call "CRYGet Channel From Signal Type.vi"("Calibration"=w70, "Signal Type Name Array In"=w71, "In/Out?"=FALSE) -> ("Channel Name Array Out"=w68:string[])  [unwired: 7 in, 1 out]
            n1869 = Index Array(array=w68) -> (element=w67:string)  [unwired: 1 in]
            n1870 = for {
              tunnel: w78 -> [w107] mode=indexing
              tunnel: w67 -> [w99]
              tunnel: [w102] -> w76
              tunnel: [w101] -> w77
              tunnel: [w100] -> w74
              tunnel: w66 -> [w98]
              stop <- w103 stop-if-true
              n1871 = Unbundle By Name(w107) -> ("Name"=w97:string, "Sampling Rate (Hz)"=w105:u32, "Vmax (V)"=w104:dbl, "Anti-aliasing Factor (%fs)"=w100:sgl)
              n1872 = Equal?(x=w99, y=w97) -> (x = y?=w106:bool)
              n1873 = case shown="False" w106 {
                tunnel: w105 -> [_ w113]
                tunnel: w104 -> [_ w112]
                tunnel: [u32 44100 ("Sampling Rate (Hz)") w113] -> w102
                tunnel: [1.0 ("Vmax (V)") w112] -> w101
                tunnel: [FALSE TRUE] -> w103
                tunnel: w98 -> [_ _]
                frame False {
                }
                frame True {
                }
              }
            }
            "Sampling Rate (Hz)" <- w76
          }
          frame #1 {
            n1874 = Unbundle By Name(w169) -> ("Level(U)Array"=w167:dbl[], "RMS_unit4"=w165:string, "Peak_unit4"=w163:string, "dc_ctrl5_2"=w162:u16, "dc_polar5"=w161:u16, "Max.Current"=w160:u16, "Steps5(#)"=w159:u32)
            n1875 = property on="RMS unit4" class="Ring (strict)"() -> ("Strings []"=w166:string[])  [unwired: 2 in, 2 out]
            n1876 = property on="Peak unit4" class="Ring (strict)"() -> ("Strings []"=w164:string[])  [unwired: 2 in, 2 out]
            n1877 = Search 1D Array(1D array=w166, element=w165) -> (index of element=w138:i32)  [unwired: 1 out]
            n1878 = Search 1D Array(1D array=w164, element=w163) -> (index of element=w134:i32)  [unwired: 1 out]
            n1879 = Index Array(array=w167, index #1=0 ("index"), index #2=1 ("index")) -> (element #1=w129:dbl, element #2=w128:dbl)
            n1880 = property on="Level(U)2" class="DigNum (strict)"("Value"=w129) -> ()  [unwired: 2 in, 2 out]
            n1881 = property on="Level4(U)" class="DigNum (strict)"("Value"=w129) -> ()  [unwired: 2 in, 2 out]
            n1882 = property on="Level6_1(U)" class="DigNum (strict)"("Value"=w129) -> ()  [unwired: 2 in, 2 out]
            n1883 = property on="Level7(U)" class="DigNum (strict)"("Value"=w129) -> ()  [unwired: 2 in, 2 out]
            n1884 = property on="Level8(U)" class="DigNum (strict)"("Value"=w129) -> ()  [unwired: 2 in, 2 out]
            n1885 = property on="Level(U)1" class="DigNum (strict)"("Value"=w129) -> ()  [unwired: 2 in, 2 out]
            n1886 = property on="LinLevel1" class="DigNum (strict)"("Value"=w129) -> ()  [unwired: 2 in, 2 out]
            n1887 = property on="dc_ctrl5_2" class="Slide (strict)"("Value"=w162) -> ()  [unwired: 2 in, 2 out]
            n1888 = property on="dcpolar5" class="Slide (strict)"("Value"=w161) -> ()  [unwired: 2 in, 2 out]
            n1889 = property on="Max.Current" class="Slide (strict)"("Value"=w160) -> ()  [unwired: 2 in, 2 out]
            n1890 = property on="Steps5" class="DigNum (strict)"("Value"=w159) -> ()  [unwired: 2 in, 2 out]
            n1891 = Less Than 0?(x=w138) -> (x < 0?=w139:bool)
            n1892 = Less Than 0?(x=w134) -> (x < 0?=w136:bool)
            n1893 = Select(t=0, s=w139, f=w138) -> (s? t:f=w137:i32)
            n1894 = Select(t=0, s=w136, f=w134) -> (s? t:f=w133:i32)
            n1895 = Unbundle By Name(w169) -> ("Start(Stop)FreqArray"=w142:dbl[], "Start(Stop)AmpArray"=w157:dbl[])
            n1896 = property on="List Index" class="DigNum (strict)"() -> ("Value"=w126:i32)  [unwired: 2 in, 2 out]
            n1897 = property on="Level6_2(U)" class="DigNum (strict)"("Value"=w128) -> ()  [unwired: 2 in, 2 out]
            n1898 = property on="Peak unit4" class="Ring (strict)"("Value"=w137) -> ()  [unwired: 2 in, 2 out]
            n1899 = property on="RMS unit4" class="Ring (strict)"("Value"=w133) -> ()  [unwired: 2 in, 2 out]
            n1900 = property on="LinLevel2" class="DigNum (strict)"("Value"=w128) -> ()  [unwired: 2 in, 2 out]
            n1901 = Greater Or Equal To 0?(x=w126) -> (x >= 0?=w127:bool)
            n1902 = Unbundle By Name(w169) -> ("Flatten Element Array"=w130:string[])
            n1903 = case shown="True" w127 {
              tunnel: w130 -> [_ w183]
              tunnel: w126 -> [_ w182]
              tunnel: [0 ("Sweep type") w181] -> w124
              frame False {
              }
              frame True {
                n1904 = Index Array(array=w183, index=w182) -> (element=w185:string)
                n1905 = call "CRYUnflatten Stimulus Element.vi"("Unflatten Stimulus Element setup"=w185) -> ("Stimulus Para"=w184:T24)  [unwired: 1 in, 9 out]
                n1906 = Unbundle By Name(w184) -> ("Sweep type"=w181:i32)
              }
            }
            n1907 = Index Array(array=w142, index #1=0 ("index"), index #2=1 ("index")) -> (element #1=w143:dbl, element #2=w120:dbl)
            n1908 = Index Array(array=w157, index #1=0 ("index"), index #2=1 ("index")) -> (element #1=w148:dbl, element #2=w118:dbl)
            n1909 = To Unsigned Long Integer(number=w115) -> (unsigned 32bit integer=w132:u32)
            n1910 = property on="Max Freq" class="DigNum (strict)"("Value"=w115) -> ()  [unwired: 2 in, 2 out]
            n1911 = property on="Start Amp3" class="DigNum (strict)"("Value"=w148) -> ()  [unwired: 2 in, 2 out]
            n1912 = property on="Stop Amp3" class="DigNum (strict)"("Value"=w118) -> ()  [unwired: 2 in, 2 out]
            n1913 = property on="StopAmp5" class="DigNum (strict)"("Value"=w118) -> ()  [unwired: 2 in, 2 out]
            n1914 = property on="StartAmp5" class="DigNum (strict)"("Value"=w148) -> ()  [unwired: 2 in, 2 out]
            n1915 = property on="StopFreq1(Hz)" class="DigNum (strict)"("Value"=w120) -> ()  [unwired: 2 in, 2 out]
            n1916 = property on="StartFreq6(Hz)" class="DigNum (strict)"("Value"=w143) -> ()  [unwired: 2 in, 2 out]
            n1917 = property on="StopFreq6(Hz)" class="DigNum (strict)"("Value"=w120) -> ()  [unwired: 2 in, 2 out]
            n1918 = property on="StartFreq1(Hz)" class="DigNum (strict)"("Value"=w143) -> ()  [unwired: 2 in, 2 out]
            n1919 = property on="Stimulus Type" class="Ring (strict)"("Value"=w124) -> ()  [unwired: 2 in, 2 out]
            n1920 = Unbundle By Name(w169) -> ("StepResolutionArray"=w116:u16[], "Time/Step5"=w156:dbl, "Level5"=w155:dbl, "StepsSize5Val"=w154:dbl, "StepSize5Unit"=w114:string, "SweepType"=w153:u16, "Fixed/Ratio6"=w152:u16, "Transition6"=w151:dbl, "Cycle/Steps6(#)"=w150:u32, "Time/Steps6(s)"=w149:dbl, "Start(Stop)FreqArray"=w145:dbl[])
            n1921 = case shown="Default" w124 {
              tunnel: [u16 5 ("t") w171 w174 w177] -> w117
              tunnel: w116 -> [_ w173 w176 w179]
              frame Default {
              }
              frame 0 {
                n1922 = Index Array(array=w173, index=0) -> (element=w171:u16)
                n1923 = property on="Step Resolution1" class="Ring (strict)"("Value"=w171) -> ()  [unwired: 2 in, 2 out]
              }
              frame 5 {
                n1924 = Index Array(array=w176, index=1) -> (element=w174:u16)
                n1925 = property on="StepResolution6" class="Ring (strict)"("Value"=w174) -> ()  [unwired: 2 in, 2 out]
              }
              frame 7 {
                n1926 = Index Array(array=w179, index=2) -> (element=w177:u16)
                n1927 = property on="Step Resolution8" class="Ring (strict)"("Value"=w177) -> ()  [unwired: 2 in, 2 out]
              }
            }
            n1928 = call "CRYStimulus Freq Max Limit.vi"("Resolution"=w117, "Decrement Flag"=TRUE, "Max Freq"=w132, "Input Val"=w132) -> ("Output Val"=w125:dbl)  [unwired: 7 out]
            n1929 = property on="Res Max Freq" class="DigNum (strict)"("Value"=w125) -> ()  [unwired: 2 in, 2 out]
            n1930 = Index Array(array=w145, index #1=2 ("index"), index #2=3 ("index")) -> (element #1=w146:dbl, element #2=w122:dbl)
            n1931 = property on="Sweep Type" class="Slide (strict)"("Val(Sgnl)"=w153) -> ()  [unwired: 2 in, 2 out]
            n1932 = property on="Fixed/Ratio6" class="Slide (strict)"("Val(Sgnl)"=w152) -> ()  [unwired: 2 in, 2 out]
            n1933 = property on="Time/Step5" class="DigNum (strict)"("Value"=w156) -> ()  [unwired: 2 in, 2 out]
            n1934 = property on="Level5" class="DigNum (strict)"("Value"=w155) -> ()  [unwired: 2 in, 2 out]
            n1935 = property on="Steps Size5" class="DigNum (strict)"("Value"=w154) -> ()  [unwired: 2 in, 2 out]
            n1936 = property on="Transition6" class="DigNum (strict)"("Value"=w151) -> ()  [unwired: 2 in, 2 out]
            n1937 = property on="Cycle/steps6" class="DigNum (strict)"("Value"=w150) -> ()  [unwired: 2 in, 2 out]
            n1938 = property on="Time/step6(s)" class="DigNum (strict)"("Value"=w149) -> ()  [unwired: 2 in, 2 out]
            n1939 = property on="StartFreq2(Hz)" class="DigNum (strict)"("Value"=w146) -> ()  [unwired: 2 in, 2 out]
            n1940 = property on="StopFreq2(Hz)" class="DigNum (strict)"("Value"=w122) -> ()  [unwired: 2 in, 2 out]
            n1941 = property on="unit5_2" class="Str"("Value"=w114) -> ()  [unwired: 2 in, 2 out]
            n1942 = property on="unit5_1" class="Str"("Value"=w114) -> ()  [unwired: 2 in, 2 out]
          }
          frame #2 {
            n1943 = Unbundle By Name(w193) -> ("NoiseType7"=w219:u16, "Difference6(Hz)"=w222:dbl, "Ratio6"=w220:string, "DegValArray"=w217:dbl[], "DegUnitArray"=w214:string[], "Duration7(s)"=w212:dbl, "TabCtrl6"=w199:enum32{"Master Tone", "Slave Tone"})
            n1944 = property on="Ratio6" class="Ring (strict)"() -> ("Strings []"=w221:string[])  [unwired: 2 in, 2 out]
            n1945 = Index Array(array=w217, index=0) -> (element=w216:dbl)
            n1946 = Search 1D Array(1D array=w221, element=w220) -> (index of element=w196:i32)  [unwired: 1 out]
            n1947 = property on="Difference6(Hz)" class="DigNum (strict)"("Value"=w222) -> ()  [unwired: 2 in, 2 out]
            n1948 = property on="Noise Type7" class="Slide (strict)"("Value"=w219) -> ()  [unwired: 2 in, 2 out]
            n1949 = Less Than 0?(x=w196) -> (x < 0?=w197:bool)
            n1950 = property on="deg1" class="DigNum (strict)"("Value"=w216) -> ()  [unwired: 2 in, 2 out]
            n1951 = property on="deg2" class="DigNum (strict)"("Value"=w216) -> ()  [unwired: 2 in, 2 out]
            n1952 = property on="deg3" class="DigNum (strict)"("Value"=w216) -> ()  [unwired: 2 in, 2 out]
            n1953 = property on="deg4" class="DigNum (strict)"("Value"=w216) -> ()  [unwired: 2 in, 2 out]
            n1954 = property on="deg6" class="DigNum (strict)"("Value"=w216) -> ()  [unwired: 2 in, 2 out]
            n1955 = property on="deg6_1" class="DigNum (strict)"("Value"=w216) -> ()  [unwired: 2 in, 2 out]
            n1956 = property on="deg7" class="DigNum (strict)"("Value"=w216) -> ()  [unwired: 2 in, 2 out]
            n1957 = property on="deg8" class="DigNum (strict)"("Value"=w216) -> ()  [unwired: 2 in, 2 out]
            n1958 = property on="Duration7(s)" class="DigNum (strict)"("Value"=w212) -> ()  [unwired: 2 in, 2 out]
            n1959 = property on="Control6 Tab" class="TabCtl (strict)"("Value"=w199) -> ()  [unwired: 2 in, 2 out]
            n1960 = Select(t=0, s=w197, f=w196) -> (s? t:f=w194:i32)
            n1961 = Index Array(array=w214, index=0) -> (element=w213:string)
            n1962 = property on="Ratio6" class="Ring (strict)"("Value"=w194) -> ()  [unwired: 2 in, 2 out]
            n1963 = property on="deg1" class="DigNum (strict)"("Caption.Text"=w213) -> ()  [unwired: 2 in, 2 out]
            n1964 = property on="deg2" class="DigNum (strict)"("Caption.Text"=w213) -> ()  [unwired: 2 in, 2 out]
            n1965 = property on="deg3" class="DigNum (strict)"("Caption.Text"=w213) -> ()  [unwired: 2 in, 2 out]
            n1966 = property on="deg4" class="DigNum (strict)"("Caption.Text"=w213) -> ()  [unwired: 2 in, 2 out]
            n1967 = property on="deg6" class="DigNum (strict)"("Caption.Text"=w213) -> ()  [unwired: 2 in, 2 out]
            n1968 = property on="deg6_1" class="DigNum (strict)"("Caption.Text"=w213) -> ()  [unwired: 2 in, 2 out]
            n1969 = property on="deg7" class="DigNum (strict)"("Caption.Text"=w213) -> ()  [unwired: 2 in, 2 out]
            n1970 = property on="deg8" class="DigNum (strict)"("Caption.Text"=w213) -> ()  [unwired: 2 in, 2 out]
            n1971 = Unbundle By Name(w193) -> ("Steps1"=w203:i32, "Steps6(#)"=w202:dbl, "Tones8"=w201:dbl, "Freq6(Hz)"=w211:dbl, "FreqRounding8"=w198:bool, "Duration8(s)"=w210:dbl, "RoundingVal8"=w209:dbl, "wave Info"=w208:string, "MinFreq7(Hz)"=w207:dbl, "MinFreq8(Hz)"=w206:dbl, "MaxFreq7(Hz)"=w205:dbl, "MaxFreq8(Hz)"=w204:dbl, "RatioVal6"=w200:dbl)
            n1972 = property on="Steps1" class="DigNum (strict)"("Value"=w203) -> ()  [unwired: 2 in, 2 out]
            n1973 = property on="Steps6" class="DigNum (strict)"("Value"=w202) -> ()  [unwired: 2 in, 2 out]
            n1974 = property on="Tones8" class="DigNum (strict)"("Value"=w201) -> ()  [unwired: 2 in, 2 out]
            n1975 = property on="Freq6(Hz)" class="DigNum (strict)"("Value"=w211) -> ()  [unwired: 2 in, 2 out]
            n1976 = property on="Freq Rounding8" class="Bool (strict)"("Value"=w198) -> ()  [unwired: 2 in, 2 out]
            n1977 = property on="Duration8(s)" class="DigNum (strict)"("Value"=w210) -> ()  [unwired: 2 in, 2 out]
            n1978 = property on="Rounding Val8" class="DigNum (strict)"("Value"=w209) -> ()  [unwired: 2 in, 2 out]
            n1979 = property on="wave info" class="Str"("Value"=w208) -> ()  [unwired: 2 in, 2 out]
            n1980 = property on="StartFreq7(Hz)" class="DigNum (strict)"("Value"=w207) -> ()  [unwired: 2 in, 2 out]
            n1981 = property on="StartFreq8(Hz)" class="DigNum (strict)"("Value"=w206) -> ()  [unwired: 2 in, 2 out]
            n1982 = property on="StopFreq7(Hz)" class="DigNum (strict)"("Value"=w205) -> ()  [unwired: 2 in, 2 out]
            n1983 = property on="StopFreq8(Hz)" class="DigNum (strict)"("Value"=w204) -> ()  [unwired: 2 in, 2 out]
            n1984 = property on="Ratio Freq6(Hz)" class="DigNum (strict)"("Value"=w200) -> ()  [unwired: 2 in, 2 out]
            n1985 = call "CRYGet Upper Step Data.vi"("Type In"=enum16{"Curves", "Values", "Results", "WFM"}."Values", "No.VI"=w186) -> ("Value array"=w188:T5)  [unwired: 9 out]
            n1986 = for {
              tunnel: w188 -> [w224] mode=indexing
              tunnel: [w223] -> w187 mode=indexing
              n1987 = Unbundle By Name(w224) -> ("Name"=w223:string)
            }
            n1988 = call "CRYGet Curve Library Data Name.vi"("sAction"="GetNameByType", "Type"=enum16{"Curves", "Values", "Results", "WFM"}."Values") -> ("sNames"=w190:string[])  [unwired: 6 in, 3 out]
            n1989 = property on="StartFreq1_CurLib" class="Ring (strict)"("Strings []"=w190) -> ()  [unwired: 2 in, 2 out]
            n1990 = property on="StopFreq1_CurLib" class="Ring (strict)"("Strings []"=w190) -> ()  [unwired: 2 in, 2 out]
            n1991 = property on="StartFreq2_CurLib" class="Ring (strict)"("Strings []"=w190) -> ()  [unwired: 2 in, 2 out]
            n1992 = property on="StopFreq2_CurLib" class="Ring (strict)"("Strings []"=w190) -> ()  [unwired: 2 in, 2 out]
            n1993 = property on="StartFreq6_CurLib" class="Ring (strict)"("Strings []"=w190) -> ()  [unwired: 2 in, 2 out]
            n1994 = property on="StopFreq6_CurLib" class="Ring (strict)"("Strings []"=w190) -> ()  [unwired: 2 in, 2 out]
            n1995 = property on="StartFreq7_CurLib" class="Ring (strict)"("Strings []"=w190) -> ()  [unwired: 2 in, 2 out]
            n1996 = property on="StopFreq7_CurLib" class="Ring (strict)"("Strings []"=w190) -> ()  [unwired: 2 in, 2 out]
            n1997 = property on="StartFreq8_CurLib" class="Ring (strict)"("Strings []"=w190) -> ()  [unwired: 2 in, 2 out]
            n1998 = property on="StopFreq8_CurLib" class="Ring (strict)"("Strings []"=w190) -> ()  [unwired: 2 in, 2 out]
            n1999 = property on="ML val level name3" class="Ring (strict)"("Strings []"=w187) -> ()  [unwired: 2 in, 2 out]
            n2000 = property on="ML val level name4" class="Ring (strict)"("Strings []"=w187) -> ()  [unwired: 2 in, 2 out]
            n2001 = property on="ML val level name6_1" class="Ring (strict)"("Strings []"=w187) -> ()  [unwired: 2 in, 2 out]
            n2002 = property on="ML val level name6_2" class="Ring (strict)"("Strings []"=w187) -> ()  [unwired: 2 in, 2 out]
            n2003 = property on="ML val level name7" class="Ring (strict)"("Strings []"=w187) -> ()  [unwired: 2 in, 2 out]
            n2004 = property on="ML val level name8" class="Ring (strict)"("Strings []"=w187) -> ()  [unwired: 2 in, 2 out]
            n2005 = property on="ML val level name" class="Ring (strict)"("Strings []"=w187) -> ()  [unwired: 2 in, 2 out]
            n2006 = property on="ML val level name2" class="Ring (strict)"("Strings []"=w187) -> ()  [unwired: 2 in, 2 out]
          }
          frame #3 {
            n2007 = flat-sequence {
              tunnel: w233 -> [w542]
              tunnel: w227 -> [w543]
              frame #0 {
                "Vmax (V)" <- w542
              }
              frame #1 {
                n2008 = property on="Channel Change" class="Str"("Val(Sgnl)"=w543) -> ()  [unwired: 2 in, 2 out]
              }
            }
            n2009 = Unbundle By Name(w237) -> ("Flatten Element Array"=w234:string[], "Unit_Array"=w225:u16[])  [unwired: 1 out]
            n2010 = call "CRYGet Current Calibration Info.vi"("Is Input?"=FALSE, "Signal Type Name"=w227) -> ("Calibration All Cluster"=w230:T20)  [unwired: 9 out]
            n2011 = Unbundle By Name(w230) -> ("Sens Curve"=w229:T6)
            n2012 = property on="List Index" class="DigNum (strict)"() -> ("Value"=w232:i32)  [unwired: 2 in, 2 out]
            n2013 = property on="Stimulus Type" class="Ring (strict)"() -> ("Value"=w236:u16)  [unwired: 2 in, 2 out]
            n2014 = Unbundle By Name(w229) -> ("Y dB ref"=w226:dbl)
            n2015 = Index Array(array=w234, index=w232) -> (element=w235:string)
            n2016 = Greater Or Equal To 0?(x=w232) -> (x >= 0?=w231:bool)
            n2017 = case shown="True" w231 {
              tunnel: w236 -> [_ w243]
              tunnel: w235 -> [_ w241]
              tunnel: w226 -> [_ w240]
              tunnel: w225 -> [_ w239]
              frame False {
              }
              frame True {
                n2018 = property on="StartFreq1_CurLib" class="Ring (strict)"() -> ("Strings []"=w238:string[])  [unwired: 2 in, 2 out]
                n2019 = call "CRYUnflatten Stimulus Element.vi"("Unflatten Stimulus Element setup"=w241) -> ("Stimulus Default"=w242:T25)  [unwired: 1 in, 9 out]
                n2020 = case shown="3" w243 {
                  tunnel: w242 -> [w286 w326 w352 w379 w398 w458 w494 w537]
                  tunnel: w240 -> [w266 w308 w327 w362 _ w417 _ _]
                  tunnel: w239 -> [w270 w310 w335 w363 _ w424 w480 w520]
                  tunnel: w238 -> [w247 w290 _ _ _ w399 w462 w502]
                  frame 0, Default {
                    n2021 = Unbundle By Name(w286) -> ("fstepsw"=w280:T10)
                    n2022 = Unbundle By Name(w280) -> ("Level(U)"=w265:dbl, "Start Freq(Hz)"=w285:dbl, "Stop Freq(Hz)"=w284:dbl, "Steps (#)"=w283:i32, "Cycles/step(#)"=w282:u32, "Time/step (s)"=w281:dbl, "Step Resolution"=w279:u16, "ML axis"=w278:u8, "Use ML Val level?"=w271:bool, "ML val level name"=w272:string, "Start Freq Name"=w251:string, "Stop Freq Name"=w250:string, "Start Freq Axis"=w261:u8, "Stop Freq Axis"=w262:u8, "Start Freq Flag"=w249:string, "Stop Freq Flag"=w248:string, "Output Imp"=w245:dbl, "Nominal Imp"=w244:dbl, "V on DUT"=w246:bool)
                    n2023 = Index Array(array=w270, index=0) -> (element=w267:u16)
                    n2024 = call "CRYConversion dB-Lin.vi"("dB ref."=w266, "Lin In"=w265) -> ("Log Out"=w264:dbl)  [unwired: 4 in, 3 out]
                    n2025 = Equal To 0?(x=w267) -> (x = 0?=w268:bool)
                    n2026 = property on="V on DUT1" class="Bool (strict)"("Value"=w246) -> ()  [unwired: 2 in, 2 out]
                    n2027 = property on="StartFreq1_Flag" class="Str"("Value"=w249) -> ()  [unwired: 2 in, 2 out]
                    n2028 = property on="StopFreq1_Flag" class="Str"("Value"=w248) -> ()  [unwired: 2 in, 2 out]
                    n2029 = Select(t=w265, s=w268, f=w264) -> (s? t:f=w263:dbl)
                    n2030 = property on="Output Imp1" class="Ring (strict)"("Value"=w245) -> ()  [unwired: 2 in, 2 out]
                    n2031 = property on="ML val level name" class="Ring (strict)"() -> ("Strings []"=w252:string[])  [unwired: 2 in, 2 out]
                    n2032 = Boolean To (0,1)(Boolean=w271) -> (0, 1=w277:i16)
                    n2033 = property on="Nominal Imp1" class="DigNum (strict)"("Value"=w244) -> ()  [unwired: 2 in, 2 out]
                    n2034 = property on="LinLevel1" class="DigNum (strict)"("Value"=w265) -> ()  [unwired: 2 in, 2 out]
                    n2035 = property on="Level(U)1" class="DigNum (strict)"("Value"=w263) -> ()  [unwired: 2 in, 2 out]
                    n2036 = property on="StartFreq1(Hz)" class="DigNum (strict)"("Value"=w285) -> ()  [unwired: 2 in, 2 out]
                    n2037 = property on="StopFreq1(Hz)" class="DigNum (strict)"("Value"=w284) -> ()  [unwired: 2 in, 2 out]
                    n2038 = property on="Steps1" class="DigNum (strict)"("Value"=w283) -> ()  [unwired: 2 in, 2 out]
                    n2039 = property on="Cycle/step1" class="DigNum (strict)"("Value"=w282) -> ()  [unwired: 2 in, 2 out]
                    n2040 = property on="Time/steps1(s)" class="DigNum (strict)"("Value"=w281) -> ()  [unwired: 2 in, 2 out]
                    n2041 = property on="Step Resolution1" class="Ring (strict)"("Value"=w279) -> ()  [unwired: 2 in, 2 out]
                    n2042 = property on="ML axis1" class="Slide (strict)"("Value"=w278) -> ()  [unwired: 2 in, 2 out]
                    n2043 = property on="UseMLVal_Level_1" class="Slide (strict)"("Value"=w277) -> ()  [unwired: 2 in, 2 out]
                    n2044 = Search 1D Array(1D array=w252, element=w272) -> (index of element=w275:i32)  [unwired: 1 out]
                    n2045 = Search 1D Array(1D array=w247, element=w250) -> (index of element=w256:i32)  [unwired: 1 out]
                    n2046 = Search 1D Array(1D array=w247, element=w251) -> (index of element=w259:i32)  [unwired: 1 out]
                    n2047 = Less Than 0?(x=w275) -> (x < 0?=w276:bool)
                    n2048 = Less Than 0?(x=w256) -> (x < 0?=w257:bool)
                    n2049 = Less Than 0?(x=w259) -> (x < 0?=w258:bool)
                    n2050 = Select(t=0, s=w276, f=w275) -> (s? t:f=w273:i32)
                    n2051 = Select(t=0, s=w257, f=w256) -> (s? t:f=w253:i32)
                    n2052 = Select(t=0, s=w258, f=w259) -> (s? t:f=w254:i32)
                    n2053 = property on="ML val level name" class="Ring (strict)"("Value"=w273) -> ()  [unwired: 2 in, 2 out]
                    n2054 = property on="StartFreq1_CurLib" class="Ring (strict)"("Value"=w254) -> ()  [unwired: 2 in, 2 out]
                    n2055 = property on="StopFreq1_CurLib" class="Ring (strict)"("Value"=w253) -> ()  [unwired: 2 in, 2 out]
                    n2056 = property on="StartFreq1_axis" class="Slide (strict)"("Value"=w261) -> ()  [unwired: 2 in, 2 out]
                    n2057 = property on="StopFreq1_axis" class="Slide (strict)"("Value"=w262) -> ()  [unwired: 2 in, 2 out]
                  }
                  frame 1 {
                    n2058 = Unbundle By Name(w326) -> ("flogsw"=w322:T11)
                    n2059 = Unbundle By Name(w322) -> ("Level(U)"=w309:dbl, "Start Freq(Hz)"=w325:dbl, "Stop Freq(Hz)"=w324:dbl, "Sweep Rate(s/dec)"=w323:dbl, "Use ML Val level?"=w306:bool, "ML axis"=w320:u8, "ML val level name"=w319:string, "Start Freq Name"=w296:string, "Stop Freq Name"=w295:string, "Start Freq Axis"=w304:u8, "Stop Freq Axis"=w305:u8, "Start Freq Flag"=w292:string, "Stop Freq Flag"=w291:string, "Output Imp"=w288:dbl, "Nominal Imp"=w287:dbl, "V on DUT"=w289:bool)
                    n2060 = Index Array(array=w310, index=1) -> (element=w312:u16)
                    n2061 = call "CRYConversion dB-Lin.vi"("dB ref."=w308, "Lin In"=w309) -> ("Log Out"=w311:dbl)  [unwired: 4 in, 3 out]
                    n2062 = Equal To 0?(x=w312) -> (x = 0?=w313:bool)
                    n2063 = property on="V on DUT2" class="Bool (strict)"("Value"=w289) -> ()  [unwired: 2 in, 2 out]
                    n2064 = property on="StartFreq2_Flag" class="Str"("Value"=w292) -> ()  [unwired: 2 in, 2 out]
                    n2065 = Select(t=w309, s=w313, f=w311) -> (s? t:f=w307:dbl)
                    n2066 = property on="ML val level name2" class="Ring (strict)"() -> ("Strings []"=w297:string[])  [unwired: 2 in, 2 out]
                    n2067 = property on="Output Imp2" class="Ring (strict)"("Value"=w288) -> ()  [unwired: 2 in, 2 out]
                    n2068 = Boolean To (0,1)(Boolean=w306) -> (0, 1=w321:i16)
                    n2069 = Search 1D Array(1D array=w290, element=w296) -> (index of element=w302:i32)  [unwired: 1 out]
                    n2070 = Search 1D Array(1D array=w290, element=w295) -> (index of element=w299:i32)  [unwired: 1 out]
                    n2071 = property on="StopFreq2_Flag" class="Str"("Value"=w291) -> ()  [unwired: 2 in, 2 out]
                    n2072 = property on="Nominal Imp2" class="DigNum (strict)"("Value"=w287) -> ()  [unwired: 2 in, 2 out]
                    n2073 = property on="LinLevel1" class="DigNum (strict)"("Value"=w309) -> ()  [unwired: 2 in, 2 out]
                    n2074 = property on="Level(U)2" class="DigNum (strict)"("Value"=w307) -> ()  [unwired: 2 in, 2 out]
                    n2075 = property on="StartFreq2(Hz)" class="DigNum (strict)"("Value"=w325) -> ()  [unwired: 2 in, 2 out]
                    n2076 = property on="StopFreq2(Hz)" class="DigNum (strict)"("Value"=w324) -> ()  [unwired: 2 in, 2 out]
                    n2077 = property on="Sweept Rate2(s/dec)" class="DigNum (strict)"("Value"=w323) -> ()  [unwired: 2 in, 2 out]
                    n2078 = property on="UseMLVal_Level_2" class="Slide (strict)"("Value"=w321) -> ()  [unwired: 2 in, 2 out]
                    n2079 = property on="ML axis2" class="Slide (strict)"("Value"=w320) -> ()  [unwired: 2 in, 2 out]
                    n2080 = Search 1D Array(1D array=w297, element=w319) -> (index of element=w317:i32)  [unwired: 1 out]
                    n2081 = Less Than 0?(x=w302) -> (x < 0?=w301:bool)
                    n2082 = Less Than 0?(x=w299) -> (x < 0?=w300:bool)
                    n2083 = Less Than 0?(x=w317) -> (x < 0?=w318:bool)
                    n2084 = Select(t=0, s=w301, f=w302) -> (s? t:f=w294:i32)
                    n2085 = Select(t=0, s=w300, f=w299) -> (s? t:f=w293:i32)
                    n2086 = Select(t=0, s=w318, f=w317) -> (s? t:f=w315:i32)
                    n2087 = property on="StartFreq2_CurLib" class="Ring (strict)"("Value"=w294) -> ()  [unwired: 2 in, 2 out]
                    n2088 = property on="StopFreq2_CurLib" class="Ring (strict)"("Value"=w293) -> ()  [unwired: 2 in, 2 out]
                    n2089 = property on="StartFreq2_axis" class="Slide (strict)"("Value"=w304) -> ()  [unwired: 2 in, 2 out]
                    n2090 = property on="StopFreq2_axis" class="Slide (strict)"("Value"=w305) -> ()  [unwired: 2 in, 2 out]
                    n2091 = property on="ML val level name2" class="Ring (strict)"("Value"=w315) -> ()  [unwired: 2 in, 2 out]
                  }
                  frame 2 {
                    n2092 = Unbundle By Name(w352) -> ("ampsw"=w349:T12)
                    n2093 = Unbundle By Name(w349) -> ("Steps (#)"=w351:i32, "Freq(Hz)"=w340:dbl, "Cycles(#)"=w350:u32, "Start Ampl(U)"=w329:dbl, "Stop Ampl(U)"=w328:dbl, "Use ML Val freq?"=w339:bool, "ML axis"=w347:u8, "ML val freq name"=w345:string)
                    n2094 = property on="ML val level name3" class="Ring (strict)"() -> ("Strings []"=w346:string[])  [unwired: 2 in, 2 out]
                    n2095 = Index Array(array=w335, index=2) -> (element=w332:u16)
                    n2096 = call "CRYConversion dB-Lin.vi"("dB ref."=w327, "Lin In"=w329) -> ("Log Out"=w336:dbl)  [unwired: 4 in, 3 out]
                    n2097 = call "CRYConversion dB-Lin.vi"("dB ref."=w327, "Lin In"=w328) -> ("Log Out"=w334:dbl)  [unwired: 4 in, 3 out]
                    n2098 = Equal To 0?(x=w332) -> (x = 0?=w337:bool)
                    n2099 = Equal To 0?(x=w332) -> (x = 0?=w333:bool)
                    n2100 = Select(t=w329, s=w337, f=w336) -> (s? t:f=w331:dbl)
                    n2101 = Search 1D Array(1D array=w346, element=w345) -> (index of element=w343:i32)  [unwired: 1 out]
                    n2102 = Select(t=w328, s=w333, f=w334) -> (s? t:f=w330:dbl)
                    n2103 = Less Than 0?(x=w343) -> (x < 0?=w344:bool)
                    n2104 = Boolean To (0,1)(Boolean=w339) -> (0, 1=w348:i16)
                    n2105 = Select(t=0, s=w344, f=w343) -> (s? t:f=w341:i32)
                    n2106 = property on="Start Amp3" class="DigNum (strict)"("Value"=w331) -> ()  [unwired: 2 in, 2 out]
                    n2107 = property on="Stop Amp3" class="DigNum (strict)"("Value"=w330) -> ()  [unwired: 2 in, 2 out]
                    n2108 = property on="Steps3" class="DigNum (strict)"("Value"=w351) -> ()  [unwired: 2 in, 2 out]
                    n2109 = property on="Freq3(Hz)" class="DigNum (strict)"("Value"=w340) -> ()  [unwired: 2 in, 2 out]
                    n2110 = property on="Cycles3" class="DigNum (strict)"("Value"=w350) -> ()  [unwired: 2 in, 2 out]
                    n2111 = property on="LinLevel2" class="DigNum (strict)"("Value"=w328) -> ()  [unwired: 2 in, 2 out]
                    n2112 = property on="UseMLVal_Level_3" class="Slide (strict)"("Value"=w348) -> ()  [unwired: 2 in, 2 out]
                    n2113 = property on="LinLevel1" class="DigNum (strict)"("Value"=w329) -> ()  [unwired: 2 in, 2 out]
                    n2114 = property on="ML axis3" class="Slide (strict)"("Value"=w347) -> ()  [unwired: 2 in, 2 out]
                    n2115 = property on="ML val level name3" class="Ring (strict)"("Value"=w341) -> ()  [unwired: 2 in, 2 out]
                    n2116 = local write "RealFreq3(Hz)"(w340) -> ()
                  }
                  frame 3 {
                    n2117 = Unbundle By Name(w379) -> ("wavefile"=w374:T13)
                    n2118 = Unbundle By Name(w374) -> ("Level(U)"=w361:dbl, "Wave Path"=w357:string, "wave info"=w378:string, "wave time"=w377:string, "Peak value4"=w376:dbl, "RMS value4"=w375:dbl, "ML axis"=w373:u8, "Use ML Val level?"=w365:bool, "ML val level name"=w370:string, "wave channel"=w358:u16, "Output Imp"=w355:dbl, "Nominal Imp"=w353:dbl, "V on DUT"=w354:bool)
                    n2119 = Index Array(array=w363, index=3) -> (element=w360:u16)
                    n2120 = property on="V on DUT4" class="Bool (strict)"("Value"=w354) -> ()  [unwired: 2 in, 2 out]
                    n2121 = property on="Wave Channel" class="Ring (strict)"("Value"=w358) -> ()  [unwired: 2 in, 2 out]
                    n2122 = property on="Output Imp4" class="Ring (strict)"("Value"=w355) -> ()  [unwired: 2 in, 2 out]
                    n2123 = property on="LinLevel1" class="DigNum (strict)"("Value"=w361) -> ()  [unwired: 2 in, 2 out]
                    n2124 = case shown="2" w360 {
                      tunnel: w361 -> [w380 w383 w386]
                      tunnel: [w380 w382 w385] -> w359
                      tunnel: w362 -> [_ w381 _]
                      frame 0, Default {
                      }
                      frame 1 {
                        n2125 = call "CRYConversion dB-Lin.vi"("dB ref."=w381, "Lin In"=w383) -> ("Log Out"=w382:dbl)  [unwired: 4 in, 3 out]
                      }
                      frame 2 {
                        n2126 = Multiply(x=w386, y=5.0) -> (x*y=w385:dbl)
                      }
                    }
                    n2127 = Boolean To (0,1)(Boolean=w365) -> (0, 1=w372:i16)
                    n2128 = property on="Nominal Imp4" class="DigNum (strict)"("Value"=w353) -> ()  [unwired: 2 in, 2 out]
                    n2129 = property on="wave info" class="Str"("Value"=w378) -> ()  [unwired: 2 in, 2 out]
                    n2130 = property on="wave time" class="Str"("Value"=w377) -> ()  [unwired: 2 in, 2 out]
                    n2131 = property on="Peak value4" class="DigNum (strict)"("Value"=w376) -> ()  [unwired: 2 in, 2 out]
                    n2132 = property on="RMS value4" class="DigNum (strict)"("Value"=w375) -> ()  [unwired: 2 in, 2 out]
                    n2133 = property on="ML axis4" class="Slide (strict)"("Value"=w373) -> ()  [unwired: 2 in, 2 out]
                    n2134 = property on="UseMLVal_Level_4" class="Slide (strict)"("Value"=w372) -> ()  [unwired: 2 in, 2 out]
                    n2135 = property on="ML val level name4" class="Ring (strict)"() -> ("Strings []"=w371:string[])  [unwired: 2 in, 2 out]
                    n2136 = String To Path(string=w357) -> (path=w356:path)
                    n2137 = Search 1D Array(1D array=w371, element=w370) -> (index of element=w368:i32)  [unwired: 1 out]
                    n2138 = property on="Level4(U)" class="DigNum (strict)"("Value"=w359) -> ()  [unwired: 2 in, 2 out]
                    n2139 = property on="Wave Path4" class="Path"("Val(Sgnl)"=w356) -> ()  [unwired: 2 in, 2 out]
                    n2140 = Less Than 0?(x=w368) -> (x < 0?=w369:bool)
                    n2141 = Select(t=0, s=w369, f=w368) -> (s? t:f=w366:i32)
                    n2142 = property on="ML val level name4" class="Ring (strict)"("Value"=w366) -> ()  [unwired: 2 in, 2 out]
                  }
                  frame 4 {
                    n2143 = Unbundle By Name(w398) -> ("dcconn"=w389:T14)
                    n2144 = Unbundle By Name(w389) -> ("dc ctrl"=w397:u16, "dcmax I"=w396:u16, "dc polar"=w395:u16, "dc ctrl"=w394:u16, "Steps (#)"=w393:i32, "Time/step (s)"=w392:dbl, "Start Ampl(U)"=w391:dbl, "Stop Ampl(U)"=w390:dbl, "Level(U)"=w388:dbl, "Step Size"=w387:dbl)
                    n2145 = property on="dc_ctrl5_1" class="Slide (strict)"("Value"=w397) -> ()  [unwired: 2 in, 2 out]
                    n2146 = property on="Max.Current" class="Slide (strict)"("Value"=w396) -> ()  [unwired: 2 in, 2 out]
                    n2147 = property on="dcpolar5" class="Slide (strict)"("Value"=w395) -> ()  [unwired: 2 in, 2 out]
                    n2148 = property on="dc_ctrl5_2" class="Slide (strict)"("Value"=w394) -> ()  [unwired: 2 in, 2 out]
                    n2149 = property on="Steps5" class="DigNum (strict)"("Value"=w393) -> ()  [unwired: 2 in, 2 out]
                    n2150 = property on="Time/Step5" class="DigNum (strict)"("Value"=w392) -> ()  [unwired: 2 in, 2 out]
                    n2151 = property on="StartAmp5" class="DigNum (strict)"("Value"=w391) -> ()  [unwired: 2 in, 2 out]
                    n2152 = property on="StopAmp5" class="DigNum (strict)"("Value"=w390) -> ()  [unwired: 2 in, 2 out]
                    n2153 = property on="Level5" class="DigNum (strict)"("Value"=w388) -> ()  [unwired: 2 in, 2 out]
                    n2154 = property on="Steps Size5" class="DigNum (strict)"("Value"=w387) -> ()  [unwired: 2 in, 2 out]
                  }
                  frame 5 {
                    n2155 = Unbundle By Name(w458) -> ("twotone"=w402:T15)
                    n2156 = Unbundle By Name(w402) -> ("Time/step (s)"=w457:dbl, "Cycles/step (#)"=w456:u32, "Diff Freq(Hz)"=w455:dbl, "Start Freq(Hz)"=w454:dbl, "Stop Freq(Hz)"=w453:dbl, "Steps (#)"=w452:i32, "Freq2(Hz)"=w451:dbl, "Level(U) 2"=w423:dbl, "Ratio Val"=w450:dbl, "Level(U)"=w418:dbl, "Tone Type"=w449:u8, "TabCtrl6"=w448:enum32{"Master Tone", "Slave Tone"}, "Use ML Val level?"=w429:bool, "Use ML Val level? 2"=w428:bool, "ML axis"=w445:u8, "ML axis 2"=w444:u8, "Diff/Ratio"=w443:u8, "Ratio"=w442:u16, "Ratio Val"=w441:dbl, "ML val level name"=w439:string, "ML val level name 2"=w431:string, "Start Freq Name"=w408:string, "Stop Freq Name"=w407:string, "Start Freq Axis"=w406:u8, "Stop Freq Axis"=w405:u8)
                    n2157 = property on="ML val level name6_1" class="Ring (strict)"() -> ("Strings []"=w440:string[])  [unwired: 2 in, 2 out]
                    n2158 = Index Array(array=w424, index=4) -> (element=w419:u16)
                    n2159 = Search 1D Array(1D array=w440, element=w439) -> (index of element=w437:i32)  [unwired: 1 out]
                    n2160 = call "CRYConversion dB-Lin.vi"("dB ref."=w417, "Lin In"=w423) -> ("Log Out"=w425:dbl)  [unwired: 4 in, 3 out]
                    n2161 = Less Than 0?(x=w437) -> (x < 0?=w438:bool)
                    n2162 = Equal To 0?(x=w419) -> (x = 0?=w426:bool)
                    n2163 = call "CRYConversion dB-Lin.vi"("dB ref."=w417, "Lin In"=w418) -> ("Log Out"=w421:dbl)  [unwired: 4 in, 3 out]
                    n2164 = Select(t=0, s=w438, f=w437) -> (s? t:f=w435:i32)
                    n2165 = Select(t=w423, s=w426, f=w425) -> (s? t:f=w422:dbl)
                    n2166 = Equal To 0?(x=w419) -> (x = 0?=w420:bool)
                    n2167 = property on="ML val level name6_1" class="Ring (strict)"("Value"=w435) -> ()  [unwired: 2 in, 2 out]
                    n2168 = property on="Time/step6(s)" class="DigNum (strict)"("Value"=w457) -> ()  [unwired: 2 in, 2 out]
                    n2169 = property on="Cycle/steps6" class="DigNum (strict)"("Value"=w456) -> ()  [unwired: 2 in, 2 out]
                    n2170 = property on="Difference6(Hz)" class="DigNum (strict)"("Value"=w455) -> ()  [unwired: 2 in, 2 out]
                    n2171 = property on="StartFreq6(Hz)" class="DigNum (strict)"("Value"=w454) -> ()  [unwired: 2 in, 2 out]
                    n2172 = property on="StopFreq6(Hz)" class="DigNum (strict)"("Value"=w453) -> ()  [unwired: 2 in, 2 out]
                    n2173 = property on="Steps6" class="DigNum (strict)"("Value"=w452) -> ()  [unwired: 2 in, 2 out]
                    n2174 = property on="Freq6(Hz)" class="DigNum (strict)"("Value"=w451) -> ()  [unwired: 2 in, 2 out]
                    n2175 = property on="LinLevel2" class="DigNum (strict)"("Value"=w423) -> ()  [unwired: 2 in, 2 out]
                    n2176 = property on="Ratio Freq6(Hz)" class="DigNum (strict)"("Value"=w450) -> ()  [unwired: 2 in, 2 out]
                    n2177 = property on="LinLevel1" class="DigNum (strict)"("Value"=w418) -> ()  [unwired: 2 in, 2 out]
                    n2178 = property on="Sweep Type" class="Slide (strict)"("Value"=w449) -> ()  [unwired: 2 in, 2 out]
                    n2179 = Select(t=w418, s=w420, f=w421) -> (s? t:f=w416:dbl)
                    n2180 = property on="Control6 Tab" class="TabCtl (strict)"("Value"=w448) -> ()  [unwired: 2 in, 2 out]
                    n2181 = property on="Level6_2(U)" class="DigNum (strict)"("Value"=w422) -> ()  [unwired: 2 in, 2 out]
                    n2182 = property on="Level6_1(U)" class="DigNum (strict)"("Value"=w416) -> ()  [unwired: 2 in, 2 out]
                    n2183 = Boolean To (0,1)(Boolean=w429) -> (0, 1=w447:i16)
                    n2184 = Boolean To (0,1)(Boolean=w428) -> (0, 1=w446:i16)
                    n2185 = property on="ML val level name6_2" class="Ring (strict)"() -> ("Strings []"=w409:string[])  [unwired: 2 in, 2 out]
                    n2186 = Unbundle By Name(w402) -> ("Start Freq Flag"=w401:string, "Stop Freq Flag"=w400:string)
                    n2187 = Search 1D Array(1D array=w409, element=w431) -> (index of element=w433:i32)  [unwired: 1 out]
                    n2188 = Search 1D Array(1D array=w399, element=w408) -> (index of element=w414:i32)  [unwired: 1 out]
                    n2189 = Search 1D Array(1D array=w399, element=w407) -> (index of element=w411:i32)  [unwired: 1 out]
                    n2190 = property on="UseMLVal_Level6_1" class="Slide (strict)"("Value"=w447) -> ()  [unwired: 2 in, 2 out]
                    n2191 = property on="UseMLVal_Level6_2" class="Slide (strict)"("Value"=w446) -> ()  [unwired: 2 in, 2 out]
                    n2192 = property on="ML axis6_1" class="Slide (strict)"("Value"=w445) -> ()  [unwired: 2 in, 2 out]
                    n2193 = property on="ML axis6_2" class="Slide (strict)"("Value"=w444) -> ()  [unwired: 2 in, 2 out]
                    n2194 = property on="Fixed/Ratio6" class="Slide (strict)"("Value"=w443) -> ()  [unwired: 2 in, 2 out]
                    n2195 = property on="Ratio6" class="Ring (strict)"("Value"=w442) -> ()  [unwired: 2 in, 2 out]
                    n2196 = property on="Ratio Freq6(Hz)" class="DigNum (strict)"("Value"=w441) -> ()  [unwired: 2 in, 2 out]
                    n2197 = Less Than 0?(x=w433) -> (x < 0?=w432:bool)
                    n2198 = Less Than 0?(x=w414) -> (x < 0?=w415:bool)
                    n2199 = Less Than 0?(x=w411) -> (x < 0?=w410:bool)
                    n2200 = Select(t=0, s=w432, f=w433) -> (s? t:f=w430:i32)
                    n2201 = Select(t=0, s=w415, f=w414) -> (s? t:f=w403:i32)
                    n2202 = Select(t=0, s=w410, f=w411) -> (s? t:f=w404:i32)
                    n2203 = property on="StartFreq6_Flag" class="Str"("Value"=w401) -> ()  [unwired: 2 in, 2 out]
                    n2204 = property on="StopFreq6_Flag" class="Str"("Value"=w400) -> ()  [unwired: 2 in, 2 out]
                    n2205 = property on="ML val level name6_2" class="Ring (strict)"("Value"=w430) -> ()  [unwired: 2 in, 2 out]
                    n2206 = property on="StartFreq6_CurLib" class="Ring (strict)"("Value"=w403) -> ()  [unwired: 2 in, 2 out]
                    n2207 = property on="StopFreq6_CurLib" class="Ring (strict)"("Value"=w404) -> ()  [unwired: 2 in, 2 out]
                    n2208 = property on="StartFreq6_axis" class="Slide (strict)"("Value"=w406) -> ()  [unwired: 2 in, 2 out]
                    n2209 = property on="StopFreq6_axis" class="Slide (strict)"("Value"=w405) -> ()  [unwired: 2 in, 2 out]
                  }
                  frame 6 {
                    n2210 = Unbundle By Name(w494) -> ("noise"=w489:T16)
                    n2211 = flat-sequence {
                      tunnel: w480 -> [w497]
                      tunnel: w479 -> [w495]
                      tunnel: [w495] -> w478
                      frame #0 {
                        n2212 = Index Array(array=w497, index=6) -> (element=w496:u16)
                        n2213 = property on="unit7" class="Ring (strict)"("Value"=w496) -> ()  [unwired: 2 in, 2 out]
                      }
                    }
                    n2214 = Unbundle By Name(w489) -> ("Noise Type"=w493:u8, "Min Freq(Hz)"=w492:dbl, "Max Freq(Hz)"=w491:dbl, "Level(U)"=w479:dbl, "Duration(s)"=w490:dbl, "ML axis"=w488:u8, "Use ML Val level?"=w481:bool, "ML val level name"=w486:string, "Start Freq Name"=w470:string, "Stop Freq Name"=w469:string, "Start Freq Axis"=w468:u8, "Stop Freq Axis"=w467:u8, "Start Freq Flag"=w464:string, "Stop Freq Flag"=w463:string, "Output Imp"=w459:dbl, "Nominal Imp"=w460:dbl, "V on DUT"=w461:bool)
                    n2215 = property on="V on DUT7" class="Bool (strict)"("Value"=w461) -> ()  [unwired: 2 in, 2 out]
                    n2216 = Boolean To (0,1)(Boolean=w481) -> (0, 1=w487:i16)
                    n2217 = property on="ML val level name7" class="Ring (strict)"() -> ("Strings []"=w471:string[])  [unwired: 2 in, 2 out]
                    n2218 = property on="Level7(U)" class="DigNum (strict)"("Val(Sgnl)"=w478) -> ()  [unwired: 2 in, 2 out]
                    n2219 = property on="LinLevel1" class="DigNum (strict)"("Value"=w478) -> ()  [unwired: 2 in, 2 out]
                    n2220 = property on="Noise Type7" class="Slide (strict)"("Value"=w493) -> ()  [unwired: 2 in, 2 out]
                    n2221 = property on="StartFreq7(Hz)" class="DigNum (strict)"("Value"=w492) -> ()  [unwired: 2 in, 2 out]
                    n2222 = property on="StopFreq7(Hz)" class="DigNum (strict)"("Value"=w491) -> ()  [unwired: 2 in, 2 out]
                    n2223 = property on="Duration7(s)" class="DigNum (strict)"("Value"=w490) -> ()  [unwired: 2 in, 2 out]
                    n2224 = property on="ML axis7" class="Slide (strict)"("Value"=w488) -> ()  [unwired: 2 in, 2 out]
                    n2225 = property on="UseMLVal_Level_7" class="Slide (strict)"("Value"=w487) -> ()  [unwired: 2 in, 2 out]
                    n2226 = property on="Output Imp7" class="Ring (strict)"("Value"=w459) -> ()  [unwired: 2 in, 2 out]
                    n2227 = property on="StartFreq7_axis" class="Slide (strict)"("Value"=w468) -> ()  [unwired: 2 in, 2 out]
                    n2228 = property on="StopFreq7_axis" class="Slide (strict)"("Value"=w467) -> ()  [unwired: 2 in, 2 out]
                    n2229 = Search 1D Array(1D array=w471, element=w486) -> (index of element=w484:i32)  [unwired: 1 out]
                    n2230 = Search 1D Array(1D array=w462, element=w470) -> (index of element=w473:i32)  [unwired: 1 out]
                    n2231 = Search 1D Array(1D array=w462, element=w469) -> (index of element=w476:i32)  [unwired: 1 out]
                    n2232 = property on="Nominal Imp7" class="DigNum (strict)"("Value"=w460) -> ()  [unwired: 2 in, 2 out]
                    n2233 = Less Than 0?(x=w484) -> (x < 0?=w485:bool)
                    n2234 = Less Than 0?(x=w473) -> (x < 0?=w474:bool)
                    n2235 = Less Than 0?(x=w476) -> (x < 0?=w475:bool)
                    n2236 = Select(t=0, s=w485, f=w484) -> (s? t:f=w482:i32)
                    n2237 = Select(t=0, s=w474, f=w473) -> (s? t:f=w466:i32)
                    n2238 = Select(t=0, s=w475, f=w476) -> (s? t:f=w465:i32)
                    n2239 = property on="ML val level name7" class="Ring (strict)"("Value"=w482) -> ()  [unwired: 2 in, 2 out]
                    n2240 = property on="StartFreq7_CurLib" class="Ring (strict)"("Value"=w466) -> ()  [unwired: 2 in, 2 out]
                    n2241 = property on="StopFreq7_CurLib" class="Ring (strict)"("Value"=w465) -> ()  [unwired: 2 in, 2 out]
                    n2242 = property on="StartFreq7_Flag" class="Str"("Value"=w464) -> ()  [unwired: 2 in, 2 out]
                    n2243 = property on="StopFreq7_Flag" class="Str"("Value"=w463) -> ()  [unwired: 2 in, 2 out]
                  }
                  frame 7 {
                    n2244 = Unbundle By Name(w537) -> ("mltitone"=w531:T17)
                    n2245 = Unbundle By Name(w531) -> ("Level(U)"=w519:dbl, "Min Freq(Hz)"=w536:dbl, "Max Freq(Hz)"=w535:dbl, "Duration(s)"=w534:dbl, "Profile"=w533:i32, "Rounding Val"=w532:dbl, "Step Resolution"=w530:u16, "Freq Rounding"=w529:bool, "Use ML Val level?"=w521:bool, "ML axis"=w527:u8, "ML val level name"=w526:string, "Start Freq Name"=w512:string, "Stop Freq Name"=w511:string, "Start Freq Axis"=w510:u8, "Stop Freq Axis"=w509:u8, "Start Freq Flag"=w504:string, "Stop Freq Flag"=w503:string, "Output Imp"=w499:dbl, "Nominal Imp"=w500:dbl, "V on DUT"=w501:bool)
                    n2246 = flat-sequence {
                      tunnel: w520 -> [w539]
                      tunnel: w519 -> [w538]
                      tunnel: [w538] -> w518
                      frame #0 {
                        n2247 = Index Array(array=w539, index=7) -> (element=w540:u16)
                        n2248 = property on="unit8" class="Ring (strict)"("Value"=w540) -> ()  [unwired: 2 in, 2 out]
                      }
                    }
                    n2249 = property on="ML val level name8" class="Ring (strict)"() -> ("Strings []"=w513:string[])  [unwired: 2 in, 2 out]
                    n2250 = property on="V on DUT8" class="Bool (strict)"("Value"=w501) -> ()  [unwired: 2 in, 2 out]
                    n2251 = property on="Output Imp8" class="Ring (strict)"("Value"=w499) -> ()  [unwired: 2 in, 2 out]
                    n2252 = Search 1D Array(1D array=w502, element=w511) -> (index of element=w514:i32)  [unwired: 1 out]
                    n2253 = Search 1D Array(1D array=w513, element=w526) -> (index of element=w524:i32)  [unwired: 1 out]
                    n2254 = Search 1D Array(1D array=w502, element=w512) -> (index of element=w517:i32)  [unwired: 1 out]
                    n2255 = Less Than 0?(x=w514) -> (x < 0?=w515:bool)
                    n2256 = Less Than 0?(x=w524) -> (x < 0?=w525:bool)
                    n2257 = Less Than 0?(x=w517) -> (x < 0?=w516:bool)
                    n2258 = property on="Nominal Imp8" class="DigNum (strict)"("Value"=w500) -> ()  [unwired: 2 in, 2 out]
                    n2259 = Select(t=0, s=w515, f=w514) -> (s? t:f=w507:i32)
                    n2260 = Boolean To (0,1)(Boolean=w521) -> (0, 1=w528:i16)
                    n2261 = Select(t=0, s=w525, f=w524) -> (s? t:f=w522:i32)
                    n2262 = Select(t=0, s=w516, f=w517) -> (s? t:f=w508:i32)
                    n2263 = property on="Level8(U)" class="DigNum (strict)"("Val(Sgnl)"=w518) -> ()  [unwired: 2 in, 2 out]
                    n2264 = property on="LinLevel1" class="DigNum (strict)"("Value"=w518) -> ()  [unwired: 2 in, 2 out]
                    n2265 = property on="StartFreq8(Hz)" class="DigNum (strict)"("Value"=w536) -> ()  [unwired: 2 in, 2 out]
                    n2266 = property on="StopFreq8(Hz)" class="DigNum (strict)"("Value"=w535) -> ()  [unwired: 2 in, 2 out]
                    n2267 = property on="Duration8(s)" class="DigNum (strict)"("Value"=w534) -> ()  [unwired: 2 in, 2 out]
                    n2268 = property on="Tones8" class="DigNum (strict)"("Value"=w533) -> ()  [unwired: 2 in, 2 out]
                    n2269 = property on="Rounding Val8" class="DigNum (strict)"("Value"=w532) -> ()  [unwired: 2 in, 2 out]
                    n2270 = property on="Step Resolution8" class="Ring (strict)"("Value"=w530) -> ()  [unwired: 2 in, 2 out]
                    n2271 = property on="Freq Rounding8" class="Bool (strict)"("Value"=w529) -> ()  [unwired: 2 in, 2 out]
                    n2272 = property on="UseMLVal_Level_8" class="Slide (strict)"("Value"=w528) -> ()  [unwired: 2 in, 2 out]
                    n2273 = property on="ML axis8" class="Slide (strict)"("Value"=w527) -> ()  [unwired: 2 in, 2 out]
                    n2274 = property on="ML val level name8" class="Ring (strict)"("Value"=w522) -> ()  [unwired: 2 in, 2 out]
                    n2275 = property on="StartFreq8_CurLib" class="Ring (strict)"("Value"=w508) -> ()  [unwired: 2 in, 2 out]
                    n2276 = property on="StopFreq8_CurLib" class="Ring (strict)"("Value"=w507) -> ()  [unwired: 2 in, 2 out]
                    n2277 = property on="StartFreq8_axis" class="Slide (strict)"("Value"=w510) -> ()  [unwired: 2 in, 2 out]
                    n2278 = property on="StopFreq8_axis" class="Slide (strict)"("Value"=w509) -> ()  [unwired: 2 in, 2 out]
                    n2279 = property on="StartFreq8_Flag" class="Str"("Value"=w504) -> ()  [unwired: 2 in, 2 out]
                    n2280 = property on="StopFreq8_Flag" class="Str"("Value"=w503) -> ()  [unwired: 2 in, 2 out]
                  }
                }
              }
            }
          }
          frame #4 {
            n2281 = property on="Stimulus Type" class="Ring (strict)"() -> ("Value"=w544:u16)  [unwired: 2 in, 2 out]
            n2282 = property on="Stimulus Type" class="Ring (strict)"("Val(Sgnl)"=w544) -> ()  [unwired: 2 in, 2 out]
          }
        }
        n2283 = flat-sequence {
          tunnel: w62 -> [_]
          frame #0 {
            n2284 = local write "Load_Test"(FALSE ("Load_Test")) -> ()
            n2285 = property on="Board1 Tab" class="TabCtl (strict)"("Visible"=TRUE) -> ()  [unwired: 2 in, 2 out]
            n2286 = property on="Control Tab" class="TabCtl (strict)"("Visible"=TRUE) -> ()  [unwired: 2 in, 2 out]
          }
        }
      }
      frame 1 {
        n2287 = case shown="False" w545 {
          tunnel: [w547 FALSE] -> w546
          frame False {
            w547 = TRUE
            n2288 = control-ref of="This VI"() -> (w549:refnum<vi>)
            n2289 = property class="VI"(reference=w549, "Front Panel.Open"=FALSE ("Front Panel Window:Open")) -> ()  [unwired: 1 in, 2 out]
            n2290 = property on="Ok Boolean" class="Bool (strict)"("Value"=w547) -> ()  [unwired: 2 in, 2 out]
            n2291 = global write "CRYStimulus Global.vi" "OK flg"(w547) -> ()
            n2292 = flat-sequence {
              frame #0 {
                n2293 = local read "Stimulus Out"() -> (w551:T2)
                n2294 = local read "Flatten Element Out"() -> (w550:string)
                n2295 = global write "CRYStimulus Global.vi" "Flatten Element Out"(w550) -> ()
                n2296 = global write "CRYStimulus Global.vi" "Stimulus Cluster"(w551) -> ()
              }
              frame #1 {
                n2297 = global write "CRYStimulus Global.vi" "End flg"(TRUE ("End flg")) -> ()
              }
            }
          }
          frame True {
          }
        }
      }
      frame 2 {
        n2298 = case shown="False" w554 {
          tunnel: [TRUE FALSE] -> w555
          frame False {
            w556 = FALSE ("Front Panel Window:Open")
            n2299 = control-ref of="This VI"() -> (w558:refnum<vi>)
            n2300 = property class="VI"(reference=w558, "Front Panel.Open"=w556) -> ()  [unwired: 1 in, 2 out]
            n2301 = property on="Ok Boolean" class="Bool (strict)"("Value"=w556) -> ()  [unwired: 2 in, 2 out]
            n2302 = global write "CRYStimulus Global.vi" "End flg"(TRUE ("End flg")) -> ()
            n2303 = global write "CRYStimulus Global.vi" "OK flg"(w556) -> ()
          }
          frame True {
          }
        }
      }
    }
    n2304 = Compound Arithmetic op=OR(w47, w48, "stop") -> (w46:bool)
  }
